vi "main4ChProspectiveStudy.vi"() -> ()   [LabVIEW 2024]
doc: "Main VI for FLS imaging system."
uses:
  SubVI/DigitizerConfiguration/FLImDAQ.ctl
  <instrlib>/niScope/Controls/niScope trigger source.ctl
  SubVI/LabJack/LJ Pin Setting.ctl
  ConfigFiles/AimingBeamVideoConfig.ctl
  LaguerreDeconLib/DeconEngineClass/LaguerreDeconEngineClass.lvclass/LaguerreDeconEngineClass.ctl
  <vilib>/Utility/error.llb/DialogType.ctl
  LaguerreDeconLib/DeconEngineClass/LaguerreDeconEngineClass.lvclass
  <vilib>/event_ctls.llb/usereventprio.ctl
  <vilib>/Utility/miscctls.llb/LVMinMaxIncTypeDef.ctl
  SubVI/APD/APDClass.lvclass
  <vilib>/Analysis/baseanly.llb/Mean (DBL).vi
  SubVI/GlobalVariables.vi
  <vilib>/addons/control/pid/pid.llb/PID (DBL).vi
  <instrlib>/niScope/Acquire/Fetch/niScope Multi Fetch Binary 16.vi
  <vilib>/Instr/_visa.llb/VISA Configure Serial Port (Instr).vi
  <vilib>/Python/Open Anaconda Python Session.vi
  C:/Users/MarcuLab/Documents/GitHub/NetDeconForLV/Source/DotNETAssembly/output/build/LaguerreDeConNative.dll
  Documents/GitHub/NetDeconForLV/Source/DotNETAssembly/output/build/LaguerreDeConNative.dll
  <userlib>/_OpenG.lib/file/file.llb/openg_file.lvlib
  <userlib>/_OpenG.lib/time/time.llb/openg_time.lvlib
  <vilib>/Analysis/NI_AALBase.lvlib
  <vilib>/Utility/miscctls.llb/LVPointTypeDef.ctl
  <vilib>/addons/control/pid/NI_PID_pid.lvlib
panel:
  in  "488nm Power":u16(ring)=32 items=["3.30mW"=60, "2.35mW"=50, "2.00mW"=47, "1.75mW"=44, "1.48mW"=41, "1.16mW"=38, "0.87mW"=35, "0.57mW"=32, "0.28mW"=29]
  in  "CancerThreshold":dbl=0.15
  out "Decon Loop timing (ms)":dbl
  out "Ch3 Lifetime (ns)":dbl caption="Lifetime (ns)"
  out "Ch2 Lifetime (ns)":dbl caption="Lifetime (ns)"
  out "Ch1 Lifetime (ns)":dbl caption="Lifetime (ns)"
  out "Cancer Prob":dbl
  in  "Overlay selection":u16(ring)=2 items=["Gain", "Lifetime", "CancerProbability"]
  out "Record Backlog 2":i32
  in  "Auto gain ch4":bool=TRUE caption="Auto gain ch3"
  in  "V 4":dbl caption="Gain 3" min=0.0 max=4.67 step=0.1
  out "Gain4":dbl
  out "IntR4":dbl format="%#_2g"
  out "SNR4":dbl format="%#_3g"
  out "Channel 4":dbl[][](graph) caption="Channel 3"
  out "RunStartTime":u32
  out "Dig1 Temp":dbl
  out "Dig2 Temp":dbl
  out "Visualization PC video source":T1
  in  "V target(1.0)":dbl=1.0 caption="V target(1.5)" min=0.3 max=1.5 step=0.1 format="%#_4g"
  out "SNR3":dbl format="%#_3g"
  out "SNR2":dbl format="%#_3g"
  out "SNR1":dbl format="%#_3g"
  in  "Show BG removed?":bool=TRUE
  out "IntR3":dbl format="%#_2g"
  out "IntR2":dbl format="%#_2g"
  out "IntR1":dbl format="%#_2g"
  in  "Video Display":bool
  out "Gain3":dbl
  out "Gain2":dbl
  out "Gain1":dbl
  in  "Skip Data Save?":bool
  out "Aq Loop?":bool
  out "ML?":bool
  out "aquisition loop Error Out":errorcluster
  out "Laser f (Hz)":dbl
  out "Record Backlog":i32
  out "Fetch Record #":i32
  out "Sync Success?":bool
  out "Disclamer":picture
  out "Calibration #":i8
  out "BG #":i8
  in  "TCP Connect":bool
  out "Help":string
  in  "355nm Laser toggle":bool caption="355nm 460Hz"
  in  "Cali&iRF alignment":bool
  in  "Background":bool
  in  "Aiming beam toggle":bool caption="488nm 15Hz"
  in  "Auto gain ch3":bool=TRUE
  in  "Auto gain ch2":bool=TRUE
  in  "Auto gain ch1":bool=TRUE
  out "Run #":i8
  in  "StopButton":bool caption="Stop"
  out "Aquisition Status:":bool
  in  "StartButton":bool caption="Start"
  in  "V 3":dbl caption="Gain 3" min=0.0 max=4.6 step=0.1
  in  "V 2":dbl caption="Gain 2" min=0.0 max=4.6 step=0.1
  in  "V 1":dbl caption="Gain 1" min=0.0 max=4.6 step=0.1 format="%#_4g"
  in  "Video Source":enum32{"Camera", "FrameGrabber"}(radio)
  out "Case #":string
  out "System Hardware Connection Status":T2
  out "Channel 3":dbl[][](graph)
  out "Channel 2":dbl[][](graph)
  out "Channel 1":dbl[][](graph)
  in  "Tab Control":T3(tab)
  out "display loop timing(ms)":u32
  out "Aquisition loop timing(ms)":u32 format="%.2f"
  out "DisplayLoop":i32
  out "PID loop":i32 caption="processing loop"
  out "PID loop timing(ms)":u32 caption="processing loop timing(ms)"
  out "Communication loop(ms)":u32
  out "laser EM lamp V":dbl format="%0.6f"
  out "Auisition Loop idx":i32
  out "LJ process (ms)":u32
  out "LJ time(ms)":u32[](array[numeric])
  out "output variable":i32
  out "BG Graph":dbl[][](graph)
  out "Lifetime (ns)":cluster{dbl, dbl, dbl}(graph)
  out "DeCon Speed(ms)":dbl(graph)
  out "iRF Graph":dbl[][](graph)
  in  "Show BG":bool
  out "iRF length":i32
  out "BG length":i32
  out "data length":i32
  out "WarmupTime(ms)":u32
  out "BGAll":dbl[][](array[numeric])
  out "DeConOut":dbl[](array[numeric])
  in  "Ch1GainLim":dbl=350.0 format="%#_13g"
  in  "Ch2&3GainLim":dbl=1750.0 format="%#_13g"
  out "LJ Pinout":T4={"Ch1 Bias"="DAC0", "Ch2 Bias"="DAC1", "Ch3 Bias"="DAC2", "Ch4 Bias"="DAC0", "355 PWM"="FIO0", "AimingBeam PWM"="FIO2", "Laser Ready"="FIO3", "Interlock"="FIO1", "Laser Start/Stop"="FIO1", "Red LED"="FIO1", "Green LED"="DIO3", "Foot Pedal"="DIO15"}
  out "FLImDAQ":T5={"Digitizer 1"="", "Digitizer 2"="", "Channel"=enum."Channel 0", "trigger source"="VAL_EXTERNAL", "trigger level"=0.5, "trigger delay"=1.35e-07, "min sample rate"=12500000000.0, "min record length"=2500, "vertical range"=1.0, "vertical offset"=-0.25, "Waveform to Avg"=2000} caption="FLIm DAQ Configuration" {"trigger delay" format="%^#.4e"; "trigger level" min=0.0 max=3.5 step=0.5 format="%.2f"; "vertical offset" format="%.4f"; "vertical range" format="%.2f"; "min sample rate" format="%#.2p"}
  in  "Sys Reconfig":bool
  out "data out(communcation loop)":string
  out "PID loop error out":errorcluster caption="processing Error Out"
  out "decon error out":errorcluster
  out "Laser Rep Rate":dbl
  out "V4 Size":i32 caption="V3 Size"
  in  "Data Class":enum16{"Data", "BG", "Cali"}(ring)=enum."BG"
  out "V1 Size":i32
  out "V2 Size":i32
  out "V3 Size":i32
  out "data Size":i32[](array[numeric])
  out "State log":string
  out "SysConfigCluster":T7
  in  "Ch4 PID gains":T8={"proportional gain (Kc)"=30.0, "integral time (Ti, min)"=0.0003, "derivative time (Td, min)"=1e-05}
  in  "Ch3 PID gains":T8={"proportional gain (Kc)"=30.0, "integral time (Ti, min)"=0.0003, "derivative time (Td, min)"=1e-05}
  in  "Ch2 PID gains":T8={"proportional gain (Kc)"=30.0, "integral time (Ti, min)"=0.0003, "derivative time (Td, min)"=1e-05}
  in  "Ch1 PID gains":T8={"proportional gain (Kc)"=30.0, "integral time (Ti, min)"=0.0003, "derivative time (Td, min)"=1e-05}
  in  "module path":path=path "C:/Users/MarcuLab/Documents/GitHub/NetDeconForLV/Classifier/ClassifierModule.py"
  in  "model path":path=path "C:/Users/MarcuLab/Desktop/V6 APD LV/V6 APD LV/ClassifierFile/xgb_model.pkl"
  in  "Env name":string="HNClassifier"
  in  "Python version":string="3.10"
  out "Python session":refnum<k35>
  in  "Quit":bool
  in  "Radio Buttons":T9(radio)=enum."Ch2" caption="DeCon Chan"
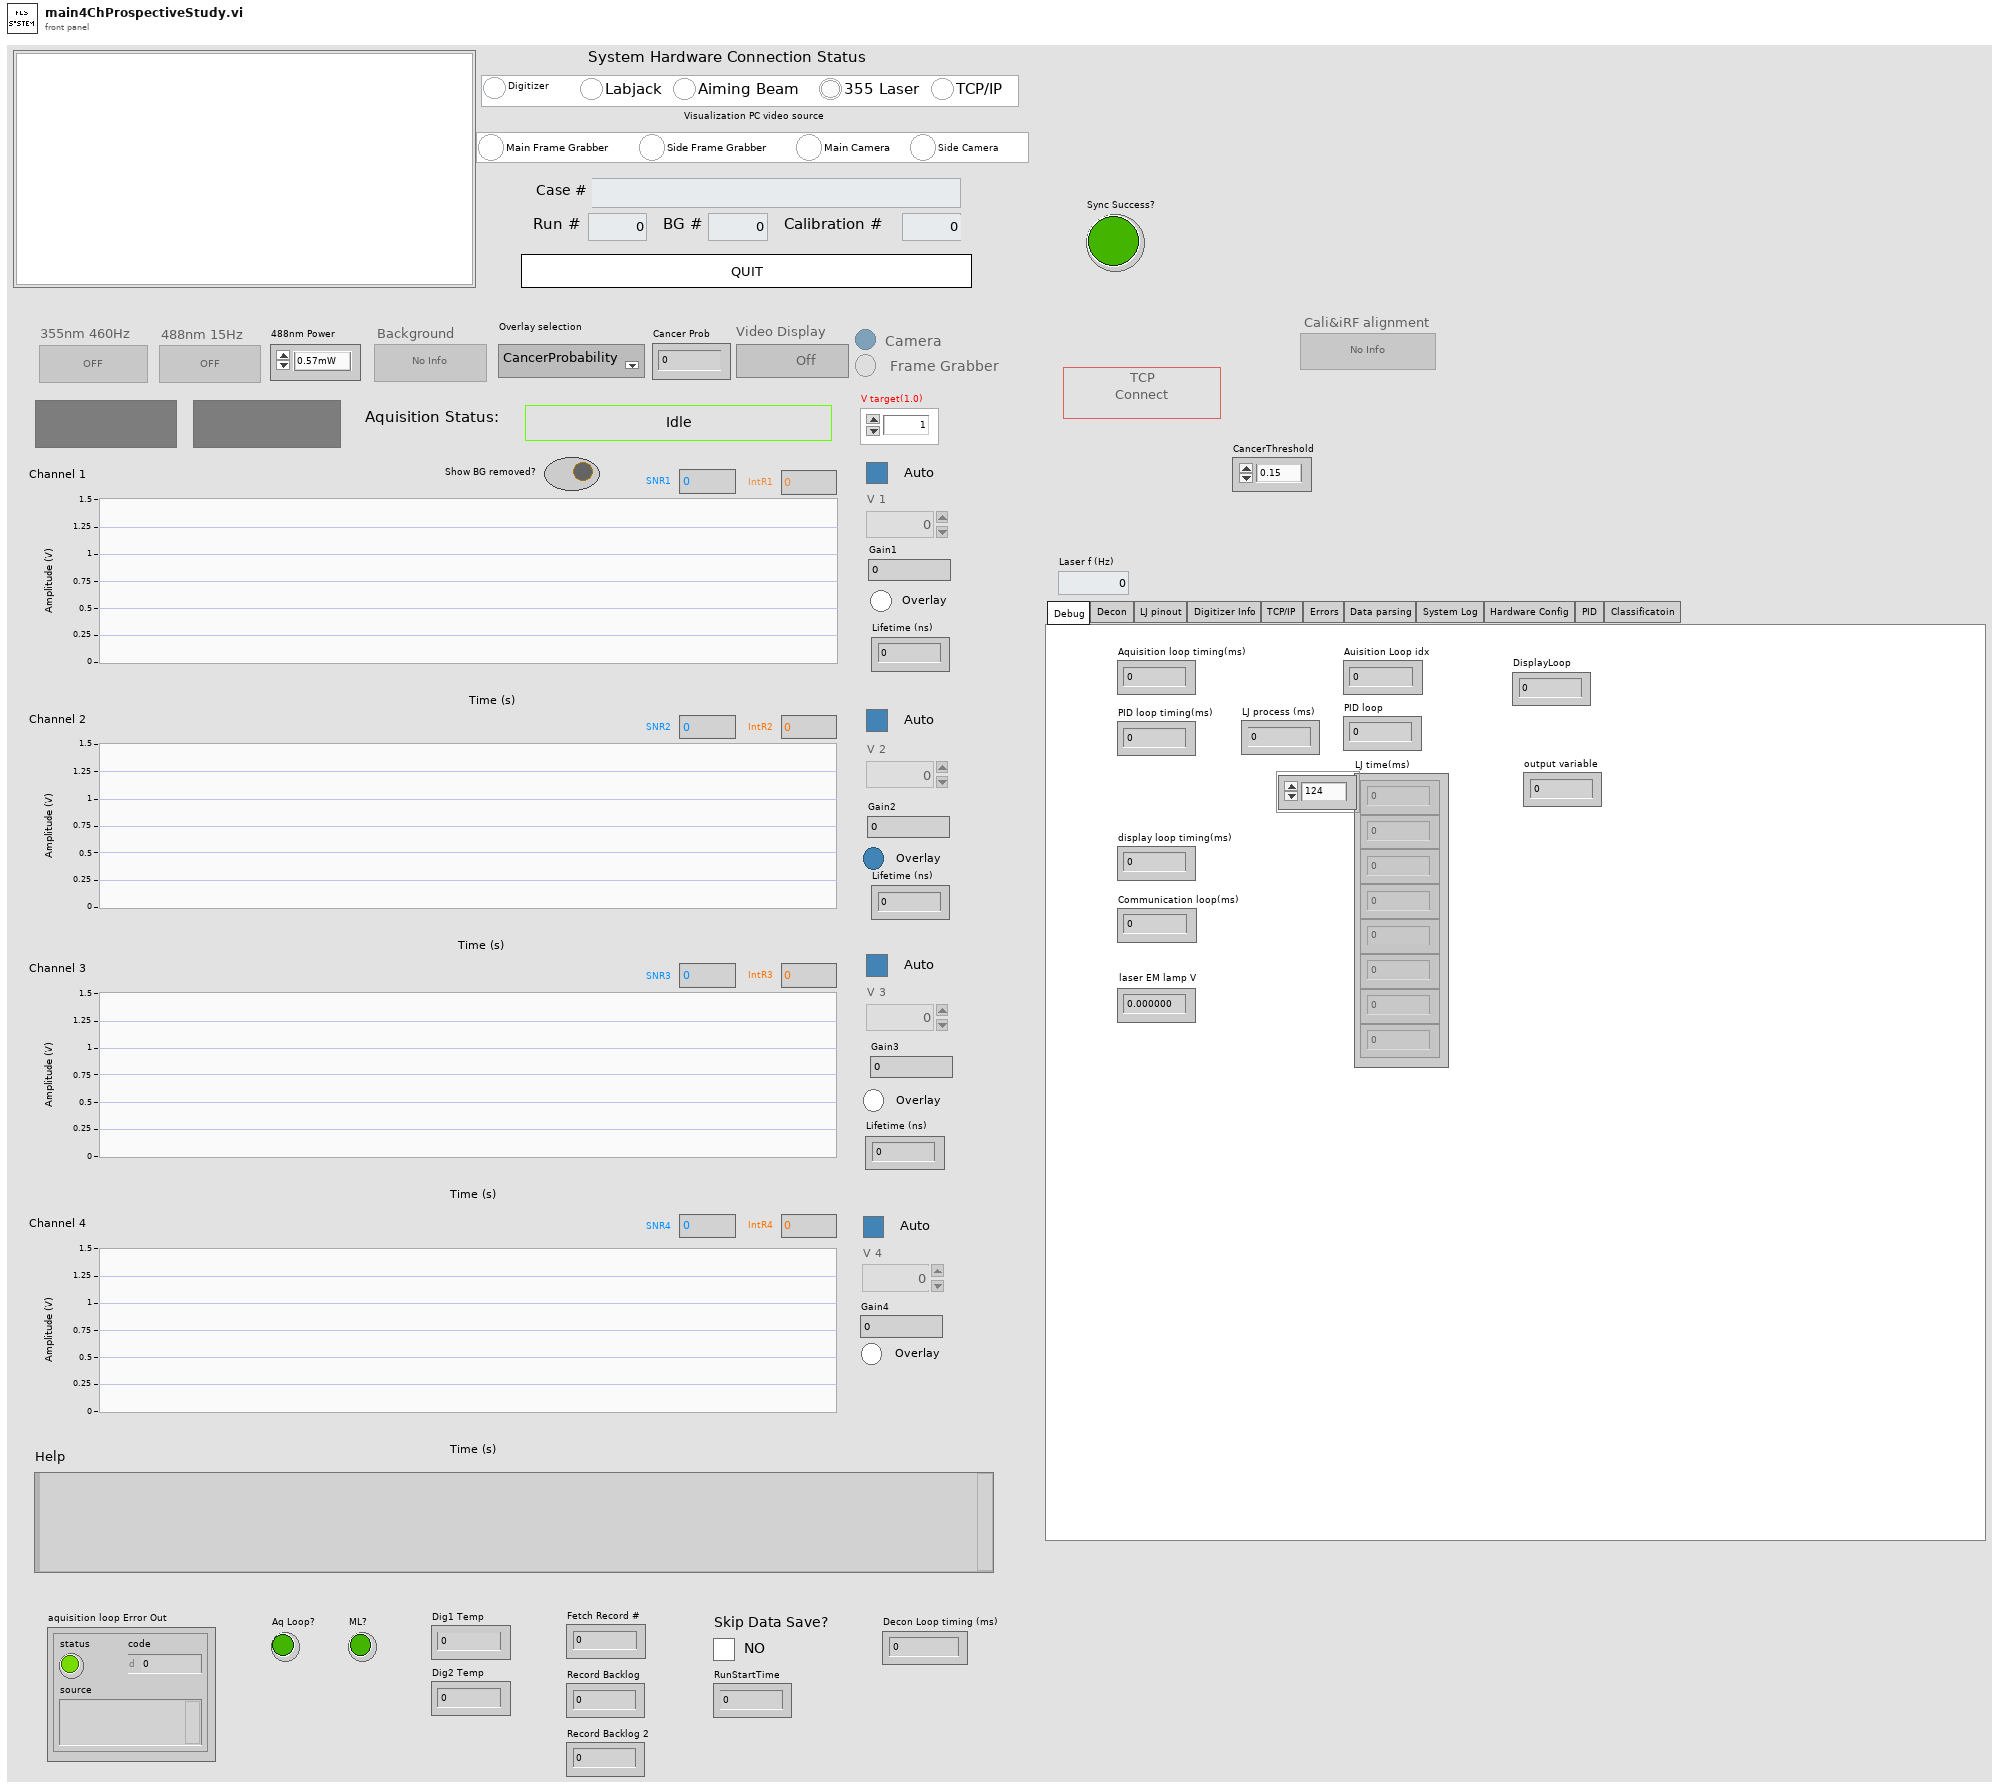
[diagram p1: front panel]
types:
  T1 = cluster{"Main Frame Grabber":bool, "Side Frame Grabber":bool, "Main Camera":bool, "Side Camera":bool}
  T2 = cluster{"Digitizer":bool, "Labjack":bool, "Aiming Beam":bool, "355 Laser":bool, "TCP/IP":bool}
  T3 = enum32{"Debug", "Decon", "LJ pinout", "Digitizer Info", "TCP/IP", "Errors", "Data parsing", "System Log", "Hardware Config", "PID", "Classificatoin"}
  T4 = typedef "LJ Pin Setting.ctl" = cluster{"Ch1 Bias":string, "Ch2 Bias":string, "Ch3 Bias":string, "Ch4 Bias":string, "355 PWM":string, "AimingBeam PWM":string, "Laser Ready":string, "Interlock":string, "Laser Start/Stop":string, "Red LED":string, "Green LED":string, "Foot Pedal":string}
  T5 = typedef "FLImDAQ.ctl" = cluster{"Digitizer 1":refnum<k15>, "Digitizer 2":refnum<k15>, "Channel":enum16{"Channel 0", "Channel 1", "Channel 0&1"}, "trigger source":T6, "trigger level":dbl, "trigger delay":dbl, "min sample rate":dbl, "min record length":i32, "vertical range":dbl, "vertical offset":dbl, "Waveform to Avg":i16}
  T6 = typedef "niScope trigger source.ctl" = string
  T7 = cluster{"Ch1Enable?":bool, "Ch2Enable?":bool, "Ch3Enable?":bool, "Ch1AutoGain?":bool, "Ch2AutoGain?":bool, "Ch3AutoGain?":bool, "AimingBeamEnable?":bool}
  T8 = cluster{"proportional gain (Kc)":dbl, "integral time (Ti, min)":dbl, "derivative time (Td, min)":dbl}
  T9 = enum32{"No Selection", "Ch1", "Ch2", "Ch3", "Ch4"}
  T10 = cluster{"remote start event":refnum<user-event>, "remote stop  event":refnum<user-event>}
  T11 = enum8{"Enabled", "Disabled", "Disabled and Grayed Out"}
  T12 = enum16{"open", "replace", "create", "open or create", "replace or create", "replace or create with confirmation"}
  T13 = cluster{"CH1":dbl[][], "CH2":dbl[][], "CH3":dbl[][], "CH4":dbl[][], "Gain cluster":cluster{"V1":dbl, "V2":dbl, "V3":dbl, "V4":dbl}}
  T14 = cluster{"idx":i32, "CH1&2":dbl[][], "CH3&4":dbl[][], "V cluster":cluster{"V1":dbl, "V2":dbl, "V3":dbl, "V4":dbl}}
  T15 = enum16{"open", "open or create", "create or replace", "create", "open (read-only)"}
  T16 = cluster{"Ch1 iRF":dbl[], "Ch2 iRF":dbl[], "Ch3 iRF":dbl[], "Ch4 iRF":dbl[]}
  T17 = enum32{"Invalid", "Standard", "Closed", "Hidden", "Minimized", "Maximized"}
  T18 = enum32{"invalid app kind", "Development System", "Run Time System", "Student Edition", "Embedded LabVIEW", "Evaluation", "Custom"}
  T19 = typedef "usereventprio.ctl" = enum32{"high priority", "normal priority"}
  T20 = enum32{"Bad", "Idle", "Run top level", "Running"}
  T21 = enum16{"Standard", "Buffered", "CRLF", "Immediate"}
  T22 = typedef "AimingBeamVideoConfig.ctl" = cluster{"DeCon Channel":enum16{"1", "2", "3"}, "Scale Bar":bool, "Scale Low":dbl, "Scale High":dbl, "ANSI":dbl, "Radius":dbl, "3D?":bool, "Firefly?":bool, "Pentero?":bool}
  T23 = cluster{"Core":cluster{"Current VI Reference":refnum<vi>, "Close Panel on Exit?":bool}, "SysConfigCluster":cluster{"Ch1Enable?":bool, "Ch2Enable?":bool, "Ch3Enable?":bool, "Ch1AutoGain?":bool, "Ch2AutoGain?":bool, "Ch3AutoGain?":bool, "AimingBeamEnable?":bool}, "System Status":cluster{"Digitizer":bool, "Labjack":bool, "Aiming Beam":bool, "355 Laser":bool, "TCP/IP":bool}, "IDs":cluster{"RunID":i8, "BG ID":i8, "Cali ID":i8}, "CaseID":string, "DefaultPath":path, "Pathes":cluster{"DataPath":path, "BG Path":path, "iRFPath":path, "CaliPath":path}, "FLImDAQ":cluster{"resource name":refnum<k15>, "resource name 2":refnum<k15>, "Channel":enum16{"Channel 0", "Channel 1", "Channel 0&1"}, "trigger source":T6, "trigger level":dbl, "trigger delay":dbl, "min sample rate":dbl, "min record length":i32, "vertical range":dbl, "vertical offset":dbl, "Waveform to Avg":i32}, "SysRunning?":bool, "AB Cluster":cluster{"Aiming Beam COM Port":refnum<visa-resource-name>, "Min Current":dbl, "Max Current":dbl, "Default Current":dbl, "Freq":i32}, "LJ Pinout":T4, "355 PWM setting":cluster{"DIO_EF_CLOCK1_DIVISOR":i16, "DIO_EF_CLOCK1_ROLL_VALUE":i32, "DIO#_EF_INDEX":i16, "DIO#_EF_OPTIONS":i16, "DIO#_EF_CONFIG_A":i32}, "AB PWM setting":cluster{"DIO_EF_CLOCK1_DIVISOR":i16, "DIO_EF_CLOCK1_ROLL_VALUE":i32, "DIO#_EF_INDEX":i16, "DIO#_EF_OPTIONS":i16, "DIO#_EF_CONFIG_A":i32}, "Last Trigger":u32, "niTClk sessions":refnum<k20>[], "Laser start tic":u32, "TCP attempt count":i32, "Ch1Data":dbl[][], "Ch2Data":dbl[][], "Ch3Data":dbl[][], "Ch4Data":dbl[][], "V1":dbl[], "V2":dbl[], "V3":dbl[], "V4":dbl[], "SlowTimer":u32, "FastTimer":u32, "listener ID":refnum<k5>, "TempPath":path, "CaliPath":path, "LED vi reference":refnum<vi>, "Aquisition Timer":u32, "APDSerialNum":cluster{"Ch1APDSerial#":string, "Ch2APDSerial#":string, "Ch3APDSerial#":string, "Ch4APDSerial#":string}, "VideoConfig":T22, "LED vi ref open?":bool, "video source":cluster{"Main Frame Grabber":bool, "Side Frame Grabber":bool, "Main Camera":bool, "Side Camera":bool}, "bothVidSourceAvail":bool}
  T24 = typedef "LVCursorListTypeDef.ctl" = cluster{"Name":string, "Color":u32, "Style":u8, "Point Style":u8, "Name Visible":bool, "Allow Drag":bool, "Cursor Mode":u32, "Plot":i32, "Index":i32, "Position":cluster{"X":dbl, "Y":dbl}, "X Scale":u32, "Y Scale":u32, "Watch Plots":i32[], "Watch All Plots":bool, "Plot Area":i32, "Label Offset":cluster{"X":dbl, "Y":dbl}}[]
  T25 = cluster{"Name":string, "Color":u32, "Style":u8, "Point Style":u8, "Name Visible":bool, "Allow Drag":bool, "Cursor Mode":u32, "Plot":i32, "Index":i32, "Position":cluster{"X":dbl, "Y":dbl}, "X Scale":u32, "Y Scale":u32, "Watch Plots":i32[], "Watch All Plots":bool, "Plot Area":i32, "Label Offset":cluster{"X":dbl, "Y":dbl}}
  T26 = cluster{"Ch1APDSerial#":string, "Ch2APDSerial#":string, "Ch3APDSerial#":string, "Ch4APDSerial#":string}
  T27 = cluster{"DataPath":path, "BG Path":path, "iRFPath":path, "CaliPath":path}
  T28 = cluster{"DIO_EF_CLOCK1_DIVISOR":i16, "DIO_EF_CLOCK1_ROLL_VALUE":i32, "DIO#_EF_INDEX":i16, "DIO#_EF_OPTIONS":i16, "DIO#_EF_CONFIG_A":i32}
  T29 = cluster{"Aiming Beam COM Port":refnum<visa-resource-name>, "Min Current":dbl, "Max Current":dbl, "Default Current":dbl, "Freq":i32}
  T30 = cluster{"resource name":refnum<k15>, "resource name 2":refnum<k15>, "Channel":enum16{"Channel 0", "Channel 1", "Channel 0&1"}, "trigger source":T6, "trigger level":dbl, "trigger delay":dbl, "min sample rate":dbl, "min record length":i32, "vertical range":dbl, "vertical offset":dbl, "Waveform to Avg":i32}
  T31 = cluster{"Current VI Reference":refnum<vi>, "Close Panel on Exit?":bool}
  T32 = cluster{"Channel 1":dbl[], "Channel 2":dbl[], "Channel 3":dbl[], "Channel 4":dbl[]}
  T33 = cluster{"V 1":dbl[], "V 2":dbl[], "V 3":dbl[], "V 4":dbl[]}
  T34 = cluster{"Ch1 WF":dbl[], "Ch2 WF":dbl[], "Ch3 WF":dbl[], "Ch4 WF":dbl[], "V1":dbl, "V2":dbl, "V3":dbl, "V4":dbl}
  T35 = typedef "iRFData.ctl" = cluster{"dt":dbl, "NumOfWFs":i32, "WFLength":i32, "iRFCtrlV":dbl[], "iRFWFsAvg":dbl[][], "iRFRaw":dbl[][]}
  T36 = cluster{"mean":dbl, "mean":dbl, "mean":dbl, "mean":dbl}
  T37 = cluster{"V1":dbl, "V2":dbl, "V3":dbl, "V4":dbl}[]
  T38 = cluster{"DataPath":path, "CaseID":string, "RunID":i16, "Ch1Data":dbl[][], "Ch2Data":dbl[][], "Ch3Data":dbl[][], "Ch4Data":dbl[][], "V1":dbl[], "V2":dbl[], "V3":dbl[], "V4":dbl[], "LaserRepRate":u16, "WFAverage":i16, "RunStartTime":u64}
  T39 = typedef "DialogType.ctl" = u16
  T40 = typedef "APD.ctl" = cluster{"gainV":dbl[], "gain":dbl[], "irfV":dbl[], "irfTNorm":dbl[][]}
  T41 = typedef "LJ PWM Setting.ctl" = cluster{"DIO_EF_CLOCK1_DIVISOR":i16, "DIO_EF_CLOCK1_ROLL_VALUE":i32, "DIO#_EF_INDEX":i16, "DIO#_EF_OPTIONS":i16, "DIO#_EF_CONFIG_A":i32}
  T42 = typedef "AimingBeam.ctl" = cluster{"Aiming Beam COM Port":refnum<visa-resource-name>, "Min Current":dbl, "Max Current":dbl, "Default Current":dbl, "Frequency(Hz)":u32}
  T43 = cluster{"DC1":i32, "DC2":i32, "BG1":i32, "BG2":i32}
  T44 = typedef "LVMinMaxIncTypeDef.ctl" = cluster{"Minimum":dbl, "Maximum":dbl, "Increment":dbl}
  T45 = typedef "LVBoundsTypeDef.ctl" = cluster{"Width":u32, "Height":u32}
  T46 = typedef "imagedata.ctl" = cluster{"image type":i32, "image depth":i32, "image":u8[], "mask":u8[], "colors":u32[], "Rectangle":cluster{"left":i16, "top":i16, "right":i16, "bottom":i16}}
  T47 = cluster{"DC Idx1":i32, "DC Idx2":i32, "BG Idx1":i32, "BG Idx2":i32}
  T48 = cluster{dbl[][], dbl[][], dbl[][], dbl[][], "V cluster":cluster{"V1":dbl, "V2":dbl, "V3":dbl, "V4":dbl}}
  T49 = cluster{"actualSamples":i32, "absoluteInitialX":dbl, "relativeInitialX":dbl, "xIncrement":dbl, "offset":dbl, "gain":dbl, "reserved1":dbl, "reserved2":dbl}[]
  T50 = cluster{"V1 out":dbl, "V2 out":dbl, "V3 out":dbl, "V3 out":dbl}
  T51 = cluster{i32, dbl[][], dbl[][], cluster{"V1 out":dbl, "V2 out":dbl, "V3 out":dbl, "V3 out":dbl}}
  T52 = typedef "LVPointTypeDef.ctl" = cluster{"Horizontal":i16, "Vertical":i16}
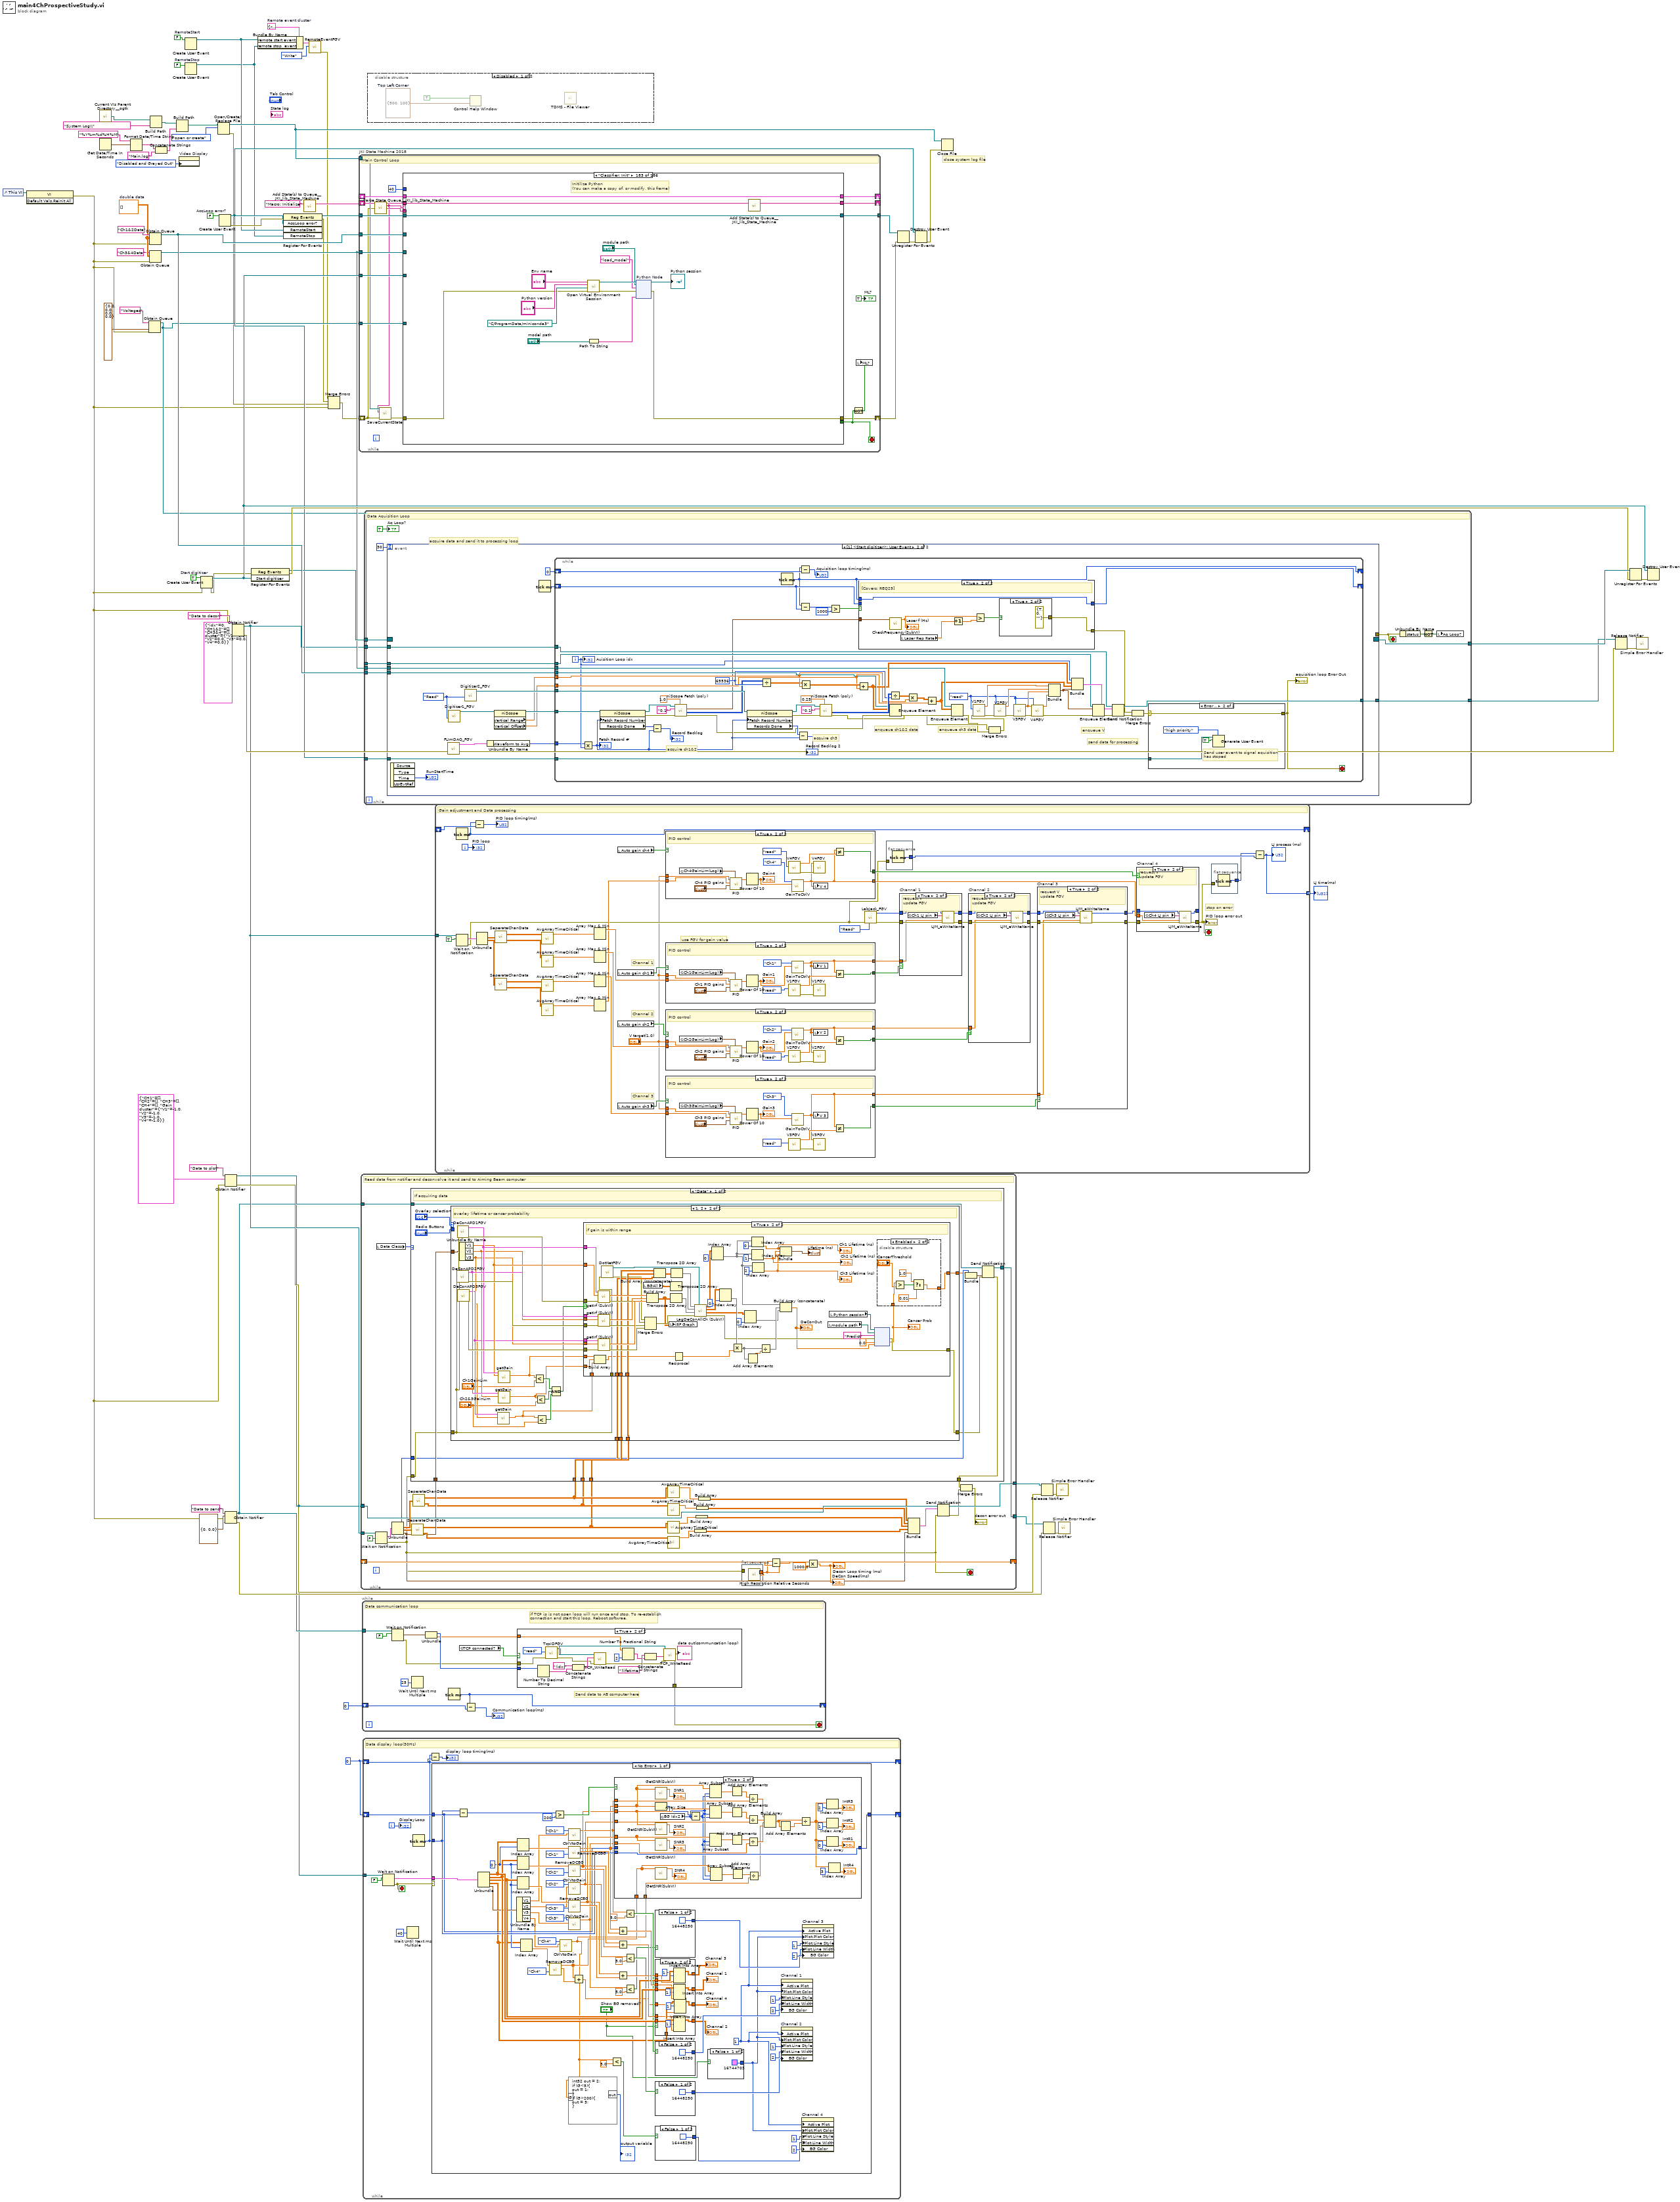
[diagram p0: block diagram]
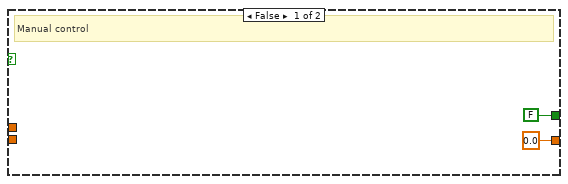
[diagram p6: hidden frame]
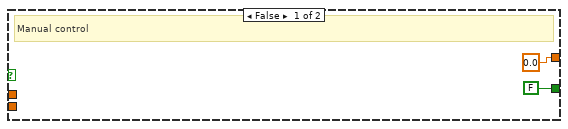
[diagram p7: hidden frame]
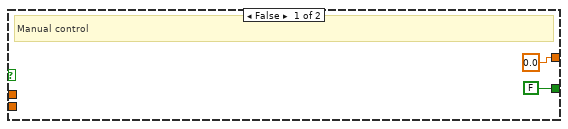
[diagram p8: hidden frame]
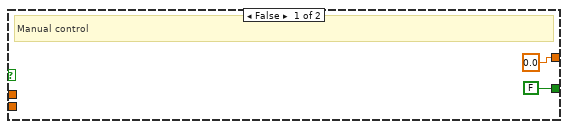
[diagram p9: hidden frame]
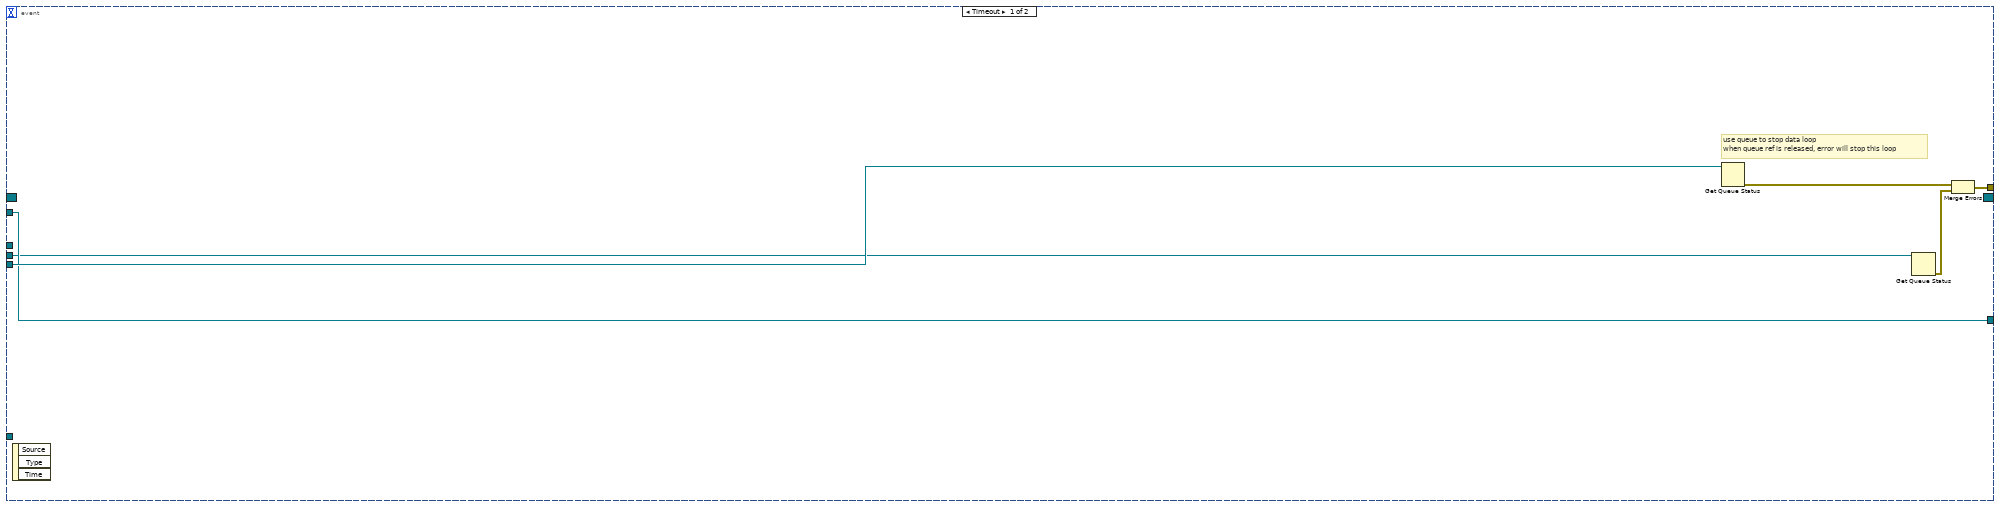
[diagram p10: hidden frame]
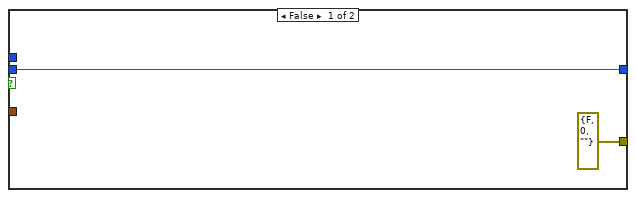
[diagram p11: hidden frame]
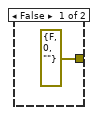
[diagram p12: hidden frame]
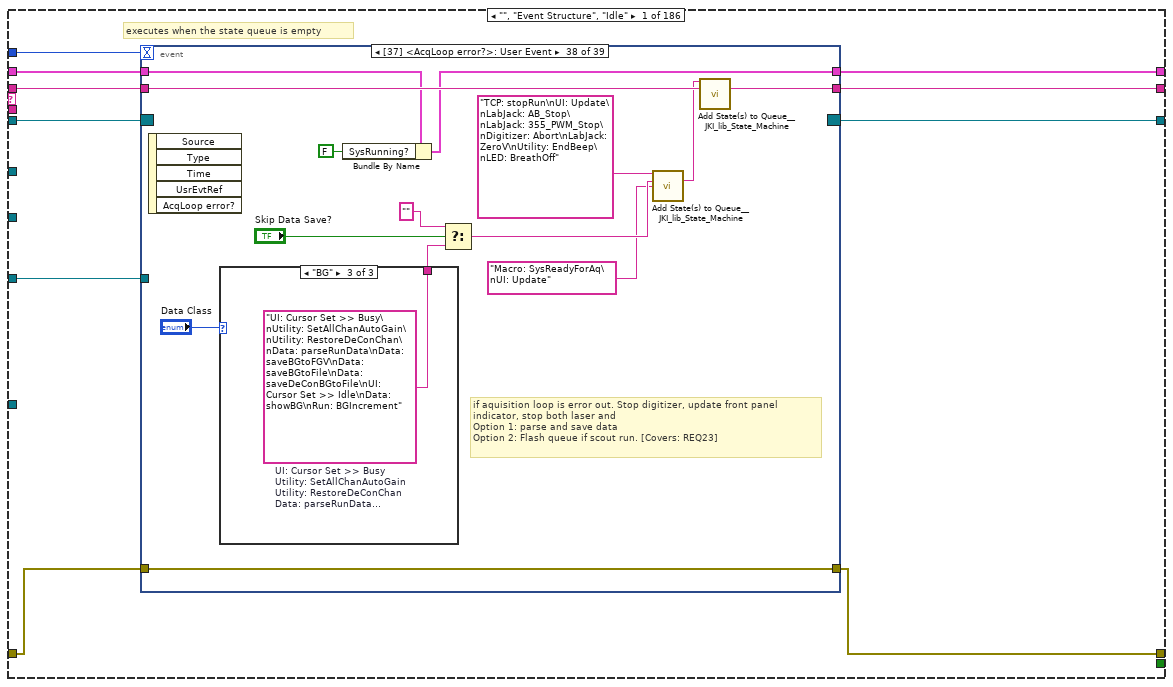
[diagram p14: hidden frame]
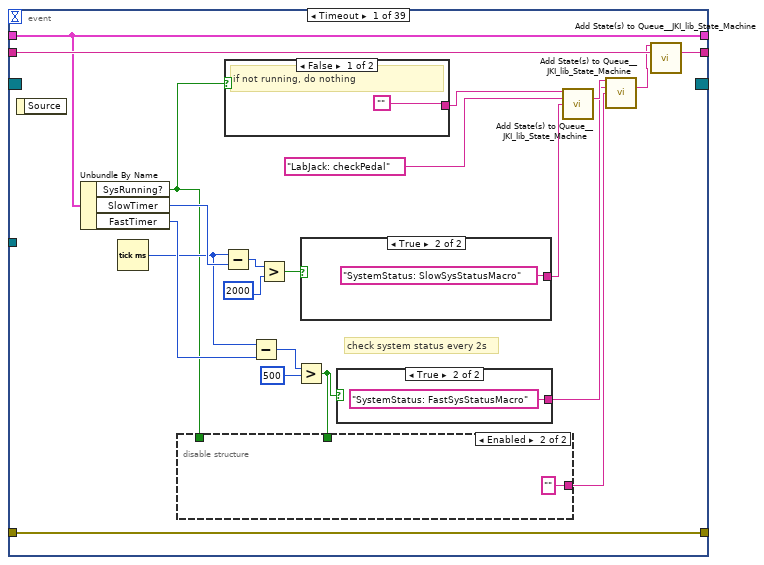
[diagram p15: hidden frame]
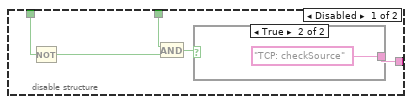
[diagram p16: hidden frame]
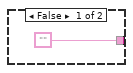
[diagram p17: hidden frame]
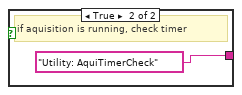
[diagram p18: hidden frame]
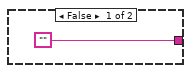
[diagram p19: hidden frame]
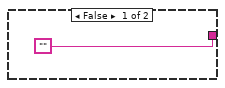
[diagram p20: hidden frame]
diagram:
  w8 = T10 {"remote start event"=refnum, "remote stop  event"=refnum}  # Remote event cluster
  w11 = FALSE  # RemoteStop
  w12 = FALSE  # RemoteStart
  w15 = u32 0 ("millisecond timer value")
  w54 = FALSE  # AcqLoop error?
  w64 = TRUE  # Start digitizer
  w67 = dbl[][] []  # double data
  # "close system log file"
  n1 = control-ref of="This VI"() -> (w69:refnum<vi>)
  n2 = invoke on="Invoke Node" class="VI" method="Default Vals.Reinit All"(reference=w69) -> (error out=w23:errorcluster)  [unwired: 2 in, 2 out]
  n3 = call <userlib>:"Current VIs Parent Directory__ogtk.vi"() -> ("Parent Directory (+ Relative)"=w34:path)  [unwired: 5 in]
  n4 = Get Date/Time In Seconds() -> (seconds since 1Jan1904=w32:timestamp)
  n5 = Format Date/Time String(time format string (%c)="%Y%m%d%H%M", seconds (now)=w32) -> (date/time string=w29:string)  [unwired: 1 in]
  n6 = Obtain Queue(name (unnamed)="Voltages", element data type=cluster{"V1":dbl, "V2":dbl, "V3":dbl, "V4":dbl} {"V1"=0.0, "V2"=0.0, "V3"=0.0, "V4"=0.0}, error in (no error)=w23) -> (queue out=w35:refnum<queue>)  [unwired: 2 in, 2 out]
  n7 = Obtain Queue(name (unnamed)="Ch3&4Data", element data type=w67, error in (no error)=w23) -> (queue out=w48:refnum<queue>)  [unwired: 2 in, 2 out]
  n8 = Obtain Queue(name (unnamed)="Ch1&2Data", element data type=w67, error in (no error)=w23) -> (queue out=w65:refnum<queue>)  [unwired: 2 in, 2 out]
  n9 = Build Path(base path=w34, name or relative path="System Log\\") -> (appended path=w25:path)
  n10 = Concatenate Strings(w29, "Main.log" ("string")) -> (w27:string)
  n11 = Build Path(base path=w25, name or relative path=w27) -> (appended path=w30:path)
  n12 = property on="Video Display" class="Bool (strict)"("DisabledEnum"=T11."Disabled and Grayed Out" ("Disabled")) -> ()  [unwired: 2 in, 2 out]
  n13 = Create User Event(user event datatype=w12) -> (user event=w10:refnum<user-event>)  [unwired: 1 in, 1 out]
  n14 = Create User Event(user event datatype=w11) -> (user event=w9:refnum<user-event>)  [unwired: 1 in, 1 out]
  n15 = Create User Event(user event datatype=w64, error in=w23) -> (user event=w53:refnum<user-event>, error out=w40:errorcluster)
  n16 = Open/Create/Replace File(file path (use dialog)=w30, operation (0:open)=T12."open or create") -> (refnum out=w21:refnum<file>, error out=w22:errorcluster)  [unwired: 4 in, 1 out]
  n17 = Create User Event(user event datatype=w54) -> (user event=w39:refnum<user-event>, error out=w41:errorcluster)  [unwired: 1 in]
  n18 = Obtain Notifier(name (unnamed)="Data to plot", notification data type=T13 {"CH1"=[], "CH2"=[], "CH3"=[], "CH4"=[], "Gain cluster"={"V1"=-1.0, "V2"=-1.0, "V3"=-1.0, "V4"=-1.0}}, error in (no error)=w23) -> (notifier out=w13:refnum<notifier>, error out=w49:errorcluster)  [unwired: 1 in, 1 out]
  n19 = Obtain Notifier(name (unnamed)="Data to send", notification data type=cluster{"idx":i32, "lifetime":dbl} {"idx"=0, "lifetime"=0.0}, error in (no error)=w23) -> (notifier out=w18:refnum<notifier>, error out=w38:errorcluster)  [unwired: 1 in, 1 out]
  n20 = Obtain Notifier(name (unnamed)="Data to decon", notification data type=T14 {"idx"=0, "CH1&2"=[], "CH3&4"=[], "V cluster"={"V1"=0.0, "V2"=0.0, "V3"=0.0, "V4"=0.0}}, error in (no error)=w23) -> (notifier out=w19:refnum<notifier>, error out=w58:errorcluster)  [unwired: 1 in, 1 out]
  n21 = register-events(error in=w40, w53) -> (reference out=w55:refnum<event-registration>, error out=w61:errorcluster)  [unwired: 1 in]
  n22 = Bundle By Name(cluster=w8, "remote start event"=w10, "remote stop  event"=w9) -> (w6:T10)
  n23 = register-events(error in=w41, w39, w10, w9) -> (reference out=w47:refnum<event-registration>, error out=w5:errorcluster)  [unwired: 1 in]
  n24 = call <vilib>:"Add State(s) to Queue__JKI_lib_State_Machine.vi"("State(s) in (\"\")"="Macro: Initialize") -> ("States Out"=w71:string)  [unwired: 14 in]
  n25 = call "RemoteEventFGV.vi"("Operation (Read)"=enum16{"Read", "Write"}."Write", "Remote Event in"=w6) -> ("Error Out"=w2:errorcluster)  [unwired: 8 in, 1 out]
  n26 = Merge Errors(w2, w5, w22, w23) -> (w24:errorcluster)
  n27 = while "JKI State Machine 2018" {
    shift-right: [w88] -> _
    shift-left: _ -> [w87]
    shift-right: [w72] -> w4
    shift-left: w24 -> [w74]
    shift-right: [w89] -> _
    shift-left: w71 -> [w90]
    tunnel: w65 -> [w85]
    tunnel: w48 -> [w84]
    tunnel: w53 -> [w83]
    tunnel: w47 -> [w82]
    tunnel: [w81] -> w46
    tunnel: w35 -> [w77]
    tunnel: w21 -> [w76]
    stop <- w80 stop-if-true
    # "Main Control Loop"
    n28 = call <vilib>:"Parse State Queue__JKI_lib_State_Machine.vi"("State Queue"=w90, "Error In (no error)"=w74) -> ("Remaining States"=w92:string, "Current State"=w75:string, "Arguments"=w91:string)  [unwired: 11 in]
    n29 = call "SaveCurrentState.vi"("error in (no error)"=w74, "Current State"=w75, "Byte Stream File in"=w76) -> ("error out"=w73:errorcluster)  [unwired: 8 in]
    n30 = case shown="\"Classifier: Init\"" w75 {
      selector: w75 -> [_ _ _ _ _ _ _ _ _ _ _ _ _ _ _ _ _ _ _ _ _ _ _ _ _ _ w1131 _ _ _ _ _ _ _ _ _ _ _ _ _ _ _ _ _ _ _ _ _ _ _ _ _ _ _ _ _ _ _ _ _ _ _ _ _ _ _ _ _ _ _ _ _ _ _ _ _ _ _ _ _ _ _ _ _ _ _ _ _ _ _ _ _ _ _ _ _ _ _ _ _ _ _ _ _ _ _ _ _ _ _ _ _ _ _ _ _ _ _ _ _ _ _ _ _ _ _ _ _ _ _ _ _ _ _ _ _ _ _ _ _ _ _ _ _ _ _ _ _ _ _ _ _ _ _ _ _ _ _ _ _ _ _ _ _ _ _ _ _ _ _ _ _ _ _ _ _ _ _ _ _ _ _ _ _ _ _]
      tunnel: w92 -> [w102 w515 w524 w530 w536 w558 w571 w613 w619 w646 w671 w683 w754 w769 w800 w827 w859 w890 w919 w945 w950 w1035 w1072 w1111 w1124 w1129 w1135 w1163 w1171 w1194 w1199 w1212 w1231 w1259 w1287 w1325 w1330 w1339 w1350 w1380 w1388 w1394 w1418 w1442 w1466 w1490 w1495 w1512 w1559 w1581 w1597 w1612 w1632 w1637 w1649 w1678 w1704 w1716 w1754 w1767 w1773 w1784 w1796 w1827 w1840 w1854 w1869 w1888 w1923 w1928 w1942 w1952 w1968 w1980 w1992 w2020 w2035 w2040 w2052 w2064 w2069 w2077 w2085 w2094 w2103 w2108 w2116 w2125 w2143 w2160 w2180 w2191 w2209 w2224 w2241 w2246 w2254 w2262 w2267 w2275 w2282 w2290 w2297 w2307 w2335 w2343 w2350 w2358 w2363 w2371 w2378 w2384 w2393 w2409 w2414 w2421 w2433 w2503 w2515 w2524 w2538 w2547 w2564 w2587 w2604 w2615 w2628 w2653 w2676 w2682 w2698 w2720 w2728 w2734 w2739 w2746 w2756 w2768 w2777 w2782 w2794 w2799 w2809 w2815 w2821 w2826 w2831 w2836 w2846 w2870 w2891 w2896 w2907 w2932 w2959 w2982 w2987 w3002 w3053 w3099 w3144 w3155 w3173 w3193 w3207 w3220 w3228 w3245 w3267 w3291 w3310 w3328 w3346 w3364 w3378 w3392 w3411 w3425 w3440 w3455 w3464 w3469 w3485 w3493 w3500 w3505]
      tunnel: w91 -> [_ _ _ _ _ _ _ _ _ _ _ _ _ _ _ _ _ _ _ _ _ _ _ _ _ _ _ _ _ _ _ _ _ _ _ _ _ _ _ _ _ _ _ _ _ _ _ _ _ _ _ _ _ _ _ _ _ _ _ _ _ _ w1794 _ _ _ _ _ _ _ _ _ _ _ _ _ _ _ _ _ _ _ _ _ _ _ _ _ _ _ _ _ _ _ _ _ _ _ _ _ _ _ _ w2298 _ _ _ _ _ _ _ _ _ _ _ w2416 w2427 _ _ _ _ w2544 w2561 _ _ _ _ _ w2672 _ _ _ _ _ _ w2741 _ _ _ _ _ _ w2805 _ _ _ _ _ _ _ _ _ _ _ _ _ _ _ _ _ _ _ _ _ _ _ _ _ _ _ _ _ _ _ _ _ _ _ _ _ _ _ _ _ _ _]
      tunnel: w87 -> [w100 w512 w520 w527 w533 w555 w568 _ w615 w642 w668 w679 w751 w760 w797 w819 w850 w887 w916 w942 w947 w996 w1064 w1099 w1119 w1126 w1133 w1156 w1168 w1192 w1196 w1200 w1221 w1251 w1279 w1321 w1327 w1337 w1348 w1378 w1386 w1391 w1399 w1423 w1448 w1472 w1492 w1505 w1549 w1578 w1582 w1609 w1629 w1634 w1638 w1667 w1694 w1709 w1737 w1765 w1770 w1777 w1792 w1810 w1835 w1846 w1864 w1881 w1906 w1925 w1938 w1946 w1965 w1977 w1989 w2008 w2024 w2037 w2050 w2062 w2066 w2071 w2078 w2090 w2099 w2105 w2112 w2122 w2130 w2147 w2175 w2181 w2206 w2217 w2239 w2243 w2247 w2255 w2264 w2273 w2279 w2287 w2294 w2304 w2332 w2340 w2347 w2355 w2360 w2365 w2376 w2381 w2387 w2406 w2411 w2419 w2429 w2500 w2505 w2518 w2536 w2545 w2562 w2577 w2601 w2612 w2622 w2646 w2673 w2679 w2691 w2716 w2725 w2731 w2736 w2743 w2750 w2764 w2774 w2779 w2791 w2796 w2802 w2812 w2818 w2823 w2828 w2833 w2843 w2868 w2889 w2893 w2905 w2930 w2957 w2980 w2984 w2995 w3047 w3095 w3141 w3151 w3168 w3188 w3202 w3216 w3222 w3240 w3262 w3286 w3305 w3323 w3341 w3359 w3373 w3387 w3406 w3420 w3435 w3452 w3462 w3466 w3483 w3491 w3497 w3502]
      tunnel: [w93 w513 w522 w528 w534 w556 w569 w611 w617 w638 w656 w675 w728 w756 w798 w807 w839 w875 w907 w929 w948 w972 w1061 w1098 w1120 w1127 w1137 w1160 errorcluster {"status"=FALSE, "code"=0, "source"=""} ("error out") w1191 w1197 w1210 w1229 w1243 w1266 w1323 w1328 w1332 w1343 w1353 w1382 w1392 w1400 w1424 w1449 w1473 w1493 w1496 w1541 w1572 w1586 w1610 w1620 w1635 w1641 w1665 w1693 w1708 w1724 w1759 w1771 w1782 w1786 w1801 w1830 w1842 w1860 w1880 w1897 w1926 w1930 w1948 w1963 w1975 w1987 w2010 w2025 w2038 w2042 w2059 w2067 w2075 w2083 w2087 w2096 w2106 w2109 w2118 w2133 w2155 w2174 w2185 w2199 w2221 w2237 w2244 w2252 w2260 w2265 w2272 w2280 w2288 w2295 w2305 w2333 w2341 w2348 w2356 w2361 w2369 w2375 w2382 w2390 w2407 w2412 w2417 w2430 w2501 w2509 w2521 w2528 w2541 w2558 w2578 w2602 w2611 w2624 w2648 w2674 w2680 w2688 w2710 w2726 w2732 w2737 w2744 w2754 w2766 w2775 w2780 w2792 w2797 w2807 w2813 w2819 w2824 w2829 w2834 w2844 w2858 w2882 w2894 w2898 w2917 w2949 w2974 w2985 w2989 w3048 w3096 w3142 w3150 w3170 w3190 w3204 w3218 w3224 w3242 w3264 w3288 w3307 w3325 w3343 w3361 w3375 w3389 w3408 w3422 w3436 w3453 w3460 w3467 w3473 w3486 w3498 w3503] -> w72
      tunnel: w73 -> [w99 w513 w522 w528 w534 w556 w569 w611 w617 w639 w663 w673 w728 w755 w798 w808 w846 w876 w897 w937 w948 w972 w1062 w1101 w1121 w1127 w1136 w1160 w1164 w1191 w1197 w1210 w1229 w1242 w1278 w1323 w1328 w1331 w1344 w1358 w1381 w1392 w1404 w1428 w1453 w1477 w1493 w1503 w1544 w1571 w1585 w1610 w1622 w1635 w1640 w1666 w1684 w1714 w1735 w1758 w1771 w1779 w1789 w1800 w1829 w1845 w1859 w1879 w1896 w1926 w1936 w1949 w1962 w1974 w1986 w2009 w2026 w2038 w2041 w2054 w2067 w2075 w2083 w2086 w2095 w2106 w2110 w2119 w2138 w2154 w2173 w2184 w2205 w2220 w2236 w2244 w2252 w2260 w2265 w2272 w2280 w2288 w2295 w2305 w2333 w2341 w2348 w2356 w2361 w2369 w2375 w2382 w2390 w2407 w2412 w2418 w2431 w2501 w2510 w2520 w2527 w2540 w2557 w2579 w2602 w2611 w2619 w2651 w2674 w2680 w2693 w2709 w2726 w2732 w2737 w2744 w2754 w2766 w2775 w2780 w2792 w2797 w2807 w2813 w2819 w2824 w2829 w2834 w2844 w2857 w2881 w2894 w2897 w2916 w2939 w2965 w2985 _ w3049 w3096 w3142 w3149 w3169 w3189 w3203 w3218 w3223 w3241 w3263 w3287 w3306 w3324 w3342 w3360 w3374 w3388 w3407 w3421 w3434 w3453 w3459 w3467 w3478 w3488 w3498 w3503]
      tunnel: [w101 w514 w523 w529 w535 w557 w570 w612 w618 w645 w670 w682 w753 w768 w799 w826 w858 w889 w918 w944 w949 w1034 w1071 w1110 w1123 w1128 w1134 w1162 w1170 w1193 w1198 w1211 w1230 w1258 w1286 w1324 w1329 w1338 w1349 w1379 w1387 w1393 w1417 w1441 w1465 w1489 w1494 w1511 w1558 w1580 w1596 w1611 w1631 w1636 w1648 w1677 w1703 w1715 w1753 w1766 w1772 w1783 w1795 w1826 w1839 w1853 w1868 w1887 w1922 w1927 w1941 w1951 w1967 w1979 w1991 w2019 w2034 w2039 w2051 w2063 w2068 w2076 w2084 w2093 w2102 w2107 w2115 w2124 w2142 w2159 w2179 w2190 w2208 w2223 w2240 w2245 w2253 w2261 w2266 w2274 w2281 w2289 w2296 w2306 w2334 w2342 w2349 w2357 w2362 w2370 w2377 w2383 w2392 w2408 w2413 w2420 w2432 w2502 w2514 w2523 w2537 w2546 w2563 w2586 w2603 w2614 w2627 w2652 w2675 w2681 w2697 w2719 w2727 w2733 w2738 w2745 w2755 w2767 w2776 w2781 w2793 w2798 w2808 w2814 w2820 w2825 w2830 w2835 w2845 w2869 w2890 w2895 w2906 w2931 w2958 w2981 w2986 w3001 w3052 w3098 w3143 w3154 w3172 w3192 w3206 w3219 w3227 w3244 w3266 w3290 w3309 w3327 w3345 w3363 w3377 w3391 w3410 w3424 w3439 w3454 w3463 w3468 w3484 w3492 w3499 w3504] -> w89
      tunnel: [_ _ _ _ _ _ _ _ _ _ _ _ _ _ _ _ _ _ _ _ _ _ _ _ _ _ _ _ _ TRUE _ _ _ _ _ _ _ _ _ _ _ _ _ _ _ _ _ _ _ _ _ _ _ _ _ _ _ _ _ _ _ _ _ _ _ _ _ _ _ _ _ _ _ _ _ _ _ _ _ _ _ _ _ _ _ _ _ _ _ _ _ _ _ _ _ _ _ _ _ _ _ _ _ _ _ _ _ _ _ _ _ _ _ _ _ _ _ _ _ _ _ _ _ _ _ _ _ _ _ _ _ _ _ _ _ _ _ _ _ _ _ _ _ _ _ _ _ _ _ _ _ _ _ _ _ _ _ _ _ _ _ _ _ _ _ _ _ _ _ _ _ _ _ _ _ _ _ _ _ _ _ _ _ _ _ _] -> w80
      tunnel: [w98 w512 w520 w527 w533 w555 w568 w586 w615 w642 w668 w679 w751 w760 w797 w819 w850 w887 w916 w942 w947 w996 w1065 w1100 w1119 w1126 w1133 w1161 w1168 w1192 w1196 w1201 w1222 w1252 w1280 w1322 w1327 w1337 w1348 w1378 w1386 w1391 w1399 w1423 w1448 w1472 w1492 w1505 w1550 w1578 w1583 w1609 w1630 w1634 w1639 w1667 w1694 w1713 w1737 w1765 w1770 w1780 w1792 w1810 w1835 w1846 w1864 w1881 w1906 w1925 w1939 w1946 w1965 w1977 w1989 w2008 w2024 w2037 w2050 w2062 w2066 w2072 w2079 w2091 w2100 w2105 w2113 w2123 w2131 w2153 w2162 w2186 w2207 w2218 w2239 w2243 w2248 w2256 w2264 w2273 w2279 w2287 w2294 w2304 w2332 w2340 w2347 w2355 w2360 w2365 w2376 w2381 w2387 w2406 w2411 w2419 w2429 w2500 w2506 w2519 w2536 w2545 w2562 w2577 w2601 w2612 w2623 w2647 w2673 w2679 w2692 w2716 w2725 w2731 w2736 w2743 w2751 w2764 w2774 w2779 w2791 w2796 w2802 w2812 w2818 w2823 w2828 w2833 w2843 w2868 w2889 w2893 w2905 w2930 w2957 w2980 w2984 w3000 w3046 w3095 w3141 w3151 w3168 w3188 w3202 w3216 w3222 w3240 w3262 w3286 w3305 w3323 w3341 w3359 w3373 w3387 w3406 w3420 w3437 w3452 w3462 w3466 w3483 w3491 w3497 w3502] -> w88
      tunnel: 40 ("Timeout") -> [w97 _ _ _ _ _ _ _ _ _ _ _ _ _ _ _ _ _ _ _ _ _ _ _ _ _ _ _ _ _ _ _ _ _ _ _ _ _ _ _ _ _ _ _ _ _ _ _ _ _ _ _ _ _ _ _ _ _ _ _ _ _ _ _ _ _ _ _ _ _ _ _ _ _ _ _ _ _ _ _ _ _ _ _ _ _ _ _ _ _ _ _ _ _ _ _ _ _ _ _ _ _ _ _ _ _ _ _ _ _ _ _ _ _ _ _ _ _ _ _ _ _ _ _ _ _ _ _ _ _ _ _ _ _ _ _ _ _ _ _ _ _ _ _ _ _ _ _ _ _ _ _ _ _ _ _ _ _ _ _ _ _ _ _ _ _ _ _ _ _ _ _ _ _ _ _ _ _ _ _ _ _ _ _ _ _]
      tunnel: w85 -> [_ _ _ _ _ _ _ _ _ _ _ _ _ _ _ _ _ _ _ _ _ _ w1069 _ _ _ _ _ _ _ _ _ _ _ _ _ _ _ _ _ _ _ _ _ _ _ _ _ _ _ _ _ _ _ _ _ _ _ _ _ _ _ _ _ _ _ _ _ _ _ _ _ _ _ _ _ _ _ w2047 w2058 _ _ _ _ _ _ _ _ _ _ _ _ _ _ _ _ _ _ _ _ _ _ _ _ _ _ _ _ _ _ _ _ _ _ _ _ _ _ _ _ _ _ _ _ _ _ _ _ _ _ _ _ _ _ _ _ _ _ _ _ _ _ _ _ _ _ _ _ _ _ _ _ _ _ _ _ _ _ _ _ _ _ _ _ _ _ _ _ _ _ _ _ _ _ _ _ _ _ _ _ _ _ _ _ _ _]
      tunnel: w84 -> [_ _ _ _ _ _ _ _ _ _ _ _ _ _ _ _ _ _ _ _ _ _ w1068 _ _ _ _ _ _ _ _ _ _ _ _ _ _ _ _ _ _ _ _ _ _ _ _ _ _ _ _ _ _ _ _ _ _ _ _ _ _ _ _ _ _ _ _ _ _ _ _ _ _ _ _ _ _ _ w2048 w2057 _ _ _ _ _ _ _ _ _ _ _ _ _ _ _ _ _ _ _ _ _ _ _ _ _ _ _ _ _ _ _ _ _ _ _ _ _ _ _ _ _ _ _ _ _ _ _ _ _ _ _ _ _ _ _ _ _ _ _ _ _ _ _ _ _ _ _ _ _ _ _ _ _ _ _ _ _ _ _ _ _ _ _ _ _ _ _ _ _ _ _ _ _ _ _ _ _ _ _ _ _ _ _ _ _ _]
      tunnel: w83 -> [w96 _ _ _ _ _ _ _ _ _ _ _ _ _ _ _ _ _ _ _ _ _ _ _ _ _ _ _ _ _ _ _ _ _ _ _ _ _ _ _ _ _ _ _ _ _ _ _ _ w1574 _ _ _ _ _ _ _ _ _ _ _ _ _ _ _ _ _ _ _ _ _ _ _ _ _ _ _ _ _ _ _ _ _ _ _ _ _ _ _ _ _ _ _ _ _ _ _ _ _ _ _ _ _ _ _ _ _ _ _ _ _ _ _ _ _ _ _ _ _ _ _ _ _ _ _ _ _ _ _ _ _ _ _ _ _ _ _ _ _ _ _ _ _ _ _ _ _ _ _ _ _ _ _ _ _ _ _ _ _ _ _ _ _ _ _ _ _ _ _ _ _ _ _ _ _ _ _ _ _ _ _ _ _ _ _ _]
      tunnel: w82 -> [w95 w511 w521 w526 w532 w547 w567 w596 w616 w644 w669 w681 w752 w767 w796 w825 w857 w888 w917 w943 w946 w1033 w1070 w1109 w1118 w1125 w1130 w1148 w1167 w1190 w1195 w1209 w1228 w1257 w1277 w1320 w1326 w1336 w1347 w1377 w1385 w1390 w1398 w1422 w1447 w1471 w1491 w1500 w1524 w1579 w1595 w1608 w1617 w1633 w1647 w1676 w1702 w1707 w1752 w1757 w1769 w1776 w1785 w1797 w1828 w1844 w1858 w1878 w1893 w1924 w1940 w1950 w1966 w1978 w1990 w2018 w2021 w2036 w2049 w2056 w2065 w2074 w2082 w2089 w2098 w2104 w2114 w2117 w2129 w2148 w2163 w2182 w2204 w2222 w2238 w2242 w2250 w2258 w2263 w2271 w2278 w2286 w2293 w2303 w2331 w2339 w2346 w2351 w2359 w2368 w2374 w2380 w2389 w2401 w2410 w2415 w2426 w2499 w2504 w2516 w2526 w2539 w2556 w2585 w2600 w2613 w2625 w2649 w2669 w2677 w2690 w2718 w2723 w2729 w2735 w2742 w2753 w2765 w2773 w2778 w2790 w2795 w2806 w2811 w2817 w2822 w2827 w2832 w2842 w2867 w2888 w2892 w2904 w2929 w2956 w2979 w2983 w2999 w3051 w3097 w3138 w3153 w3171 w3191 w3205 w3217 w3226 w3243 w3265 w3289 w3308 w3326 w3344 w3362 w3376 w3390 w3409 w3423 w3438 w3451 w3461 w3465 w3482 w3490 w3496 w3501]
      tunnel: [w94 w511 w521 w526 w532 w547 w567 w596 w616 w644 w669 w681 w752 w767 w796 w825 w857 w888 w917 w943 w946 w1033 w1070 w1109 w1118 w1125 w1130 w1148 w1167 w1190 w1195 w1209 w1228 w1257 w1277 w1320 w1326 w1336 w1347 w1377 w1385 w1390 w1398 w1422 w1447 w1471 w1491 w1500 w1524 w1579 w1595 w1608 w1617 w1633 w1647 w1676 w1702 w1707 w1752 w1757 w1769 w1776 w1785 w1797 w1828 w1844 w1858 w1878 w1893 w1924 w1940 w1950 w1966 w1978 w1990 w2018 w2021 w2036 w2049 w2056 w2065 w2074 w2082 w2089 w2098 w2104 w2114 w2117 w2129 w2148 w2163 w2182 w2204 w2222 w2238 w2242 w2250 w2258 w2263 w2271 w2278 w2286 w2293 w2303 w2331 w2339 w2346 w2351 w2359 w2368 w2374 w2380 w2389 w2401 w2410 w2415 w2426 w2499 w2504 w2516 w2526 w2539 w2556 w2585 w2600 w2613 w2625 w2649 w2669 w2677 w2690 w2718 w2723 w2729 w2735 w2742 w2753 w2765 w2773 w2778 w2790 w2795 w2806 w2811 w2817 w2822 w2827 w2832 w2842 w2867 w2888 w2892 w2904 w2929 w2956 w2979 w2983 w2999 w3051 w3097 w3138 w3153 w3171 w3191 w3205 w3217 w3226 w3243 w3265 w3289 w3308 w3326 w3344 w3362 w3376 w3390 w3409 w3423 w3438 w3451 w3461 w3465 w3482 w3490 w3496 w3501] -> w81
      tunnel: w77 -> [_ _ _ _ _ _ _ _ _ _ _ _ _ _ _ _ _ _ _ _ _ _ w1063 _ _ _ _ _ _ _ _ _ _ _ _ _ _ _ _ _ _ _ _ _ _ _ _ _ _ _ _ _ _ _ _ _ _ _ _ _ _ _ _ _ _ _ _ _ _ _ _ _ _ _ _ _ _ _ w2046 w2055 _ _ _ _ _ _ _ _ _ _ _ _ _ _ _ _ _ _ _ _ _ _ _ _ _ _ _ _ _ _ _ _ _ _ _ _ _ _ _ _ _ _ _ _ _ _ _ _ _ _ _ _ _ _ _ _ _ _ _ _ _ _ _ _ _ _ _ _ _ _ _ _ _ _ _ _ _ _ _ _ _ _ _ _ _ _ _ _ _ _ _ _ _ _ _ _ _ _ _ _ _ _ _ _ _ _]
      frame "", "Event Structure", "Idle" {
        # "executes when the state queue is empty"
        n31 = event shown="[37] <AcqLoop error?>: User Event" {
          selector: w95 -> [_ _ _ _ _ _ _ _ _ _ _ _ _ _ _ _ _ _ _ _ _ _ _ _ _ _ _ _ _ _ _ _ _ _ _ _ _ _ _]
          dyn-events: [_ _ _ _ _ _ _ _ _ _ _ _ _ _ _ _ _ _ _ _ _ _ _ _ _ _ _ _ _ _ _ _ _ _ _ _ _ _ _] -> w94
          timeout: w97 -> [_ _ _ _ _ _ _ _ _ _ _ _ _ _ _ _ _ _ _ _ _ _ _ _ _ _ _ _ _ _ _ _ _ _ _ _ _ _ _]
          tunnel: w102 -> [w122 w141 w149 w153 w157 w165 w171 w179 w187 w197 w204 w233 w253 w273 w293 w297 w304 w327 w341 w355 w369 w374 w377 w383 w390 w397 w403 w409 w415 w422 w435 w446 w458 w465 w469 w473 w480 w494 w510]
          tunnel: [w123 w141 w148 w153 w156 w165 w171 w179 w187 w197 w203 w233 w253 w273 w293 w297 w303 w327 w341 w355 w369 w373 w376 w383 w391 w398 w402 w408 w415 w423 w436 w446 w459 w465 w469 w472 w479 w495 w509] -> w101
          tunnel: w100 -> [w106 w139 w143 w151 w158 w164 w172 w180 w188 w195 w199 w231 w251 w271 w291 w295 w299 w326 w340 w354 w368 w370 w378 w381 w386 w393 w405 w410 w413 w417 w430 w444 w454 w463 w467 w474 w481 w492 w507]
          tunnel: [w121 w140 w144 w152 w159 w163 w170 w178 w186 w196 w205 w232 w252 w272 w292 w296 w305 w324 w328 w351 w366 w372 w379 w382 w387 w394 w406 w411 w414 w421 w434 w445 w455 w464 w468 w475 w482 w496 w508] -> w93
          tunnel: w99 -> [w121 w140 w144 w152 w159 w163 w170 w178 w186 w196 w205 w232 w252 w272 w292 w296 w305 w321 w330 w342 w358 w372 w379 w382 w387 w394 w406 w411 w414 w421 w434 w445 w457 w464 w468 w475 w482 w496 w508]
          tunnel: [w106 w139 w143 w151 w158 w164 w172 w180 w188 w195 w200 w231 w251 w271 w291 w295 w300 w326 w340 w354 w368 w370 w378 w381 w388 w395 w405 w410 w413 w418 w431 w444 w460 w463 w467 w474 w481 w493 w507] -> w98
          tunnel: w96 -> [_ _ _ _ _ _ _ _ _ _ _ _ _ _ _ _ _ _ _ _ _ _ _ _ _ _ _ _ _ _ _ _ _ _ _ _ _ _ _]
          event Timeout {
            # "check system status every 2s"
            n32 = event-data() -> ()  [unwired: 1 in, 1 out]
            n33 = Unbundle By Name(w106) -> ("SysRunning?"=w104:bool, "SlowTimer"=w120:u32, "FastTimer"=w114:u32)
            n34 = Tick Count (ms)() -> (millisecond timer value=w107:u32)
            n35 = Subtract(x=w107, y=w120) -> (x-y=w117:u32)
            n36 = case shown="False" w104 {
              tunnel: ["" "Utility: AquiTimerCheck" ("State(s) in Front (\"\")")] -> w112
              frame False {
                # "if not running, do nothing"
              }
              frame True {
                # "if aquisition is running, check timer"
              }
            }
            n37 = Subtract(x=w107, y=w114) -> (x-y=w115:u32)
            n38 = Greater?(x=w117, y=u32 2000) -> (0:w118:bool)
            n39 = Greater?(x=w115, y=u32 500) -> (0:w105:bool)
            n40 = disable-structure shown="Enabled" {
              disable-tunnel: w105 -> [w128 _]
              disable-tunnel: w104 -> [w127 _]
              disable-tunnel: [w124 "" ("State(s) at Back (\"\")")] -> w103
              frame Disabled {
                n41 = Not(x=w127) -> (.not. x?=w126:bool)
                n42 = And(x=w128, y=w126) -> (x .and. y?=w125:bool)
                n43 = case shown="True" w125 {
                  tunnel: ["" ("Empty String Constant") "TCP: checkSource" ("State(s) in Front (\"\")")] -> w124
                  frame False {
                  }
                  frame True {
                  }
                }
              }
              frame Enabled {
              }
            }
            n44 = case shown="True" w118 {
              tunnel: ["" ("Empty String Constant") "SystemStatus: SlowSysStatusMacro" ("State(s) in Front (\"\")")] -> w110
              frame False {
              }
              frame True {
              }
            }
            n45 = case shown="True" w105 {
              tunnel: ["" ("Empty String Constant") "SystemStatus: FastSysStatusMacro" ("State(s) in Front (\"\")")] -> w108
              frame False {
              }
              frame True {
              }
            }
            n46 = call <vilib>:"Add State(s) to Queue__JKI_lib_State_Machine.vi"("State(s) in Front (\"\")"=w112, "State(s) in (\"\")"="LabJack: checkPedal" ("State(s) in Front (\"\")"), "State(s) at Back (\"\")"=w110) -> ("States Out"=w109:string)  [unwired: 12 in]
            n47 = call <vilib>:"Add State(s) to Queue__JKI_lib_State_Machine.vi"("State(s) in Front (\"\")"=w109, "State(s) in (\"\")"=w108, "State(s) at Back (\"\")"=w103) -> ("States Out"=w113:string)  [unwired: 12 in]
            n48 = call <vilib>:"Add State(s) to Queue__JKI_lib_State_Machine.vi"("State(s) in Front (\"\")"=w113, "State(s) in (\"\")"=w122) -> ("States Out"=w123:string)  [unwired: 13 in]
          }
          event "355nm Laser toggle": Mouse Enter {
            n49 = event-data() -> ()  [unwired: 1 in, 4 out]
            n50 = local write "Help"("Toggle 355nm laser." ("Help")) -> ()
          }
          event "355nm Laser toggle": Value Change {
            # "[Covers: REQ34]"
            n51 = event-data() -> ()  [unwired: 1 in, 6 out]
            n52 = Select(t="LabJack: 355_PWM_Start\nLabJack: AB_Start", s="355nm Laser toggle", f="LabJack: 355_PWM_Stop\nLabJack: AB_Stop") -> (s? t:f=w146:string)
            n53 = call <vilib>:"Add State(s) to Queue__JKI_lib_State_Machine.vi"("State(s) in Front (\"\")"=w146, "State(s) in (\"\")"=w149) -> ("States Out"=w148:string)  [unwired: 13 in]
          }
          event "Aiming beam toggle": Mouse Enter {
            n54 = event-data() -> ()  [unwired: 1 in, 4 out]
            n55 = local write "Help"("Toggle aiming beam laser." ("Help")) -> ()
          }
          event "Aiming beam toggle": Value Change {
            # "[Covers: REQ33]"
            n56 = event-data() -> ()  [unwired: 1 in, 6 out]
            n57 = case shown="True" "Aiming beam toggle" {
              tunnel: ["LabJack: AB_Stop" ("State(s) in Front (\"\")") "LabJack: AB_Start" ("State(s) in Front (\"\")")] -> w155
              frame False {
              }
              frame True {
              }
            }
            n58 = call <vilib>:"Add State(s) to Queue__JKI_lib_State_Machine.vi"("State(s) in Front (\"\")"=w155, "State(s) in (\"\")"=w157) -> ("States Out"=w156:string)  [unwired: 13 in]
          }
          event "Auto gain ch1": Value Change {
            n59 = event-data() -> ("NewVal"=w162:bool)  [unwired: 1 in, 5 out]
            n60 = case shown="True" w162 {
              frame False {
                n61 = local read "V 1"() -> (w166:dbl)
                n62 = call "V1FGV.vi"("action (write)"=enum16{"write", "read"}."write" ("action"), "V1 in"=w166) -> ()  [unwired: 8 in, 2 out]
                n63 = property on="V 1" class="DigNum (strict)"("DisabledEnum"=T11."Enabled" ("Disabled")) -> ()  [unwired: 2 in, 2 out]
              }
              frame True {
                n64 = property on="V 1" class="DigNum (strict)"("DisabledEnum"=T11."Disabled and Grayed Out" ("Disabled")) -> ()  [unwired: 2 in, 2 out]
              }
            }
          }
          event "Auto gain ch2": Value Change {
            n65 = event-data() -> ("NewVal"=w173:bool)  [unwired: 1 in, 5 out]
            n66 = case shown="False" w173 {
              frame False {
                n67 = local read "V 2"() -> (w174:dbl)
                n68 = property on="V 2" class="DigNum (strict)"("DisabledEnum"=T11."Enabled" ("Disabled")) -> ()  [unwired: 2 in, 2 out]
                n69 = call "V2FGV.vi"("action(write)"=enum16{"write", "read"}."write" ("action"), "V2 in"=w174) -> ()  [unwired: 8 in, 2 out]
              }
              frame True {
                n70 = property on="V 2" class="DigNum (strict)"("DisabledEnum"=T11."Disabled and Grayed Out" ("Disabled")) -> ()  [unwired: 2 in, 2 out]
              }
            }
          }
          event "Auto gain ch3": Value Change {
            n71 = event-data() -> ("NewVal"=w181:bool)  [unwired: 1 in, 5 out]
            n72 = case shown="False" w181 {
              frame False {
                n73 = local read "V 3"() -> (w182:dbl)
                n74 = property on="V 3" class="DigNum (strict)"("DisabledEnum"=T11."Enabled" ("Disabled")) -> ()  [unwired: 2 in, 2 out]
                n75 = call "V3FGV.vi"("action(write)"=enum16{"write", "read"}."write" ("action"), "V3 in"=w182) -> ()  [unwired: 8 in, 2 out]
              }
              frame True {
                n76 = property on="V 3" class="DigNum (strict)"("DisabledEnum"=T11."Disabled and Grayed Out" ("Disabled")) -> ()  [unwired: 2 in, 2 out]
              }
            }
          }
          event "Auto gain ch4": Value Change {
            n77 = event-data() -> ("NewVal"=w189:bool)  [unwired: 1 in, 5 out]
            n78 = case shown="False" w189 {
              frame False {
                n79 = local read "V 4"() -> (w190:dbl)
                n80 = property on="V 4" class="DigNum (strict)"("DisabledEnum"=T11."Enabled" ("Disabled")) -> ()  [unwired: 2 in, 2 out]
                n81 = call "V4FGV.vi"("action(write)"=enum16{"write", "read"}."write" ("action"), "V3 in"=w190) -> ()  [unwired: 8 in, 2 out]
              }
              frame True {
                n82 = property on="V 4" class="DigNum (strict)"("DisabledEnum"=T11."Disabled and Grayed Out" ("Disabled")) -> ()  [unwired: 2 in, 2 out]
              }
            }
          }
          event "Background": Mouse Enter {
            n83 = event-data() -> ()  [unwired: 1 in, 4 out]
            n84 = local write "Help"("Click to record a background." ("Help")) -> ()
          }
          event "Background": Value Change {
            n85 = event-data() -> ("NewVal"=w201:bool)  [unwired: 1 in, 5 out]
            n86 = case shown="True" w201 {
              tunnel: ["Utility: SetAllChanManualGain\nQueue: Flash\nUtility: Dewelling >> 2500\nLabJack: 355_PWM_Stop\nLabJack: AB_Stop" "Utility: SetDataClass >> Bg\nUI: Update\nLabJack: 355_PWM_Start\nLabJack: AB_Start\nUtility: SaveDeconChan\nUtility: Dewelling >> 50\nLabJack: SetV\nDigitizer: Start\nUtility: AquiTimerReset\nLED: BreathGreen\nUI: duringBGAcquire"] -> w202
              tunnel: [FALSE TRUE] -> w198
              frame False {
                n87 = local read "Skip Data Save?"() -> (w206:bool)
                n88 = case shown="False" w206 {
                  frame False {
                    n89 = property on="Background" class="Bool (strict)"("BoolText.Text"="Done!" ("Boolean Text.Text")) -> ()  [unwired: 2 in, 2 out]
                  }
                  frame True {
                  }
                }
              }
              frame True {
                # "[Covers: REQ6]"
                n90 = property on="Background" class="Bool (strict)"("BoolText.Text"="Running" ("Boolean Text.Text"), "Colors [4]"=cluster{u32, u32}[] [{6618880, 6618880}, {16711680, 16711680}]) -> ()  [unwired: 2 in, 2 out]
              }
            }
            n91 = Bundle By Name(cluster=w199, "SysRunning?"=w198) -> (w200:T23)
            n92 = call <vilib>:"Add State(s) to Queue__JKI_lib_State_Machine.vi"("State(s) in Front (\"\")"=w202, "State(s) in (\"\")"=w204) -> ("States Out"=w203:string)  [unwired: 13 in]
          }
          event "Channel 1": Cursor Move {
            n93 = event-data() -> ("CursIdx"=w217:i32, "CursLoc"=w229:cluster{"X":dbl, "Y":dbl})  [unwired: 1 in, 7 out]
            n94 = property on="Channel 3" class="WFGraph (strict)"() -> ("CrsrList"=w224:T24)  [unwired: 2 in, 2 out]
            n95 = property on="Channel 4" class="WFGraph (strict)"() -> ("CrsrList"=w216:T24)  [unwired: 2 in, 2 out]
            n96 = property on="Channel 2" class="WFGraph (strict)"() -> ("CrsrList"=w227:T24)  [unwired: 2 in, 2 out]
            n97 = Index Array(array=w224, index=w217) -> (element=w228:T25)
            n98 = Index Array(array=w216, index=w217) -> (element=w219:T25)
            n99 = Unbundle By Name(w229) -> ("X"=w218:dbl)
            n100 = Index Array(array=w227, index=w217) -> (element=w230:T25)
            n101 = Bundle By Name(cluster=w228, "Position.X"=w218) -> (w223:T25)
            n102 = Bundle By Name(cluster=w219, "Position.X"=w218) -> (w215:T25)
            n103 = Bundle By Name(cluster=w230, "Position.X"=w218) -> (w226:T25)
            n104 = control-ref of="Channel 1"() -> (w220:refnum<vi>)
            n105 = Replace Array Subset(array=w224, new element=w223, index=w217) -> (w222:T24)
            n106 = Replace Array Subset(array=w216, new element=w215, index=w217) -> (w214:T24)
            n107 = Replace Array Subset(array=w227, new element=w226, index=w217) -> (w225:T24)
            n108 = property on="Channel 3" class="WFGraph (strict)"("CrsrList"=w222) -> (error out=w221:errorcluster)  [unwired: 2 in, 1 out]
            n109 = property on="Channel 4" class="WFGraph (strict)"("CrsrList"=w214) -> ()  [unwired: 2 in, 2 out]
            n110 = property on="Channel 2" class="WFGraph (strict)"("CrsrList"=w225) -> ()  [unwired: 2 in, 2 out]
            n111 = call "UpdateCurserIdx(SubVI).vi"("error in (no error)"=w221, "WaveformGraph in"=w220) -> ()  [unwired: 9 in, 1 out]
          }
          event "Channel 2": Cursor Move {
            n112 = event-data() -> ("CursIdx"=w236:i32, "CursLoc"=w250:cluster{"X":dbl, "Y":dbl})  [unwired: 1 in, 7 out]
            n113 = Unbundle By Name(w250) -> ("X"=w238:dbl)
            n114 = property on="Channel 1" class="WFGraph (strict)"() -> ("CrsrList"=w244:T24)  [unwired: 2 in, 2 out]
            n115 = property on="Channel 3" class="WFGraph (strict)"() -> ("CrsrList"=w246:T24)  [unwired: 2 in, 2 out]
            n116 = property on="Channel 4" class="WFGraph (strict)"() -> ("CrsrList"=w237:T24)  [unwired: 2 in, 2 out]
            n117 = Index Array(array=w244, index=w236) -> (element=w249:T25)
            n118 = Index Array(array=w246, index=w236) -> (element=w248:T25)
            n119 = Index Array(array=w237, index=w236) -> (element=w239:T25)
            n120 = Bundle By Name(cluster=w239, "Position.X"=w238) -> (w235:T25)
            n121 = Bundle By Name(cluster=w249, "Position.X"=w238) -> (w247:T25)
            n122 = Bundle By Name(cluster=w248, "Position.X"=w238) -> (w245:T25)
            n123 = Replace Array Subset(array=w244, new element=w247, index=w236) -> (w243:T24)
            n124 = Replace Array Subset(array=w246, new element=w245, index=w236) -> (w242:T24)
            n125 = Replace Array Subset(array=w237, new element=w235, index=w236) -> (w234:T24)
            n126 = control-ref of="Channel 1"() -> (w241:refnum<vi>)
            n127 = property on="Channel 1" class="WFGraph (strict)"("CrsrList"=w243) -> ()  [unwired: 2 in, 2 out]
            n128 = property on="Channel 3" class="WFGraph (strict)"("CrsrList"=w242) -> (error out=w240:errorcluster)  [unwired: 2 in, 1 out]
            n129 = property on="Channel 4" class="WFGraph (strict)"("CrsrList"=w234) -> ()  [unwired: 2 in, 2 out]
            n130 = call "UpdateCurserIdx(SubVI).vi"("error in (no error)"=w240, "WaveformGraph in"=w241) -> ()  [unwired: 9 in, 1 out]
          }
          event "Channel 3": Cursor Move {
            n131 = event-data() -> ("CursIdx"=w256:i32, "CursLoc"=w270:cluster{"X":dbl, "Y":dbl})  [unwired: 1 in, 7 out]
            n132 = Unbundle By Name(w270) -> ("X"=w258:dbl)
            n133 = property on="Channel 4" class="WFGraph (strict)"() -> ("CrsrList"=w257:T24)  [unwired: 2 in, 2 out]
            n134 = property on="Channel 1" class="WFGraph (strict)"() -> ("CrsrList"=w267:T24)  [unwired: 2 in, 2 out]
            n135 = property on="Channel 2" class="WFGraph (strict)"() -> ("CrsrList"=w265:T24)  [unwired: 2 in, 2 out]
            n136 = Index Array(array=w257, index=w256) -> (element=w259:T25)
            n137 = Index Array(array=w267, index=w256) -> (element=w269:T25)
            n138 = Index Array(array=w265, index=w256) -> (element=w268:T25)
            n139 = Bundle By Name(cluster=w259, "Position.X"=w258) -> (w255:T25)
            n140 = Bundle By Name(cluster=w269, "Position.X"=w258) -> (w266:T25)
            n141 = Bundle By Name(cluster=w268, "Position.X"=w258) -> (w264:T25)
            n142 = Replace Array Subset(array=w257, new element=w255, index=w256) -> (w254:T24)
            n143 = Replace Array Subset(array=w267, new element=w266, index=w256) -> (w263:T24)
            n144 = Replace Array Subset(array=w265, new element=w264, index=w256) -> (w262:T24)
            n145 = control-ref of="Channel 1"() -> (w260:refnum<vi>)
            n146 = property on="Channel 4" class="WFGraph (strict)"("CrsrList"=w254) -> ()  [unwired: 2 in, 2 out]
            n147 = property on="Channel 1" class="WFGraph (strict)"("CrsrList"=w263) -> ()  [unwired: 2 in, 2 out]
            n148 = property on="Channel 2" class="WFGraph (strict)"("CrsrList"=w262) -> (error out=w261:errorcluster)  [unwired: 2 in, 1 out]
            n149 = call "UpdateCurserIdx(SubVI).vi"("error in (no error)"=w261, "WaveformGraph in"=w260) -> ()  [unwired: 9 in, 1 out]
          }
          event "Channel 4": Cursor Move {
            n150 = event-data() -> ("CursIdx"=w278:i32, "CursLoc"=w290:cluster{"X":dbl, "Y":dbl})  [unwired: 1 in, 7 out]
            n151 = Unbundle By Name(w290) -> ("X"=w276:dbl)
            n152 = property on="Channel 1" class="WFGraph (strict)"() -> ("CrsrList"=w288:T24)  [unwired: 2 in, 2 out]
            n153 = property on="Channel 2" class="WFGraph (strict)"() -> ("CrsrList"=w284:T24)  [unwired: 2 in, 2 out]
            n154 = property on="Channel 3" class="WFGraph (strict)"() -> ("CrsrList"=w279:T24)  [unwired: 2 in, 2 out]
            n155 = Index Array(array=w288, index=w278) -> (element=w289:T25)
            n156 = Index Array(array=w284, index=w278) -> (element=w285:T25)
            n157 = Index Array(array=w279, index=w278) -> (element=w281:T25)
            n158 = Bundle By Name(cluster=w289, "Position.X"=w276) -> (w287:T25)
            n159 = Bundle By Name(cluster=w285, "Position.X"=w276) -> (w283:T25)
            n160 = Bundle By Name(cluster=w281, "Position.X"=w276) -> (w280:T25)
            n161 = Replace Array Subset(array=w288, new element=w287, index=w278) -> (w286:T24)
            n162 = Replace Array Subset(array=w284, new element=w283, index=w278) -> (w282:T24)
            n163 = Replace Array Subset(array=w279, new element=w280, index=w278) -> (w277:T24)
            n164 = control-ref of="Channel 1"() -> (w274:refnum<vi>)
            n165 = call "UpdateCurserIdx(SubVI).vi"() -> ()  [unwired: 11 in, 1 out]
            n166 = call "UpdateCurserIdx(SubVI).vi"() -> ()  [unwired: 11 in, 1 out]
            n167 = property on="Channel 1" class="WFGraph (strict)"("CrsrList"=w286) -> ()  [unwired: 2 in, 2 out]
            n168 = property on="Channel 2" class="WFGraph (strict)"("CrsrList"=w282) -> ()  [unwired: 2 in, 2 out]
            n169 = property on="Channel 3" class="WFGraph (strict)"("CrsrList"=w277) -> (error out=w275:errorcluster)  [unwired: 2 in, 1 out]
            n170 = call "UpdateCurserIdx(SubVI).vi"("error in (no error)"=w275, "WaveformGraph in"=w274) -> ()  [unwired: 9 in, 1 out]
          }
          event "Cali&iRF alignment": Mouse Enter {
            n171 = event-data() -> ()  [unwired: 1 in, 4 out]
            n172 = local write "Help"("Click to run system intensity calibration and irf alignment" ("Help")) -> ()
          }
          event "Cali&iRF alignment": Value Change {
            n173 = event-data() -> ("NewVal"=w301:bool)  [unwired: 1 in, 5 out]
            n174 = case shown="False" w301 {
              tunnel: ["Utility: SetAllChanManualGain\nQueue: Flash\nUtility: Dewelling >> 2500\nLabJack: 355_PWM_Stop\nLabJack: AB_Stop" "Utility: SetDataClass >> Cali\nUI: Update\nUtility: SaveDeconChan\nLabJack: 355_PWM_Start\nLabJack: AB_Start\nLabJack: SetV\nDigitizer: Start\nUtility: AquiTimerReset\nLED: BreathGreen\nUI: duringIRFAlign"] -> w302
              tunnel: [FALSE TRUE] -> w298
              frame False {
                n175 = local read "Skip Data Save?"() -> (w306:bool)
                n176 = case shown="False" w306 {
                  frame False {
                    n177 = property on="Cali&iRF alignment" class="Bool (strict)"("BoolText.Text"="Done!" ("Boolean Text.Text")) -> ()  [unwired: 2 in, 2 out]
                  }
                  frame True {
                  }
                }
              }
              frame True {
                n178 = property on="Cali&iRF alignment" class="Bool (strict)"("BoolText.Text"="Running" ("Boolean Text.Text"), "Colors [4]"=cluster{u32, u32}[] [{6618880, 6618880}, {16711680, 16711680}]) -> ()  [unwired: 2 in, 2 out]
              }
            }
            n179 = Bundle By Name(cluster=w299, "SysRunning?"=w298) -> (w300:T23)
            n180 = call <vilib>:"Add State(s) to Queue__JKI_lib_State_Machine.vi"("State(s) in Front (\"\")"=w302, "State(s) in (\"\")"=w304) -> ("States Out"=w303:string)  [unwired: 13 in]
          }
          event "V 1": Value Change {
            n181 = event-data() -> ()  [unwired: 1 in, 6 out]
            n182 = call "LabJack_FGV.vi"("Operation(Read)"=enum16{"Write", "Read"}."Read" ("Operation"), "error in (no error)"=w321) -> ("error out"=w318:errorcluster, "Read data"=w319:i32)  [unwired: 8 in]
            n183 = global read "GlobalVariables.vi" "Ch1 LJ pin"() -> (w317:string)
            n184 = call "LJM_eWriteName.vi"("Handle In"=w319, "Name"=w317, "Value"="V 1", "error in"=w318) -> ("error out"=w315:errorcluster)  [unwired: 10 in, 1 out]
            n185 = call "V1FGV.vi"("Error In"=w315, "action (write)"=enum16{"write", "read"}."write" ("action"), "V1 in"="V 1") -> ("Error Out"=w314:errorcluster)  [unwired: 7 in, 1 out]
            n186 = call "CtrlVtoGain.vi"("error in (no error)"=w314, "CtrlV(V)"="V 1", "Channel"=enum16{"Ch1", "Ch2", "Ch3"}."Ch1" ("Enum")) -> ("error out"=w324:errorcluster, "Gain"=w323:dbl)  [unwired: 7 in]
            n187 = local write "Gain1"(w323) -> ()
          }
          event "V 2": Value Change {
            n188 = event-data() -> ()  [unwired: 1 in, 6 out]
            n189 = call "LabJack_FGV.vi"("Operation(Read)"=enum16{"Write", "Read"}."Read" ("Operation"), "error in (no error)"=w330) -> ("error out"=w335:errorcluster, "Read data"=w336:i32)  [unwired: 8 in]
            n190 = global read "GlobalVariables.vi" "Ch2 LJ pin"() -> (w334:string)
            n191 = call "LJM_eWriteName.vi"("Handle In"=w336, "Name"=w334, "Value"="V 2", "error in"=w335) -> ("error out"=w333:errorcluster)  [unwired: 10 in, 1 out]
            n192 = call "V2FGV.vi"("Error In"=w333, "action(write)"=enum16{"write", "read"}."write" ("action"), "V2 in"="V 2") -> ("Error Out"=w332:errorcluster)  [unwired: 7 in, 1 out]
            n193 = call "CtrlVtoGain.vi"("error in (no error)"=w332, "CtrlV(V)"="V 2", "Channel"=enum16{"Ch1", "Ch2", "Ch3"}."Ch2" ("Enum")) -> ("error out"=w328:errorcluster, "Gain"=w329:dbl)  [unwired: 7 in]
            n194 = local write "Gain2"(w329) -> ()
          }
          event "V 3": Value Change {
            n195 = event-data() -> ()  [unwired: 1 in, 6 out]
            n196 = call "LabJack_FGV.vi"("Operation(Read)"=enum16{"Write", "Read"}."Read" ("Operation"), "error in (no error)"=w342) -> ("error out"=w347:errorcluster, "Read data"=w348:i32)  [unwired: 8 in]
            n197 = global read "GlobalVariables.vi" "Ch3 LJ pin"() -> (w346:string)
            n198 = call "LJM_eWriteName.vi"("Handle In"=w348, "Name"=w346, "Value"="V 3", "error in"=w347) -> ("error out"=w344:errorcluster)  [unwired: 10 in, 1 out]
            n199 = call "V3FGV.vi"("Error In"=w344, "action(write)"=enum16{"write", "read"}."write" ("action"), "V3 in"="V 3") -> ("Error Out"=w343:errorcluster)  [unwired: 7 in, 1 out]
            n200 = call "CtrlVtoGain.vi"("error in (no error)"=w343, "CtrlV(V)"="V 3", "Channel"=enum16{"Ch1", "Ch2", "Ch3"}."Ch3" ("Enum")) -> ("error out"=w351:errorcluster, "Gain"=w350:dbl)  [unwired: 7 in]
            n201 = local write "Gain3"(w350) -> ()
          }
          event "V 4": Value Change {
            n202 = event-data() -> ()  [unwired: 1 in, 6 out]
            n203 = call "LabJack_FGV.vi"("Operation(Read)"=enum16{"Write", "Read"}."Read" ("Operation"), "error in (no error)"=w358) -> ("error out"=w362:errorcluster, "Read data"=w363:i32)  [unwired: 8 in]
            n204 = global read "GlobalVariables.vi" "Ch4 LJ pin"() -> (w361:string)
            n205 = call "LJM_eWriteName.vi"("Handle In"=w363, "Name"=w361, "Value"="V 4", "error in"=w362) -> ("error out"=w360:errorcluster)  [unwired: 10 in, 1 out]
            n206 = call "V4FGV.vi"("Error In"=w360, "action(write)"=enum16{"write", "read"}."write" ("action"), "V3 in"="V 4") -> ("Error Out"=w359:errorcluster)  [unwired: 7 in, 1 out]
            n207 = call "CtrlVtoGain.vi"("error in (no error)"=w359, "CtrlV(V)"="V 4", "Channel"=enum16{"Ch1", "Ch2", "Ch3", "Ch4"}."Ch4") -> ("error out"=w366:errorcluster, "Gain"=w365:dbl)  [unwired: 7 in]
            n208 = local write "Gain4"(w365) -> ()
          }
          event "Quit": Value Change {
            # "Exit Button Value Change (pressed) Event\n(when pressed.  quite)"
            n209 = event-data() -> ()  [unwired: 1 in, 1 out]
            n210 = call <vilib>:"Add State(s) to Queue__JKI_lib_State_Machine.vi"("State(s) in Front (\"\")"="LED: Off\nMacro: Exit", "State(s) in (\"\")"=w374) -> ("States Out"=w373:string)  [unwired: 13 in]
          }
          event "Show BG": Value Change {
            n211 = event-data() -> ()  [unwired: 1 in, 6 out]
            n212 = call <vilib>:"Add State(s) to Queue__JKI_lib_State_Machine.vi"("State(s) in Front (\"\")"="Data: showBG" ("State(s) in Front (\"\")"), "State(s) in (\"\")"=w377) -> ("States Out"=w376:string)  [unwired: 13 in]
          }
          event "StartButton": Mouse Enter {
            n213 = event-data() -> ()  [unwired: 1 in, 4 out]
            n214 = local write "Help"("Press to start aquisition." ("Help")) -> ()
          }
          event "StartButton": Value Change {
            # "[Covers: REQ32]"
            # "start PWM before acquisition"
            # "Initialize both digitizer aquisition and\n send user event to trigger aquisition loop"
            n215 = event-data() -> ()  [unwired: 1 in, 6 out]
            n216 = local write "StartButton"(FALSE ("StartButton")) -> ()
            n217 = Bundle By Name(cluster=w386, "SysRunning?"=TRUE) -> (w388:T23)
            n218 = call <vilib>:"Add State(s) to Queue__JKI_lib_State_Machine.vi"("State(s) in Front (\"\")"="TCP: stopCam\nUtility: SetDataClass >> Data\nQueue: Flash\nUI: Update\nUtility: StartBeep\nLabJack: 355_PWM_Start\nLabJack: AB_Start\nLabJack: SetV\nDigitizer: Start\nUtility: AquiTimerReset\nUI: DuringAquisition\nLED: BreathGreen\nTCP: sendRunNum\nTCP: sendVideoSource\nTCP: sendChannel\nTCP: startRun", "State(s) in (\"\")"=w390) -> ("States Out"=w391:string)  [unwired: 13 in]
          }
          event User Event {
            # "[Covers: REQ32]"
            # "start PWM before acquisition"
            # "Initialize both digitizer aquisition and\n send user event to trigger aquisition loop"
            n219 = event-data() -> ()  [unwired: 1 in, 5 out]
            n220 = Bundle By Name(cluster=w393, "SysRunning?"=TRUE) -> (w395:T23)
            n221 = call <vilib>:"Add State(s) to Queue__JKI_lib_State_Machine.vi"("State(s) in Front (\"\")"="TCP: stopCam\nUtility: SetDataClass >> Data\nQueue: Flash\nUI: Update\nUtility: StartBeep\nLabJack: 355_PWM_Start\nLabJack: AB_Start\nLabJack: SetV\nDigitizer: Start\nUtility: AquiTimerReset\nUI: DuringAquisition\nLED: BreathGreen\nTCP: sendRunNum\nTCP: sendVideoSource\nTCP: sendChannel\nTCP: startRun", "State(s) in (\"\")"=w397) -> ("States Out"=w398:string)  [unwired: 13 in]
          }
          event "Video Display": Value Change {
            n222 = event-data() -> ("NewVal"=w404:bool)  [unwired: 1 in, 5 out]
            n223 = Select(t="TCP: startCam", s=w404, f="TCP: stopCam") -> (s? t:f=w401:string)
            n224 = call <vilib>:"Add State(s) to Queue__JKI_lib_State_Machine.vi"("State(s) in (\"\")"=w403, "State(s) at Back (\"\")"=w401) -> ("States Out"=w402:string)  [unwired: 13 in]
          }
          event "Video Source": Value Change {
            n225 = event-data() -> ()  [unwired: 1 in, 6 out]
            n226 = call <vilib>:"Add State(s) to Queue__JKI_lib_State_Machine.vi"("State(s) in Front (\"\")"="TCP: sendVideoSource" ("State(s) in Front (\"\")"), "State(s) in (\"\")"=w409) -> ("States Out"=w408:string)  [unwired: 13 in]
          }
          event "StopButton": Mouse Enter {
            n227 = event-data() -> ()  [unwired: 1 in, 4 out]
            n228 = local write "Help"("Press to stop data aquisition." ("Help")) -> ()
          }
          event "StopButton": Value Change {
            # "if system is running, send stop command, if not do nothing."
            # "stop aquisition\nupdate UI"
            n229 = event-data() -> ()  [unwired: 1 in, 6 out]
            n230 = Unbundle By Name(w417) -> ("SysRunning?"=w419:bool)
            n231 = case shown="True" w419 {
              tunnel: ["" ("Empty String Constant") "LabJack: AB_Stop\nLabJack: 355_PWM_Stop\n/*Digitizer: Abort"] -> w420
              tunnel: w417 -> [w424 w428]
              tunnel: [w424 w427] -> w418
              frame False {
              }
              frame True {
                n232 = Bundle By Name(cluster=w428, "SysRunning?"=FALSE) -> (w427:T23)
              }
            }
            n233 = call <vilib>:"Add State(s) to Queue__JKI_lib_State_Machine.vi"("State(s) in Front (\"\")"=w420, "State(s) in (\"\")"=w422) -> ("States Out"=w423:string)  [unwired: 13 in]
            n234 = local write "StopButton"(FALSE ("StopButton")) -> ()
          }
          event User Event {
            # "if system is running, send stop command, if not do nothing."
            # "stop aquisition\nupdate UI"
            n235 = event-data() -> ()  [unwired: 1 in, 5 out]
            n236 = Unbundle By Name(w430) -> ("SysRunning?"=w432:bool)
            n237 = case shown="True" w432 {
              tunnel: ["" ("Empty String Constant") "LabJack: AB_Stop\nLabJack: 355_PWM_Stop\n/*Digitizer: Abort"] -> w433
              tunnel: w430 -> [w437 w441]
              tunnel: [w437 w440] -> w431
              frame False {
              }
              frame True {
                n238 = Bundle By Name(cluster=w441, "SysRunning?"=FALSE) -> (w440:T23)
              }
            }
            n239 = call <vilib>:"Add State(s) to Queue__JKI_lib_State_Machine.vi"("State(s) in Front (\"\")"=w433, "State(s) in (\"\")"=w435) -> ("States Out"=w436:string)  [unwired: 13 in]
          }
          event "Sys Reconfig": Mouse Enter {
            n240 = event-data() -> ()  [unwired: 1 in, 4 out]
            n241 = local write "Help"("Click to reconfig digitizer settings." ("Help")) -> ()
          }
          event "Sys Reconfig": Value Change {
            # "everytime the user change data aquisition setting, need to reinitilize decon engine and realign iRF.\ncheck whether data length has changed, if changed, reinitialize Decon engine\nreset BG ready, need a new BG"
            # "update DAQ FGV"
            n242 = event-data() -> ()  [unwired: 1 in, 6 out]
            n243 = call "SystemConfigEditorV6.vi"("error in"=w457) -> ("error out"=w456:errorcluster, "FLImDAQ out"=w451:T5)  [unwired: 1 in]
            n244 = Unbundle By Name(w454) -> ("FLImDAQ.min record length"=w453:i32)
            n245 = Unbundle By Name(w451) -> ("min record length"=w452:i32)
            n246 = call "FLImDAQ_FGV.vi"("error in (no error)"=w456, "Operation (Read)"=enum16{"Write", "Read"}."Write" ("Operation"), "Write data"=w451) -> ("error out"=w455:errorcluster, "Read data"=w450:T5)  [unwired: 7 in]
            n247 = Equal?(x=w453, y=w452) -> (x = y?=w449:bool)
            n248 = case shown="False" w449 {
              tunnel: ["UI: Cursor Set >> Busy\nDigitizer: Config\nDeconEngine: InitializeCh1\nDeconEngine: InitializeCh2\nDeconEngine: InitializeCh3\nUI: CaliAndiRFNotReady\n/*UI iRF not ready\nUI: Update\nUI: Cursor Set >> Idle" "UI: Cursor Set >> Busy\nDigitizer: Config\nUI: Update\nUI: Cursor Set >> Idle"] -> w448
              frame False {
              }
              frame True {
              }
            }
            n249 = Bundle By Name(cluster=w454, "FLImDAQ"=w450) -> (w460:T23)
            n250 = call <vilib>:"Add State(s) to Queue__JKI_lib_State_Machine.vi"("State(s) in Front (\"\")"=w448, "State(s) in (\"\")"=w458) -> ("States Out"=w459:string)  [unwired: 13 in]
          }
          event "System Hardware Connection Status", "StartButton", "StopButton", "355nm Laser toggle", "Aiming beam toggle", "Cali&iRF alignment", "Background", "Sys Reconfig": Mouse Leave {
            n251 = event-data() -> ()  [unwired: 1 in, 4 out]
            n252 = invoke on="Help" class="Str" method="Reinit To Default"() -> ()  [unwired: 3 in, 3 out]
          }
          event "System Hardware Connection Status.Digitizer": Mouse Enter {
            n253 = event-data() -> ()  [unwired: 1 in, 4 out]
            n254 = local write "Help"("Status of hardware connections. TCP/IP is optional." ("Help")) -> ()
          }
          event "TCP Connect": Value Change {
            n255 = event-data() -> ("NewVal"=w470:bool)  [unwired: 1 in, 5 out]
            n256 = case shown="True" w470 {
              tunnel: ["TCP: Close\nUI: Update" ("State(s) in Front (\"\")") "TCP: SendSettingMacro\nUI: Update" ("State(s) in Front (\"\")")] -> w471
              frame False {
              }
              frame True {
              }
            }
            n257 = call <vilib>:"Add State(s) to Queue__JKI_lib_State_Machine.vi"("State(s) in Front (\"\")"=w471, "State(s) in (\"\")"=w473) -> ("States Out"=w472:string)  [unwired: 13 in]
          }
          event "488nm Power": Value Change {
            n258 = event-data() -> ()  [unwired: 1 in, 6 out]
            n259 = call <vilib>:"Add State(s) to Queue__JKI_lib_State_Machine.vi"("State(s) in Front (\"\")"="AimingBeam: Set Current" ("State(s) in Front (\"\")"), "State(s) in (\"\")"=w480) -> ("States Out"=w479:string)  [unwired: 13 in]
          }
          event User Event {
            # "if aquisition loop is error out. Stop digitizer, update front panel indicator, stop both laser and \nOption 1: parse and save data\nOption 2: Flash queue if scout run. [Covers: REQ23]"
            n260 = event-data() -> ()  [unwired: 1 in, 5 out]
            n261 = case shown="\"BG\"" "Data Class" {
              tunnel: [w500 "UI: Cursor Set >> Busy\nUtility: SetAllChanAutoGain\nUtility: RestoreDeConChan\nData: parseRunData\nData: irfAlignment\nUI: Cursor Set >> Idle" w504] -> w490
              frame "Data", Default {
                n262 = local read "Video Display"() -> (w502:bool)
                n263 = Select(t="TCP: startCam", s=w502, f="") -> (s? t:f=w498:string)
                n264 = call <vilib>:"Add State(s) to Queue__JKI_lib_State_Machine.vi"("State(s) in Front (\"\")"="UI: Cursor Set >> Busy\nData: parseRunData\nData: saveRunData\nUI: Cursor Set>>Idle" ("State(s) in Front (\"\")"), "State(s) in (\"\")"=w498) -> ("States Out"=w500:string)  [unwired: 13 in]
              }
              frame "Cali" {
              }
              frame "BG" {
                w504 = "UI: Cursor Set >> Busy\nUtility: SetAllChanAutoGain\nUtility: RestoreDeConChan\nData: parseRunData\nData: saveBGtoFGV\nData: saveBGtoFile\nData: saveDeConBGtoFile\nUI: Cursor Set >> Idle\nData: showBG\nRun: BGIncrement"  # UI: Cursor Set >> Busy Utility: SetAllChanAutoGain Utility: RestoreDeConChan Data: parseRunData Data: saveBGtoFGV Data: saveBGtoFile Data: saveDeConBGtoFile UI: Cursor Set >> Idle Data: showBG Run: BGIncrement
              }
            }
            n265 = Bundle By Name(cluster=w492, "SysRunning?"=FALSE) -> (w493:T23)
            n266 = Select(t="" ("State(s) in Front (\"\")"), s="Skip Data Save?", f=w490) -> (s? t:f=w487:string)
            n267 = call <vilib>:"Add State(s) to Queue__JKI_lib_State_Machine.vi"("State(s) in Front (\"\")"="TCP: stopRun\nUI: Update\nLabJack: AB_Stop\nLabJack: 355_PWM_Stop\nDigitizer: Abort\nLabJack: ZeroV\nUtility: EndBeep\nLED: BreathOff" ("State(s) in Front (\"\")"), "State(s) in (\"\")"=w487, "State(s) at Back (\"\")"="Macro: SysReadyForAq\nUI: Update" ("State(s) in Front (\"\")")) -> ("States Out"=w485:string)  [unwired: 12 in]
            n268 = call <vilib>:"Add State(s) to Queue__JKI_lib_State_Machine.vi"("State(s) in Front (\"\")"=w485, "State(s) in (\"\")"=w494) -> ("States Out"=w495:string)  [unwired: 13 in]
          }
          event Panel Close? {
            # "Discard the event because we'll close the front panel ourselves in Macro: Exit"
            # "Close Panel button (pressed) Event\n(this executes Macro: Exit to terminate the VI)"
            n269 = event-data() -> ()  [unwired: 1 in, 1 out]
            n270 = event-data ("Event Filter Node")("Discard?"=TRUE) -> ()  [unwired: 1 in, 1 out]
            n271 = call <vilib>:"Add State(s) to Queue__JKI_lib_State_Machine.vi"("State(s) in Front (\"\")"="Macro: Exit", "State(s) in (\"\")"=w510) -> ("States Out"=w509:string)  [unwired: 13 in]
          }
        }
      }
      frame "---------- Macro ----------" {
        # "Do not put any code in this frame.\n(It is a separator no-op. You can make a copy of this frame to create a new Macro frame)"
        n272 = call <vilib>:"Add State(s) to Queue__JKI_lib_State_Machine.vi"("State(s) in (\"\")"=w515) -> ("States Out"=w514:string)  [unwired: 14 in]
      }
      frame "Macro: Initialize" {
        # "load Labjack setting 1st as it contaisn laser pin infortmation"
        # "start laser 1st, need 7.5s for laser to get ready"
        # "Initialization Macro\n(This is called once, when the VI starts)"
        n273 = call <vilib>:"Add State(s) to Queue__JKI_lib_State_Machine.vi"("State(s) in Front (\"\")"="UI: showDisclaimer\nUI: Cursor Set >> Busy\nData: Initialize\nInitialize Core Data\nUI: Initialize\nUI: Front Panel State >> Open\nMacro: LoadSysConfig\nTCP: InitializeNew\nTCP: checkSource\nUI: Update\nLabJack: Open\nLabJack: SetDefaultSub\nLED: OpenVIRef\nLED: BreathOrange\nUI: Update\n355 Laser: CheckControllerStatus\n355 Laser: Laser enable\n355 Laser: Dewelling>>500\n355 Laser: CheckControllerStatus\nUI: Update\nLabJack: 355_PWM_Config\nLabJack: AB_PWM_Config\nUI: Update", "State(s) in (\"\")"="Digitizer: Initialize\nDigitizer: Config\nUI: Update\nAimingBeam: Initialize\nAimingBeam: Set APC Status>>Disable\nAimingBeam: Set ACC Status>>Enable\nAimingBeam: Set Current\nUI: Update\n355 Laser: Check Dewelling\nUI: Cursor Set >> Idle\nCase: GetID\nUI: Update\nTCP: SendSettingMacro\nCase: CreatFileStruct\nUI: Update\nData: loadLastUseMacro\nDeconEngine: InitDotNet\nDeconEngine: loadIRF\nDeconEngine: Warmup\nClassifier: Init\nGraph: SetXMultiplier\nGraph: AddCursors\nAPD: Initialize\nAPD: LoadFromSerial\nAPD: UpdateCtrlVLimit\nAPD: GetGainLimits\nPID: loadPID\nLED: BreathOff\nMacro: SysReadyForAq") -> ("States Out"=w516:string)  [unwired: 13 in]
        n274 = call <vilib>:"Add State(s) to Queue__JKI_lib_State_Machine.vi"("State(s) in Front (\"\")"=w516, "State(s) in (\"\")"=w524) -> ("States Out"=w523:string)  [unwired: 13 in]
        "Help" <- "Hover over controls to see help!" ("Help")
      }
      frame "Macro: LoadSysConfig" {
        # "System configuration Macro. [Covers: REQ15]\n(Load configurations for different component of the system)"
        n275 = call <vilib>:"Add State(s) to Queue__JKI_lib_State_Machine.vi"("State(s) in Front (\"\")"="SysConfig: Load Sys Config\nSysConfig: Load Digitizer Setting\nSysConfig: Load AB setting\nSysConfig: Load LJ Pinout\nSysConfig: Load 355 PWM\nSysConfig: LoadAPDSerialNumber\nSysConfig: LoadABVideoSetting\nSysConfig: LoadCursorLocation", "State(s) in (\"\")"=w530) -> ("States Out"=w529:string)  [unwired: 13 in]
      }
      frame "Macro: SysReadyForAq" {
        # "Macro for system ready\n(It is a separator no-op. You can make a copy of this frame to create a new Macro frame)"
        n276 = call <vilib>:"Add State(s) to Queue__JKI_lib_State_Machine.vi"("State(s) in Front (\"\")"="UI: ReadyForAquisition\nLED: Green" ("State(s) in Front (\"\")"), "State(s) in (\"\")"=w536) -> ("States Out"=w535:string)  [unwired: 13 in]
      }
      frame "Macro: Exit" {
        # "close LJ last"
        # "check whether hardware is initilized, if so close, if not do nothing"
        # "Exit Macro, close all hardware\n(This is called once, when the VI exits)"
        n277 = Unbundle By Name(w555) -> ("System Status.Digitizer"=w551:bool, "System Status.Aiming Beam"=w550:bool, "System Status.355 Laser"=w549:bool, "System Status.Labjack"=w540:bool, "Core.Close Panel on Exit?"=w544:bool)
        n278 = case shown="True" w551 {
          tunnel: ["" ("Empty String Constant") "Digitizer: Close"] -> w546
          frame False {
          }
          frame True {
          }
        }
        n279 = case shown="True" w540 {
          tunnel: ["" ("Empty String Constant") "LabJack: SetDefaultAndClose"] -> w537
          frame False {
          }
          frame True {
          }
        }
        n280 = case shown="True" w550 {
          tunnel: ["" ("Empty String Constant") "AimingBeam: Set ACC Status >> Disable\nAimingBeam: Close"] -> w539
          frame False {
          }
          frame True {
          }
        }
        n281 = case shown="True" w549 {
          tunnel: ["" ("Empty String Constant") "355 Laser: Close\n355 Laser: CheckControllerStatus"] -> w538
          frame False {
          }
          frame True {
          }
        }
        n282 = Select(t="UI: Front Panel State >> Close", s=w544, f="" ("Empty String Constant")) -> (s? t:f=w541:string)
        n283 = call <vilib>:"Add State(s) to Queue__JKI_lib_State_Machine.vi"("State(s) in Front (\"\")"="TCP: Close\nDeconEngine: CloseNetRef\nClassifier: Close", "State(s) in (\"\")"=w546, "State(s) at Back (\"\")"=w539) -> ("States Out"=w548:string)  [unwired: 12 in]
        n284 = call <vilib>:"Add State(s) to Queue__JKI_lib_State_Machine.vi"("State(s) in Front (\"\")"=w548, "State(s) in (\"\")"=w538, "State(s) at Back (\"\")"=w537) -> ("States Out"=w543:string)  [unwired: 12 in]
        n285 = call <vilib>:"Add State(s) to Queue__JKI_lib_State_Machine.vi"("State(s) in Front (\"\")"=w543, "State(s) in (\"\")"="UI: Update\nUI: Reset\nGraph: SaveCursorLoc\nLED: CloseVIRef\nQueue: Destory\nData: Cleanup\nExit", "State(s) at Back (\"\")"=w541) -> ("States Out"=w552:string)  [unwired: 12 in]
        n286 = call <vilib>:"Add State(s) to Queue__JKI_lib_State_Machine.vi"("State(s) in Front (\"\")"=w552, "State(s) in (\"\")"=w558) -> ("States Out"=w557:string)  [unwired: 13 in]
      }
      frame "---------- Data ----------" {
        # "Do not put any code in this frame.\n(It is a separator no-op. You can make a copy of this frame to create a new Data frame)"
        n287 = call <vilib>:"Add State(s) to Queue__JKI_lib_State_Machine.vi"("State(s) in (\"\")"=w571) -> ("States Out"=w570:string)  [unwired: 14 in]
      }
      frame "Data: Initialize" {
        w572 = path ""  # CaliPath
        w573 = dbl[] []  # V4
        w574 = dbl[][] []  # Ch4Data
        w575 = FALSE  # bothVidSourceAvail
        w576 = T1 {"Main Frame Grabber"=FALSE, "Side Frame Grabber"=FALSE, "Main Camera"=FALSE, "Side Camera"=FALSE}  # video source
        w577 = FALSE  # LED vi ref open?
        w579 = T22 {"DeCon Channel"=enum."1", "Scale Bar"=FALSE, "Scale Low"=3.0, "Scale High"=8.0, "ANSI"=20.0, "Radius"=1.0, "3D?"=FALSE, "Firefly?"=FALSE, "Pentero?"=FALSE}  # VideoConfig
        w580 = T26 {"Ch1APDSerial#"="", "Ch2APDSerial#"="", "Ch3APDSerial#"="", "Ch4APDSerial#"=""}  # APDSerialNum
        w581 = u32 0  # Aquisition Timer
        w582 = cluster{"RunID":i8, "BG ID":i8, "Cali ID":i8} {"RunID"=1, "BG ID"=1, "Cali ID"=1}  # IDs
        w583 = refnum<vi> refnum  # LED vi reference
        w584 = path ""  # TempPath
        w585 = T27 {"DataPath"=path "", "BG Path"=path "", "iRFPath"=path "", "CaliPath"=path ""}  # Pathes
        w587 = dbl[] []  # V3
        w588 = dbl[] []  # V2
        w589 = dbl[] []  # V1
        w591 = u32 0  # FastTimer
        w592 = u32 0  # SlowTimer
        w593 = dbl[][] []  # Ch3Data
        w594 = dbl[][] []  # Ch2Data
        w578 = dbl[][] []  # Ch1Data
        w597 = T2 {"Digitizer"=FALSE, "Labjack"=FALSE, "Aiming Beam"=FALSE, "355 Laser"=FALSE, "TCP/IP"=FALSE}  # System Status
        w598 = T28 {"DIO_EF_CLOCK1_DIVISOR"=16, "DIO_EF_CLOCK1_ROLL_VALUE"=25000, "DIO#_EF_INDEX"=0, "DIO#_EF_OPTIONS"=1, "DIO#_EF_CONFIG_A"=6250}  # AB PWM setting
        w599 = T4 {"Ch1 Bias"="TDA11", "Ch2 Bias"="DAC10", "Ch3 Bias"="DAC0", "Ch4 Bias"="DAC0", "355 PWM"="FIO0", "AimingBeam PWM"="FIO2", "Laser Ready"="FIO3", "Interlock"="FIO1", "Laser Start/Stop"="FIO1", "Red LED"="FIO1", "Green LED"="FIO1", "Foot Pedal"="DIO15"}  # LJ Pinout
        w600 = 0  # TCP attempt count
        w601 = u32 0  # Laser start tic
        w602 = refnum<k20>[] []  # niTClk sessions
        w603 = u32 0  # Last Trigger
        w604 = T28 {"DIO_EF_CLOCK1_DIVISOR"=16, "DIO_EF_CLOCK1_ROLL_VALUE"=25000, "DIO#_EF_INDEX"=0, "DIO#_EF_OPTIONS"=1, "DIO#_EF_CONFIG_A"=6250}  # 355 PWM setting
        w605 = T29 {"Aiming Beam COM Port"="COM3", "Min Current"=0.0, "Max Current"=63.0, "Default Current"=20.0, "Freq"=0}  # AB Cluster
        w606 = T30 {"resource name"="", "resource name 2"="", "Channel"=enum."Channel 0", "trigger source"="VAL_EXTERNAL", "trigger level"=0.5, "trigger delay"=1.35e-07, "min sample rate"=12500000000.0, "min record length"=2500, "vertical range"=1.0, "vertical offset"=-0.25, "Waveform to Avg"=2000}  # FLImDAQ
        w607 = FALSE  # SysRunning?
        w595 = path ""  # DefaultPath
        w608 = ""  # CaseID
        w609 = T7 {"Ch1Enable?"=FALSE, "Ch2Enable?"=FALSE, "Ch3Enable?"=FALSE, "Ch1AutoGain?"=FALSE, "Ch2AutoGain?"=FALSE, "Ch3AutoGain?"=FALSE, "AimingBeamEnable?"=FALSE}  # SysConfigCluster
        w610 = T31 {"Current VI Reference"=refnum, "Close Panel on Exit?"=FALSE}  # Core
        # "Initialize the shift-register data, here.\n(data names are defined by what you wire into the bundle function)"
        n288 = Bundle("Core"=w610, "SysConfigCluster"=w609, "System Status"=w597, "IDs"=w582, "CaseID"=w608, "DefaultPath"=w595, "Pathes"=w585, "FLImDAQ"=w606, "SysRunning?"=w607, "AB Cluster"=w605, "LJ Pinout"=w599, "355 PWM setting"=w604, "AB PWM setting"=w598, "Last Trigger"=w603, "niTClk sessions"=w602, "Laser start tic"=w601, "TCP attempt count"=w600, "Ch1Data"=w578, "Ch2Data"=w594, "Ch3Data"=w593, "Ch4Data"=w574, "V1"=w589, "V2"=w588, "V3"=w587, "V4"=w573, "SlowTimer"=w592, "FastTimer"=w591, "listener ID"=refnum<k5> refnum, "TempPath"=w584, "CaliPath"=w572, "LED vi reference"=w583, "Aquisition Timer"=w581, "APDSerialNum"=w580, "VideoConfig"=w579, "LED vi ref open?"=w577, "video source"=w576, "bothVidSourceAvail"=w575) -> (w586:T23)  [unwired: 1 in]
        n289 = call <vilib>:"Add State(s) to Queue__JKI_lib_State_Machine.vi"("State(s) in (\"\")"=w613) -> ("States Out"=w612:string)  [unwired: 14 in]
      }
      frame "Data: loadLastUseMacro" {
        # "Load last use BG and Cali and iRF.\n(It is a separator no-op. You can make a copy of this frame to create a new Data frame)"
        n290 = call <vilib>:"Add State(s) to Queue__JKI_lib_State_Machine.vi"("State(s) in Front (\"\")"="Data: loadLastUseBG\nData: LoadRealtimeDeConBG\nData: loadSystemCali\nData: loadLastUseiRF\n/*Data: LoadiRFFromAPDFile\nUI: CaliAndiRFLoaded\nData: ShowiRF" ("State(s) in Front (\"\")"), "State(s) in (\"\")"=w619) -> ("States Out"=w618:string)  [unwired: 13 in]
      }
      frame "Data: loadLastUseBG" {
        w623 = enum16{"write", "read"}."write" ("action")
        # "Load last use BG.\n()"
        n291 = Unbundle By Name(w642) -> ("TempPath"=w641:path)
        n292 = call "FLImDAQ_FGV.vi"() -> ("Read data"=w637:T5)  [unwired: 10 in, 1 out]
        n293 = Build Path(base path=w641, name or relative path="Background.tdms") -> (appended path=w640:path)
        n294 = call "ReadBGorCali (SubVI).vi"("DataType"=enum16{"BG", "Cali"}."BG", "error in (no error)"=w639, "file path in"=w640) -> ("error out"=w638:errorcluster, "AvgDataCluster"=w633:T32)  [unwired: 6 in, 1 out]
        n295 = Unbundle By Name(w633) -> ("Channel 1"=w620:dbl[], "Channel 2"=w632:dbl[], "Channel 3"=w625:dbl[], "Channel 4"=w622:dbl[])
        n296 = Unbundle By Name(w637) -> ("min record length"=w629:i32)
        n297 = Array Size(array=w620) -> (size(s)=w631:i32)
        "BG length" <- w631
        n298 = Equal?(x=w631, y=w629) -> (x = y?=w630:bool)
        n299 = Select(t="UI: BGLoaded" ("State(s) in Front (\"\")"), s=w630, f="UI: BGSizeError" ("State(s) in Front (\"\")")) -> (s? t:f=w634:string)
        n300 = case shown="True" w630 {
          tunnel: w620 -> [_ w653]
          tunnel: w632 -> [_ w652]
          tunnel: w625 -> [_ w651]
          tunnel: w629 -> [w648 _]
          tunnel: [w647 w653] -> w628
          tunnel: [w647 w652] -> w627
          tunnel: [w647 w651] -> w626
          tunnel: w622 -> [_ w650]
          tunnel: [w647 w650] -> w621
          frame False {
            # "If error set BG all 0, update UI"
            n301 = for {
              N: w648 -> [_]
              tunnel: [0.0] -> w647 mode=indexing
            }
          }
          frame True {
            # "If no error, check size match"
          }
        }
        n302 = call "BG4FGV.vi"("action"=w623, "BG4 in"=w621) -> ()  [unwired: 8 in, 2 out]
        n303 = call "BG3FGV.vi"("action"=w623, "BG3 in"=w626) -> ()  [unwired: 8 in, 2 out]
        n304 = call "BG1FGV.vi"("action"=w623, "BG1 in"=w628) -> ()  [unwired: 8 in, 2 out]
        n305 = call "BG2FGV.vi"("action"=w623, "BG2 in"=w627) -> ()  [unwired: 8 in, 2 out]
        n306 = call <vilib>:"Add State(s) to Queue__JKI_lib_State_Machine.vi"("State(s) in Front (\"\")"=w634, "State(s) in (\"\")"=w646) -> ("States Out"=w645:string)  [unwired: 13 in]
      }
      frame "Data: LoadRealtimeDeConBG" {
        # "Load saved realtime DeCon BG from Temp file"
        n307 = Unbundle By Name(w668) -> ("TempPath"=w667:path)
        n308 = Build Path(base path=w667, name or relative path="RealTimeDeConBGTemp.tdms") -> (appended path=w665:path)
        n309 = TDMS Open(8:w663, 10:T15."open" ("operation (0:open)"), 11:w665) -> (0:w660:errorcluster, 3:w662:refnum<k34>)  [unwired: 4 in]
        n310 = TDMS Read(0:w662, 5:"Realtime DeCon BG" ("group name in (Untitled)"), 7:string[] ["Ch1", "Ch2", "Ch3"], 11:w660, 12:dbl[][] [] ("BGAll")) -> (4:w658:refnum<k34>, 10:w654:dbl[][], 15:w657:errorcluster)  [unwired: 3 in, 3 out]
        n311 = local write "BGAll"(w654) -> ()
        n312 = TDMS Close(8:w657, 11:w658) -> (0:w656:errorcluster)  [unwired: 1 out]
        n313 = local write "BG Graph"(w654) -> ()
        n314 = call <vilib>:"Add State(s) to Queue__JKI_lib_State_Machine.vi"("State(s) in (\"\")"=w671) -> ("States Out"=w670:string)  [unwired: 14 in]
      }
      frame "Data: loadSystemCali" {
        # "Load last use calibration.\n()"
        n315 = Unbundle By Name(w679) -> ("CaliPath"=w678:path)
        n316 = Build Path(base path=w678, name or relative path="Calibration.tdms") -> (appended path=w674:path)
        n317 = call "ReadBGorCali (SubVI).vi"("DataType"=enum16{"BG", "Cali"}."Cali", "error in (no error)"=w673, "file path in"=w674) -> ("error out"=w675:errorcluster, "CtrlVCluster"=w677:T33, "AvgDataCluster"=w676:T32)  [unwired: 6 in]
        n318 = case shown="No Error" w675 {
          tunnel: w677 -> [w698 _]
          tunnel: w676 -> [w697 _]
          frame No Error {
            w688 = T34 {"Ch1 WF"=[], "Ch2 WF"=[], "Ch3 WF"=[], "Ch4 WF"=[], "V1"=0.0, "V2"=0.0, "V3"=0.0, "V4"=0.0}  # SysCaliData
            n319 = Unbundle By Name(w697) -> ("Channel 1"=w696:dbl[], "Channel 2"=w695:dbl[], "Channel 3"=w694:dbl[], "Channel 4"=w687:dbl[])
            n320 = Unbundle By Name(w698) -> ("V 1"=w693:dbl[], "V 2"=w692:dbl[], "V 3"=w686:dbl[], "V 4"=w684:dbl[])
            n321 = Index Array(array=w693) -> (element=w691:dbl)  [unwired: 1 in]
            n322 = Index Array(array=w692) -> (element=w690:dbl)  [unwired: 1 in]
            n323 = Index Array(array=w686) -> (element=w689:dbl)  [unwired: 1 in]
            n324 = Index Array(array=w684) -> (element=w685:dbl)  [unwired: 1 in]
            n325 = Bundle By Name(cluster=w688, "Ch1 WF"=w696, "Ch2 WF"=w695, "Ch3 WF"=w694, "Ch4 WF"=w687, "V1"=w691, "V2"=w690, "V3"=w689, "V4"=w685) -> (w699:T34)
            n326 = global write "GlobalVariables.vi" "SysCaliData"(w699) -> ()
          }
          frame Error {
          }
        }
        n327 = call <vilib>:"Add State(s) to Queue__JKI_lib_State_Machine.vi"("State(s) in (\"\")"=w683) -> ("States Out"=w682:string)  [unwired: 14 in]
      }
      frame "Data: LoadiRFFromAPDFile" {
        w729 = T16 {"Ch1 iRF"=[], "Ch2 iRF"=[], "Ch3 iRF"=[], "Ch4 iRF"=[]}  # LastUseiRF
        # "only load the last 5th  iRF for the moment"
        # "Load APD detector data\n(It is a separator no-op. You can make a copy of this frame to create a new Data frame)"
        n328 = Unbundle By Name(w751) -> ("APDSerialNum.Ch1APDSerial#"=w750:string, "APDSerialNum.Ch2APDSerial#"=w731:string, "APDSerialNum.Ch3APDSerial#"=w730:string, "APDSerialNum.Ch4APDSerial#"=w727:string)
        n329 = call "CreatFromSerialNumNoRaw.vi"("error in (no error)"=w728, "APD Serial #"=w750) -> ("error out"=w748:errorcluster, "APDClass out"=w749:refnum<class "APDClass.lvclass">)  [unwired: 8 in]
        n330 = call "CreatFromSerialNumNoRaw.vi"("error in (no error)"=w728, "APD Serial #"=w731) -> ("error out"=w739:errorcluster, "APDClass out"=w740:refnum<class "APDClass.lvclass">)  [unwired: 8 in]
        n331 = call "CreatFromSerialNumNoRaw.vi"("error in (no error)"=w728, "APD Serial #"=w730) -> ("error out"=w733:errorcluster, "APDClass out"=w734:refnum<class "APDClass.lvclass">)  [unwired: 8 in]
        n332 = call "CreatFromSerialNumNoRaw.vi"("error in (no error)"=w728, "APD Serial #"=w727) -> ("error out"=w725:errorcluster, "APDClass out"=w726:refnum<class "APDClass.lvclass">)  [unwired: 8 in]
        n333 = call-dynamic "Read iRFData.vi"("error in (no error)"=w748, "APDClass in"=w749) -> ("iRFData"=w747:T35)  [unwired: 7 in, 2 out]
        n334 = call-dynamic "Read iRFData.vi"("error in (no error)"=w739, "APDClass in"=w740) -> ("iRFData"=w743:T35)  [unwired: 7 in, 2 out]
        n335 = call-dynamic "Read iRFData.vi"("error in (no error)"=w733, "APDClass in"=w734) -> ("iRFData"=w737:T35)  [unwired: 7 in, 2 out]
        n336 = call-dynamic "Read iRFData.vi"("error in (no error)"=w725, "APDClass in"=w726) -> ("iRFData"=w724:T35)  [unwired: 7 in, 2 out]
        n337 = Unbundle By Name(w747) -> ("iRFWFsAvg"=w746:dbl[][])
        n338 = Unbundle By Name(w743) -> ("iRFWFsAvg"=w742:dbl[][])
        n339 = Unbundle By Name(w737) -> ("iRFWFsAvg"=w736:dbl[][])
        n340 = Unbundle By Name(w724) -> ("iRFWFsAvg"=w721:dbl[][])
        n341 = Array Size(array=w746) -> (size(s)=w745:i32[])
        n342 = Array Size(array=w742) -> (size(s)=w738:i32[])
        n343 = Array Size(array=w736) -> (size(s)=w732:i32[])
        n344 = Array Size(array=w721) -> (size(s)=w722:i32[])
        n345 = Index Array(array=w745, index=0) -> (element=w720:i32)
        n346 = Index Array(array=w738, index=0) -> (element=w716:i32)
        n347 = Index Array(array=w732, index=0) -> (element=w713:i32)
        n348 = Index Array(array=w722, index=0) -> (element=w710:i32)
        n349 = Subtract(x=w720, y=5) -> (x-y=w718:i32)
        n350 = Subtract(x=w716, y=5) -> (x-y=w715:i32)
        n351 = Subtract(x=w713, y=5) -> (x-y=w712:i32)
        n352 = Subtract(x=w710, y=5) -> (x-y=w709:i32)
        n353 = Index Array(array=w746, index (row)=w718) -> (element=w708:dbl[])  [unwired: 1 in]
        n354 = Index Array(array=w742, index (row)=w715) -> (element=w707:dbl[])  [unwired: 1 in]
        n355 = Index Array(array=w736, index (row)=w712) -> (element=w706:dbl[])  [unwired: 1 in]
        n356 = Index Array(array=w721, index (row)=w709) -> (element=w705:dbl[])  [unwired: 1 in]
        n357 = call "DownSampleAndShiftiRF (SubVI).vi"("ArrayIn"=w708) -> ("ArrayOut"=w704:dbl[])  [unwired: 10 in]
        n358 = call "DownSampleAndShiftiRF (SubVI).vi"("ArrayIn"=w707) -> ("ArrayOut"=w700:dbl[])  [unwired: 10 in]
        n359 = call "DownSampleAndShiftiRF (SubVI).vi"("ArrayIn"=w706) -> ("ArrayOut"=w701:dbl[])  [unwired: 10 in]
        n360 = call "DownSampleAndShiftiRF (SubVI).vi"("ArrayIn"=w705) -> ("ArrayOut"=w703:dbl[])  [unwired: 10 in]
        n361 = call <vilib>:"Add State(s) to Queue__JKI_lib_State_Machine.vi"("State(s) in (\"\")"=w754) -> ("States Out"=w753:string)  [unwired: 14 in]
        n362 = Bundle(cluster=w729, "Ch1 iRF"=w704, "Ch2 iRF"=w700, "Ch3 iRF"=w701, "Ch4 iRF"=w703) -> (w702:T16)
        n363 = global write "GlobalVariables.vi" "LastUseiRF"(w702) -> ()
      }
      frame "Data: loadLastUseiRF" {
        # "Load last use iRF.\n()"
        n364 = Unbundle By Name(w760) -> ("TempPath"=w759:path)
        n365 = Build Path(base path=w759, name or relative path="iRF.tdms") -> (appended path=w765:path)
        n366 = TDMS Open(8:w755, 11:w765) -> (0:w763:errorcluster, 3:w764:refnum<k34>)  [unwired: 5 in]
        n367 = TDMS Read(0:w764, 11:w763, 12:dbl[][] []) -> (4:w758:refnum<k34>, 10:w761:dbl[][], 15:w757:errorcluster)  [unwired: 5 in, 3 out]
        n368 = TDMS Close(8:w757, 11:w758) -> (0:w756:errorcluster)  [unwired: 1 out]
        n369 = case shown="No Error" w757 {
          tunnel: w761 -> [w775 _]
          frame No Error {
            w778 = T16 {"Ch1 iRF"=[], "Ch2 iRF"=[], "Ch3 iRF"=[], "Ch4 iRF"=[]}  # LastUseiRF
            n370 = Index Array(array=w775, index (row)=0) -> (element=w770:dbl[])  [unwired: 1 in]
            n371 = Index Array(array=w775, index (row)=1) -> (element=w771:dbl[])  [unwired: 1 in]
            n372 = Index Array(array=w775, index (row)=2) -> (element=w772:dbl[])  [unwired: 1 in]
            n373 = Index Array(array=w775, index (row)=3) -> (element=w773:dbl[])  [unwired: 1 in]
            n374 = Add Array Elements(numeric array=w770) -> (sum=w784:dbl)
            n375 = Add Array Elements(numeric array=w771) -> (sum=w782:dbl)
            n376 = Add Array Elements(numeric array=w772) -> (sum=w780:dbl)
            n377 = Add Array Elements(numeric array=w773) -> (sum=w776:dbl)
            n378 = Divide(x=w770, y=w784) -> (x/y=w783:dbl[])
            n379 = Divide(x=w771, y=w782) -> (x/y=w781:dbl[])
            n380 = Divide(x=w772, y=w780) -> (x/y=w779:dbl[])
            n381 = Divide(x=w773, y=w776) -> (x/y=w774:dbl[])
            n382 = Bundle(cluster=w778, "Ch1 iRF"=w783, "Ch2 iRF"=w781, "Ch3 iRF"=w779, "Ch4 iRF"=w774) -> (w786:T16)
            n383 = Array Size(array=w770) -> (size(s)=→"iRF length":i32)
            n384 = global write "GlobalVariables.vi" "LastUseiRF"(w786) -> ()
          }
          frame Error {
          }
        }
        n385 = call <vilib>:"Add State(s) to Queue__JKI_lib_State_Machine.vi"("State(s) in (\"\")"=w769) -> ("States Out"=w768:string)  [unwired: 14 in]
      }
      frame "Data: ShowiRF" {
        # "Show loaded iRF.\n(It is a separator no-op. You can make a copy of this frame to create a new Data frame)"
        n386 = global read "GlobalVariables.vi" "LastUseiRF"() -> (w795:T16)
        n387 = Unbundle By Name(w795) -> ("Ch1 iRF"=w794:dbl[], "Ch2 iRF"=w793:dbl[], "Ch3 iRF"=w792:dbl[], "Ch4 iRF"=w791:dbl[])
        n388 = Build Array(w794, w793, w792, w791) -> (→"iRF Graph":dbl[][])
        n389 = call <vilib>:"Add State(s) to Queue__JKI_lib_State_Machine.vi"("State(s) in (\"\")"=w800) -> ("States Out"=w799:string)  [unwired: 14 in]
      }
      frame "Data: saveCalibration" {
        # "Average data and save calibration file. [Covers: REQ11]\n(It is a separator no-op. You can make a copy of this frame to create a new Data frame)"
        n390 = Unbundle By Name(w819) -> ("Ch1Data"=w818:dbl[][], "V1"=w817:dbl[], "Ch2Data"=w816:dbl[][], "V2"=w815:dbl[], "Ch3Data"=w814:dbl[][], "V3"=w813:dbl[], "Ch4Data"=w804:dbl[][], "V4"=w803:dbl[], "Pathes.CaliPath"=w822:path, "IDs.Cali ID"=w821:i8)
        n391 = Increment(x=w821) -> (x+1=w805:i8)
        n392 = Bundle("Ch1Data"=w818, "V1"=w817) -> (w812:cluster{"Ch1Data":dbl[][], "V1":dbl[]})  [unwired: 1 in]
        n393 = Bundle("Ch4Data"=w804, "V4"=w803) -> (w802:cluster{"Ch4Data":dbl[][], "V4":dbl[]})  [unwired: 1 in]
        n394 = Bundle("Ch2Data"=w816, "V2"=w815) -> (w811:cluster{"Ch2Data":dbl[][], "V2":dbl[]})  [unwired: 1 in]
        n395 = Bundle("Ch3Data"=w814, "V3"=w813) -> (w810:cluster{"Ch3Data":dbl[][], "V3":dbl[]})  [unwired: 1 in]
        n396 = Format Value(string ("")="Calibration" ("default name"), format string="%02d", value (0)=w805) -> (output string=w824:string)
        n397 = Build Path(base path=w822, name or relative path=w824) -> (appended path=w809:path)
        n398 = call "SaveBGorCali(SubVI).vi"("Channel1"=w812, "BG path"=w809, "DataType"=enum16{"BG", "Cali"}."Cali", "Channel 2"=w811, "Channel 3"=w810, "Channel 4"=w802, "error in (no error)"=w808, "SytemID"="UCDVetMed") -> ("error out"=w807:errorcluster)  [unwired: 7 in]
        n399 = call <vilib>:"Add State(s) to Queue__JKI_lib_State_Machine.vi"("State(s) in (\"\")"=w827) -> ("States Out"=w826:string)  [unwired: 14 in]
      }
      frame "Data: saveiRF" {
        w833 = enum16{"write", "read"}."read" ("action")
        # "Get iRF from decon stracture and save it on disk.\n(It is a separator no-op. You can make a copy of this frame to create a new Data frame)"
        n400 = Unbundle By Name(w850) -> ("TempPath"=w849:path)
        n401 = call "Ch1DeconEngineFGV.vi"("action(read)"=w833) -> ("Error Out"=w855:errorcluster, "Ch1DeconEngine out"=w856:refnum<class "LaguerreDeconEngineClass.lvclass">)  [unwired: 9 in]
        n402 = call "Ch2DeconEngineFGV.vi"("action(read)"=w833) -> ("Error Out"=w853:errorcluster, "Ch2DeconEngine out"=w854:refnum<class "LaguerreDeconEngineClass.lvclass">)  [unwired: 9 in]
        n403 = call "Ch3DeconEngineFGV.vi"("action(read)"=w833) -> ("Error Out"=w851:errorcluster, "Ch3DeconEngine out"=w852:refnum<class "LaguerreDeconEngineClass.lvclass">)  [unwired: 9 in]
        n404 = call "Ch4DeconEngineFGV.vi"("action(read)"=w833) -> ("Error Out"=w832:errorcluster, "Ch3DeconEngine out"=w831:refnum<class "LaguerreDeconEngineClass.lvclass">)  [unwired: 9 in]
        n405 = Build Path(base path=w849, name or relative path="iRF" ("default name")) -> (appended path=w847:path)
        n406 = call "getIRF.vi"("error in (no error)"=w832, "LaguerreDeconEngineClass in"=w831) -> ("iRF"=w830:dbl[])  [unwired: 7 in, 2 out]
        n407 = call "getIRF.vi"("error in (no error)"=w855, "LaguerreDeconEngineClass in"=w856) -> ("iRF"=w838:dbl[])  [unwired: 7 in, 2 out]
        n408 = call "getIRF.vi"("error in (no error)"=w853, "LaguerreDeconEngineClass in"=w854) -> ("iRF"=w837:dbl[])  [unwired: 7 in, 2 out]
        n409 = call "getIRF.vi"("error in (no error)"=w851, "LaguerreDeconEngineClass in"=w852) -> ("iRF"=w836:dbl[])  [unwired: 7 in, 2 out]
        n410 = TDMS Open(8:w846, 10:T15."create or replace" ("operation (0:open)"), 11:w847) -> (0:w843:errorcluster, 3:w844:refnum<k34>)  [unwired: 4 in]
        n411 = Bundle(cluster=T16 {"Ch1 iRF"=[], "Ch2 iRF"=[], "Ch3 iRF"=[], "Ch4 iRF"=[]} ("LastUseiRF"), "Ch1 iRF"=w838, "Ch2 iRF"=w837, "Ch3 iRF"=w836, "Ch4 iRF"=w830) -> (w834:T16)
        n412 = Build Array(w838, w837, w836, w830) -> (w842:dbl[][])
        n413 = global write "GlobalVariables.vi" "LastUseiRF"(w834) -> ()
        n414 = TDMS Write(0:w844, 5:"iRF" ("group name in (Untitled)"), 7:string[] ["Ch1", "Ch2", "Ch3", "Ch4"] ("channel name(s) in (Untitled)"), 9:w842, 11:w843) -> (4:w841:refnum<k34>, 15:w840:errorcluster)  [unwired: 1 in, 2 out]
        n415 = TDMS Close(8:w840, 11:w841) -> (0:w839:errorcluster)  [unwired: 1 out]
        n416 = call <vilib>:"Add State(s) to Queue__JKI_lib_State_Machine.vi"("State(s) in (\"\")"=w859) -> ("States Out"=w858:string)  [unwired: 14 in]
      }
      frame "Data: saveBGtoFGV" {
        w886 = enum16{"write", "read"}."write" ("action")
        # "Save BG and pass it to FGV.\n(save BG to disk and set it to FGV)"
        n417 = call "DotNetFGV.vi"("Error In"=w876) -> ("Error Out"=w881:errorcluster, "reference out"=w882:refnum<k24>)  [unwired: 9 in]
        n418 = Unbundle By Name(w887) -> ("Ch1Data"=w871:dbl[][], "Ch2Data"=w869:dbl[][], "Ch3Data"=w867:dbl[][], "Ch4Data"=w865:dbl[][])
        n419 = Transpose 2D Array(2D array=w871) -> (transposed array=w885:dbl[][])
        n420 = Transpose 2D Array(2D array=w869) -> (transposed array=w884:dbl[][])
        n421 = Transpose 2D Array(2D array=w867) -> (transposed array=w883:dbl[][])
        n422 = call "AvgArrayTimeCritical.vi"("2D array"=w869) -> ("1D Avg"=w868:dbl[])  [unwired: 10 in]
        n423 = call "AvgArrayTimeCritical.vi"("2D array"=w867) -> ("1D Avg"=w866:dbl[])  [unwired: 10 in]
        n424 = call "WaveformTUA(SubVI).vi"("error in (no error)"=w881, "WF in"=w885, "new reference"=w882) -> ("error out"=w863:errorcluster, "WF out"=w872:dbl[])  [unwired: 6 in, 1 out]
        n425 = call "WaveformTUA(SubVI).vi"("error in (no error)"=w881, "WF in"=w884, "new reference"=w882) -> ("error out"=w862:errorcluster, "WF out"=w874:dbl[])  [unwired: 6 in, 1 out]
        n426 = call "WaveformTUA(SubVI).vi"("error in (no error)"=w881, "WF in"=w883, "new reference"=w882) -> ("error out"=w861:errorcluster, "WF out"=w873:dbl[])  [unwired: 6 in, 1 out]
        n427 = call "AvgArrayTimeCritical.vi"("2D array"=w871) -> ("1D Avg"=w870:dbl[])  [unwired: 10 in]
        n428 = call "AvgArrayTimeCritical.vi"("2D array"=w865) -> ("1D Avg"=w864:dbl[])  [unwired: 10 in]
        n429 = call "BG1FGV.vi"("Error In"=w863, "action"=w886, "BG1 in"=w870) -> ("Error Out"=w880:errorcluster)  [unwired: 7 in, 1 out]
        n430 = call "BG2FGV.vi"("Error In"=w862, "action"=w886, "BG2 in"=w868) -> ("Error Out"=w879:errorcluster)  [unwired: 7 in, 1 out]
        n431 = call "BG3FGV.vi"("Error In"=w861, "action"=w886, "BG3 in"=w866) -> ("Error Out"=w878:errorcluster)  [unwired: 7 in, 1 out]
        n432 = call "BG4FGV.vi"("action"=w886, "BG4 in"=w864) -> ("Error Out"=w877:errorcluster)  [unwired: 8 in, 1 out]
        n433 = Build Array(w872, w874, w873) -> (→"BGAll" →"BG Graph":dbl[][])
        n434 = Merge Errors(w880, w879, w878, w877) -> (w875:errorcluster)
        n435 = call <vilib>:"Add State(s) to Queue__JKI_lib_State_Machine.vi"("State(s) in (\"\")"=w890) -> ("States Out"=w889:string)  [unwired: 14 in]
      }
      frame "Data: saveBGtoFile" {
        w912 = "Background" ("name or relative path")
        # "Save BG to file.\n(save BG to disk both data folder and temp folder)"
        n436 = Unbundle By Name(w916) -> ("Pathes.BG Path"=w909:path, "IDs.BG ID"=w908:i8, "Ch1Data"=w906:dbl[][], "V1"=w905:dbl[], "Ch2Data"=w904:dbl[][], "V2"=w903:dbl[], "Ch3Data"=w902:dbl[][], "V3"=w901:dbl[], "Ch4Data"=w893:dbl[][], "V4"=w892:dbl[], "TempPath"=w914:path)
        n437 = Increment(x=w908) -> (x+1=w913:i8)
        n438 = Format Value(string ("")=w912, format string="%02d", value (0)=w913) -> (output string=w911:string)
        n439 = Build Path(base path=w914, name or relative path=w912) -> (appended path=w895:path)
        n440 = call "File Dialog2"("start path"=w909, "prompt"="Please select BG name, DO NOT CANCEL!", "default name"=w911) -> ("selected path"=w896:path)  [unwired: 9 in, 3 out]
        n441 = Bundle("Ch1Data"=w906, "V1"=w905) -> (w900:cluster{"Ch1Data":dbl[][], "V1":dbl[]})  [unwired: 1 in]
        n442 = Bundle("Ch4Data"=w893, "V4"=w892) -> (w891:cluster{"Ch4Data":dbl[][], "V4":dbl[]})  [unwired: 1 in]
        n443 = Bundle("Ch2Data"=w904, "V2"=w903) -> (w899:cluster{"Ch2Data":dbl[][], "V2":dbl[]})  [unwired: 1 in]
        n444 = Bundle("Ch3Data"=w902, "V3"=w901) -> (w898:cluster{"Ch3Data":dbl[][], "V3":dbl[]})  [unwired: 1 in]
        n445 = Build Array(w896, w895) -> (w894:path[])
        n446 = for {
          tunnel: w900 -> [w927]
          tunnel: w899 -> [w926]
          tunnel: w898 -> [w925]
          shift-right: [w928] -> w907
          shift-left: w897 -> [w924]
          tunnel: w894 -> [w923] mode=indexing
          tunnel: w891 -> [w921]
          n447 = call "SaveBGorCali(SubVI).vi"("Channel1"=w927, "BG path"=w923, "DataType"=enum16{"BG", "Cali"}."BG", "Channel 2"=w926, "Channel 3"=w925, "Channel 4"=w921, "error in (no error)"=w924, "SytemID"="UCDMC") -> ("error out"=w928:errorcluster)  [unwired: 7 in]
        }
        n448 = call <vilib>:"Add State(s) to Queue__JKI_lib_State_Machine.vi"("State(s) in (\"\")"=w919) -> ("States Out"=w918:string)  [unwired: 14 in]
      }
      frame "Data: saveDeConBGtoFile" {
        # "Save realtime DeCon BG to temp file.\n(It is a separator no-op. You can make a copy of this frame to create a new Data frame)"
        n449 = Unbundle By Name(w942) -> ("TempPath"=w941:path)
        n450 = Build Path(base path=w941, name or relative path="RealTimeDeConBGTemp") -> (appended path=w939:path)
        n451 = local read "BGAll"() -> (w935:dbl[][])
        n452 = TDMS Open(8:w937, 10:T15."create or replace" ("operation (0:open)"), 11:w939) -> (0:w934:errorcluster, 3:w936:refnum<k34>)  [unwired: 4 in]
        n453 = TDMS Write(0:w936, 5:"Realtime DeCon BG" ("group name in (Untitled)"), 7:string[] ["Ch1", "Ch2", "Ch3"], 9:w935, 11:w934) -> (4:w931:refnum<k34>, 15:w930:errorcluster)  [unwired: 1 in, 2 out]
        n454 = TDMS Close(8:w930, 11:w931) -> (0:w929:errorcluster)  [unwired: 1 out]
        n455 = call <vilib>:"Add State(s) to Queue__JKI_lib_State_Machine.vi"("State(s) in (\"\")"=w945) -> ("States Out"=w944:string)  [unwired: 14 in]
      }
      frame "Data: showBG" {
        # "Show BG in seperate window.\n()"
        n456 = call "showBG.vi"() -> ()  [unwired: 12 in]
        n457 = call <vilib>:"Add State(s) to Queue__JKI_lib_State_Machine.vi"("State(s) in (\"\")"=w950) -> ("States Out"=w949:string)  [unwired: 14 in]
      }
      frame "Data: irfAlignment" {
        w951 = enum16{"write", "read"}."write" ("action")
        # "do iRF alignment in this state\n(It is a separator no-op. You can make a copy of this frame to create a new Data frame)"
        n458 = Unbundle By Name(w996) -> ("Ch1Data"=w1032:dbl[][], "Ch2Data"=w1031:dbl[][], "Ch3Data"=w1030:dbl[][], "Ch4Data"=w973:dbl[][])
        n459 = call "Ch1DeconEngineFGV.vi"("Error In"=w972) -> ("Error Out"=w1028:errorcluster, "Ch1DeconEngine out"=w1029:refnum<class "LaguerreDeconEngineClass.lvclass">)  [unwired: 9 in]
        n460 = call "Ch2DeconEngineFGV.vi"("Error In"=w972) -> ("Error Out"=w1026:errorcluster, "Ch2DeconEngine out"=w1027:refnum<class "LaguerreDeconEngineClass.lvclass">)  [unwired: 9 in]
        n461 = call "Ch3DeconEngineFGV.vi"("Error In"=w972) -> ("Error Out"=w1024:errorcluster, "Ch3DeconEngine out"=w1025:refnum<class "LaguerreDeconEngineClass.lvclass">)  [unwired: 9 in]
        n462 = call "Ch4DeconEngineFGV.vi"("Error In"=w972) -> ("Error Out"=w963:errorcluster, "Ch3DeconEngine out"=w962:refnum<class "LaguerreDeconEngineClass.lvclass">)  [unwired: 9 in]
        n463 = call "AvgArray.vi"("2D array in"=w1031) -> ("1D Avg out"=w978:dbl[])  [unwired: 10 in]
        n464 = call "AvgArray.vi"("2D array in"=w1030) -> ("1D Avg out"=w977:dbl[])  [unwired: 10 in]
        n465 = call "AvgArray.vi"("2D array in"=w973) -> ("1D Avg out"=w952:dbl[])  [unwired: 10 in]
        n466 = call "AvgArray.vi"("2D array in"=w1032) -> ("1D Avg out"=w979:dbl[])  [unwired: 10 in]
        n467 = call "RemoveDCBG.vi"("WF in"=w979) -> ("DC"=w986:dbl, "WF out"=w976:dbl[])  [unwired: 8 in, 1 out]
        n468 = call "RemoveDCBG.vi"("WF in"=w978) -> ("DC"=w983:dbl, "WF out"=w989:dbl[])  [unwired: 8 in, 1 out]
        n469 = call "RemoveDCBG.vi"("WF in"=w977) -> ("DC"=w981:dbl, "WF out"=w988:dbl[])  [unwired: 8 in, 1 out]
        n470 = call "RemoveDCBG.vi"("WF in"=w952) -> ("DC"=w956:dbl, "WF out"=w954:dbl[])  [unwired: 8 in, 1 out]
        n471 = call "computeIRFAlignment.vi"("error in (no error)"=w1028, "fIRF temp"=w976, "LaguerreDeconEngineClass in"=w1029) -> ("error out"=w1020:errorcluster, "LaguerreDeconEngineClass out"=w1021:refnum<class "LaguerreDeconEngineClass.lvclass">)  [unwired: 6 in, 1 out]
        n472 = call "computeIRFAlignment.vi"("error in (no error)"=w1026, "fIRF temp"=w989, "LaguerreDeconEngineClass in"=w1027) -> ("error out"=w1018:errorcluster, "LaguerreDeconEngineClass out"=w1019:refnum<class "LaguerreDeconEngineClass.lvclass">)  [unwired: 6 in, 1 out]
        n473 = call "computeIRFAlignment.vi"("error in (no error)"=w1024, "fIRF temp"=w988, "LaguerreDeconEngineClass in"=w1025) -> ("error out"=w1022:errorcluster, "LaguerreDeconEngineClass out"=w1023:refnum<class "LaguerreDeconEngineClass.lvclass">)  [unwired: 6 in, 1 out]
        n474 = call "computeIRFAlignment.vi"("error in (no error)"=w963, "fIRF temp"=w954, "LaguerreDeconEngineClass in"=w962) -> ("error out"=w970:errorcluster, "LaguerreDeconEngineClass out"=w971:refnum<class "LaguerreDeconEngineClass.lvclass">)  [unwired: 6 in, 1 out]
        n475 = call "Ch1DeconEngineFGV.vi"("Error In"=w1020, "action(read)"=w951, "Ch1DeconEngine in"=w1021) -> ("Error Out"=w1016:errorcluster, "Ch1DeconEngine out"=w1017:refnum<class "LaguerreDeconEngineClass.lvclass">)  [unwired: 7 in]
        n476 = call "Ch2DeconEngineFGV.vi"("Error In"=w1018, "action(read)"=w951, "Ch2DeconEngine in"=w1019) -> ("Error Out"=w1006:errorcluster, "Ch2DeconEngine out"=w1007:refnum<class "LaguerreDeconEngineClass.lvclass">)  [unwired: 7 in]
        n477 = call "Ch3DeconEngineFGV.vi"("Error In"=w1022, "action(read)"=w951, "Ch3DeconEngine in"=w1023) -> ("Error Out"=w1000:errorcluster, "Ch3DeconEngine out"=w1001:refnum<class "LaguerreDeconEngineClass.lvclass">)  [unwired: 7 in]
        n478 = call "Ch4DeconEngineFGV.vi"("Error In"=w970, "action(read)"=w951, "Ch3DeconEngine in"=w971) -> ("Error Out"=w964:errorcluster, "Ch3DeconEngine out"=w965:refnum<class "LaguerreDeconEngineClass.lvclass">)  [unwired: 7 in]
        n479 = call "setfIRF.vi"("error in (no error)"=w1000, "fIRF"=w988, "LaguerreDeconEngineClass in"=w1001) -> ("error out"=w1004:errorcluster, "LaguerreDeconEngineClass out"=w1005:refnum<class "LaguerreDeconEngineClass.lvclass">)  [unwired: 7 in]
        n480 = call "setfIRF.vi"("error in (no error)"=w964, "fIRF"=w954, "LaguerreDeconEngineClass in"=w965) -> ("error out"=w968:errorcluster, "LaguerreDeconEngineClass out"=w969:refnum<class "LaguerreDeconEngineClass.lvclass">)  [unwired: 7 in]
        n481 = call "setfIRF.vi"("error in (no error)"=w1006, "fIRF"=w989, "LaguerreDeconEngineClass in"=w1007) -> ("error out"=w1010:errorcluster, "LaguerreDeconEngineClass out"=w1011:refnum<class "LaguerreDeconEngineClass.lvclass">)  [unwired: 7 in]
        n482 = call "setfIRF.vi"("error in (no error)"=w1016, "fIRF"=w976, "LaguerreDeconEngineClass in"=w1017) -> ("error out"=w1014:errorcluster, "LaguerreDeconEngineClass out"=w1015:refnum<class "LaguerreDeconEngineClass.lvclass">)  [unwired: 7 in]
        n483 = Unbundle By Name(w996) -> ("V1"=w975:dbl[], "V2"=w995:dbl[], "V3"=w994:dbl[], "V4"=w961:dbl[])
        n484 = call "computeLCs.vi"("error in (no error)"=w1014, "LaguerreDeconClass in"=w1015) -> ("error out"=w1012:errorcluster, "LaguerreDeconClass out"=w1013:refnum<class "LaguerreDeconEngineClass.lvclass">)  [unwired: 8 in]
        n485 = call "computeLCs.vi"("error in (no error)"=w1010, "LaguerreDeconClass in"=w1011) -> ("error out"=w1008:errorcluster, "LaguerreDeconClass out"=w1009:refnum<class "LaguerreDeconEngineClass.lvclass">)  [unwired: 8 in]
        n486 = call "computeLCs.vi"("error in (no error)"=w1004, "LaguerreDeconClass in"=w1005) -> ("error out"=w1002:errorcluster, "LaguerreDeconClass out"=w1003:refnum<class "LaguerreDeconEngineClass.lvclass">)  [unwired: 8 in]
        n487 = call "computeLCs.vi"("error in (no error)"=w968, "LaguerreDeconClass in"=w969) -> ("error out"=w966:errorcluster, "LaguerreDeconClass out"=w967:refnum<class "LaguerreDeconEngineClass.lvclass">)  [unwired: 8 in]
        n488 = call-poly <vilib>:"Mean.vi"("X"=w975) -> ("mean"=w974:dbl)  [unwired: 1 out]
        n489 = call-poly <vilib>:"Mean.vi"("X"=w961) -> ("mean"=w960:dbl)  [unwired: 1 out]
        n490 = call-poly <vilib>:"Mean.vi"("X"=w995) -> ("mean"=w993:dbl)  [unwired: 1 out]
        n491 = call "getFitting.vi"("error in (no error)"=w1012, "LaguerreDeconEngineClass in"=w1013) -> ("Fitting"=w985:dbl[])  [unwired: 7 in, 2 out]
        n492 = call "getFitting.vi"("error in (no error)"=w1008, "LaguerreDeconEngineClass in"=w1009) -> ("Fitting"=w982:dbl[])  [unwired: 7 in, 2 out]
        n493 = call "getFitting.vi"("error in (no error)"=w1002, "LaguerreDeconEngineClass in"=w1003) -> ("Fitting"=w958:dbl[])  [unwired: 7 in, 2 out]
        n494 = call "getFitting.vi"("error in (no error)"=w966, "LaguerreDeconEngineClass in"=w967) -> ("Fitting"=w957:dbl[])  [unwired: 7 in, 2 out]
        n495 = Add(x=w986, y=w985) -> (x+y=w987:dbl[])
        n496 = Add(x=w983, y=w982) -> (x+y=w984:dbl[])
        n497 = call-poly <vilib>:"Mean.vi"("X"=w994) -> ("mean"=w992:dbl)  [unwired: 1 out]
        n498 = Add(x=w981, y=w958) -> (x+y=w980:dbl[])
        n499 = Build Array(w979, w987) -> (w999:dbl[][])
        n500 = Build Array(w978, w984) -> (w998:dbl[][])
        n501 = Build Array(w977, w980) -> (w997:dbl[][])
        n502 = Add(x=w956, y=w957) -> (x+y=w955:dbl[])
        n503 = Bundle("mean"=w974, "mean"=w993, "mean"=w992, "mean"=w960) -> (w959:T36)  [unwired: 1 in]
        n504 = Build Array(w952, w955) -> (w953:dbl[][])
        n505 = call "Calib_and_iRFAlign_confirm.vi"("Current V"=w959, "Ch4 Data"=w953, "Ch3 Data"=w997, "Ch2 Data"=w998, "Ch1 Data"=w999) -> ("Save?"=w991:bool)  [unwired: 6 in]
        n506 = case shown="True" w991 {
          tunnel: ["" ("Empty String Constant") "Data: saveCalibration\nData: saveiRF\nRun: CaliIncrement"] -> w990
          frame False {
          }
          frame True {
            # "[Covers: REQ2]"
          }
        }
        n507 = call <vilib>:"Add State(s) to Queue__JKI_lib_State_Machine.vi"("State(s) in Front (\"\")"=w990, "State(s) in (\"\")"=w1035) -> ("States Out"=w1034:string)  [unwired: 13 in]
      }
      frame "Data: parseRunData" {
        # "All APD bias"
        # "flash queue"
        # "Ch3&4"
        # "Ch1&2"
        # "Flash data from queue and save it in structure\n()"
        n508 = Flush Queue(queue=w1063, error in (no error)=w1062) -> (remaining elements=w1057:T37, error out=w1058:errorcluster)  [unwired: 1 out]
        n509 = Flush Queue(queue=w1068, error in (no error)=w1062) -> (remaining elements=w1066:cluster{"double data":dbl[][]}[], error out=w1059:errorcluster)  [unwired: 1 out]
        n510 = Flush Queue(queue=w1069, error in (no error)=w1062) -> (remaining elements=w1067:cluster{"double data":dbl[][]}[], error out=w1060:errorcluster)  [unwired: 1 out]
        n511 = for {
          tunnel: w1067 -> [w1085] mode=indexing
          tunnel: [w1083] -> w1052 mode=concatenating
          tunnel: [w1082] -> w1053 mode=concatenating
          n512 = Unbundle By Name(w1085) -> ("double data"=w1084:dbl[][])
          n513 = call "SeperateChanData.vi"("Input (Ch1&2)"=w1084) -> ("Ch1"=w1083:dbl[][], "Ch2"=w1082:dbl[][])
        }
        n514 = for {
          tunnel: w1066 -> [w1081] mode=indexing
          tunnel: [w1080] -> w1042 mode=concatenating
          tunnel: [w1078] -> w1043 mode=concatenating
          n515 = Unbundle By Name(w1081) -> ("double data"=w1079:dbl[][])
          n516 = call "SeperateChanData.vi"("Input (Ch1&2)"=w1079) -> ("Ch1"=w1080:dbl[][], "Ch2"=w1078:dbl[][])
        }
        n517 = call "FLImDAQ_FGV.vi"() -> ("Read data"=w1050:T5)  [unwired: 10 in, 1 out]
        n518 = Unbundle By Name(w1050) -> ("Waveform to Avg"=w1040:i16)
        n519 = for {
          tunnel: w1057 -> [w1077] mode=indexing
          tunnel: [w1076] -> w1049 mode=indexing
          tunnel: [w1075] -> w1047 mode=indexing
          tunnel: [w1074] -> w1045 mode=indexing
          tunnel: [w1073] -> w1041 mode=indexing
          n520 = Unbundle By Name(w1077) -> ("V1"=w1076:dbl, "V2"=w1075:dbl, "V3"=w1074:dbl, "V4"=w1073:dbl)
        }
        n521 = call "DuplicateV(SubVI).vi"("Averaging"=w1040, "V in"=w1049) -> ("V out"=w1048:dbl[])  [unwired: 9 in]
        n522 = Array Size(array=w1042) -> (size(s)=→"data Size":i32[])
        n523 = call "DuplicateV(SubVI).vi"("Averaging"=w1040, "V in"=w1047) -> ("V out"=w1046:dbl[])  [unwired: 9 in]
        n524 = call "DuplicateV(SubVI).vi"("Averaging"=w1040, "V in"=w1045) -> ("V out"=w1044:dbl[])  [unwired: 9 in]
        n525 = call "DuplicateV(SubVI).vi"("Averaging"=w1040, "V in"=w1041) -> ("V out"=w1038:dbl[])  [unwired: 9 in]
        n526 = Bundle By Name(cluster=w1064, "Ch1Data"=w1052, "Ch2Data"=w1053, "Ch3Data"=w1042, "Ch4Data"=w1043, "V1"=w1048, "V2"=w1046, "V3"=w1044, "V4"=w1038) -> (w1065:T23)
        n527 = Merge Errors(w1060, w1059, w1058) -> (w1061:errorcluster)
        n528 = Array Size(array=w1048) -> (size(s)=→"V1 Size":i32)
        n529 = Array Size(array=w1046) -> (size(s)=→"V2 Size":i32)
        n530 = Array Size(array=w1044) -> (size(s)=→"V3 Size":i32)
        n531 = Array Size(array=w1038) -> (size(s)=→"V4 Size":i32)
        n532 = call <vilib>:"Add State(s) to Queue__JKI_lib_State_Machine.vi"("State(s) in (\"\")"=w1072) -> ("States Out"=w1071:string)  [unwired: 14 in]
      }
      frame "Data: saveRunData" {
        w1088 = T38 {"DataPath"=path "", "CaseID"="", "RunID"=0, "Ch1Data"=[], "Ch2Data"=[], "Ch3Data"=[], "Ch4Data"=[], "V1"=[], "V2"=[], "V3"=[], "V4"=[], "LaserRepRate"=0, "WFAverage"=0, "RunStartTime"=0}  # Data cluster
        # "Save FLIm data to disk.\n(Save to LV tdms file format)"
        n533 = Unbundle By Name(w1099) -> ("Pathes.DataPath"=w1095:path, "CaseID"=w1107:string, "IDs.RunID"=w1097:i8, "Ch1Data"=w1106:dbl[][], "Ch2Data"=w1105:dbl[][], "Ch3Data"=w1094:dbl[][], "Ch4Data"=w1087:dbl[][], "V1"=w1089:dbl[], "V2"=w1104:dbl[], "V3"=w1103:dbl[], "V4"=w1086:dbl[])
        n534 = call "FLImDAQ_FGV.vi"() -> ("Read data"=w1092:T5)  [unwired: 10 in, 1 out]
        n535 = Unbundle By Name(w1092) -> ("Waveform to Avg"=w1091:i16)
        n536 = local read "RunStartTime"() -> (w1090:u32)
        n537 = local read "Laser Rep Rate"() -> (w1093:dbl)
        n538 = Increment(x=w1097) -> (x+1=w1096:i8)
        n539 = Bundle By Name(cluster=w1088, "DataPath"=w1095, "CaseID"=w1107, "RunID"=w1096, "Ch1Data"=w1106, "Ch2Data"=w1105, "Ch3Data"=w1094, "Ch4Data"=w1087, "V1"=w1089, "V2"=w1104, "V3"=w1103, "V4"=w1086, "LaserRepRate"=w1093, "WFAverage"=w1091, "RunStartTime"=w1090) -> (w1102:T38)
        n540 = call "SaveRunData(SubVI).vi"("Data cluster"=w1102, "error in (no error)"=w1101) -> ("error out"=w1098:errorcluster)  [unwired: 13 in]
        n541 = flat-sequence {
          tunnel: w1099 -> [w1115]
          tunnel: [w1114] -> w1100
          tunnel: w1098 -> [_]
          frame #0 {
            w1112 = dbl[][] [] ("Ch1Data")
            w1113 = dbl[] [] ("V1")
            # "reset local data"
            n542 = Bundle By Name(cluster=w1115, "Ch1Data"=w1112, "Ch2Data"=w1112, "Ch3Data"=w1112, "Ch4Data"=w1112, "V1"=w1113, "V2"=w1113, "V3"=w1113, "V4"=w1113) -> (w1114:T23)
          }
        }
        n543 = case shown="No Error" w1098 {
          tunnel: ["Run: Increment" "" ("Empty String Constant")] -> w1108
          frame No Error {
          }
          frame Error {
          }
        }
        n544 = call <vilib>:"Add State(s) to Queue__JKI_lib_State_Machine.vi"("State(s) in Front (\"\")"=w1108, "State(s) in (\"\")"=w1111) -> ("States Out"=w1110:string)  [unwired: 13 in]
      }
      frame "Data: Cleanup" {
        # "Cleanup any data and references, here.\n(this is called automatically, by the Macro: Exit)"
        n545 = Unbundle By Name(w1119) -> ("Core.Current VI Reference"=w1122:refnum<vi>)
        n546 = Close Reference(reference=w1122, error in (no error)=w1121) -> (error out=w1120:errorcluster)
        n547 = call <vilib>:"Add State(s) to Queue__JKI_lib_State_Machine.vi"("State(s) in (\"\")"=w1124) -> ("States Out"=w1123:string)  [unwired: 14 in]
      }
      frame "---------- Core ----------" {
        # "Do not put any code in this frame.\n(it is a separator no-op)"
        n548 = call <vilib>:"Add State(s) to Queue__JKI_lib_State_Machine.vi"("State(s) in (\"\")"=w1129) -> ("States Out"=w1128:string)  [unwired: 14 in]
      }
      frame Default {
        w1140 = 42 items=["No error", "Argument error", "Memory is full", "Out of zone", "End of file", "File already open", "Generic file I/O error", "File not found", "File permission error", "Disk is full", "Duplicate path", "Too many files open", "System feature not enabled", "Resource file not found", "Cannot add resource", "Resource not found", "Image not found", "Image memory error", "Pen does not exist", "Config type invalid", "Config token not found", "Config parse error", "Config memory error", "Bad external code format", "Bad external code offset", "External code not present", "Null window", "Destroy window error", "Null menu", "Print aborted", "Bad print record", "Print driver error", "Windows error during printing", "Memory error during printing", "Print dialog error", "Generic print error", "Invalid device refnum", "Device not found", "Device parameter error", "Device unit error", "Cannot open device", "Device call aborted", "Generic error", "Cancelled by user", "Object ID too low", "Object ID too high", "Object not in heap", "Unknown heap", "Unknown object (invalid DefProc)", "Unknown object (DefProc not in table)", "Message out of range", "Invalid (null) method", "Unknown message", "Manager call not supported", "Bad address", "Network operation in progress", "Network operation timed out", "Connection is busy", "Network attribute not supported", "Network error", "Address in use", "System out of memory", "Connection aborted", "Connection refused", "Not connected", "Already connected", "Connection closed", "Initialization error (interapplication manager)", "Bad occurrence", "Wait on unbound occurrence handler", "Occurrence queue overflow", "Datalog type conflict", "Unused", "Unrecognized type (interapplication manager)", "Memory corrupt", "Failed to make temporary DLL", "Old CIN version", "Drag socket not found", "Failed to load drop-object", "Failed to register OLE object", "Failed to release OLE object", "Format specifier type mismatch", "Unknown format specifier", "Too few format specifiers", "Too many format specifiers", "Scan failed", "Newer CIN version", "Error converting to variant", "Runtime menu error", "Password tampered", "Variant attribute not found", "Incompatible variant data type", "Event data is not available", "Event Store is not present", "Occurrence is not found", "Event Queue is not created", "Event info is not available", "Refnum passed is NULL", "Error retrieving Class GUID", "Error retrieving CoClass GUID", "Error retrieving TypeLib GUID.", "Bad built application magic bytes.", "Specific driver is different from the specific driver associated with the Logical Name.", "There is no session opened to the class driver.", "Max Error", "MAX - Error with config objects", "MAX - Error loading configuration", "MAX - Group not supported"]
        # "Current State"
        # "Do not delete, rename, or modify this frame.\n(this is used to capture unhandled states and typos)"
        # "Handle mistyped state name (developer tool)"
        n549 = Format Into String(format string="Software Exception: Unhandled State \"%s\"." ("message"), error in=w1136, w1131) -> (resulting string=w1139:string, error out=w1138:errorcluster)  [unwired: 1 in]
        n550 = call <vilib>:"Error Cluster From Error Code.vi"("show call chain? (False)"=TRUE, "error in (no error)"=w1138, "error message (\"\")"=w1139, "error code (0)"=w1140) -> ("error out"=w1137:errorcluster)  [unwired: 5 in]
        n551 = call <vilib>:"Add State(s) to Queue__JKI_lib_State_Machine.vi"("State(s) in (\"\")"=w1135) -> ("States Out"=w1134:string)  [unwired: 14 in]
      }
      frame "Initialize Core Data" {
        # "Build default path based on the location of project"
        # "Do not delete, rename, or modify this frame.\n(this is used to determine panel behavior on exit)"
        # "originally closed?"
        # "exe?"
        # "If panel starts closed or is an EXE, then close it when we exit"
        n552 = call <vilib>:"Application Directory.vi"() -> ("Application Directory"=w1143:path)
        n553 = property on="Property Node" class="App"() -> ("App.Kind"=w1159:T18)  [unwired: 2 in, 2 out]
        n554 = property on="Property Node" class="VI"() -> ("FP.State"=w1153:T17)  [unwired: 2 in, 2 out]
        n555 = control-ref of="Current VI Reference"() -> (w1154:refnum<vi>)
        n556 = Equal?(x=w1153, y=T17."Closed" ("Front Panel Window:State")) -> (x = y?=w1151:bool)
        n557 = Strip Path(path=w1143) -> (stripped path=w1142:path)  [unwired: 1 out]
        n558 = Equal?(x=w1159, y=T18."Run Time System" ("Application:Kind")) -> (x = y?=w1157:bool)
        n559 = Build Path(base path=w1142, name or relative path="Data") -> (appended path=w1149:path)
        n560 = Build Path(base path=w1143, name or relative path="SystemTemp") -> (appended path=w1146:path)
        n561 = Build Path(base path=w1143, name or relative path="SystemCalibrationFile") -> (appended path=w1144:path)
        n562 = Or(x=w1151, y=w1157) -> (x .or. y?=w1155:bool)
        n563 = Bundle By Name(cluster=w1156, "Core.Current VI Reference"=w1154, "Core.Close Panel on Exit?"=w1155, "DefaultPath"=w1149, "TempPath"=w1146, "CaliPath"=w1144) -> (w1161:T23)
        n564 = call <vilib>:"Add State(s) to Queue__JKI_lib_State_Machine.vi"("State(s) in (\"\")"=w1163) -> ("States Out"=w1162:string)  [unwired: 14 in]
      }
      frame "Error Handler" {
        # "Unhandled Error -- Display it"
        # "Handle any errors here.\nYou can also output any states to clean-up after errors occur"
        # "Clear error"
        n565 = Unbundle By Name(w1164) -> ("code"=w1166:i32)
        n566 = case shown="Default" w1166 {
          tunnel: ["Macro: Exit" w1176 w1182] -> w1165
          tunnel: w1164 -> [w1172 _ _]
          frame Default {
            w1174 = T39 1 items=["no dialog", "OK message", "continue or stop message", "OK message + warnings", "continue/stop + warnings"] ("type of dialog (OK msg:1)")
            n567 = call <vilib>:"General Error Handler.vi"("type of dialog (OK msg:1)"=w1174, "error in (no error)"=w1172) -> ()  [unwired: 9 in, 5 out]
          }
          frame 5002 {
            n568 = Two Button Dialog(message="Laser interlock open! Please close interlock and try again! ", 1:"Safely Shutdown" ("F button name (\"Cancel\")"), 2:"OK" ("T button name (\"OK\")")) -> (T button?=w1177:bool)
            n569 = case shown="True" w1177 {
              tunnel: ["Macro: Exit" "355 Laser: CheckControllerStatus"] -> w1176
              frame False {
              }
              frame True {
              }
            }
          }
          frame 5001 {
            n570 = Two Button Dialog(message="Unable to connect to imaging computer, do you want to run data aquisiton alone? ", 1:"No" ("F button name (\"Cancel\")"), 2:"Yes" ("T button name (\"OK\")")) -> (T button?=w1183:bool)
            n571 = case shown="False" w1183 {
              tunnel: ["Macro: Exit" "" ("Empty String Constant")] -> w1182
              frame False {
              }
              frame True {
              }
            }
          }
        }
        n572 = call <vilib>:"Add State(s) to Queue__JKI_lib_State_Machine.vi"("State(s) in Front (\"\")"=w1165, "State(s) in (\"\")"=w1171) -> ("States Out"=w1170:string)  [unwired: 13 in]
      }
      frame "Exit" {
        # "Do not put any code in this frame.\n(No errors that occur here will be handled.)"
        n573 = call <vilib>:"Add State(s) to Queue__JKI_lib_State_Machine.vi"("State(s) in (\"\")"=w1194) -> ("States Out"=w1193:string)  [unwired: 14 in]
      }
      frame "---------- Case ----------" {
        # "Template Separator\n(You can make a copy of, or modify, this frame)"
        n574 = call <vilib>:"Add State(s) to Queue__JKI_lib_State_Machine.vi"("State(s) in (\"\")"=w1199) -> ("States Out"=w1198:string)  [unwired: 14 in]
      }
      frame "Case: getCaliID" {
        # "Get Calibration file #\n(You can make a copy of, or modify, this frame)"
        n575 = Unbundle By Name(w1200) -> ("Pathes.CaliPath"=w1203:path)
        n576 = call <vilib>:"Recursive File List.vi"("pattern"="*.tdms", "Treat LLBs as Folders?"=FALSE, "Folder Path"=w1203) -> ("All Files in Dir"=w1208:path[])  [unwired: 4 in, 4 out]
        n577 = for {
          tunnel: w1208 -> [w1218] mode=indexing
          tunnel: [w1217] -> w1207 mode=indexing
          tunnel: "Calibration" -> [w1214]
          n578 = Strip Path(path=w1218) -> (name=w1215:string)  [unwired: 1 out]
          n579 = Search and Replace String(input string=w1215, search string=w1214) -> (result string=w1213:string)  [unwired: 6 in, 3 out]
          n580 = Scan From String(format string="%d" ("string"), input string=w1213) -> (output 1=w1217:i32)  [unwired: 3 in, 3 out]
        }
        n581 = Array Max & Min(array=w1207) -> (max value=w1206:i32)  [unwired: 3 out]
        n582 = Bundle By Name(cluster=w1200, "IDs.Cali ID"=w1206) -> (w1201:T23)
        n583 = call <vilib>:"Add State(s) to Queue__JKI_lib_State_Machine.vi"("State(s) in (\"\")"=w1212) -> ("States Out"=w1211:string)  [unwired: 14 in]
      }
      frame "Case: getBGID" {
        # "Get background #\n(You can make a copy of, or modify, this frame)"
        n584 = Unbundle By Name(w1221) -> ("Pathes.BG Path"=w1226:path)
        n585 = call <vilib>:"Recursive File List.vi"("pattern"="*.tdms", "Treat LLBs as Folders?"=FALSE, "Folder Path"=w1226) -> ("All Files in Dir"=w1224:path[])  [unwired: 4 in, 4 out]
        n586 = for {
          tunnel: w1224 -> [w1241] mode=indexing
          tunnel: "Background" ("name or relative path") -> [w1239]
          shift-right: [w1232] -> w1219
          shift-left: 0 -> [w1236]
          n587 = Strip Path(path=w1241) -> (name=w1240:string)  [unwired: 1 out]
          n588 = Search and Replace String(input string=w1240, search string=w1239) -> (number of replacements=w1238:i32)  [unwired: 6 in, 3 out]
          n589 = Greater Than 0?(x=w1238) -> (x > 0?=w1237:bool)
          n590 = Select(t=1, s=w1237, f=0) -> (s? t:f=w1235:i32)
          n591 = Add(x=w1235, y=w1236) -> (x+y=w1232:i32)
        }
        n592 = Bundle By Name(cluster=w1221, "IDs.BG ID"=w1219) -> (w1222:T23)
        n593 = call <vilib>:"Add State(s) to Queue__JKI_lib_State_Machine.vi"("State(s) in (\"\")"=w1231) -> ("States Out"=w1230:string)  [unwired: 14 in]
      }
      frame "Case: getRunID" {
        # "Check folder for run ID\n(You can make a copy of, or modify, this frame)"
        n594 = Unbundle By Name(w1251) -> ("Pathes.DataPath"=w1250:path, "CaseID"=w1246:string)
        n595 = Build Array("Background" ("name or relative path"), "Calibration", "3DScanData" ("element")) -> (w1256:string[])
        n596 = call <vilib>:"Recursive File List.vi"("Folders to Exclude"=w1256, "pattern"="*.tdms", "Treat LLBs as Folders?"=FALSE, "Folder Path"=w1250) -> ("All Files in Dir"=w1247:path[])  [unwired: 3 in, 4 out]
        n597 = for {
          tunnel: w1247 -> [w1265] mode=indexing
          tunnel: [w1264] -> w1253 mode=indexing
          tunnel: w1246 -> [w1261]
          n598 = Strip Path(path=w1265) -> (name=w1262:string)  [unwired: 1 out]
          n599 = Search and Replace String(input string=w1262, search string=w1261) -> (result string=w1260:string)  [unwired: 6 in, 3 out]
          n600 = Scan From String(format string="_%d" ("string"), input string=w1260) -> (output 1=w1264:i32)  [unwired: 3 in, 3 out]
        }
        n601 = Array Max & Min(array=w1253) -> (max value=w1244:i32)  [unwired: 3 out]
        n602 = Bundle By Name(cluster=w1251, "IDs.RunID"=w1244) -> (w1252:T23)
        n603 = call "RunIDFGV.vi"("Error In"=w1242, "RunID in"=w1244) -> ("Error Out"=w1243:errorcluster)  [unwired: 8 in, 1 out]
        n604 = call <vilib>:"Add State(s) to Queue__JKI_lib_State_Machine.vi"("State(s) in (\"\")"=w1259) -> ("States Out"=w1258:string)  [unwired: 14 in]
      }
      frame "Case: CreatFileStruct" {
        # "Creat case file structure"
        n605 = Unbundle By Name(w1279) -> ("DefaultPath"=w1285:path, "CaseID"=w1272:string)
        n606 = Build Path(base path=w1285, name or relative path=w1272) -> (appended path=w1284:path)
        n607 = call <vilib>:"Check if File or Folder Exists.vi"("error in (no error)"=w1278, "path"=w1284) -> ("error out"=w1281:errorcluster, "file or folder exists?"=w1283:bool, "dup path"=w1282:path)  [unwired: 7 in]
        n608 = case shown="True" w1283 {
          tunnel: w1282 -> [w1302 w1310]
          tunnel: w1281 -> [w1300 w1305]
          tunnel: [w1294 w1310] -> w1270
          tunnel: [w1298 w1312] -> w1269
          tunnel: [u32 0 u32 0] -> w1268
          tunnel: [w1296 w1315] -> w1276
          tunnel: "Background" ("name or relative path") -> [w1295 w1307]
          tunnel: "Calibration" -> [w1293 w1306]
          tunnel: [w1289 w1308] -> w1273
          tunnel: w1272 -> [_ _]
          tunnel: ["" ("Empty String Constant") "Case: getRunID\nCase: getBGID\nCase: getCaliID\nUI: Update"] -> w1271
          frame False {
            # "Folder not exist. Creat folders."
            n609 = Create Folder(path (use dialog)=w1302, error in=w1300) -> (created path=w1294:path, error out=w1291:errorcluster)  [unwired: 1 in, 1 out]
            n610 = Build Path(base path=w1294, name or relative path=w1293) -> (appended path=w1292:path)
            n611 = Build Path(base path=w1294, name or relative path=w1295) -> (appended path=w1301:path)
            n612 = Create Folder(path (use dialog)=w1301, error in=w1291) -> (created path=w1296:path, error out=w1297:errorcluster)  [unwired: 1 in, 1 out]
            n613 = Create Folder(path (use dialog)=w1292, error in=w1291) -> (created path=w1289:path, error out=w1290:errorcluster)  [unwired: 1 in, 1 out]
            n614 = Merge Errors(w1297, w1290) -> (w1298:errorcluster)
          }
          frame True {
            # "Folder exsit, check file #"
            n615 = Build Path(base path=w1310, name or relative path=w1306) -> (appended path=w1311:path)
            n616 = Build Path(base path=w1310, name or relative path=w1307) -> (appended path=w1316:path)
            n617 = call <vilib>:"Check if File or Folder Exists.vi"("path"=w1311) -> ("file or folder exists?"=w1309:bool, "dup path"=w1308:path)  [unwired: 8 in, 1 out]
            n618 = call <vilib>:"Check if File or Folder Exists.vi"("path"=w1316) -> ("file or folder exists?"=w1314:bool, "dup path"=w1315:path)  [unwired: 8 in, 1 out]
            n619 = And(x=w1314, y=w1309) -> (x .and. y?=w1313:bool)
            n620 = case shown="False" w1313 {
              tunnel: w1305 -> [_ w1318]
              tunnel: [errorcluster {"status"=TRUE, "code"=5003, "source"="File structure error."} ("error out") w1318] -> w1312
              frame False {
              }
              frame True {
              }
            }
          }
        }
        n621 = Bundle By Name(cluster=w1279, "Pathes.DataPath"=w1270, "Pathes.BG Path"=w1276, "Pathes.CaliPath"=w1273, "IDs.RunID"=w1268, "IDs.BG ID"=w1268, "IDs.Cali ID"=w1268) -> (w1280:T23)
        n622 = call "DataRootPathFGV.vi"("Error In"=w1269, "PathIn"=w1270) -> ("Error Out"=w1267:errorcluster)  [unwired: 8 in, 1 out]
        n623 = call "RunIDFGV.vi"("Error In"=w1267, "RunID in"=w1268) -> ("Error Out"=w1266:errorcluster)  [unwired: 8 in, 1 out]
        n624 = call <vilib>:"Add State(s) to Queue__JKI_lib_State_Machine.vi"("State(s) in Front (\"\")"=w1271, "State(s) in (\"\")"=w1287) -> ("States Out"=w1286:string)  [unwired: 13 in]
      }
      frame "Case: GetID" {
        # "Template Separator\n(You can make a copy of, or modify, this frame)"
        n625 = call "set_subjectID.vi"() -> ("subject_id"=w1319:string)  [unwired: 10 in]
        n626 = Bundle By Name(cluster=w1321, "CaseID"=w1319) -> (w1322:T23)
        n627 = call <vilib>:"Add State(s) to Queue__JKI_lib_State_Machine.vi"("State(s) in (\"\")"=w1325) -> ("States Out"=w1324:string)  [unwired: 14 in]
      }
      frame "---------- DeconEngine ----------" {
        # "start data aquisition and then set irfAligh to ture and decon channel to 1,2 and 3."
        # "Template Separator\n(You can make a copy of, or modify, this frame)"
        n628 = call <vilib>:"Add State(s) to Queue__JKI_lib_State_Machine.vi"("State(s) in (\"\")"=w1330) -> ("States Out"=w1329:string)  [unwired: 14 in]
      }
      frame "DeconEngine: InitDotNet" {
        # "Initialize Dot Net Decon and save the FGV"
        # "Initilize Dot Net \n(You can make a copy of, or modify, this frame)"
        n629 = constructor on="Constructor Node" class="LaguerreDeCon"(error in=w1331) -> (reference out=w1334:refnum<k24>, error out=w1333:errorcluster)  [unwired: 2 in, 1 out]
        n630 = call "DotNetFGV.vi"("Error In"=w1333, "Operation (Read)"=enum16{"Read", "Write"}."Write", "reference in"=w1334) -> ("Error Out"=w1332:errorcluster)  [unwired: 7 in, 1 out]
        n631 = call <vilib>:"Add State(s) to Queue__JKI_lib_State_Machine.vi"("State(s) in (\"\")"=w1339) -> ("States Out"=w1338:string)  [unwired: 14 in]
      }
      frame "DeconEngine: Warmup" {
        # "Warm up parpool\n(You can make a copy of, or modify, this frame)"
        n632 = call "DotNetFGV.vi"("Error In"=w1344) -> ("Error Out"=w1345:errorcluster, "reference out"=w1346:refnum<k24>)  [unwired: 9 in]
        n633 = flat-sequence {
          tunnel: w1344 -> [_]
          tunnel: [w1352] -> w1341
          frame #0 {
            n634 = Tick Count (ms)() -> (millisecond timer value=w1352:u32)
          }
        }
        n635 = invoke class="LaguerreDeCon" method="init_parpool"(reference=w1346, error in=w1345) -> (error out=w1343:errorcluster)  [unwired: 1 in, 2 out]
        n636 = flat-sequence {
          tunnel: w1343 -> [_]
          tunnel: [w1351] -> w1342
          frame #0 {
            n637 = Tick Count (ms)() -> (millisecond timer value=w1351:u32)
          }
        }
        n638 = Subtract(x=w1342, y=w1341) -> (x-y=→"WarmupTime(ms)":u32)
        n639 = call <vilib>:"Add State(s) to Queue__JKI_lib_State_Machine.vi"("State(s) in (\"\")"=w1350) -> ("States Out"=w1349:string)  [unwired: 14 in]
      }
      frame "DeconEngine: loadIRF" {
        # "Load IRF for decon and save to FGV\n(You can make a copy of, or modify, this frame)"
        n640 = Current VI's Path() -> (path=w1370:path)
        n641 = Strip Path(path=w1370) -> (stripped path=w1369:path)  [unwired: 1 out]
        n642 = Build Path(base path=w1369, name or relative path="DotNetDecon") -> (appended path=w1357:path)
        n643 = Build Path(base path=w1357, name or relative path="Channel1.tdms") -> (appended path=w1374:path)
        n644 = Build Path(base path=w1357, name or relative path="Channel3.tdms") -> (appended path=w1359:path)
        n645 = Build Path(base path=w1357, name or relative path="Channel2.tdms") -> (appended path=w1360:path)
        n646 = call "LoadIRF.vi"("error in (no error)"=w1358, "file path"=w1374) -> ("error out"=w1372:errorcluster, "APD"=w1373:T40)  [unwired: 8 in]
        n647 = call "LoadIRF.vi"("error in (no error)"=w1358, "file path"=w1360) -> ("error out"=w1365:errorcluster, "APD"=w1366:T40)  [unwired: 8 in]
        n648 = call "LoadIRF.vi"("error in (no error)"=w1358, "file path"=w1359) -> ("error out"=w1362:errorcluster, "APD"=w1363:T40)  [unwired: 8 in]
        n649 = call "DeConAPD1FGV.vi"("Error In"=w1372, "Operation (Read)"=enum16{"Read", "Write"}."Write", "APDClass in"=w1373) -> ("Error Out"=w1356:errorcluster)  [unwired: 7 in, 1 out]
        n650 = call "DeConAPD2FGV.vi"("Error In"=w1365, "Operation (Read)"=enum16{"Read", "Write"}."Write", "APDClass in"=w1366) -> ("Error Out"=w1355:errorcluster)  [unwired: 7 in, 1 out]
        n651 = call "DeConAPD3FGV.vi"("Error In"=w1362, "Operation (Read)"=enum16{"Read", "Write"}."Write", "APDClass in"=w1363) -> ("Error Out"=w1354:errorcluster)  [unwired: 7 in, 1 out]
        n652 = Merge Errors(w1356, w1355, w1354) -> (w1353:errorcluster)
        n653 = call <vilib>:"Add State(s) to Queue__JKI_lib_State_Machine.vi"("State(s) in (\"\")"=w1380) -> ("States Out"=w1379:string)  [unwired: 14 in]
      }
      frame "DeconEngine: CloseNetRef" {
        # "Template Separator\n(You can make a copy of, or modify, this frame)"
        n654 = call "DotNetFGV.vi"("Error In"=w1381) -> ("Error Out"=w1383:errorcluster, "reference out"=w1384:refnum<k24>)  [unwired: 9 in]
        n655 = Close Reference(reference=w1384, error in (no error)=w1383) -> (error out=w1382:errorcluster)
        n656 = call <vilib>:"Add State(s) to Queue__JKI_lib_State_Machine.vi"("State(s) in (\"\")"=w1388) -> ("States Out"=w1387:string)  [unwired: 14 in]
      }
      frame "DeconEngine: InitilizeMacro" {
        # "start data aquisition and then set irfAligh to ture and decon channel to 1,2 and 3."
        # "Initilize Decon Engine for all channel\n(You can make a copy of, or modify, this frame)"
        n657 = call <vilib>:"Add State(s) to Queue__JKI_lib_State_Machine.vi"("State(s) in Front (\"\")"="DeconEngine: InitializeCh1\nDeconEngine: InitializeCh2\nDeconEngine: InitializeCh3\nDeconEngine: InitializeCh4" ("State(s) in Front (\"\")"), "State(s) in (\"\")"=w1394) -> ("States Out"=w1393:string)  [unwired: 13 in]
      }
      frame "DeconEngine: InitializeCh1" {
        w1416 = refnum<class "LaguerreDeconEngineClass.lvclass"> refnum  # Ch1DeconObj
        # "Initilize Laguerre Deconvolution engine Object\n(You can make a copy of, or modify, this frame)"
        n658 = global read "GlobalVariables.vi" "LastUseiRF"() -> (w1397:T16)
        n659 = call "setLaguerreOrder.vi"("error in (no error)"=w1404, "LaguerreOrder"=u32 12, "LaguerreDeconClass in"=w1416) -> ("error out"=w1413:errorcluster, "LaguerreDeconClass out"=w1414:refnum<class "LaguerreDeconEngineClass.lvclass">)  [unwired: 7 in]
        n660 = Unbundle By Name(w1397) -> ("Ch1 iRF"=w1396:dbl[])
        n661 = call "setDataLength.vi"("error in (no error)"=w1413, "dataLength"=u32 600, "LaguerreDeconClass in"=w1414) -> ("error out"=w1412:errorcluster, "LaguerreDeconClass out"=w1411:refnum<class "LaguerreDeconEngineClass.lvclass">)  [unwired: 7 in]
        n662 = call "setIRF.vi"("error in (no error)"=w1412, "iRF"=w1396, "LaguerreDeconClass in"=w1411) -> ("error out"=w1409:errorcluster, "LaguerreDeconClass out"=w1410:refnum<class "LaguerreDeconEngineClass.lvclass">)  [unwired: 7 in]
        n663 = call "computeAlpha.vi"("error in (no error)"=w1409, "LaguerreDeconClass in"=w1410) -> ("error out"=w1407:errorcluster, "LaguerreDeconClass out"=w1408:refnum<class "LaguerreDeconEngineClass.lvclass">)  [unwired: 8 in]
        n664 = call "dataInitilize.vi"("error in (no error)"=w1407, "LaguerreDeconClass in"=w1408) -> ("error out"=w1405:errorcluster, "LaguerreDeconClass out"=w1406:refnum<class "LaguerreDeconEngineClass.lvclass">)  [unwired: 8 in]
        n665 = call "computeDeconMatrix.vi"("error in (no error)"=w1405, "LaguerreDeconClass in"=w1406) -> ("error out"=w1401:errorcluster, "LaguerreDeconClass out"=w1403:refnum<class "LaguerreDeconEngineClass.lvclass">)  [unwired: 8 in]
        n666 = call "Ch1DeconEngineFGV.vi"("Error In"=w1401, "action(read)"=enum16{"write", "read"}."write" ("action"), "Ch1DeconEngine in"=w1403) -> ("Error Out"=w1400:errorcluster)  [unwired: 7 in, 1 out]
        n667 = call <vilib>:"Add State(s) to Queue__JKI_lib_State_Machine.vi"("State(s) in (\"\")"=w1418) -> ("States Out"=w1417:string)  [unwired: 14 in]
      }
      frame "DeconEngine: InitializeCh2" {
        w1440 = refnum<class "LaguerreDeconEngineClass.lvclass"> refnum  # Ch2DeconObj
        # "Initilize Laguerre Deconvolution engine Object\n(You can make a copy of, or modify, this frame)"
        n668 = global read "GlobalVariables.vi" "LastUseiRF"() -> (w1421:T16)
        n669 = call "setLaguerreOrder.vi"("error in (no error)"=w1428, "LaguerreOrder"=u32 12, "LaguerreDeconClass in"=w1440) -> ("error out"=w1437:errorcluster, "LaguerreDeconClass out"=w1438:refnum<class "LaguerreDeconEngineClass.lvclass">)  [unwired: 7 in]
        n670 = Unbundle By Name(w1421) -> ("Ch2 iRF"=w1420:dbl[])
        n671 = call "setDataLength.vi"("error in (no error)"=w1437, "dataLength"=u32 600, "LaguerreDeconClass in"=w1438) -> ("error out"=w1436:errorcluster, "LaguerreDeconClass out"=w1435:refnum<class "LaguerreDeconEngineClass.lvclass">)  [unwired: 7 in]
        n672 = call "setIRF.vi"("error in (no error)"=w1436, "iRF"=w1420, "LaguerreDeconClass in"=w1435) -> ("error out"=w1433:errorcluster, "LaguerreDeconClass out"=w1434:refnum<class "LaguerreDeconEngineClass.lvclass">)  [unwired: 7 in]
        n673 = call "computeAlpha.vi"("error in (no error)"=w1433, "LaguerreDeconClass in"=w1434) -> ("error out"=w1431:errorcluster, "LaguerreDeconClass out"=w1432:refnum<class "LaguerreDeconEngineClass.lvclass">)  [unwired: 8 in]
        n674 = call "dataInitilize.vi"("error in (no error)"=w1431, "LaguerreDeconClass in"=w1432) -> ("error out"=w1429:errorcluster, "LaguerreDeconClass out"=w1430:refnum<class "LaguerreDeconEngineClass.lvclass">)  [unwired: 8 in]
        n675 = call "computeDeconMatrix.vi"("error in (no error)"=w1429, "LaguerreDeconClass in"=w1430) -> ("error out"=w1425:errorcluster, "LaguerreDeconClass out"=w1427:refnum<class "LaguerreDeconEngineClass.lvclass">)  [unwired: 8 in]
        n676 = call "Ch2DeconEngineFGV.vi"("Error In"=w1425, "action(read)"=enum16{"write", "read"}."write" ("action"), "Ch2DeconEngine in"=w1427) -> ("Error Out"=w1424:errorcluster)  [unwired: 7 in, 1 out]
        n677 = call <vilib>:"Add State(s) to Queue__JKI_lib_State_Machine.vi"("State(s) in (\"\")"=w1442) -> ("States Out"=w1441:string)  [unwired: 14 in]
      }
      frame "DeconEngine: InitializeCh3" {
        w1444 = refnum<class "LaguerreDeconEngineClass.lvclass"> refnum  # Ch3DeconObj
        # "Initilize Laguerre Deconvolution engine Object\n(You can make a copy of, or modify, this frame)"
        n678 = global read "GlobalVariables.vi" "LastUseiRF"() -> (w1446:T16)
        n679 = call "setLaguerreOrder.vi"("error in (no error)"=w1453, "LaguerreOrder"=u32 12, "LaguerreDeconClass in"=w1444) -> ("error out"=w1462:errorcluster, "LaguerreDeconClass out"=w1463:refnum<class "LaguerreDeconEngineClass.lvclass">)  [unwired: 7 in]
        n680 = Unbundle By Name(w1446) -> ("Ch3 iRF"=w1445:dbl[])
        n681 = call "setDataLength.vi"("error in (no error)"=w1462, "dataLength"=600, "LaguerreDeconClass in"=w1463) -> ("error out"=w1461:errorcluster, "LaguerreDeconClass out"=w1460:refnum<class "LaguerreDeconEngineClass.lvclass">)  [unwired: 7 in]
        n682 = call "setIRF.vi"("error in (no error)"=w1461, "iRF"=w1445, "LaguerreDeconClass in"=w1460) -> ("error out"=w1458:errorcluster, "LaguerreDeconClass out"=w1459:refnum<class "LaguerreDeconEngineClass.lvclass">)  [unwired: 7 in]
        n683 = call "computeAlpha.vi"("error in (no error)"=w1458, "LaguerreDeconClass in"=w1459) -> ("error out"=w1456:errorcluster, "LaguerreDeconClass out"=w1457:refnum<class "LaguerreDeconEngineClass.lvclass">)  [unwired: 8 in]
        n684 = call "dataInitilize.vi"("error in (no error)"=w1456, "LaguerreDeconClass in"=w1457) -> ("error out"=w1454:errorcluster, "LaguerreDeconClass out"=w1455:refnum<class "LaguerreDeconEngineClass.lvclass">)  [unwired: 8 in]
        n685 = call "computeDeconMatrix.vi"("error in (no error)"=w1454, "LaguerreDeconClass in"=w1455) -> ("error out"=w1450:errorcluster, "LaguerreDeconClass out"=w1452:refnum<class "LaguerreDeconEngineClass.lvclass">)  [unwired: 8 in]
        n686 = call "Ch3DeconEngineFGV.vi"("Error In"=w1450, "action(read)"=enum16{"write", "read"}."write" ("action"), "Ch3DeconEngine in"=w1452) -> ("Error Out"=w1449:errorcluster)  [unwired: 7 in, 1 out]
        n687 = call <vilib>:"Add State(s) to Queue__JKI_lib_State_Machine.vi"("State(s) in (\"\")"=w1466) -> ("States Out"=w1465:string)  [unwired: 14 in]
      }
      frame "DeconEngine: InitializeCh4" {
        w1468 = refnum<class "LaguerreDeconEngineClass.lvclass"> refnum  # Ch3DeconObj
        # "Initilize Laguerre Deconvolution engine Object\n(You can make a copy of, or modify, this frame)"
        n688 = global read "GlobalVariables.vi" "LastUseiRF"() -> (w1470:T16)
        n689 = call "setLaguerreOrder.vi"("error in (no error)"=w1477, "LaguerreOrder"=u32 12, "LaguerreDeconClass in"=w1468) -> ("error out"=w1486:errorcluster, "LaguerreDeconClass out"=w1487:refnum<class "LaguerreDeconEngineClass.lvclass">)  [unwired: 7 in]
        n690 = Unbundle By Name(w1470) -> ("Ch4 iRF"=w1469:dbl[])
        n691 = call "setDataLength.vi"("error in (no error)"=w1486, "dataLength"=u32 600, "LaguerreDeconClass in"=w1487) -> ("error out"=w1485:errorcluster, "LaguerreDeconClass out"=w1484:refnum<class "LaguerreDeconEngineClass.lvclass">)  [unwired: 7 in]
        n692 = call "setIRF.vi"("error in (no error)"=w1485, "iRF"=w1469, "LaguerreDeconClass in"=w1484) -> ("error out"=w1482:errorcluster, "LaguerreDeconClass out"=w1483:refnum<class "LaguerreDeconEngineClass.lvclass">)  [unwired: 7 in]
        n693 = call "computeAlpha.vi"("error in (no error)"=w1482, "LaguerreDeconClass in"=w1483) -> ("error out"=w1480:errorcluster, "LaguerreDeconClass out"=w1481:refnum<class "LaguerreDeconEngineClass.lvclass">)  [unwired: 8 in]
        n694 = call "dataInitilize.vi"("error in (no error)"=w1480, "LaguerreDeconClass in"=w1481) -> ("error out"=w1478:errorcluster, "LaguerreDeconClass out"=w1479:refnum<class "LaguerreDeconEngineClass.lvclass">)  [unwired: 8 in]
        n695 = call "computeDeconMatrix.vi"("error in (no error)"=w1478, "LaguerreDeconClass in"=w1479) -> ("error out"=w1474:errorcluster, "LaguerreDeconClass out"=w1476:refnum<class "LaguerreDeconEngineClass.lvclass">)  [unwired: 8 in]
        n696 = call "Ch4DeconEngineFGV.vi"("Error In"=w1474, "action(read)"=enum16{"write", "read"}."write" ("action"), "Ch3DeconEngine in"=w1476) -> ("Error Out"=w1473:errorcluster)  [unwired: 7 in, 1 out]
        n697 = call <vilib>:"Add State(s) to Queue__JKI_lib_State_Machine.vi"("State(s) in (\"\")"=w1490) -> ("States Out"=w1489:string)  [unwired: 14 in]
      }
      frame "---------- Digitizer ----------" {
        # "Template Separator\n(You can make a copy of, or modify, this frame)"
        n698 = call <vilib>:"Add State(s) to Queue__JKI_lib_State_Machine.vi"("State(s) in (\"\")"=w1495) -> ("States Out"=w1494:string)  [unwired: 14 in]
      }
      frame "Digitizer: Initialize" {
        # "reset digitizer to everytime the system runs"
        # "reset digitizer to everytime the system runs"
        # "Initialize digitizer.\nInitialize both digitizer and update status."
        n699 = call "FLImDAQ_FGV.vi"("error in (no error)"=w1503) -> ("error out"=w1497:errorcluster, "Read data"=w1502:T5)  [unwired: 9 in]
        n700 = Unbundle By Name(w1505) -> ("SysConfigCluster.Ch1Enable?"=w1510:bool, "SysConfigCluster.Ch2Enable?"=w1509:bool, "SysConfigCluster.Ch3Enable?"=w1507:bool)
        n701 = Unbundle By Name(w1502) -> ("Digitizer 1"=w1498:refnum<k15>, "Digitizer 2"=w1501:refnum<k15>)
        n702 = property on="Digitizer" class="Bool (strict)"("Blinking"=TRUE) -> ()  [unwired: 2 in, 2 out]
        n703 = Or(x=w1510, y=w1509) -> (x .or. y?=w1508:bool)
        n704 = case shown="True" w1508 {
          tunnel: w1497 -> [w1518 w1521]
          tunnel: [w1518 w1520] -> w1499
          tunnel: w1498 -> [_ w1522]
          frame False {
          }
          frame True {
            n705 = call <instrlib>:"niScope Initialize.vi"("resource name"=w1522, "reset device"=TRUE, "error in"=w1521) -> ("error out"=w1520:errorcluster)  [unwired: 11 in, 1 out]
          }
        }
        n706 = case shown="True" w1507 {
          tunnel: w1497 -> [w1513 w1515]
          tunnel: [w1513 w1517] -> w1504
          tunnel: w1501 -> [_ w1516]
          frame False {
          }
          frame True {
            n707 = call <instrlib>:"niScope Initialize.vi"("resource name"=w1516, "reset device"=TRUE, "error in"=w1515) -> ("error out"=w1517:errorcluster)  [unwired: 11 in, 1 out]
          }
        }
        n708 = Merge Errors(w1499, w1504) -> (w1496:errorcluster)
        n709 = call <vilib>:"Add State(s) to Queue__JKI_lib_State_Machine.vi"("State(s) in (\"\")"=w1512) -> ("States Out"=w1511:string)  [unwired: 14 in]
      }
      frame "Digitizer: Config" {
        # "Synchronize is taking time ~3s."
        # "Config  digitizer\nCall subVi to config digitizer"
        n710 = call "FLImDAQ_FGV.vi"() -> ("Read data"=w1540:T5)  [unwired: 10 in, 1 out]
        n711 = Unbundle By Name(w1549) -> ("SysConfigCluster.Ch1Enable?"=w1557:bool, "SysConfigCluster.Ch2Enable?"=w1556:bool, "SysConfigCluster.Ch3Enable?"=w1554:bool, "FLImDAQ"=w1551:T30)
        n712 = Unbundle By Name(w1540) -> ("Digitizer 1"=w1543:refnum<k15>, "Digitizer 2"=w1542:refnum<k15>)
        n713 = property on="Digitizer" class="Bool (strict)"(error in=w1544, "Blinking"=TRUE) -> (error out=w1545:errorcluster)  [unwired: 1 in, 1 out]
        n714 = Or(x=w1557, y=w1556) -> (x .or. y?=w1555:bool)
        n715 = case shown="True" w1555 {
          tunnel: w1551 -> [_ w1570]
          tunnel: w1545 -> [w1566 w1569]
          tunnel: [w1566 w1568] -> w1552
          tunnel: w1543 -> [_ w1567]
          frame False {
          }
          frame True {
            n716 = call "DigitizerConfig.vi"("error in (no error)"=w1569, "FLImDAQ"=w1570, "IVI Refnum in"=w1567) -> ("error out"=w1568:errorcluster)  [unwired: 7 in, 1 out]
          }
        }
        n717 = case shown="True" w1554 {
          tunnel: w1551 -> [_ w1565]
          tunnel: w1552 -> [w1560 w1564]
          tunnel: [w1560 w1563] -> w1528
          tunnel: w1542 -> [_ w1561]
          frame False {
          }
          frame True {
            n718 = call "DigitizerConfig.vi"("Config Trigger? (T)"=FALSE ("Config Trigge(T)r:"), "error in (no error)"=w1564, "FLImDAQ"=w1565, "IVI Refnum in"=w1561) -> ("error out"=w1563:errorcluster)  [unwired: 6 in, 1 out]
          }
        }
        n719 = call "Digitizer1_FGV.vi"("error in (no error)"=w1528) -> ("error out"=w1538:errorcluster, "Read data"=w1539:refnum<k15>)  [unwired: 9 in]
        n720 = call <instrlib>:"niScope Get Session Reference.vi"("instrument handle"=w1539, "error in"=w1538) -> ("session reference"=w1532:refnum<k20>, "error out"=w1530:errorcluster)  [unwired: 11 in, 1 out]
        n721 = call "Digitizer2_FGV.vi"("error in (no error)"=w1530) -> ("error out"=w1536:errorcluster, "Read data"=w1537:refnum<k15>)  [unwired: 9 in]
        n722 = call <instrlib>:"niScope Get Session Reference.vi"("instrument handle"=w1537, "error in"=w1536) -> ("session reference"=w1531:refnum<k20>, "error out"=w1529:errorcluster)  [unwired: 11 in, 1 out]
        n723 = Build Array(w1532, w1531) -> (w1535:refnum<k20>[])
        n724 = call <instrlib>:"niTClk Configure For Homogeneous Triggers.vi"("error in (no error)"=w1529, "sessions"=w1535) -> ("error out"=w1534:errorcluster, "sessions out"=w1533:refnum<k20>[])  [unwired: 8 in]
        n725 = call <instrlib>:"niTClk Synchronize.vi"("error in (no error)"=w1534, "sessions"=w1533) -> ("error out"=w1527:errorcluster, "sessions out"=w1525:refnum<k20>[])  [unwired: 8 in]
        n726 = call <userlib>:"Wait (ms)__ogtk.vi"("error in (no error)"=w1527, "milliseconds to wait"=u32 1500) -> ("error out"=w1523:errorcluster)  [unwired: 8 in, 1 out]
        n727 = Unbundle By Name(w1523) -> ("status"=w1548:bool)
        n728 = Not(x=w1548) -> (.not. x?=w1547:bool)
        n729 = Bundle By Name(cluster=w1549, "System Status.Digitizer"=w1547, "niTClk sessions"=w1525) -> (w1550:T23)
        n730 = property on="Digitizer" class="Bool (strict)"(error in=w1523, "Blinking"=FALSE) -> (error out=w1541:errorcluster)  [unwired: 1 in, 1 out]
        n731 = call <vilib>:"Add State(s) to Queue__JKI_lib_State_Machine.vi"("State(s) in (\"\")"=w1559) -> ("States Out"=w1558:string)  [unwired: 14 in]
      }
      frame "Digitizer: Start" {
        # "send trigger to start acquisition loop"
        # "initilize aquisition"
        # "Start Digitizer\n(TClk start)"
        n732 = Unbundle By Name(w1578) -> ("niTClk sessions"=w1577:refnum<k20>[])
        n733 = call <instrlib>:"niTClk Initiate.vi"("error in (no error)"=w1571, "sessions"=w1577) -> ("error out"=w1573:errorcluster)  [unwired: 8 in, 1 out]
        n734 = Generate User Event(priority (normal)=usereventprio."high priority", user event=w1574, event data cluster=TRUE ("event data"), error in=w1573) -> (error out=w1572:errorcluster)  [unwired: 1 out]
        n735 = call <vilib>:"Add State(s) to Queue__JKI_lib_State_Machine.vi"("State(s) in (\"\")"=w1581) -> ("States Out"=w1580:string)  [unwired: 14 in]
      }
      frame "Digitizer: Abort" {
        # "Template Separator\n(You can make a copy of, or modify, this frame)"
        n736 = call "Digitizer1_FGV.vi"("error in (no error)"=w1585, "Operation (Read)"=enum16{"Write", "Read"}."Read" ("Operation")) -> ("error out"=w1592:errorcluster, "Read data"=w1589:refnum<k15>)  [unwired: 8 in]
        n737 = call "Digitizer2_FGV.vi"("error in (no error)"=w1585, "Operation (Read)"=enum16{"Write", "Read"}."Read" ("Operation")) -> ("error out"=w1588:errorcluster, "Read data"=w1590:refnum<k15>)  [unwired: 8 in]
        n738 = Bundle By Name(cluster=w1582, "SysRunning?"=FALSE ("System Status")) -> (w1583:T23)
        n739 = call <instrlib>:"niScope Abort.vi"("instrument handle"=w1589, "error in"=w1592) -> ("error out"=w1594:errorcluster)  [unwired: 12 in, 1 out]
        n740 = call <instrlib>:"niScope Abort.vi"("instrument handle"=w1590, "error in"=w1588) -> ("error out"=w1593:errorcluster)  [unwired: 12 in, 1 out]
        n741 = Merge Errors(w1594, w1593) -> (w1586:errorcluster)
        n742 = call <vilib>:"Add State(s) to Queue__JKI_lib_State_Machine.vi"("State(s) in (\"\")"=w1597) -> ("States Out"=w1596:string)  [unwired: 14 in]
      }
      frame "Digitizer: checkTemp" {
        w1600 = 65.0 ("y")
        w1605 = enum16{"Write", "Read"}."Read" ("Operation")
        # "Template Separator\n(You can make a copy of, or modify, this frame)"
        n743 = call "Digitizer1_FGV.vi"("Operation (Read)"=w1605) -> ("error out"=w1606:errorcluster, "Read data"=w1607:refnum<k15>)  [unwired: 9 in]
        n744 = call "Digitizer2_FGV.vi"("Operation (Read)"=w1605) -> ("error out"=w1603:errorcluster, "Read data"=w1604:refnum<k15>)  [unwired: 9 in]
        n745 = property on="Property Node" class="niScope"(reference=w1604, error in=w1603) -> ("Device Temperature"=w1601:dbl)  [unwired: 2 out]
        "Dig2 Temp" <- w1601
        n746 = property on="Property Node" class="niScope"(reference=w1607, error in=w1606) -> ("Device Temperature"=w1602:dbl)  [unwired: 2 out]
        "Dig1 Temp" <- w1602
        n747 = Greater?(x=w1602, y=w1600) -> (0:w1599:bool)
        n748 = Greater?(x=w1601, y=w1600) -> (0:w1598:bool)
        n749 = case shown="True" w1599 {
          frame False {
          }
          frame True {
            n750 = One Button Dialog(message="Digitizer 1 over heating!", button name ("OK")="OK") -> ()  [unwired: 1 out]
          }
        }
        n751 = case shown="True" w1598 {
          frame False {
          }
          frame True {
            n752 = One Button Dialog(message="Digitizer 2 over heating!", button name ("OK")="OK") -> ()  [unwired: 1 out]
          }
        }
        n753 = call <vilib>:"Add State(s) to Queue__JKI_lib_State_Machine.vi"("State(s) in (\"\")"=w1612) -> ("States Out"=w1611:string)  [unwired: 14 in]
      }
      frame "Digitizer: Close" {
        # "Close Digitizer"
        n754 = call "Digitizer1_FGV.vi"("error in (no error)"=w1622, "Operation (Read)"=enum16{"Write", "Read"}."Read" ("Operation")) -> ("error out"=w1624:errorcluster, "Read data"=w1628:refnum<k15>)  [unwired: 8 in]
        n755 = call "Digitizer2_FGV.vi"("error in (no error)"=w1622, "Operation (Read)"=enum16{"Write", "Read"}."Read" ("Operation")) -> ("error out"=w1623:errorcluster, "Read data"=w1626:refnum<k15>)  [unwired: 8 in]
        n756 = call <instrlib>:"niScope Close.vi"("instrument handle"=w1628, "error in"=w1624) -> ("error out"=w1621:errorcluster)  [unwired: 13 in]
        n757 = call <instrlib>:"niScope Close.vi"("instrument handle"=w1626, "error in"=w1623) -> ("error out"=w1620:errorcluster)  [unwired: 13 in]
        n758 = Merge Errors(w1621, w1620) -> (w1619:errorcluster)
        n759 = Unbundle By Name(w1619) -> ("status"=w1618:bool)
        n760 = Bundle By Name(cluster=w1629, "System Status.Digitizer"=w1618) -> (w1630:T23)
        n761 = call <vilib>:"Add State(s) to Queue__JKI_lib_State_Machine.vi"("State(s) in (\"\")"=w1632) -> ("States Out"=w1631:string)  [unwired: 14 in]
      }
      frame "---------- LabJack ----------" {
        # "Template Separator\n(You can make a copy of, or modify, this frame)"
        n762 = call <vilib>:"Add State(s) to Queue__JKI_lib_State_Machine.vi"("State(s) in (\"\")"=w1637) -> ("States Out"=w1636:string)  [unwired: 14 in]
      }
      frame "LabJack: checkPedal" {
        # "Template Separator\n(You can make a copy of, or modify, this frame)"
        n763 = Unbundle By Name(w1638) -> ("LJ Pinout.Foot Pedal"=w1642:string)
        n764 = call "LabJack_FGV.vi"("Operation(Read)"=enum16{"Write", "Read"}."Read" ("Operation"), "error in (no error)"=w1640) -> ("error out"=w1644:errorcluster, "Read data"=w1645:i32)  [unwired: 8 in]
        n765 = call "LJM_eReadName.vi"("Handle In"=w1645, "Name"=w1642, "error in"=w1644) -> ("Value"=w1643:dbl, "error out"=w1641:errorcluster)  [unwired: 10 in, 1 out]
        n766 = case shown="1" w1643 {
          tunnel: w1638 -> [w1650 w1653]
          tunnel: [w1650 w1651] -> w1639
          frame 0, Default {
          }
          frame 1 {
            # "If Pedal pressed"
            n767 = Tick Count (ms)() -> (millisecond timer value=w1657:u32)
            n768 = Unbundle By Name(w1653) -> ("Last Trigger"=w1652:u32)
            n769 = Subtract(x=w1657, y=w1652) -> (x-y=w1656:u32)
            n770 = Greater Or Equal?(x=w1656, y=u32 2000) -> (x >= y?=w1654:bool)
            n771 = case shown="True" w1654 {
              tunnel: w1653 -> [w1658 w1659]
              tunnel: w1652 -> [_ _]
              tunnel: [w1658 w1660] -> w1651
              frame False {
              }
              frame True {
                n772 = Tick Count (ms)() -> (millisecond timer value=w1661:u32)
                n773 = Unbundle By Name(w1659) -> ("SysRunning?"=w1662:bool)
                n774 = case shown="False" w1662 {
                  frame False {
                    n775 = property on="StartButton" class="Bool (strict)"("Val(Sgnl)"=TRUE ("Value (Signaling)")) -> ()  [unwired: 2 in, 2 out]
                  }
                  frame True {
                    n776 = property on="StopButton" class="Bool (strict)"("Val(Sgnl)"=TRUE ("Value (Signaling)")) -> ()  [unwired: 2 in, 2 out]
                  }
                }
                n777 = Bundle By Name(cluster=w1659, "Last Trigger"=w1661) -> (w1660:T23)
              }
            }
          }
        }
        n778 = call <vilib>:"Add State(s) to Queue__JKI_lib_State_Machine.vi"("State(s) in (\"\")"=w1649) -> ("States Out"=w1648:string)  [unwired: 14 in]
      }
      frame "LabJack: ZeroV" {
        # "Just Zero V\nDO not update FGV and front panel\nWIll resume from last V"
        # "set bias to 0"
        # "Zero APD bias\n(You can make a copy of, or modify, this frame)"
        n779 = Unbundle By Name(w1667) -> ("LJ Pinout.Ch1 Bias"=w1672:string, "LJ Pinout.Ch2 Bias"=w1671:string, "LJ Pinout.Ch3 Bias"=w1670:string)
        n780 = Build Array(w1672, w1671, w1670) -> (w1669:string[])
        n781 = call "LabJack_FGV.vi"("Operation(Read)"=enum16{"Write", "Read"}."Read" ("Operation"), "error in (no error)"=w1666) -> ("error out"=w1673:errorcluster, "Read data"=w1674:i32)  [unwired: 8 in]
        n782 = call "LJM_eWriteNames.vi"("Handle In"=w1674, "aNames"=w1669, "aValuesIn"=dbl[] [0.0, 0.0, 0.0], "error in"=w1673) -> ("error out"=w1665:errorcluster)  [unwired: 9 in, 2 out]
        n783 = call <vilib>:"Add State(s) to Queue__JKI_lib_State_Machine.vi"("State(s) in (\"\")"=w1678) -> ("States Out"=w1677:string)  [unwired: 14 in]
      }
      frame "LabJack: SetV" {
        w1685 = enum16{"write", "read"}."read" ("action (write)")
        # "set bias to user specifid"
        # "Set APD bias\n(You can make a copy of, or modify, this frame)"
        n784 = Unbundle By Name(w1694) -> ("LJ Pinout.Ch1 Bias"=w1698:string, "LJ Pinout.Ch2 Bias"=w1697:string, "LJ Pinout.Ch3 Bias"=w1696:string, "LJ Pinout.Ch4 Bias"=w1688:string)
        n785 = call "V2FGV.vi"("Error In"=w1684, "action(write)"=w1685) -> ("Error Out"=w1682:errorcluster, "V2 out"=w1690:dbl)  [unwired: 8 in]
        n786 = call "V4FGV.vi"("Error In"=w1684, "action(write)"=w1685) -> ("Error Out"=w1680:errorcluster, "V3 out"=w1686:dbl)  [unwired: 8 in]
        n787 = call "V1FGV.vi"("Error In"=w1684, "action (write)"=w1685) -> ("Error Out"=w1683:errorcluster, "V1 out"=w1687:dbl)  [unwired: 8 in]
        n788 = call "V3FGV.vi"("Error In"=w1684, "action(write)"=w1685) -> ("Error Out"=w1681:errorcluster, "V3 out"=w1689:dbl)  [unwired: 8 in]
        n789 = local write "V 3"(w1689) -> ()
        n790 = local write "V 2"(w1690) -> ()
        n791 = local write "V 4"(w1686) -> ()
        n792 = local write "V 1"(w1687) -> ()
        n793 = Build Array(w1698, w1697, w1696, w1688) -> (w1695:string[])
        n794 = call "LabJack_FGV.vi"("Operation(Read)"=enum16{"Write", "Read"}."Read" ("Operation"), "error in (no error)"=w1684) -> ("error out"=w1699:errorcluster, "Read data"=w1700:i32)  [unwired: 8 in]
        n795 = Build Array(w1687, w1690, w1689, w1686) -> (w1691:dbl[])
        n796 = call "LJM_eWriteNames.vi"("Handle In"=w1700, "aNames"=w1695, "aValuesIn"=w1691, "error in"=w1699) -> ("error out"=w1692:errorcluster)  [unwired: 9 in, 2 out]
        n797 = Merge Errors(w1683, w1682, w1681, w1680) -> (w1679:errorcluster)
        n798 = call <vilib>:"Add State(s) to Queue__JKI_lib_State_Machine.vi"("State(s) in (\"\")"=w1704) -> ("States Out"=w1703:string)  [unwired: 14 in]
        n799 = Merge Errors(w1679, w1692) -> (w1693:errorcluster)
      }
      frame "LabJack: Open" {
        # "Initialize LabJack T7\nEstablish connection and initialize pins"
        n800 = call "LJ_Open.vi"("error in"=w1714, "DeviceType"="LJM_dtT7") -> ("error out"=w1711:errorcluster, "Success?"=w1712:bool, "Handle Out"=w1706:i32)  [unwired: 7 in]
        n801 = call "LabJack_FGV.vi"("Operation(Read)"=enum16{"Write", "Read"}."Write" ("Operation"), "error in (no error)"=w1711, "Write data"=w1706) -> ("error out"=w1708:errorcluster)  [unwired: 7 in, 1 out]
        n802 = Bundle By Name(cluster=w1709, "System Status.Labjack"=w1712) -> (w1713:T23)
        n803 = call <vilib>:"Add State(s) to Queue__JKI_lib_State_Machine.vi"("State(s) in (\"\")"=w1716) -> ("States Out"=w1715:string)  [unwired: 14 in]
      }
      frame "LabJack: SetDefaultSub" {
        w1726 = enum16{"write", "read"}."write" ("action")
        w1727 = 0.0 ("V1 in")
        w1740 = "_EF_ENABLE" ("string")
        # "1. Disable PWM\n2. Set all V to 0\n3. Set 355 relay to open\n4. Set LED to off"
        # "read once to set DIO to input"
        # "set all initila V to 0. Set footpedal to input. Set PWM to low. Set laser relay to open. Set LEDs to yellow."
        # "Set Labjack to correct input and output state and initial values"
        n804 = disable-structure shown="Disabled" {
          frame Disabled {
            (unwired) dbl[] [0.0, 0.0, 0.0, 0.0, 0.0, 0.0, 0.0, 0.0, 0.0] ("aValuesIn")
          }
          frame Enabled {
          }
        }
        n805 = Unbundle By Name(w1737) -> ("LJ Pinout.355 PWM"=w1742:string, "LJ Pinout.AimingBeam PWM"=w1741:string, "LJ Pinout.Ch1 Bias"=w1747:string, "LJ Pinout.Ch2 Bias"=w1717:string, "LJ Pinout.Ch3 Bias"=w1751:string, "LJ Pinout.Ch4 Bias"=w1731:string, "LJ Pinout.Laser Start/Stop"=w1750:string, "LJ Pinout.Red LED"=w1749:string, "LJ Pinout.Green LED"=w1748:string)
        n806 = call "V1FGV.vi"("Error In"=w1735, "action (write)"=w1726, "V1 in"=w1727) -> ("Error Out"=w1730:errorcluster, "V1 out"=w1734:dbl)  [unwired: 7 in]
        n807 = local write "V 1"(w1734) -> ()
        n808 = call "V2FGV.vi"("Error In"=w1730, "action(write)"=w1726, "V2 in"=w1727) -> ("Error Out"=w1729:errorcluster, "V2 out"=w1733:dbl)  [unwired: 7 in]
        n809 = call "LabJack_FGV.vi"("Operation(Read)"=enum16{"Write", "Read"}."Read" ("Operation"), "error in (no error)"=w1735) -> ("error out"=w1723:errorcluster, "Read data"=w1745:i32)  [unwired: 8 in]
        n810 = Concatenate Strings(w1742, w1740) -> (w1739:string)
        n811 = Concatenate Strings(w1741, w1740) -> (w1738:string)
        n812 = local write "V 2"(w1733) -> ()
        n813 = call "V3FGV.vi"("Error In"=w1729, "action(write)"=w1726, "V3 in"=w1727) -> ("Error Out"=w1728:errorcluster, "V3 out"=w1732:dbl)  [unwired: 7 in]
        n814 = Build Array(w1739, w1738, w1747, w1717, w1751, w1731, w1750, w1749, w1748) -> (w1721:string[])
        n815 = local write "V 3"(w1732) -> ()
        n816 = call "V4FGV.vi"("Error In"=w1728, "action(write)"=w1726, "V3 in"=w1727) -> ("Error Out"=w1724:errorcluster, "V3 out"=w1725:dbl)  [unwired: 7 in]
        n817 = Array Size(array=w1721) -> (size(s)=w1720:i32)
        n818 = local write "V 4"(w1725) -> ()
        n819 = Initialize Array(0.0 ("element"), w1720) -> (w1718:dbl[])
        n820 = Unbundle By Name(w1737) -> ("LJ Pinout.Foot Pedal"=w1736:string)
        n821 = call "LJM_eWriteNames.vi"("Handle In"=w1745, "aNames"=w1721, "aValuesIn"=w1718, "error in"=w1723) -> ("Handle Out"=w1744:i32, "error out"=w1743:errorcluster)  [unwired: 9 in, 1 out]
        n822 = call "LJM_eReadName.vi"("Handle In"=w1744, "Name"=w1736, "error in"=w1743) -> ("error out"=w1722:errorcluster)  [unwired: 10 in, 2 out]
        n823 = case shown="Error .." w1722 {
          frame No Error {
            # "no error"
          }
          frame Error {
            # "handle error"
            n824 = One Button Dialog(message="Labjack error! The pin assignment is likely wrong. Please check pin setting of Labjack. Program will terminate.", button name ("OK")="OK") -> ()  [unwired: 1 out]
          }
        }
        n825 = call <vilib>:"Add State(s) to Queue__JKI_lib_State_Machine.vi"("State(s) in (\"\")"=w1754) -> ("States Out"=w1753:string)  [unwired: 14 in]
      }
      frame "LabJack: FootPedalConfig" {
        # "Setup footPedal\n(You can make a copy of, or modify, this frame)"
        n826 = call "LabJack_FGV.vi"("Operation(Read)"=enum16{"Write", "Read"}."Read" ("Operation"), "error in (no error)"=w1758) -> ("error out"=w1762:errorcluster, "Read data"=w1763:i32)  [unwired: 8 in]
        n827 = call "LJM_eWriteName.vi"("Handle In"=w1763, "Name"="DIO15", "Value"=1.0, "error in"=w1762) -> ("error out"=w1759:errorcluster)  [unwired: 10 in, 1 out]
        n828 = call <vilib>:"Add State(s) to Queue__JKI_lib_State_Machine.vi"("State(s) in (\"\")"=w1767) -> ("States Out"=w1766:string)  [unwired: 14 in]
      }
      frame "LabJack: SetDefaultAndClose" {
        # "Template Separator\n(You can make a copy of, or modify, this frame)"
        n829 = call <vilib>:"Add State(s) to Queue__JKI_lib_State_Machine.vi"("State(s) in Front (\"\")"="LabJack: SetDefaultSub\nLabJack: Close" ("State(s) in Front (\"\")"), "State(s) in (\"\")"=w1773) -> ("States Out"=w1772:string)  [unwired: 13 in]
      }
      frame "LabJack: Close" {
        # "Close LabJack Refnum"
        n830 = call "LabJack_FGV.vi"("Operation(Read)"=enum16{"Write", "Read"}."Read" ("Operation"), "error in (no error)"=w1779) -> ("error out"=w1774:errorcluster, "Read data"=w1775:i32)  [unwired: 8 in]
        n831 = Bundle By Name(cluster=w1777, "System Status.Labjack"=FALSE ("System Status.Gain Control")) -> (w1780:T23)
        n832 = call "LJM_Close.vi"("error in"=w1774, "Handle"=w1775) -> ("error out"=w1782:errorcluster)  [unwired: 9 in]
        n833 = call <vilib>:"Add State(s) to Queue__JKI_lib_State_Machine.vi"("State(s) in (\"\")"=w1784) -> ("States Out"=w1783:string)  [unwired: 14 in]
      }
      frame "LabJack: Interlock enable/disable" {
        w1793 = i8 0  # int8
        # "[Covers: REQ8]"
        # "Interlock enable/disable\n(Usage: \"LabJack: Interlock enable/disable >> 1|0\")"
        n834 = Fract/Exp String To Number(string=w1794, default (0 dbl)=w1793) -> (number=w1790:i8)  [unwired: 2 in, 1 out]
        n835 = Unbundle By Name(w1792) -> ("LJ Pinout.Interlock"=w1791:string)
        n836 = call "LabJack_FGV.vi"("Operation(Read)"=enum16{"Write", "Read"}."Read" ("Operation")) -> ("Read data"=w1788:i32)  [unwired: 9 in, 1 out]
        n837 = call "LJM_eWriteName.vi"("Handle In"=w1788, "Name"=w1791, "Value"=w1790, "error in"=w1789) -> ("error out"=w1786:errorcluster)  [unwired: 10 in, 1 out]
        n838 = call <vilib>:"Add State(s) to Queue__JKI_lib_State_Machine.vi"("State(s) in (\"\")"=w1796) -> ("States Out"=w1795:string)  [unwired: 14 in]
      }
      frame "LabJack: 355_PWM_Config" {
        w1798 = 0.0 ("element")
        w1818 = "DIO_EF_CLOCK1_ENABLE"
        # "Config PWM frequency"
        n839 = Unbundle By Name(w1810) -> ("LJ Pinout.355 PWM"=w1817:string)
        n840 = Unbundle By Name(w1810) -> ("355 PWM setting.DIO_EF_CLOCK1_DIVISOR"=w1809:i16, "355 PWM setting.DIO_EF_CLOCK1_ROLL_VALUE"=w1808:i32, "355 PWM setting.DIO#_EF_INDEX"=w1805:i16, "355 PWM setting.DIO#_EF_OPTIONS"=w1804:i16, "355 PWM setting.DIO#_EF_CONFIG_A"=w1803:i32)
        n841 = Concatenate Strings(w1817, "_EF_ENABLE" ("string")) -> (w1813:string)
        n842 = Concatenate Strings(w1817, "_EF_INDEX") -> (w1816:string)
        n843 = Concatenate Strings(w1817, "_EF_OPTIONS") -> (w1815:string)
        n844 = Concatenate Strings(w1817, "_EF_CONFIG_A") -> (w1814:string)
        n845 = call "LabJack_FGV.vi"("Operation(Read)"=enum16{"Write", "Read"}."Read" ("Operation")) -> ("Read data"=w1811:i32)  [unwired: 9 in, 1 out]
        n846 = Build Array(w1798, w1798, w1809, w1808, 1.0 ("element"), 0.0 ("element"), w1805, w1804, w1803) -> (w1802:dbl[])
        n847 = Build Array("DIO_EF_CLOCK0_ENABLE", w1818, "DIO_EF_CLOCK1_DIVISOR", "DIO_EF_CLOCK1_ROLL_VALUE", w1818, w1813, w1816, w1815, w1814) -> (w1812:string[])
        n848 = call "LJM_eWriteNames.vi"("Handle In"=w1811, "aNames"=w1812, "aValuesIn"=w1802, "error in"=w1800) -> ("error out"=w1801:errorcluster)  [unwired: 9 in, 2 out]
        n849 = call <vilib>:"Add State(s) to Queue__JKI_lib_State_Machine.vi"("State(s) in (\"\")"=w1827) -> ("States Out"=w1826:string)  [unwired: 14 in]
      }
      frame "LabJack: 355_PWM_Start" {
        # "Template Separator\n(You can make a copy of, or modify, this frame)"
        n850 = Unbundle By Name(w1835) -> ("LJ Pinout.355 PWM"=w1834:string)
        n851 = call "LabJack_FGV.vi"("Operation(Read)"=enum16{"Write", "Read"}."Read" ("Operation"), "error in (no error)"=w1829) -> ("error out"=w1836:errorcluster, "Read data"=w1837:i32)  [unwired: 8 in]
        n852 = Concatenate Strings(w1834, "_EF_ENABLE" ("string")) -> (w1832:string)
        n853 = call "LJM_eWriteName.vi"("Handle In"=w1837, "Name"=w1832, "Value"=1.0, "error in"=w1836) -> ("error out"=w1830:errorcluster)  [unwired: 10 in, 1 out]
        n854 = call <vilib>:"Add State(s) to Queue__JKI_lib_State_Machine.vi"("State(s) in (\"\")"=w1840) -> ("States Out"=w1839:string)  [unwired: 14 in]
      }
      frame "LabJack: 355_PWM_Stop" {
        # "Template Separator\n(You can make a copy of, or modify, this frame)"
        n855 = Unbundle By Name(w1846) -> ("LJ Pinout.355 PWM"=w1850:string)
        n856 = call "LabJack_FGV.vi"("Operation(Read)"=enum16{"Write", "Read"}."Read" ("Operation"), "error in (no error)"=w1845) -> ("error out"=w1851:errorcluster, "Read data"=w1843:i32)  [unwired: 8 in]
        n857 = Concatenate Strings(w1850, "_EF_ENABLE" ("string")) -> (w1848:string)
        n858 = call "LJM_eWriteName.vi"("Handle In"=w1843, "Name"=w1848, "Value"=0.0, "error in"=w1851) -> ("error out"=w1842:errorcluster)  [unwired: 10 in, 1 out]
        n859 = local write "355nm Laser toggle"(FALSE ("355nm Laser toggle")) -> ()
        n860 = call <vilib>:"Add State(s) to Queue__JKI_lib_State_Machine.vi"("State(s) in (\"\")"=w1854) -> ("States Out"=w1853:string)  [unwired: 14 in]
      }
      frame "LabJack: AB_Start" {
        # "Aiming Beam Start\n(Based on aimging beam frequency, set LabJack pin)"
        n861 = Unbundle By Name(w1864) -> ("AB Cluster.Freq"=w1856:i32, "LJ Pinout.AimingBeam PWM"=w1863:string)
        n862 = Greater Than 0?(x=w1856) -> (x > 0?=w1855:bool)
        n863 = case shown="False" w1855 {
          tunnel: w1863 -> [w1870 w1873]
          tunnel: [w1870 w1871] -> w1862
          frame False {
            # "if 0 freq, set PWM pin"
          }
          frame True {
            # "if non zero freq, set PWM enable"
            n864 = Concatenate Strings(w1873, "_EF_ENABLE" ("string")) -> (w1871:string)
          }
        }
        n865 = call "LabJack_FGV.vi"("Operation(Read)"=enum16{"Write", "Read"}."Read" ("Operation"), "error in (no error)"=w1859) -> ("error out"=w1865:errorcluster, "Read data"=w1866:i32)  [unwired: 8 in]
        n866 = call "LJM_eWriteName.vi"("Handle In"=w1866, "Name"=w1862, "Value"=1.0, "error in"=w1865) -> ("error out"=w1860:errorcluster)  [unwired: 10 in, 1 out]
        n867 = local write "Aiming beam toggle"(TRUE ("Aiming beam toggle")) -> ()
        n868 = call <vilib>:"Add State(s) to Queue__JKI_lib_State_Machine.vi"("State(s) in (\"\")"=w1869) -> ("States Out"=w1868:string)  [unwired: 14 in]
      }
      frame "LabJack: AB_Stop" {
        # "Aiming Beam Stop\n(Based on aiming beam frequency, set LabJack pin low)"
        n869 = Unbundle By Name(w1881) -> ("AB Cluster.Freq"=w1876:i32, "LJ Pinout.AimingBeam PWM"=w1883:string)
        n870 = Greater Than 0?(x=w1876) -> (x > 0?=w1875:bool)
        n871 = case shown="False" w1875 {
          tunnel: w1883 -> [w1889 w1892]
          tunnel: [w1889 w1890] -> w1874
          frame False {
          }
          frame True {
            n872 = Concatenate Strings(w1892, "_EF_ENABLE" ("string")) -> (w1890:string)
          }
        }
        n873 = call "LabJack_FGV.vi"("Operation(Read)"=enum16{"Write", "Read"}."Read" ("Operation"), "error in (no error)"=w1879) -> ("error out"=w1884:errorcluster, "Read data"=w1885:i32)  [unwired: 8 in]
        n874 = call "LJM_eWriteName.vi"("Handle In"=w1885, "Name"=w1874, "Value"=0.0, "error in"=w1884) -> ("error out"=w1880:errorcluster)  [unwired: 10 in, 1 out]
        n875 = local write "Aiming beam toggle"(FALSE ("Aiming beam toggle")) -> ()
        n876 = call <vilib>:"Add State(s) to Queue__JKI_lib_State_Machine.vi"("State(s) in (\"\")"=w1888) -> ("States Out"=w1887:string)  [unwired: 14 in]
      }
      frame "LabJack: AB_PWM_Config" {
        w1894 = 0.0 ("element")
        w1914 = "DIO_EF_CLOCK2_ENABLE"
        # "Config PWM frequency"
        n877 = Unbundle By Name(w1906) -> ("LJ Pinout.AimingBeam PWM"=w1913:string)
        n878 = Unbundle By Name(w1906) -> ("AB PWM setting.DIO_EF_CLOCK1_DIVISOR"=w1905:i16, "AB PWM setting.DIO_EF_CLOCK1_ROLL_VALUE"=w1904:i32, "AB PWM setting.DIO#_EF_INDEX"=w1901:i16, "AB PWM setting.DIO#_EF_OPTIONS"=w1900:i16, "AB PWM setting.DIO#_EF_CONFIG_A"=w1899:i32)
        n879 = Concatenate Strings(w1913, "_EF_ENABLE" ("string")) -> (w1909:string)
        n880 = Concatenate Strings(w1913, "_EF_INDEX") -> (w1912:string)
        n881 = Concatenate Strings(w1913, "_EF_OPTIONS") -> (w1911:string)
        n882 = Concatenate Strings(w1913, "_EF_CONFIG_A") -> (w1910:string)
        n883 = call "LabJack_FGV.vi"("Operation(Read)"=enum16{"Write", "Read"}."Read" ("Operation")) -> ("Read data"=w1907:i32)  [unwired: 9 in, 1 out]
        n884 = Build Array(w1894, w1894, w1905, w1904, 1.0 ("element"), 0.0 ("element"), w1901, w1900, w1899) -> (w1898:dbl[])
        n885 = Build Array("DIO_EF_CLOCK0_ENABLE", w1914, "DIO_EF_CLOCK2_DIVISOR", "DIO_EF_CLOCK2_ROLL_VALUE", w1914, w1909, w1912, w1911, w1910) -> (w1908:string[])
        n886 = call "LJM_eWriteNames.vi"("Handle In"=w1907, "aNames"=w1908, "aValuesIn"=w1898, "error in"=w1896) -> ("error out"=w1897:errorcluster)  [unwired: 9 in, 2 out]
        n887 = call <vilib>:"Add State(s) to Queue__JKI_lib_State_Machine.vi"("State(s) in (\"\")"=w1923) -> ("States Out"=w1922:string)  [unwired: 14 in]
      }
      frame "---------- LED ----------" {
        # "Template Separator\n(You can make a copy of, or modify, this frame)"
        n888 = call <vilib>:"Add State(s) to Queue__JKI_lib_State_Machine.vi"("State(s) in (\"\")"=w1928) -> ("States Out"=w1927:string)  [unwired: 14 in]
      }
      frame "LED: OpenVIRef" {
        # "Template Separator\n(You can make a copy of, or modify, this frame)"
        n889 = call <vilib>:"Application Directory.vi"() -> ("Application Directory"=w1935:path)
        n890 = Build Path(base path=w1935, name or relative path="SubVI") -> (appended path=w1933:path)
        n891 = Build Path(base path=w1933, name or relative path="LEDBreath.vi") -> (appended path=w1931:path)
        n892 = Open VI Reference(vi path=w1931, error in (no error)=w1936) -> (vi reference=w1937:refnum<vi>, error out=w1930:errorcluster)  [unwired: 4 in]
        n893 = case shown="Error .." w1930 {
          tunnel: [TRUE FALSE] -> w1929
          frame No Error {
          }
          frame Error {
          }
        }
        n894 = Bundle By Name(cluster=w1938, "LED vi reference"=w1937, "LED vi ref open?"=w1929) -> (w1939:T23)
        n895 = call <vilib>:"Add State(s) to Queue__JKI_lib_State_Machine.vi"("State(s) in (\"\")"=w1942) -> ("States Out"=w1941:string)  [unwired: 14 in]
      }
      frame "LED: CloseVIRef" {
        # "Template Separator\n(You can make a copy of, or modify, this frame)"
        n896 = Unbundle By Name(w1946) -> ("LED vi reference"=w1947:refnum<vi>, "LED vi ref open?"=w1945:bool)
        n897 = case shown="True" w1945 {
          tunnel: w1949 -> [w1953 w1956]
          tunnel: [w1953 w1955] -> w1948
          tunnel: w1947 -> [_ w1954]
          frame False {
          }
          frame True {
            n898 = Close Reference(reference=w1954, error in (no error)=w1956) -> (error out=w1955:errorcluster)
          }
        }
        n899 = call <vilib>:"Add State(s) to Queue__JKI_lib_State_Machine.vi"("State(s) in (\"\")"=w1952) -> ("States Out"=w1951:string)  [unwired: 14 in]
      }
      frame "LED: BreathGreen" {
        w1957 = FALSE ("Wait Until Done")
        # "Breath system LED\n(LED: Breath >> True/False)"
        n900 = Unbundle By Name(w1965) -> ("LED vi reference"=w1964:refnum<vi>)
        n901 = invoke class="VI" method="Ctrl Val.Set"(reference=w1964, error in=w1962, "Control Name"="Color", "Value"=0) -> (reference out=w1961:refnum<vi>, error out=w1960:errorcluster)  [unwired: 1 in, 3 out]
        n902 = invoke on="Invoke Node" class="VI" method="Run VI"(reference=w1961, error in=w1960, "Wait until done"=w1957, "Auto Dispose Ref"=w1957) -> (error out=w1963:errorcluster)  [unwired: 1 in, 4 out]
        n903 = call <vilib>:"Add State(s) to Queue__JKI_lib_State_Machine.vi"("State(s) in (\"\")"=w1968) -> ("States Out"=w1967:string)  [unwired: 14 in]
      }
      frame "LED: BreathOrange" {
        w1969 = FALSE ("Wait Until Done")
        # "Breath system LED\n(LED: Breath >> True/False)"
        n904 = Unbundle By Name(w1977) -> ("LED vi reference"=w1976:refnum<vi>)
        n905 = invoke class="VI" method="Ctrl Val.Set"(reference=w1976, error in=w1974, "Control Name"="Color", "Value"=1) -> (reference out=w1973:refnum<vi>, error out=w1972:errorcluster)  [unwired: 1 in, 3 out]
        n906 = invoke on="Invoke Node" class="VI" method="Run VI"(reference=w1973, error in=w1972, "Wait until done"=w1969, "Auto Dispose Ref"=w1969) -> (error out=w1975:errorcluster)  [unwired: 1 in, 4 out]
        n907 = call <vilib>:"Add State(s) to Queue__JKI_lib_State_Machine.vi"("State(s) in (\"\")"=w1980) -> ("States Out"=w1979:string)  [unwired: 14 in]
      }
      frame "LED: BreathOff" {
        # "System LED Breath Off\n(Breath off, check VI status to make sure it is off)"
        n908 = Unbundle By Name(w1989) -> ("LED vi reference"=w1988:refnum<vi>)
        n909 = invoke on="Invoke Node" class="VI" method="Ctrl Val.Set"(reference=w1988, error in=w1986, "Control Name"="Stop", "Value"=TRUE) -> (reference out=w1981:refnum<vi>, error out=w1982:errorcluster)  [unwired: 1 in, 3 out]
        n910 = case shown="No Error" w1982 {
          selector: w1982 -> [w1994 _]
          tunnel: [w1993 errorcluster {"status"=FALSE, "code"=0, "source"=""} ("error IO")] -> w1987
          tunnel: ["" ("State(s) in Front (\"\")") "LED: BreathOff" ("State(s) in Front (\"\")")] -> w1985
          tunnel: w1981 -> [w1995 _]
          frame No Error {
            # "No error, wait for VI to stop"
            n911 = while {
              tunnel: w1995 -> [w2003]
              shift-right: [w1997] -> w1993
              shift-left: w1994 -> [w2002]
              stop <- w1999 stop-if-true
              # "continue check whether vi is running"
              n912 = property class="VI"(reference=w2003, error in=w2002) -> (error out=w1997:errorcluster, "Exec.State"=w2001:T20)  [unwired: 1 out]
              n913 = Wait (ms)(milliseconds to wait=u32 50) -> ()  [unwired: 1 out]
              n914 = Equal?(x=w2001, y=T20."Idle") -> (x = y?=w1999:bool)
            }
          }
          frame Error {
            # "try again when error"
          }
        }
        n915 = call <vilib>:"Add State(s) to Queue__JKI_lib_State_Machine.vi"("State(s) in Front (\"\")"=w1985, "State(s) in (\"\")"=w1992) -> ("States Out"=w1991:string)  [unwired: 13 in]
      }
      frame "LED: Off" {
        # "set LED to red"
        # "Template Separator\n(You can make a copy of, or modify, this frame)"
        n916 = Unbundle By Name(w2008) -> ("LJ Pinout.Red LED"=w2007:string, "LJ Pinout.Green LED"=w2006:string)
        n917 = call "LabJack_FGV.vi"("Operation(Read)"=enum16{"Write", "Read"}."Read" ("Operation"), "error in (no error)"=w2009) -> ("error out"=w2016:errorcluster, "Read data"=w2015:i32)  [unwired: 8 in]
        n918 = call "LJM_eWriteName.vi"("Handle In"=w2015, "Name"=w2007, "Value"=0.0, "error in"=w2016) -> ("Handle Out"=w2013:i32, "error out"=w2012:errorcluster)  [unwired: 10 in]
        n919 = call "LJM_eWriteName.vi"("Handle In"=w2013, "Name"=w2006, "Value"=0.0, "error in"=w2012) -> ("error out"=w2010:errorcluster)  [unwired: 10 in, 1 out]
        n920 = call <vilib>:"Add State(s) to Queue__JKI_lib_State_Machine.vi"("State(s) in (\"\")"=w2020) -> ("States Out"=w2019:string)  [unwired: 14 in]
      }
      frame "LED: Green" {
        # "set LED to green"
        # "Template Separator\n(You can make a copy of, or modify, this frame)"
        n921 = Unbundle By Name(w2024) -> ("LJ Pinout.Red LED"=w2022:string, "LJ Pinout.Green LED"=w2023:string)
        n922 = call "LabJack_FGV.vi"("Operation(Read)"=enum16{"Write", "Read"}."Read" ("Operation"), "error in (no error)"=w2026) -> ("error out"=w2032:errorcluster, "Read data"=w2031:i32)  [unwired: 8 in]
        n923 = call "LJM_eWriteName.vi"("Handle In"=w2031, "Name"=w2022, "Value"=0.0, "error in"=w2032) -> ("Handle Out"=w2029:i32, "error out"=w2028:errorcluster)  [unwired: 10 in]
        n924 = call "LJM_eWriteName.vi"("Handle In"=w2029, "Name"=w2023, "Value"=9.0, "error in"=w2028) -> ("error out"=w2025:errorcluster)  [unwired: 10 in, 1 out]
        n925 = call <vilib>:"Add State(s) to Queue__JKI_lib_State_Machine.vi"("State(s) in (\"\")"=w2035) -> ("States Out"=w2034:string)  [unwired: 14 in]
      }
      frame "---------- Queue ----------" {
        # "Template Separator\n(You can make a copy of, or modify, this frame)"
        n926 = call <vilib>:"Add State(s) to Queue__JKI_lib_State_Machine.vi"("State(s) in (\"\")"=w2040) -> ("States Out"=w2039:string)  [unwired: 14 in]
      }
      frame "Queue: Flash" {
        # "Clear queue contnet\n(clear queue content by flash it)"
        n927 = Flush Queue(queue=w2047, error in (no error)=w2041) -> (error out=w2045:errorcluster)  [unwired: 2 out]
        n928 = Flush Queue(queue=w2048, error in (no error)=w2041) -> (error out=w2044:errorcluster)  [unwired: 2 out]
        n929 = Flush Queue(queue=w2046, error in (no error)=w2041) -> (error out=w2043:errorcluster)  [unwired: 2 out]
        n930 = Merge Errors(w2045, w2044, w2043) -> (w2042:errorcluster)
        n931 = call <vilib>:"Add State(s) to Queue__JKI_lib_State_Machine.vi"("State(s) in (\"\")"=w2052) -> ("States Out"=w2051:string)  [unwired: 14 in]
      }
      frame "Queue: Destory" {
        # "Destory Data Queue\nDistory data queue ref so the aquisition loop stop"
        n932 = Release Queue(queue=w2058, error in (no error)=w2054) -> (error out=w2061:errorcluster)  [unwired: 1 in, 2 out]
        n933 = Release Queue(queue=w2057, error in (no error)=w2054) -> (error out=w2060:errorcluster)  [unwired: 1 in, 2 out]
        n934 = Release Queue(queue=w2055, error in (no error)=w2054) -> (error out=w2053:errorcluster)  [unwired: 1 in, 2 out]
        n935 = Merge Errors(w2061, w2060, w2053) -> (w2059:errorcluster)
        n936 = call <vilib>:"Simple Error Handler.vi"("error in (no error)"=w2059) -> ()  [unwired: 4 in, 5 out]
        n937 = call <vilib>:"Add State(s) to Queue__JKI_lib_State_Machine.vi"("State(s) in (\"\")"=w2064) -> ("States Out"=w2063:string)  [unwired: 14 in]
      }
      frame "---------- Run ----------" {
        # "Template Separator\n(You can make a copy of, or modify, this frame)"
        n938 = call <vilib>:"Add State(s) to Queue__JKI_lib_State_Machine.vi"("State(s) in (\"\")"=w2069) -> ("States Out"=w2068:string)  [unwired: 14 in]
      }
      frame "Run: CaliIncrement" {
        # "Increment Calibration #\n(You can make a copy of, or modify, this frame)"
        n939 = Unbundle By Name(w2071) -> ("IDs.Cali ID"=w2073:i8)
        n940 = Increment(x=w2073) -> (x+1=w2070:i8)
        n941 = Bundle By Name(cluster=w2071, "IDs.Cali ID"=w2070) -> (w2072:T23)
        n942 = call <vilib>:"Add State(s) to Queue__JKI_lib_State_Machine.vi"("State(s) in (\"\")"=w2077) -> ("States Out"=w2076:string)  [unwired: 14 in]
      }
      frame "Run: BGIncrement" {
        # "Increment BG #\n(You can make a copy of, or modify, this frame)"
        n943 = Unbundle By Name(w2078) -> ("IDs.BG ID"=w2081:i8)
        n944 = Increment(x=w2081) -> (x+1=w2080:i8)
        n945 = Bundle By Name(cluster=w2078, "IDs.BG ID"=w2080) -> (w2079:T23)
        n946 = call <vilib>:"Add State(s) to Queue__JKI_lib_State_Machine.vi"("State(s) in (\"\")"=w2085) -> ("States Out"=w2084:string)  [unwired: 14 in]
      }
      frame "Run: Increment" {
        # "Increase Run# by 1"
        n947 = Unbundle By Name(w2090) -> ("IDs.RunID"=w2092:i8)
        n948 = Increment(x=w2092) -> (x+1=w2088:i8)
        n949 = Bundle By Name(cluster=w2090, "IDs.RunID"=w2088) -> (w2091:T23)
        n950 = call "RunIDFGV.vi"("Error In"=w2086, "RunID in"=w2088) -> ("Error Out"=w2087:errorcluster)  [unwired: 8 in, 1 out]
        n951 = call <vilib>:"Add State(s) to Queue__JKI_lib_State_Machine.vi"("State(s) in (\"\")"=w2094) -> ("States Out"=w2093:string)  [unwired: 14 in]
      }
      frame "Run: Decrement" {
        # "Increase Run# by 1"
        n952 = Unbundle By Name(w2099) -> ("IDs.RunID"=w2101:i8)
        n953 = Decrement(x=w2101) -> (x-1=w2097:i8)
        n954 = Bundle By Name(cluster=w2099, "IDs.RunID"=w2097) -> (w2100:T23)
        n955 = call "RunIDFGV.vi"("Error In"=w2095, "RunID in"=w2097) -> ("Error Out"=w2096:errorcluster)  [unwired: 8 in, 1 out]
        n956 = call <vilib>:"Add State(s) to Queue__JKI_lib_State_Machine.vi"("State(s) in (\"\")"=w2103) -> ("States Out"=w2102:string)  [unwired: 14 in]
      }
      frame "---------- SysConfig ----------" {
        # "Template Separator\n(You can make a copy of, or modify, this frame)"
        n957 = call <vilib>:"Add State(s) to Queue__JKI_lib_State_Machine.vi"("State(s) in (\"\")"=w2108) -> ("States Out"=w2107:string)  [unwired: 14 in]
      }
      frame "SysConfig: LoadAPDSerialNumber" {
        # "Template Separator\n(You can make a copy of, or modify, this frame)"
        n958 = call "readAPDSerial.vi"("Error In"=w2110) -> ("Error Out"=w2109:errorcluster, "output cluster"=w2111:T26)  [unwired: 9 in]
        n959 = Bundle By Name(cluster=w2112, "APDSerialNum"=w2111) -> (w2113:T23)
        n960 = call <vilib>:"Add State(s) to Queue__JKI_lib_State_Machine.vi"("State(s) in (\"\")"=w2116) -> ("States Out"=w2115:string)  [unwired: 14 in]
      }
      frame "SysConfig: Load Sys Config" {
        # "[Covers: REQ5]"
        # "Load System config"
        # "Load system configuration\n(Load both hardware and DAQ config)"
        n961 = call "LoadSysConfig.vi"("Error In"=w2119, "Enum"=enum16{"LastUse", "Default"}."LastUse") -> ("Error Out"=w2118:errorcluster, "SysConfigCluster"=w2121:T7)  [unwired: 8 in]
        "SysConfigCluster" <- w2121
        n962 = Bundle By Name(cluster=w2122, "SysConfigCluster"=w2121) -> (w2123:T23)
        n963 = call <vilib>:"Add State(s) to Queue__JKI_lib_State_Machine.vi"("State(s) in (\"\")"=w2125) -> ("States Out"=w2124:string)  [unwired: 14 in]
      }
      frame "SysConfig: Load Digitizer Setting" {
        w2126 = enum16{"Write", "Read"}."Write" ("Operation")
        # "Load DAQ config\nSave to FGV"
        # "Template Separator\n(You can make a copy of, or modify, this frame)"
        n964 = call <userlib>:"Current VIs Parent Directory__ogtk.vi"() -> ("Parent Directory (+ Relative)"=w2140:path)  [unwired: 5 in]
        n965 = Build Path(base path=w2140, name or relative path="SubVI\\DigitizerConfiguration\\V6_Scope_last_use.config") -> (appended path=w2141:path)
        n966 = call "ReadDigitizerConfig(SubVI).vi"("error in (no error)"=w2138, "appended path"=w2141) -> ("error out"=w2134:errorcluster, "FLImDAQ"=w2132:T5)  [unwired: 8 in]
        n967 = call "FLImDAQ_FGV.vi"("error in (no error)"=w2134, "Operation (Read)"=w2126, "Write data"=w2132) -> ("error out"=w2136:errorcluster)  [unwired: 7 in, 1 out]
        n968 = Unbundle By Name(w2132) -> ("min record length"=→"data length":i32, "Digitizer 1"=w2128:refnum<k15>, "Digitizer 2"=w2135:refnum<k15>)
        n969 = Bundle By Name(cluster=w2130, "FLImDAQ"=w2132) -> (w2131:T23)
        n970 = call "Digitizer1_FGV.vi"("error in (no error)"=w2136, "Operation (Read)"=w2126, "Write data"=w2128) -> ("error out"=w2137:errorcluster)  [unwired: 7 in, 1 out]
        n971 = call "Digitizer2_FGV.vi"("error in (no error)"=w2137, "Operation (Read)"=w2126, "Write data"=w2135) -> ("error out"=w2133:errorcluster)  [unwired: 7 in, 1 out]
        n972 = call <vilib>:"Add State(s) to Queue__JKI_lib_State_Machine.vi"("State(s) in (\"\")"=w2143) -> ("States Out"=w2142:string)  [unwired: 14 in]
      }
      frame "SysConfig: Load LJ Pinout" {
        # "Template Separator\n(You can make a copy of, or modify, this frame)"
        n973 = call <userlib>:"Current VIs Parent Directory__ogtk.vi"() -> ("Parent Directory (+ Relative)"=w2158:path)  [unwired: 5 in]
        n974 = Build Path(base path=w2158, name or relative path="SubVI\\LabJack\\LJ_pin_setting.config") -> (appended path=w2156:path)
        n975 = call "ReadLabjackConfig(SubVI).vi"("error in (no error)"=w2154, "appended path"=w2156) -> ("error out"=w2155:errorcluster, "Utility"=w2152:T4)  [unwired: 8 in]
        n976 = Unbundle By Name(w2152) -> ("Ch1 Bias"=w2151:string, "Ch2 Bias"=w2150:string, "Ch3 Bias"=w2149:string, "Ch4 Bias"=w2144:string, "Red LED"=w2146:string, "Green LED"=w2145:string)
        n977 = global write "GlobalVariables.vi" "LED Green pin"(w2145) -> ()
        n978 = global write "GlobalVariables.vi" "Ch1 LJ pin"(w2151) -> ()
        n979 = global write "GlobalVariables.vi" "Ch2 LJ pin"(w2150) -> ()
        n980 = global write "GlobalVariables.vi" "Ch3 LJ pin"(w2149) -> ()
        n981 = global write "GlobalVariables.vi" "Ch4 LJ pin"(w2144) -> ()
        n982 = global write "GlobalVariables.vi" "LED Red pin"(w2146) -> ()
        n983 = Bundle By Name(cluster=w2147, "LJ Pinout"=w2152) -> (w2153:T23)
        n984 = call <vilib>:"Add State(s) to Queue__JKI_lib_State_Machine.vi"("State(s) in (\"\")"=w2160) -> ("States Out"=w2159:string)  [unwired: 14 in]
      }
      frame "SysConfig: Load 355 PWM" {
        # "Template Separator\n(You can make a copy of, or modify, this frame)"
        n985 = call <userlib>:"Current VIs Parent Directory__ogtk.vi"() -> ("Parent Directory (+ Relative)"=w2178:path)  [unwired: 5 in]
        n986 = Build Path(base path=w2178, name or relative path="SubVI\\LabJack\\PWM_setting_355.config") -> (appended path=w2176:path)
        n987 = call "ReadPWMConfig(SubVI).vi"("error in (no error)"=w2173, "appended path"=w2176) -> ("error out"=w2174:errorcluster, "PWM Setting"=w2172:T41)  [unwired: 8 in]
        n988 = Unbundle By Name(w2172) -> ("DIO_EF_CLOCK1_DIVISOR"=w2169:i16, "DIO_EF_CLOCK1_ROLL_VALUE"=w2168:i32)
        n989 = Multiply(x=w2169, y=w2168) -> (x*y=w2170:i32)
        n990 = Bundle By Name(cluster=w2175, "355 PWM setting"=w2172) -> (w2162:T23)
        n991 = Divide(x=80000000.0, y=w2170) -> (x/y=w2167:dbl)
        "Laser Rep Rate" <- w2167
        n992 = Number To Decimal String(number=w2167) -> (decimal integer string=w2166:string)  [unwired: 1 in]
        n993 = Concatenate Strings("355nm " ("string"), w2166, "Hz" ("string")) -> (w2164:string)
        n994 = property on="355nm Laser toggle" class="Bool (strict)"("Caption.Text"=w2164) -> ()  [unwired: 2 in, 2 out]
        n995 = call <vilib>:"Add State(s) to Queue__JKI_lib_State_Machine.vi"("State(s) in (\"\")"=w2180) -> ("States Out"=w2179:string)  [unwired: 14 in]
      }
      frame "SysConfig: Load AB PWM" {
        # "Template Separator\n(You can make a copy of, or modify, this frame)"
        n996 = call <userlib>:"Current VIs Parent Directory__ogtk.vi"() -> ("Parent Directory (+ Relative)"=w2189:path)  [unwired: 5 in]
        n997 = Build Path(base path=w2189, name or relative path="SubVI\\LabJack\\PWM_setting_AB.config") -> (appended path=w2187:path)
        n998 = call "ReadPWMConfig(SubVI).vi"("error in (no error)"=w2184, "appended path"=w2187) -> ("error out"=w2185:errorcluster, "PWM Setting"=w2183:T41)  [unwired: 8 in]
        n999 = Bundle By Name(cluster=w2181, "AB PWM setting"=w2183) -> (w2186:T23)
        n1000 = call <vilib>:"Add State(s) to Queue__JKI_lib_State_Machine.vi"("State(s) in (\"\")"=w2191) -> ("States Out"=w2190:string)  [unwired: 14 in]
      }
      frame "SysConfig: Load AB setting" {
        # "load aming beam setting\n(check frequency, if 0 do nothing, if not zero, config PWM)"
        n1001 = call "readAimingBeamSetting.vi"("error in (no error)"=w2205) -> ("error out"=w2200:errorcluster, "Aiming Beam Setting"=w2193:T42)  [unwired: 9 in]
        n1002 = Unbundle By Name(w2193) -> ("Frequency(Hz)"=w2192:u32)
        n1003 = Equal To 0?(x=w2192) -> (x = 0?=w2198:bool)
        n1004 = Select(t="", s=w2198, f="SysConfig: Load AB PWM" ("State(s) in Front (\"\")")) -> (s? t:f=w2201:string)
        n1005 = Number To Decimal String(number=w2192) -> (decimal integer string=w2197:string)  [unwired: 1 in]
        n1006 = Concatenate Strings("488nm " ("string"), w2197, "Hz " ("string")) -> (w2196:string)
        n1007 = property on="Aiming beam toggle" class="Bool (strict)"("Caption.Text"=w2196) -> ()  [unwired: 2 in, 2 out]
        n1008 = case shown="False" w2198 {
          tunnel: w2200 -> [w2213 w2216]
          tunnel: [w2212 w2216] -> w2199
          tunnel: w2192 -> [w2211 _]
          frame False {
            n1009 = call "LJ_calculate_PWM_parameters.vi"("Duty Cycle (%)"=u32 10, "Error In"=w2213, "Show Confirmation"=FALSE, "Laser Rep Rate (Hz)"=w2211, "Laser"=enum16{"355nm", "AimingBeam"}."AimingBeam") -> ("Error Out"=w2212:errorcluster)  [unwired: 5 in, 1 out]
          }
          frame True {
          }
        }
        n1010 = Bundle By Name(cluster=w2206, "AB Cluster"=w2193) -> (w2207:T23)
        n1011 = call <vilib>:"Add State(s) to Queue__JKI_lib_State_Machine.vi"("State(s) in Front (\"\")"=w2201, "State(s) in (\"\")"=w2209) -> ("States Out"=w2208:string)  [unwired: 13 in]
      }
      frame "SysConfig: LoadABVideoSetting" {
        # "Load AB video setting form ini file\n()"
        n1012 = call "readVideoConfig.vi"("error in (no error)"=w2220) -> ("error out"=w2221:errorcluster, "Aiming Beam Config"=w2219:T22)  [unwired: 8 in, 1 out]
        n1013 = Bundle By Name(cluster=w2217, "VideoConfig"=w2219) -> (w2218:T23)
        n1014 = call <vilib>:"Add State(s) to Queue__JKI_lib_State_Machine.vi"("State(s) in (\"\")"=w2224) -> ("States Out"=w2223:string)  [unwired: 14 in]
      }
      frame "SysConfig: LoadCursorLocation" {
        # "Load cursor location from ini file\n(load cursor from system setting ini file)"
        n1015 = call "readCursorConfigMain.vi"("error in (no error)"=w2236) -> ("error out"=w2237:errorcluster, "Cursor Locations"=w2235:T43)  [unwired: 9 in]
        n1016 = Unbundle By Name(w2235) -> ("DC1"=w2234:i32, "DC2"=w2233:i32, "BG1"=w2228:i32, "BG2"=w2227:i32)
        n1017 = Build Array(w2234, w2233) -> (w2232:i32[])
        n1018 = Build Array(w2228, w2227) -> (w2229:i32[])
        n1019 = Array Max & Min(array=w2232) -> (max value=w2231:i32, min value=w2230:i32)  [unwired: 2 out]
        n1020 = Array Max & Min(array=w2229) -> (max value=w2226:i32, min value=w2225:i32)  [unwired: 2 out]
        n1021 = global write "GlobalVariables.vi" "DC Idx2"(w2231) -> ()
        n1022 = global write "GlobalVariables.vi" "DC Idx1"(w2230) -> ()
        n1023 = global write "GlobalVariables.vi" "BG Idx2"(w2226) -> ()
        n1024 = global write "GlobalVariables.vi" "BG Idx1"(w2225) -> ()
        n1025 = call <vilib>:"Add State(s) to Queue__JKI_lib_State_Machine.vi"("State(s) in (\"\")"=w2241) -> ("States Out"=w2240:string)  [unwired: 14 in]
      }
      frame "---------- SystemStatus ----------" {
        # "Template Separator\n(You can make a copy of, or modify, this frame)"
        n1026 = call <vilib>:"Add State(s) to Queue__JKI_lib_State_Machine.vi"("State(s) in (\"\")"=w2246) -> ("States Out"=w2245:string)  [unwired: 14 in]
      }
      frame "SystemStatus: SlowSysStatusMacro" {
        # "store system check time"
        # "Template Separator\n(You can make a copy of, or modify, this frame)"
        n1027 = Tick Count (ms)() -> (millisecond timer value=w2249:u32)
        n1028 = Bundle By Name(cluster=w2247, "SlowTimer"=w2249) -> (w2248:T23)
        n1029 = call <vilib>:"Add State(s) to Queue__JKI_lib_State_Machine.vi"("State(s) in Front (\"\")"="Digitizer: checkTemp\nTCP: CheckConnection" ("State(s) in Front (\"\")"), "State(s) in (\"\")"=w2254) -> ("States Out"=w2253:string)  [unwired: 13 in]
      }
      frame "SystemStatus: FastSysStatusMacro" {
        # "store system check time"
        # "Template Separator\n(You can make a copy of, or modify, this frame)"
        n1030 = Tick Count (ms)() -> (millisecond timer value=w2257:u32)
        n1031 = Bundle By Name(cluster=w2255, "FastTimer"=w2257) -> (w2256:T23)
        n1032 = call <vilib>:"Add State(s) to Queue__JKI_lib_State_Machine.vi"("State(s) in Front (\"\")"="355 Laser: CheckPWMStatus\nAimingBeam: GetPWMStatus\n/*355 Laser: CheckControllerStatus" ("State(s) in Front (\"\")"), "State(s) in (\"\")"=w2262) -> ("States Out"=w2261:string)  [unwired: 13 in]
      }
      frame "---------- UI ----------" {
        # "Do not put any code in this frame.\n(It is a separator no-op. You can make a copy of this frame to create a new UI frame)"
        n1033 = call <vilib>:"Add State(s) to Queue__JKI_lib_State_Machine.vi"("State(s) in (\"\")"=w2267) -> ("States Out"=w2266:string)  [unwired: 14 in]
      }
      frame "UI: Initialize" {
        w2269 = T44 {"Minimum"=0.0, "Maximum"=4.6, "Increment"=0.1} ("Data Entry Limits")
        w2268 = T11."Disabled and Grayed Out" ("Disabled")
        # "Disable all button on startup"
        # "Initialize the User Interface, here.\n(this is called automatically, by the Macro: Init)"
        n1034 = property on="V 1" class="DigNum (strict)"("DisabledEnum"=w2268) -> ()  [unwired: 2 in, 2 out]
        n1035 = property on="V 2" class="DigNum (strict)"("DisabledEnum"=w2268) -> ()  [unwired: 2 in, 2 out]
        n1036 = property on="StopButton" class="Bool (strict)"("DisabledEnum"=w2268) -> ()  [unwired: 2 in, 2 out]
        n1037 = property on="Sys Reconfig" class="Bool"("DisabledEnum"=w2268) -> ()  [unwired: 2 in, 2 out]
        n1038 = property on="StartButton" class="Bool (strict)"("DisabledEnum"=w2268) -> ()  [unwired: 2 in, 2 out]
        n1039 = property on="355nm Laser toggle" class="Bool (strict)"("DisabledEnum"=w2268) -> ()  [unwired: 2 in, 2 out]
        n1040 = property on="Aiming beam toggle" class="Bool (strict)"("DisabledEnum"=w2268) -> ()  [unwired: 2 in, 2 out]
        n1041 = property on="Background" class="Bool (strict)"("DisabledEnum"=w2268) -> ()  [unwired: 2 in, 2 out]
        n1042 = property on="Cali&iRF alignment" class="Bool (strict)"("DisabledEnum"=w2268) -> ()  [unwired: 2 in, 2 out]
        n1043 = property on="V 3" class="DigNum (strict)"("DisabledEnum"=w2268) -> ()  [unwired: 2 in, 2 out]
        n1044 = property on="Video Source" class="RadioBtnsControl (strict)"("DisabledEnum"=w2268) -> ()  [unwired: 2 in, 2 out]
        n1045 = property on="V 1" class="DigNum (strict)"("Data Range"=w2269) -> ()  [unwired: 2 in, 2 out]
        n1046 = property on="V 2" class="DigNum (strict)"("Data Range"=w2269) -> ()  [unwired: 2 in, 2 out]
        n1047 = property on="V 3" class="DigNum (strict)"("Data Range"=w2269) -> ()  [unwired: 2 in, 2 out]
        n1048 = call <vilib>:"Add State(s) to Queue__JKI_lib_State_Machine.vi"("State(s) in Front (\"\")"="UI: CaliAndiRFNotReady" ("State(s) in Front (\"\")"), "State(s) in (\"\")"=w2275) -> ("States Out"=w2274:string)  [unwired: 13 in]
      }
      frame "UI: BGLoaded" {
        # "[Covers: REQ24]"
        # "Do not put any code in this frame.\n(It is a separator no-op. You can make a copy of this frame to create a new UI frame)"
        n1049 = property on="Background" class="Bool (strict)"("BoolText.Text"="Loaded!" ("Boolean Text.Text"), "Colors [4]"=cluster{u32, u32}[] [{15764023, 15764023}, {16711680, 16711680}]) -> ()  [unwired: 2 in, 2 out]
        n1050 = call <vilib>:"Add State(s) to Queue__JKI_lib_State_Machine.vi"("State(s) in (\"\")"=w2282) -> ("States Out"=w2281:string)  [unwired: 14 in]
      }
      frame "UI: BGSizeError" {
        # "[Covers: REQ24]"
        # "Do not put any code in this frame.\n(It is a separator no-op. You can make a copy of this frame to create a new UI frame)"
        n1051 = property on="Background" class="Bool (strict)"("BoolText.Text"="Loaded!" ("Boolean Text.Text"), "Colors [4]"=cluster{u32, u32}[] [{7171459, 7171459}, {16711680, 16711680}]) -> ()  [unwired: 2 in, 2 out]
        n1052 = One Button Dialog(message="Background waveform length and current digitizer setting mismatch! Please take a new background before any aquisition!") -> ()  [unwired: 1 in, 1 out]
        n1053 = call <vilib>:"Add State(s) to Queue__JKI_lib_State_Machine.vi"("State(s) in (\"\")"=w2290) -> ("States Out"=w2289:string)  [unwired: 14 in]
      }
      frame "UI: CaliAndiRFLoaded" {
        # "[Covers: REQ24]"
        # "Do not put any code in this frame.\n(It is a separator no-op. You can make a copy of this frame to create a new UI frame)"
        n1054 = property on="Cali&iRF alignment" class="Bool (strict)"("BoolText.Text"="Loaded!" ("Boolean Text.Text"), "Colors [4]"=cluster{u32, u32}[] [{15764023, 15764023}, {16711680, 16711680}]) -> ()  [unwired: 2 in, 2 out]
        n1055 = call <vilib>:"Add State(s) to Queue__JKI_lib_State_Machine.vi"("State(s) in (\"\")"=w2297) -> ("States Out"=w2296:string)  [unwired: 14 in]
      }
      frame "UI: WFAutoScale" {
        # "Set graph auto scale.\n(UI: WFAutoScale >> T/F)"
        n1056 = Equal?(x=w2298, y="F") -> (x = y?=w2299:bool)
        n1057 = Equal?(x=w2298, y="T") -> (x = y?=w2301:bool)
        n1058 = case shown="True" w2301 {
          frame False {
          }
          frame True {
            w2317 = u8 2 ("Y Scale.Scale Fit")
            n1059 = property on="Channel 1" class="WFGraph (strict)"("YScale.ScaleFit"=w2317) -> ()  [unwired: 2 in, 2 out]
            n1060 = property on="Channel 2" class="WFGraph (strict)"("YScale.ScaleFit"=w2317) -> ()  [unwired: 2 in, 2 out]
            n1061 = property on="Channel 3" class="WFGraph (strict)"("YScale.ScaleFit"=w2317) -> ()  [unwired: 2 in, 2 out]
          }
        }
        n1062 = case shown="True" w2299 {
          frame False {
          }
          frame True {
            w2314 = 0.0 ("Y Scale.Range:Maximum")
            w2315 = 2.0 ("Y Scale.Range:Maximum")
            w2316 = u8 0 ("Y Scale.Scale Fit")
            n1063 = property on="Channel 1" class="WFGraph (strict)"("YScale.ScaleFit"=w2316) -> (error out=w2313:errorcluster)  [unwired: 2 in, 1 out]
            n1064 = property on="Channel 2" class="WFGraph (strict)"("YScale.ScaleFit"=w2316) -> (error out=w2312:errorcluster)  [unwired: 2 in, 1 out]
            n1065 = property on="Channel 3" class="WFGraph (strict)"("YScale.ScaleFit"=w2316) -> (error out=w2311:errorcluster)  [unwired: 2 in, 1 out]
            n1066 = property on="Channel 1" class="WFGraph (strict)"(error in=w2313, "YScale.Maximum"=w2315) -> (error out=w2310:errorcluster)  [unwired: 1 in, 1 out]
            n1067 = property on="Channel 2" class="WFGraph (strict)"(error in=w2312, "YScale.Maximum"=w2315) -> (error out=w2309:errorcluster)  [unwired: 1 in, 1 out]
            n1068 = property on="Channel 3" class="WFGraph (strict)"(error in=w2311, "YScale.Maximum"=w2315) -> (error out=w2308:errorcluster)  [unwired: 1 in, 1 out]
            n1069 = property on="Channel 1" class="WFGraph (strict)"(error in=w2310, "YScale.Minimum"=w2314) -> ()  [unwired: 1 in, 2 out]
            n1070 = property on="Channel 2" class="WFGraph (strict)"(error in=w2309, "YScale.Minimum"=w2314) -> ()  [unwired: 1 in, 2 out]
            n1071 = property on="Channel 3" class="WFGraph (strict)"(error in=w2308, "YScale.Minimum"=w2314) -> ()  [unwired: 1 in, 2 out]
          }
        }
        n1072 = call <vilib>:"Add State(s) to Queue__JKI_lib_State_Machine.vi"("State(s) in (\"\")"=w2307) -> ("States Out"=w2306:string)  [unwired: 14 in]
      }
      frame "UI: showDisclaimer" {
        # "Show disclamer window.\n(It is a separator no-op. You can make a copy of this frame to create a new UI frame)"
        n1073 = call <vilib>:"Application Directory.vi"() -> ("Application Directory"=w2330:path)
        n1074 = Build Path(base path=w2330, name or relative path="Disclamer.png") -> (appended path=w2328:path)
        n1075 = property on="Disclamer" class="Pict"() -> ("Draw Area Size"=w2326:T45)  [unwired: 2 in, 2 out]
        n1076 = disable-structure "Diagram Disable Structure" shown="Disabled" {
          frame Disabled {
            n1077 = flat-sequence {
              frame #0 {
                n1078 = call "disclaimer.vi"() -> ()  [unwired: 12 in]
              }
              frame #1 {
                n1079 = Wait (ms)(milliseconds to wait=u32 250) -> ()  [unwired: 1 out]
              }
              frame #2 {
                n1080 = call "SoftwareNote.vi"() -> ()  [unwired: 12 in]
              }
            }
          }
          frame Enabled {
          }
        }
        n1081 = call <vilib>:"Read PNG File.vi"("path to PNG file"=w2328) -> ("image data"=w2325:T46)  [unwired: 8 in, 2 out]
        n1082 = Unbundle By Name(w2325) -> ("Rectangle.right"=w2323:i16, "Rectangle.bottom"=w2321:i16)
        n1083 = Unbundle By Name(w2326) -> ("Width"=w2324:u32, "Height"=w2322:u32)
        n1084 = call <vilib>:"Draw Flattened Pixmap.vi"("image data"=w2325) -> ("new picture"=→"Disclamer":picture)  [unwired: 8 in]
        n1085 = Divide(x=w2324, y=w2323) -> (x/y=w2320:dbl)
        n1086 = Divide(x=w2322, y=w2321) -> (x/y=w2319:dbl)
        n1087 = Max & Min(x=w2320, y=w2319) -> (min(x,y)=w2318:dbl)  [unwired: 1 out]
        n1088 = property on="Disclamer" class="Pict"("ZoomFactor"=w2318) -> ()  [unwired: 2 in, 2 out]
        n1089 = call <vilib>:"Add State(s) to Queue__JKI_lib_State_Machine.vi"("State(s) in (\"\")"=w2335) -> ("States Out"=w2334:string)  [unwired: 14 in]
      }
      frame "UI: CaliAndiRFNotReady" {
        # "Do not put any code in this frame.\n(It is a separator no-op. You can make a copy of this frame to create a new UI frame)"
        n1090 = property on="Cali&iRF alignment" class="Bool (strict)"("BoolText.Text"="No Info" ("Boolean Text.Text"), "Colors [4]"=cluster{u32, u32}[] [{13816530, 13816530}, {16711680, 16711680}]) -> ()  [unwired: 2 in, 2 out]
        n1091 = call <vilib>:"Add State(s) to Queue__JKI_lib_State_Machine.vi"("State(s) in (\"\")"=w2343) -> ("States Out"=w2342:string)  [unwired: 14 in]
      }
      frame "UI: BGnotReady" {
        # "Do not put any code in this frame.\n(It is a separator no-op. You can make a copy of this frame to create a new UI frame)"
        n1092 = property on="Background" class="Bool (strict)"("BoolText.Text"="No Info" ("Boolean Text.Text"), "Colors [4]"=cluster{u32, u32}[] [{13816530, 13816530}, {16711680, 16711680}]) -> ()  [unwired: 2 in, 2 out]
        n1093 = call <vilib>:"Add State(s) to Queue__JKI_lib_State_Machine.vi"("State(s) in (\"\")"=w2350) -> ("States Out"=w2349:string)  [unwired: 14 in]
      }
      frame "UI: Reset" {
        w2352 = cluster{u32, u32}[] [{13816530, 13816530}, {13816530, 13816530}] ("Colors [4]")
        # "Do not put any code in this frame.\n(It is a separator no-op. You can make a copy of this frame to create a new UI frame)"
        n1094 = property on="Cali&iRF alignment" class="Bool (strict)"("BoolText.Text"="No Info" ("Boolean Text.Text"), "Colors [4]"=w2352) -> ()  [unwired: 2 in, 2 out]
        n1095 = property on="Background" class="Bool (strict)"("BoolText.Text"="No Info" ("Boolean Text.Text"), "Colors [4]"=w2352) -> ()  [unwired: 2 in, 2 out]
        n1096 = call <vilib>:"Add State(s) to Queue__JKI_lib_State_Machine.vi"("State(s) in (\"\")"=w2358) -> ("States Out"=w2357:string)  [unwired: 14 in]
      }
      frame "UI: SetButtonText" {
        # "Set button text of 355nm laser and aiming beam."
        n1097 = call <vilib>:"Add State(s) to Queue__JKI_lib_State_Machine.vi"("State(s) in (\"\")"=w2363) -> ("States Out"=w2362:string)  [unwired: 14 in]
      }
      frame "UI: DuringAquisition" {
        w2366 = T11."Disabled and Grayed Out" ("Disabled")
        # "Do not put any code in this frame.\n(It is a separator no-op. You can make a copy of this frame to create a new UI frame)"
        n1098 = Unbundle By Name(w2365) -> ("bothVidSourceAvail"=w2364:bool)
        n1099 = case shown="True" w2364 {
          tunnel: w2366 -> [_ w2372]
          frame False {
          }
          frame True {
            n1100 = property on="Video Source" class="RadioBtnsControl (strict)"("DisabledEnum"=w2372) -> ()  [unwired: 2 in, 2 out]
          }
        }
        n1101 = property on="StartButton" class="Bool (strict)"("DisabledEnum"=w2366) -> ()  [unwired: 2 in, 2 out]
        n1102 = property on="Sys Reconfig" class="Bool"("DisabledEnum"=w2366) -> ()  [unwired: 2 in, 2 out]
        n1103 = property on="355nm Laser toggle" class="Bool (strict)"("DisabledEnum"=w2366) -> ()  [unwired: 2 in, 2 out]
        n1104 = property on="Aiming beam toggle" class="Bool (strict)"("DisabledEnum"=w2366) -> ()  [unwired: 2 in, 2 out]
        n1105 = property on="Background" class="Bool (strict)"("DisabledEnum"=w2366) -> ()  [unwired: 2 in, 2 out]
        n1106 = property on="Radio Buttons" class="RadioBtnsControl (strict)"("DisabledEnum"=w2366) -> ()  [unwired: 2 in, 2 out]
        n1107 = property on="Cali&iRF alignment" class="Bool (strict)"("DisabledEnum"=w2366) -> ()  [unwired: 2 in, 2 out]
        n1108 = property on="Quit" class="Bool"("DisabledEnum"=w2366) -> ()  [unwired: 2 in, 2 out]
        n1109 = property on="Skip Data Save?" class="Bool (strict)"("DisabledEnum"=w2366) -> ()  [unwired: 2 in, 2 out]
        n1110 = property on="Video Display" class="Bool (strict)"("DisabledEnum"=w2366) -> ()  [unwired: 2 in, 2 out]
        n1111 = property on="StopButton" class="Bool (strict)"("DisabledEnum"=T11."Enabled" ("Disabled")) -> ()  [unwired: 2 in, 2 out]
        n1112 = call <vilib>:"Add State(s) to Queue__JKI_lib_State_Machine.vi"("State(s) in (\"\")"=w2371) -> ("States Out"=w2370:string)  [unwired: 14 in]
      }
      frame "UI: duringIRFAlign" {
        w2373 = T11."Disabled and Grayed Out" ("Disabled")
        # "Set UI to during iRF alignment\n(It is a separator no-op. You can make a copy of this frame to create a new UI frame)"
        n1113 = property on="StartButton" class="Bool (strict)"("DisabledEnum"=w2373) -> ()  [unwired: 2 in, 2 out]
        n1114 = property on="Sys Reconfig" class="Bool"("DisabledEnum"=w2373) -> ()  [unwired: 2 in, 2 out]
        n1115 = property on="355nm Laser toggle" class="Bool (strict)"("DisabledEnum"=w2373) -> ()  [unwired: 2 in, 2 out]
        n1116 = property on="Aiming beam toggle" class="Bool (strict)"("DisabledEnum"=w2373) -> ()  [unwired: 2 in, 2 out]
        n1117 = property on="Background" class="Bool (strict)"("DisabledEnum"=w2373) -> ()  [unwired: 2 in, 2 out]
        n1118 = property on="StopButton" class="Bool (strict)"("DisabledEnum"=w2373) -> ()  [unwired: 2 in, 2 out]
        n1119 = call <vilib>:"Add State(s) to Queue__JKI_lib_State_Machine.vi"("State(s) in (\"\")"=w2378) -> ("States Out"=w2377:string)  [unwired: 14 in]
      }
      frame "UI: duringBGAcquire" {
        w2379 = T11."Disabled and Grayed Out" ("Disabled")
        # "Do not put any code in this frame.\n(It is a separator no-op. You can make a copy of this frame to create a new UI frame)"
        n1120 = property on="StartButton" class="Bool (strict)"("DisabledEnum"=w2379) -> ()  [unwired: 2 in, 2 out]
        n1121 = property on="StopButton" class="Bool (strict)"("DisabledEnum"=w2379) -> ()  [unwired: 2 in, 2 out]
        n1122 = property on="Sys Reconfig" class="Bool"("DisabledEnum"=w2379) -> ()  [unwired: 2 in, 2 out]
        n1123 = property on="355nm Laser toggle" class="Bool (strict)"("DisabledEnum"=w2379) -> ()  [unwired: 2 in, 2 out]
        n1124 = property on="Aiming beam toggle" class="Bool (strict)"("DisabledEnum"=w2379) -> ()  [unwired: 2 in, 2 out]
        n1125 = property on="Cali&iRF alignment" class="Bool (strict)"("DisabledEnum"=w2379) -> ()  [unwired: 2 in, 2 out]
        n1126 = call <vilib>:"Add State(s) to Queue__JKI_lib_State_Machine.vi"("State(s) in (\"\")"=w2384) -> ("States Out"=w2383:string)  [unwired: 14 in]
      }
      frame "UI: ReadyForAquisition" {
        w2388 = T11."Enabled" ("Disabled")
        # "Do not put any code in this frame.\n(It is a separator no-op. You can make a copy of this frame to create a new UI frame)"
        n1127 = Unbundle By Name(w2387) -> ("System Status.TCP/IP"=w2386:bool, "bothVidSourceAvail"=w2385:bool)
        n1128 = property on="StartButton" class="Bool (strict)"("DisabledEnum"=w2388) -> ()  [unwired: 2 in, 2 out]
        n1129 = property on="Sys Reconfig" class="Bool"("DisabledEnum"=w2388) -> ()  [unwired: 2 in, 2 out]
        n1130 = property on="355nm Laser toggle" class="Bool (strict)"("DisabledEnum"=w2388) -> ()  [unwired: 2 in, 2 out]
        n1131 = property on="Aiming beam toggle" class="Bool (strict)"("DisabledEnum"=w2388) -> ()  [unwired: 2 in, 2 out]
        n1132 = property on="Cali&iRF alignment" class="Bool (strict)"("DisabledEnum"=w2388) -> ()  [unwired: 2 in, 2 out]
        n1133 = property on="Background" class="Bool (strict)"("DisabledEnum"=w2388) -> ()  [unwired: 2 in, 2 out]
        n1134 = property on="Quit" class="Bool"("DisabledEnum"=w2388) -> ()  [unwired: 2 in, 2 out]
        n1135 = property on="Radio Buttons" class="RadioBtnsControl (strict)"("DisabledEnum"=w2388) -> ()  [unwired: 2 in, 2 out]
        n1136 = case shown="True" w2385 {
          tunnel: w2388 -> [_ w2394]
          frame False {
          }
          frame True {
            n1137 = property on="Video Source" class="RadioBtnsControl (strict)"("DisabledEnum"=w2394) -> ()  [unwired: 2 in, 2 out]
          }
        }
        n1138 = property on="Skip Data Save?" class="Bool (strict)"("DisabledEnum"=w2388) -> ()  [unwired: 2 in, 2 out]
        n1139 = case shown="True" w2386 {
          tunnel: w2388 -> [_ w2395]
          frame False {
          }
          frame True {
            n1140 = property on="Video Display" class="Bool (strict)"("DisabledEnum"=w2395) -> ()  [unwired: 2 in, 2 out]
          }
        }
        n1141 = property on="StopButton" class="Bool (strict)"("DisabledEnum"=T11."Disabled and Grayed Out" ("Disabled")) -> ()  [unwired: 2 in, 2 out]
        n1142 = call <vilib>:"Add State(s) to Queue__JKI_lib_State_Machine.vi"("State(s) in (\"\")"=w2393) -> ("States Out"=w2392:string)  [unwired: 14 in]
      }
      frame "UI: Update" {
        # "Do not put any code in this frame.\n(It is a separator no-op. You can make a copy of this frame to create a new UI frame)"
        n1143 = Unbundle By Name(w2406) -> ("System Status"=→"System Hardware Connection Status":T2, "IDs.RunID"=→"Run #":i8, "CaseID"=→"Case #":string, "FLImDAQ"=→"FLImDAQ":T30, "SysRunning?"=→"Aquisition Status:":bool, "LJ Pinout"=→"LJ Pinout":T4, "IDs.BG ID"=→"BG #":i8, "IDs.Cali ID"=→"Calibration #":i8, "video source"=→"Visualization PC video source":T1)
        n1144 = call <vilib>:"Add State(s) to Queue__JKI_lib_State_Machine.vi"("State(s) in (\"\")"=w2409) -> ("States Out"=w2408:string)  [unwired: 14 in]
      }
      frame "UI: updateVideoToggle" {
        # "Set video toggle based on visualization PC video source.\n(take )"
        n1145 = call <vilib>:"Add State(s) to Queue__JKI_lib_State_Machine.vi"("State(s) in (\"\")"=w2414) -> ("States Out"=w2413:string)  [unwired: 14 in]
      }
      frame "UI: Cursor Set" {
        # "Argument"
        # "Set and Unset Cursor Busy.\n(Usage: \"UI: Cursor Set >> Busy|Idle\")"
        n1146 = case shown="\"Idle\", Default" w2416 {
          tunnel: w2418 -> [w2423 w2425]
          tunnel: [w2422 w2424] -> w2417
          frame "Idle", Default {
            n1147 = call <vilib>:"Unset Busy.vi"("error in (no error)"=w2423) -> ("error out"=w2422:errorcluster)  [unwired: 10 in]
          }
          frame "Busy" {
            n1148 = call <vilib>:"Set Busy.vi"("error in (no error)"=w2425) -> ("error out"=w2424:errorcluster)  [unwired: 9 in, 1 out]
          }
        }
        n1149 = call <vilib>:"Add State(s) to Queue__JKI_lib_State_Machine.vi"("State(s) in (\"\")"=w2421) -> ("States Out"=w2420:string)  [unwired: 14 in]
      }
      frame "UI: Front Panel State" {
        # "Argument"
        # "Set Front Panel Open or Closed\n(Usage: \"UI: Front Panel State >> Open|Close\")"
        n1150 = Unbundle By Name(w2429) -> ("Core.Current VI Reference"=w2428:refnum<vi>)
        n1151 = case shown="\"Open\", \"Standard\", Default" w2427 {
          tunnel: w2431 -> [w2439 w2454 w2465 w2478 w2491]
          tunnel: [w2441 w2455 w2467 w2480 w2493] -> w2430
          tunnel: w2428 -> [w2440 w2452 w2466 w2479 w2492]
          frame "Open", "Standard", Default {
            w2434 = T17."Standard" ("State")
            n1152 = property on="Property Node" class="VI"(reference=w2440, error in=w2439) -> (reference out=w2437:refnum<vi>, error out=w2438:errorcluster, "FP.State"=w2436:T17)
            n1153 = Not Equal?(x=w2436, y=w2434) -> (x != y?=w2435:bool)
            n1154 = case shown="True" w2435 {
              tunnel: [w2445 w2447] -> w2441
              tunnel: w2438 -> [w2444 w2447]
              tunnel: w2437 -> [w2443 _]
              tunnel: w2434 -> [w2442 _]
              frame True {
                n1155 = invoke on="Invoke Node" class="VI" method="FP.Open"(reference=w2443, error in=w2444, "Activate"=TRUE, "State"=w2442) -> (error out=w2445:errorcluster)  [unwired: 1 in, 4 out]
              }
              frame False {
              }
            }
          }
          frame "Close", "Closed" {
            n1156 = property on="Property Node" class="VI"(reference=w2452, error in=w2454) -> (reference out=w2451:refnum<vi>, error out=w2453:errorcluster, "FP.State"=w2449:T17)
            n1157 = Not Equal?(x=w2449, y=T17."Closed" ("Front Panel Window:State")) -> (x != y?=w2448:bool)
            n1158 = case shown="True" w2448 {
              tunnel: [w2456 w2459] -> w2455
              tunnel: w2453 -> [w2456 w2458]
              tunnel: w2451 -> [_ w2457]
              frame False {
              }
              frame True {
                n1159 = invoke on="Invoke Node" class="VI" method="FP.Close"(reference=w2457, error in=w2458) -> (error out=w2459:errorcluster)  [unwired: 1 in, 2 out]
              }
            }
          }
          frame "Hidden", "Hide" {
            w2460 = T17."Hidden" ("State")
            n1160 = property on="Property Node" class="VI"(reference=w2466, error in=w2465) -> (reference out=w2463:refnum<vi>, error out=w2464:errorcluster, "FP.State"=w2462:T17)
            n1161 = Not Equal?(x=w2462, y=w2460) -> (x != y?=w2461:bool)
            n1162 = case shown="True" w2461 {
              tunnel: [w2471 w2472] -> w2467
              tunnel: w2464 -> [w2470 w2472]
              tunnel: w2463 -> [w2469 _]
              tunnel: w2460 -> [w2468 _]
              frame True {
                n1163 = invoke on="Invoke Node" class="VI" method="FP.Open"(reference=w2469, error in=w2470, "State"=w2468) -> (error out=w2471:errorcluster)  [unwired: 2 in, 4 out]
              }
              frame False {
              }
            }
          }
          frame "Minimize", "Minimized" {
            w2473 = T17."Minimized" ("State")
            n1164 = property on="Property Node" class="VI"(reference=w2479, error in=w2478) -> (reference out=w2476:refnum<vi>, error out=w2477:errorcluster, "FP.State"=w2475:T17)
            n1165 = Not Equal?(x=w2475, y=w2473) -> (x != y?=w2474:bool)
            n1166 = case shown="True" w2474 {
              tunnel: [w2484 w2485] -> w2480
              tunnel: w2477 -> [w2483 w2485]
              tunnel: w2476 -> [w2482 _]
              tunnel: w2473 -> [w2481 _]
              frame True {
                n1167 = invoke on="Invoke Node" class="VI" method="FP.Open"(reference=w2482, error in=w2483, "State"=w2481) -> (error out=w2484:errorcluster)  [unwired: 2 in, 4 out]
              }
              frame False {
              }
            }
          }
          frame "Maximize", "Maximized" {
            w2486 = T17."Maximized" ("State")
            n1168 = property on="Property Node" class="VI"(reference=w2492, error in=w2491) -> (reference out=w2489:refnum<vi>, error out=w2490:errorcluster, "FP.State"=w2488:T17)
            n1169 = Not Equal?(x=w2488, y=w2486) -> (x != y?=w2487:bool)
            n1170 = case shown="True" w2487 {
              tunnel: [w2497 w2498] -> w2493
              tunnel: w2490 -> [w2496 w2498]
              tunnel: w2489 -> [w2495 _]
              tunnel: w2486 -> [w2494 _]
              frame True {
                n1171 = invoke on="Invoke Node" class="VI" method="FP.Open"(reference=w2495, error in=w2496, "State"=w2494) -> (error out=w2497:errorcluster)  [unwired: 2 in, 4 out]
              }
              frame False {
              }
            }
          }
        }
        n1172 = call <vilib>:"Add State(s) to Queue__JKI_lib_State_Machine.vi"("State(s) in (\"\")"=w2433) -> ("States Out"=w2432:string)  [unwired: 14 in]
      }
      frame "---------- AimingBeam ----------" {
        # "Template Separator\n(You can make a copy of, or modify, this frame)"
        n1173 = call <vilib>:"Add State(s) to Queue__JKI_lib_State_Machine.vi"("State(s) in (\"\")"=w2503) -> ("States Out"=w2502:string)  [unwired: 14 in]
      }
      frame "AimingBeam: Initialize" {
        # "set aiming beam button color"
        # "Open COM port for Aiming Beam\n(Require USB connection)"
        n1174 = Unbundle By Name(w2505) -> ("AB Cluster.Aiming Beam COM Port"=w2513:refnum<visa-resource-name>)
        n1175 = call-poly "VISA Configure Serial Port"("VISA resource name"=w2513, "Enable Termination\nChar (T)"=TRUE ("Enable Termination\nChar (T)"), "baud rate (9600)"=u32 9600, "error in (no error)"=w2510) -> ("error out"=w2509:errorcluster)  [unwired: 10 in, 1 out]
        n1176 = Unbundle By Name(w2509) -> ("status"=w2508:bool)
        n1177 = Not(x=w2508) -> (.not. x?=w2507:bool)
        n1178 = Bundle By Name(cluster=w2505, "System Status.Aiming Beam"=w2507) -> (w2506:T23)
        n1179 = call <vilib>:"Add State(s) to Queue__JKI_lib_State_Machine.vi"("State(s) in (\"\")"=w2515) -> ("States Out"=w2514:string)  [unwired: 14 in]
      }
      frame "AimingBeam: Close" {
        # "Close Aiming Beam COM port\n(Require USB connection to Aiming Beam Laser)"
        n1180 = Unbundle By Name(w2518) -> ("AB Cluster.Aiming Beam COM Port"=w2522:refnum<visa-resource-name>)
        n1181 = VISA Close(VISA resource name=w2522, error in (no error)=w2520) -> (error out=w2521:errorcluster)
        n1182 = Bundle By Name(cluster=w2518, "System Status.Aiming Beam"=FALSE) -> (w2519:T23)
        n1183 = call <vilib>:"Add State(s) to Queue__JKI_lib_State_Machine.vi"("State(s) in (\"\")"=w2524) -> ("States Out"=w2523:string)  [unwired: 14 in]
      }
      frame "AimingBeam: Set Current" {
        # "Set Aiming Beam Current\n(You can make a copy of, or modify, this frame)"
        n1184 = Unbundle By Name(w2536) -> ("AB Cluster.Aiming Beam COM Port"=w2529:refnum<visa-resource-name>)
        n1185 = Number To Fractional String(number="488nm Power", precision (6)=i16 2) -> (F-format string=w2530:string)  [unwired: 2 in]
        n1186 = Concatenate Strings("slc:", w2530, "\r" ("Carriage Return Constant"), "\n" ("Line Feed Constant")) -> (w2533:string)
        n1187 = VISA Write(VISA resource name=w2529, write buffer=w2533, error in (no error)=w2527) -> (error out=w2528:errorcluster)  [unwired: 2 out]
        n1188 = call <vilib>:"Add State(s) to Queue__JKI_lib_State_Machine.vi"("State(s) in (\"\")"=w2538) -> ("States Out"=w2537:string)  [unwired: 14 in]
      }
      frame "AimingBeam: Set ACC Status" {
        # "Enable Aiming Beam\n(Usage: \"AimingBeam: Set >> Enable|Disable\")"
        n1189 = Unbundle By Name(w2545) -> ("AB Cluster.Aiming Beam COM Port"=w2542:refnum<visa-resource-name>)
        n1190 = case shown="\"Enable\"" w2544 {
          tunnel: [w2548 w2552] -> w2543
          frame "Disable", Default {
            n1191 = Concatenate Strings("cof", "\r" ("Carriage Return Constant"), "\n" ("Line Feed Constant")) -> (w2548:string)
          }
          frame "Enable" {
            n1192 = Concatenate Strings("con", "\r" ("Carriage Return Constant"), "\n" ("Line Feed Constant")) -> (w2552:string)
          }
        }
        n1193 = VISA Write(VISA resource name=w2542, write buffer=w2543, error in (no error)=w2540) -> (error out=w2541:errorcluster)  [unwired: 2 out]
        n1194 = call <vilib>:"Add State(s) to Queue__JKI_lib_State_Machine.vi"("State(s) in (\"\")"=w2547) -> ("States Out"=w2546:string)  [unwired: 14 in]
      }
      frame "AimingBeam: Set APC Status" {
        # "Enable Aiming Beam\n(Usage: \"AimingBeam: Set >> Enable|Disable\")"
        n1195 = Unbundle By Name(w2562) -> ("AB Cluster.Aiming Beam COM Port"=w2559:refnum<visa-resource-name>)
        n1196 = case shown="\"Disable\", Default" w2561 {
          tunnel: [w2565 w2569] -> w2560
          frame "Disable", Default {
            n1197 = Concatenate Strings("lof", "\r" ("Carriage Return Constant"), "\n" ("Line Feed Constant")) -> (w2565:string)
          }
          frame "Enable" {
            n1198 = Concatenate Strings("lon", "\r" ("Carriage Return Constant"), "\n" ("Line Feed Constant")) -> (w2569:string)
          }
        }
        n1199 = VISA Write(VISA resource name=w2559, write buffer=w2560, error in (no error)=w2557) -> (error out=w2558:errorcluster)  [unwired: 2 out]
        n1200 = call <vilib>:"Add State(s) to Queue__JKI_lib_State_Machine.vi"("State(s) in (\"\")"=w2564) -> ("States Out"=w2563:string)  [unwired: 14 in]
      }
      frame "AimingBeam: GetPWMStatus" {
        # "Get aiming beam PWM status\n()"
        n1201 = Unbundle By Name(w2577) -> ("AB Cluster.Freq"=w2576:i32, "LJ Pinout.AimingBeam PWM"=w2583:string)
        n1202 = Equal To 0?(x=w2576) -> (x = 0?=w2575:bool)
        n1203 = call "LabJack_FGV.vi"("Operation(Read)"=enum16{"Write", "Read"}."Read" ("Operation"), "error in (no error)"=w2579) -> ("error out"=w2581:errorcluster, "Read data"=w2582:i32)  [unwired: 8 in]
        n1204 = case shown="True" w2575 {
          tunnel: w2583 -> [w2596 _]
          tunnel: [w2594 "DIO_STATE"] -> w2580
          frame False {
            n1205 = Concatenate Strings(w2596, "_EF_ENABLE" ("string")) -> (w2594:string)
          }
          frame True {
          }
        }
        n1206 = call "LJM_eReadName.vi"("Handle In"=w2582, "Name"=w2580, "error in"=w2581) -> ("Value"=w2574:dbl, "error out"=w2578:errorcluster)  [unwired: 10 in, 1 out]
        n1207 = case shown="True" w2575 {
          tunnel: w2574 -> [w2589 w2593]
          tunnel: [w2588 w2590] -> w2573
          frame False {
            n1208 = Greater Than 0?(x=w2589) -> (x > 0?=w2588:bool)
          }
          frame True {
            n1209 = Number To Boolean Array(number=w2593) -> (Boolean array=w2592:bool[])
            n1210 = Index Array(array=w2592, index=3) -> (element=w2590:bool)
          }
        }
        n1211 = case shown="False" w2573 {
          frame False {
            # "PWM is off\nset color to dark green"
            n1212 = local write "Aiming beam toggle"(FALSE ("Aimging beam")) -> ()
          }
          frame True {
            # "PWM is on\nset color to light green"
            n1213 = local write "Aiming beam toggle"(TRUE ("Aimging beam")) -> ()
          }
        }
        n1214 = call <vilib>:"Add State(s) to Queue__JKI_lib_State_Machine.vi"("State(s) in (\"\")"=w2587) -> ("States Out"=w2586:string)  [unwired: 14 in]
      }
      frame "---------- 355 Laser ----------" {
        # "Template Separator\n(You can make a copy of, or modify, this frame)"
        n1215 = call <vilib>:"Add State(s) to Queue__JKI_lib_State_Machine.vi"("State(s) in (\"\")"=w2604) -> ("States Out"=w2603:string)  [unwired: 14 in]
      }
      frame "355 Laser: Check Dewelling" {
        # "if time laser start time is less than 7.5s before, wait 250ms then check again."
        # "Template Separator\n(You can make a copy of, or modify, this frame)"
        n1216 = Unbundle By Name(w2612) -> ("Laser start tic"=w2609:u32)
        n1217 = Tick Count (ms)() -> (millisecond timer value=w2610:u32)
        n1218 = Subtract(x=w2610, y=w2609) -> (x-y=w2608:u32)
        n1219 = Greater?(x=w2608, y=u32 5000) -> (0:w2606:bool)
        n1220 = case shown="False" w2606 {
          tunnel: ["355 Laser: Check Dewelling" ""] -> w2605
          frame False {
            n1221 = Wait (ms)(milliseconds to wait=u32 250) -> ()  [unwired: 1 out]
          }
          frame True {
          }
        }
        n1222 = call <vilib>:"Add State(s) to Queue__JKI_lib_State_Machine.vi"("State(s) in Front (\"\")"=w2605, "State(s) in (\"\")"=w2615) -> ("States Out"=w2614:string)  [unwired: 13 in]
      }
      frame "355 Laser: Laser enable" {
        # "Laser enable/disable\n(Usage: \"LabJack: Laser enable/disable >> 1|0\")"
        n1223 = Unbundle By Name(w2622) -> ("LJ Pinout.Laser Start/Stop"=w2626:string, "System Status.355 Laser"=w2620:bool)
        n1224 = case shown="False" w2620 {
          tunnel: w2619 -> [w2641 w2642]
          tunnel: w2626 -> [w2635 _]
          tunnel: [w2630 w2642] -> w2624
          tunnel: [w2629 u32 0 ("millisecond timer value")] -> w2621
          frame False {
            n1225 = call "LabJack_FGV.vi"("Operation(Read)"=enum16{"Write", "Read"}."Read" ("Operation")) -> ("Read data"=w2637:i32)  [unwired: 9 in, 1 out]
            n1226 = call "LJM_eWriteName.vi"("Handle In"=w2637, "Name"=w2635, "Value"=1.0, "error in"=w2641) -> ("Handle Out"=w2636:i32, "error out"=w2634:errorcluster)  [unwired: 10 in]
            n1227 = call <userlib>:"Wait (ms)__ogtk.vi"("error in (no error)"=w2634, "milliseconds to wait"=u32 250) -> ("error out"=w2633:errorcluster)  [unwired: 8 in, 1 out]
            n1228 = call "LJM_eWriteName.vi"("Handle In"=w2636, "Name"=w2635, "Value"=0.0, "error in"=w2633) -> ("error out"=w2631:errorcluster)  [unwired: 10 in, 1 out]
            n1229 = call <userlib>:"Tick Count (ms)__ogtk.vi"("error in (no error)"=w2631) -> ("error out"=w2630:errorcluster, "millisecond timer value"=w2629:u32)  [unwired: 9 in]
          }
          frame True {
          }
        }
        n1230 = Bundle By Name(cluster=w2622, "Laser start tic"=w2621) -> (w2623:T23)
        n1231 = call <vilib>:"Add State(s) to Queue__JKI_lib_State_Machine.vi"("State(s) in (\"\")"=w2628) -> ("States Out"=w2627:string)  [unwired: 14 in]
      }
      frame "355 Laser: Laser disable" {
        # "Laser enable/disable\n(Usage: \"LabJack: Laser enable/disable >> 1|0\")"
        n1232 = Unbundle By Name(w2646) -> ("LJ Pinout.Laser Start/Stop"=w2650:string, "System Status.355 Laser"=w2644:bool)
        n1233 = case shown="True" w2644 {
          tunnel: w2651 -> [w2654 w2668]
          tunnel: w2650 -> [_ w2662]
          tunnel: [w2654 w2657] -> w2648
          tunnel: [u32 0 ("millisecond timer value") w2656] -> w2645
          frame False {
          }
          frame True {
            n1234 = call "LabJack_FGV.vi"("Operation(Read)"=enum16{"Write", "Read"}."Read" ("Operation")) -> ("Read data"=w2664:i32)  [unwired: 9 in, 1 out]
            n1235 = call "LJM_eWriteName.vi"("Handle In"=w2664, "Name"=w2662, "Value"=1.0, "error in"=w2668) -> ("Handle Out"=w2663:i32, "error out"=w2661:errorcluster)  [unwired: 10 in]
            n1236 = call <userlib>:"Wait (ms)__ogtk.vi"("error in (no error)"=w2661, "milliseconds to wait"=u32 250) -> ("error out"=w2660:errorcluster)  [unwired: 8 in, 1 out]
            n1237 = call "LJM_eWriteName.vi"("Handle In"=w2663, "Name"=w2662, "Value"=0.0, "error in"=w2660) -> ("error out"=w2658:errorcluster)  [unwired: 10 in, 1 out]
            n1238 = call <userlib>:"Tick Count (ms)__ogtk.vi"("error in (no error)"=w2658) -> ("error out"=w2657:errorcluster, "millisecond timer value"=w2656:u32)  [unwired: 9 in]
          }
        }
        n1239 = Bundle By Name(cluster=w2646, "Laser start tic"=w2645) -> (w2647:T23)
        n1240 = call <vilib>:"Add State(s) to Queue__JKI_lib_State_Machine.vi"("State(s) in (\"\")"=w2653) -> ("States Out"=w2652:string)  [unwired: 14 in]
      }
      frame "355 Laser: Dewelling" {
        # "Wait some time (ms)\n(355 Laser: Dewelling >> #)"
        n1241 = Fract/Exp String To Number(string=w2672, default (0 dbl)=0) -> (number=w2670:i32)  [unwired: 2 in, 1 out]
        n1242 = Wait (ms)(milliseconds to wait=w2670) -> ()  [unwired: 1 out]
        n1243 = call <vilib>:"Add State(s) to Queue__JKI_lib_State_Machine.vi"("State(s) in (\"\")"=w2676) -> ("States Out"=w2675:string)  [unwired: 14 in]
      }
      frame "355 Laser: Close" {
        # "Template Separator\n(You can make a copy of, or modify, this frame)"
        n1244 = call <vilib>:"Add State(s) to Queue__JKI_lib_State_Machine.vi"("State(s) in Front (\"\")"="355 Laser: CheckControllerStatus\n355 Laser: Laser disable\n355 Laser: Dewelling >>1000", "State(s) in (\"\")"=w2682) -> ("States Out"=w2681:string)  [unwired: 13 in]
      }
      frame "355 Laser: CheckControllerStatus" {
        # "if average < 2, laser no power\nif average 2 < average < 9.3, laser on\nif 9.3<average<10, interlock open, blink indicator\nif average > 10, laser off\n[Covers: REQ30]"
        # "take 10 measuremt and look at average"
        # "Check 355 laser controller status\nBy probing Emisison Lamp negative terminal voltage"
        n1245 = Unbundle By Name(w2691) -> ("LJ Pinout.Laser Ready"=w2694:string)
        n1246 = call "LabJack_FGV.vi"("Operation(Read)"=enum16{"Write", "Read"}."Read" ("Operation")) -> ("Read data"=w2695:i32)  [unwired: 9 in, 1 out]
        n1247 = for {
          N: 20 -> [_]
          tunnel: w2695 -> [w2706]
          tunnel: w2694 -> [w2705]
          shift-right: [w2704] -> w2687
          shift-left: w2693 -> [w2703]
          tunnel: [w2701] -> w2686 mode=indexing
          n1248 = call "LJM_eReadName.vi"("Handle In"=w2706, "Name"=w2705, "error in"=w2703) -> ("Value"=w2701:dbl, "error out"=w2704:errorcluster)  [unwired: 10 in, 1 out]
          n1249 = Wait (ms)(milliseconds to wait=u32 25) -> ()  [unwired: 1 out]
        }
        n1250 = call "checkLaserStatus.vi"("error in (no error)"=w2687, "Laser LED voltage"=w2686) -> ("error out"=w2688:errorcluster, "Interlock open?"=w2683:bool, "Laser on?"=w2685:bool, "Mean voltage"=→"laser EM lamp V":dbl)  [unwired: 6 in]
        n1251 = Bundle By Name(cluster=w2691, "System Status.355 Laser"=w2685) -> (w2692:T23)
        n1252 = case shown="True" w2683 {
          frame False {
            n1253 = property on="355 Laser" class="Bool (strict)"("Blinking"=FALSE) -> ()  [unwired: 2 in, 2 out]
          }
          frame True {
            n1254 = property on="355 Laser" class="Bool (strict)"("Blinking"=TRUE) -> ()  [unwired: 2 in, 2 out]
          }
        }
        n1255 = call <vilib>:"Add State(s) to Queue__JKI_lib_State_Machine.vi"("State(s) in (\"\")"=w2698) -> ("States Out"=w2697:string)  [unwired: 14 in]
      }
      frame "355 Laser: CheckPWMStatus" {
        # "Check 355 laser PWM status\n(Read LJ DIO#EF_ENABLE register to determine PWM status)"
        n1256 = Unbundle By Name(w2716) -> ("LJ Pinout.355 PWM"=w2715:string)
        n1257 = call "LabJack_FGV.vi"("Operation(Read)"=enum16{"Write", "Read"}."Read" ("Operation"), "error in (no error)"=w2709) -> ("error out"=w2712:errorcluster, "Read data"=w2713:i32)  [unwired: 8 in]
        n1258 = Concatenate Strings(w2715, "_EF_ENABLE" ("string")) -> (w2711:string)
        n1259 = call "LJM_eReadName.vi"("Handle In"=w2713, "Name"=w2711, "error in"=w2712) -> ("Value"=w2708:dbl, "error out"=w2710:errorcluster)  [unwired: 10 in, 1 out]
        n1260 = Greater Than 0?(x=w2708) -> (x > 0?=w2707:bool)
        n1261 = case shown="False" w2707 {
          frame False {
            # "PWM is off\nset color to gray"
            n1262 = local write "355nm Laser toggle"(FALSE ("355nm Laser")) -> ()
          }
          frame True {
            # "PWM is on\nset color to light green"
            n1263 = local write "355nm Laser toggle"(TRUE ("355nm Laser")) -> ()
          }
        }
        n1264 = call <vilib>:"Add State(s) to Queue__JKI_lib_State_Machine.vi"("State(s) in (\"\")"=w2720) -> ("States Out"=w2719:string)  [unwired: 14 in]
      }
      frame "355 Laser: Start" {
        # "Template Separator\n(You can make a copy of, or modify, this frame)"
        n1265 = call <vilib>:"Add State(s) to Queue__JKI_lib_State_Machine.vi"("State(s) in Front (\"\")"="LabJack: 355_PWM_Start", "State(s) in (\"\")"=w2728) -> ("States Out"=w2727:string)  [unwired: 13 in]
      }
      frame "355 Laser: Stop" {
        # "Template Separator\n(You can make a copy of, or modify, this frame)"
        n1266 = call <vilib>:"Add State(s) to Queue__JKI_lib_State_Machine.vi"("State(s) in Front (\"\")"="LabJack: 355_PWM_Stop", "State(s) in (\"\")"=w2734) -> ("States Out"=w2733:string)  [unwired: 13 in]
      }
      frame "---------- Utility ----------" {
        # "Template Separator\n(You can make a copy of, or modify, this frame)"
        n1267 = call <vilib>:"Add State(s) to Queue__JKI_lib_State_Machine.vi"("State(s) in (\"\")"=w2739) -> ("States Out"=w2738:string)  [unwired: 14 in]
      }
      frame "Utility: SetDataClass" {
        # "Set Data Class in Queues\n(Set data class to either Data, Bg or Cali)"
        n1268 = case shown="\"Cali\"" w2741 {
          tunnel: [enum16{"Data", "BG", "Cali"}."Data" ("Data Class") enum16{"Data", "BG", "Cali"}."BG" ("Data Class") enum16{"Data", "BG", "Cali"}."Cali" ("Data Class")] -> w2740
          frame "Data", Default {
          }
          frame "Bg" {
          }
          frame "Cali" {
          }
        }
        n1269 = local write "Data Class"(w2740) -> ()
        n1270 = call <vilib>:"Add State(s) to Queue__JKI_lib_State_Machine.vi"("State(s) in (\"\")"=w2746) -> ("States Out"=w2745:string)  [unwired: 14 in]
      }
      frame "Utility: AquiTimerReset" {
        # "Set Aquisition Timer\n(You can make a copy of, or modify, this frame)"
        n1271 = Tick Count (ms)() -> (millisecond timer value=w2752:u32)
        n1272 = Bundle By Name(cluster=w2750, "Aquisition Timer"=w2752) -> (w2751:T23)
        n1273 = call <vilib>:"Add State(s) to Queue__JKI_lib_State_Machine.vi"("State(s) in (\"\")"=w2756) -> ("States Out"=w2755:string)  [unwired: 14 in]
      }
      frame "Utility: AquiTimerCheck" {
        # "5min to ms"
        # "Set Aquisition Timer\n([Covers: REQ35])"
        n1274 = Unbundle By Name(w2764) -> ("Aquisition Timer"=w2762:u32)
        n1275 = Tick Count (ms)() -> (millisecond timer value=w2763:u32)
        n1276 = Subtract(x=w2763, y=w2762) -> (x-y=w2761:u32)
        n1277 = Multiply(x=1000, y=300) -> (x*y=w2758:i32)
        n1278 = Greater Or Equal?(x=w2761, y=w2758) -> (x >= y?=w2757:bool)
        n1279 = case shown="True" w2757 {
          frame False {
            # "do nothing"
          }
          frame True {
            # "if timed out, stop aquisition"
            n1280 = property on="StopButton" class="Bool (strict)"("Val(Sgnl)"=TRUE ("Value (Signaling)")) -> ()  [unwired: 2 in, 2 out]
          }
        }
        n1281 = call <vilib>:"Add State(s) to Queue__JKI_lib_State_Machine.vi"("State(s) in (\"\")"=w2768) -> ("States Out"=w2767:string)  [unwired: 14 in]
      }
      frame "Utility: StartBeep" {
        # "Beep\n([Covers: REQ18])"
        n1282 = call <vilib>:"Beep.vi"("use system alert? (T)"=FALSE, "duration (msec)"=u32 1000, "frequency (Hz)"=u32 2000) -> ()  [unwired: 9 in]
        n1283 = call <vilib>:"Add State(s) to Queue__JKI_lib_State_Machine.vi"("State(s) in (\"\")"=w2777) -> ("States Out"=w2776:string)  [unwired: 14 in]
      }
      frame "Utility: EndBeep" {
        # "Beep\n([Covers: REQ18])"
        n1284 = flat-sequence {
          frame #0 {
            n1285 = call <vilib>:"Beep.vi"("use system alert? (T)"=FALSE, "duration (msec)"=u32 500, "frequency (Hz)"=u32 2000) -> ()  [unwired: 9 in]
          }
          frame #1 {
            n1286 = call <vilib>:"Beep.vi"("use system alert? (T)"=FALSE, "duration (msec)"=u32 500, "frequency (Hz)"=u32 2000) -> ()  [unwired: 9 in]
          }
        }
        n1287 = call <vilib>:"Add State(s) to Queue__JKI_lib_State_Machine.vi"("State(s) in (\"\")"=w2782) -> ("States Out"=w2781:string)  [unwired: 14 in]
      }
      frame "Utility: RestoreDeConChan" {
        # "Template Separator\n(You can make a copy of, or modify, this frame)"
        n1288 = global read "GlobalVariables.vi" "DeconChan Temp"() -> (w2789:T9)
        n1289 = local write "Radio Buttons"(w2789) -> ()
        n1290 = call <vilib>:"Add State(s) to Queue__JKI_lib_State_Machine.vi"("State(s) in (\"\")"=w2794) -> ("States Out"=w2793:string)  [unwired: 14 in]
      }
      frame "Utility: SaveDeconChan" {
        # "Save Decon Channel to global temp\n(You can make a copy of, or modify, this frame)"
        n1291 = flat-sequence {
          frame #0 {
            n1292 = local read "Radio Buttons"() -> (w2800:T9)
            n1293 = global write "GlobalVariables.vi" "DeconChan Temp"(w2800) -> ()
          }
          frame #1 {
            n1294 = local write "Radio Buttons"(T9."No Selection" ("Radio Buttons")) -> ()
          }
        }
        n1295 = flat-sequence {
          frame #0 {
          }
          frame #1 {
            (unwired) enum32{"No Selection", "Ch1", "Ch2", "Ch3"}."No Selection" ("Radio Buttons")
          }
        }
        n1296 = call <vilib>:"Add State(s) to Queue__JKI_lib_State_Machine.vi"("State(s) in (\"\")"=w2799) -> ("States Out"=w2798:string)  [unwired: 14 in]
      }
      frame "Utility: Dewelling" {
        # "Main loop dewell\n(Dewelling >> #)"
        n1297 = Fract/Exp String To Number(string=w2805, default (0 dbl)=0) -> (number=w2803:i32)  [unwired: 2 in, 1 out]
        n1298 = Wait (ms)(milliseconds to wait=w2803) -> ()  [unwired: 1 out]
        n1299 = call <vilib>:"Add State(s) to Queue__JKI_lib_State_Machine.vi"("State(s) in (\"\")"=w2809) -> ("States Out"=w2808:string)  [unwired: 14 in]
      }
      frame "Utility: SetAllChanManualGain" {
        w2810 = FALSE ("Value (Signaling)")
        # "Set all channel to manual gain\n(You can make a copy of, or modify, this frame)"
        n1300 = property on="Auto gain ch1" class="Bool (strict)"("Val(Sgnl)"=w2810) -> ()  [unwired: 2 in, 2 out]
        n1301 = property on="Auto gain ch2" class="Bool (strict)"("Val(Sgnl)"=w2810) -> ()  [unwired: 2 in, 2 out]
        n1302 = property on="Auto gain ch3" class="Bool (strict)"("Val(Sgnl)"=w2810) -> ()  [unwired: 2 in, 2 out]
        n1303 = property on="Auto gain ch4" class="Bool (strict)"("Val(Sgnl)"=w2810) -> ()  [unwired: 2 in, 2 out]
        n1304 = call <vilib>:"Add State(s) to Queue__JKI_lib_State_Machine.vi"("State(s) in (\"\")"=w2815) -> ("States Out"=w2814:string)  [unwired: 14 in]
      }
      frame "Utility: SetAllChanAutoGain" {
        w2816 = TRUE ("Value (Signaling)")
        # "Set all channels to auto gain\n(You can make a copy of, or modify, this frame)"
        n1305 = property on="Auto gain ch1" class="Bool (strict)"("Val(Sgnl)"=w2816) -> ()  [unwired: 2 in, 2 out]
        n1306 = property on="Auto gain ch2" class="Bool (strict)"("Val(Sgnl)"=w2816) -> ()  [unwired: 2 in, 2 out]
        n1307 = property on="Auto gain ch3" class="Bool (strict)"("Val(Sgnl)"=w2816) -> ()  [unwired: 2 in, 2 out]
        n1308 = property on="Auto gain ch4" class="Bool (strict)"("Val(Sgnl)"=w2816) -> ()  [unwired: 2 in, 2 out]
        n1309 = call <vilib>:"Add State(s) to Queue__JKI_lib_State_Machine.vi"("State(s) in (\"\")"=w2821) -> ("States Out"=w2820:string)  [unwired: 14 in]
      }
      frame "---------- SysLog ----------" {
        # "Template Separator\n(You can make a copy of, or modify, this frame)"
        n1310 = call <vilib>:"Add State(s) to Queue__JKI_lib_State_Machine.vi"("State(s) in (\"\")"=w2826) -> ("States Out"=w2825:string)  [unwired: 14 in]
      }
      frame "SysLog: OpenLogFile" {
        # "Template Separator\n(You can make a copy of, or modify, this frame)"
        n1311 = call <vilib>:"Add State(s) to Queue__JKI_lib_State_Machine.vi"("State(s) in (\"\")"=w2831) -> ("States Out"=w2830:string)  [unwired: 14 in]
      }
      frame "---------- Graph ----------" {
        # "Template Separator\n(You can make a copy of, or modify, this frame)"
        n1312 = call <vilib>:"Add State(s) to Queue__JKI_lib_State_Machine.vi"("State(s) in (\"\")"=w2836) -> ("States Out"=w2835:string)  [unwired: 14 in]
      }
      frame "Graph: SetXMultiplier" {
        # "Set X multiplier of WF graphs\n(You can make a copy of, or modify, this frame)"
        n1313 = call "Digitizer1_FGV.vi"() -> ("error out"=w2840:errorcluster, "Read data"=w2841:refnum<k15>)  [unwired: 10 in]
        n1314 = property class="niScope"(reference=w2841, error in=w2840) -> ("Min Sample Rate"=w2839:dbl)  [unwired: 2 out]
        n1315 = Divide(x=1.0, y=w2839) -> (x/y=w2837:dbl)
        n1316 = property on="Channel 1" class="WFGraph (strict)"("XScale.Multiplier"=w2837) -> ()  [unwired: 2 in, 2 out]
        n1317 = property on="Channel 2" class="WFGraph (strict)"("XScale.Multiplier"=w2837) -> ()  [unwired: 2 in, 2 out]
        n1318 = property on="Channel 3" class="WFGraph (strict)"("XScale.Multiplier"=w2837) -> ()  [unwired: 2 in, 2 out]
        n1319 = property on="Channel 4" class="WFGraph (strict)"("XScale.Multiplier"=w2837) -> ()  [unwired: 2 in, 2 out]
        n1320 = call <vilib>:"Add State(s) to Queue__JKI_lib_State_Machine.vi"("State(s) in (\"\")"=w2846) -> ("States Out"=w2845:string)  [unwired: 14 in]
      }
      frame "Graph: AddCursors" {
        # "Add BG and DC cursor to all graphs\n(You can make a copy of, or modify, this frame)"
        n1321 = property on="Channel 1" class="WFGraph (strict)"() -> ("XScale.Multiplier"=w2855:dbl)  [unwired: 2 in, 2 out]
        n1322 = global read "GlobalVariables.vi" "DC Idx1"() -> (w2854:i32)
        n1323 = global read "GlobalVariables.vi" "DC Idx2"() -> (w2853:i32)
        n1324 = global read "GlobalVariables.vi" "BG Idx1"() -> (w2852:i32)
        n1325 = global read "GlobalVariables.vi" "BG Idx2"() -> (w2851:i32)
        n1326 = property on="Channel 1" class="WFGraph (strict)"(error in=w2857) -> ("CrsrList"=w2866:T24)  [unwired: 1 in, 2 out]
        n1327 = property on="Channel 2" class="WFGraph (strict)"() -> ("CrsrList"=w2863:T24)  [unwired: 2 in, 2 out]
        n1328 = property on="Channel 3" class="WFGraph (strict)"() -> ("CrsrList"=w2862:T24)  [unwired: 2 in, 2 out]
        n1329 = property on="Channel 4" class="WFGraph (strict)"() -> ("CrsrList"=w2848:T24)  [unwired: 2 in, 2 out]
        n1330 = Build Array(w2854, w2853, w2852, w2851) -> (w2850:i32[])
        n1331 = Multiply(x=w2850, y=w2855) -> (x*y=w2849:dbl[])
        n1332 = for {
          tunnel: w2866 -> [w2880] mode=indexing
          tunnel: w2849 -> [w2873] mode=indexing
          tunnel: [w2879] -> w2865 mode=indexing
          tunnel: u32[] [6618880, 6618880, 16711680, 16711680] -> [w2872] mode=indexing
          tunnel: w2863 -> [w2878] mode=indexing
          tunnel: w2862 -> [w2877] mode=indexing
          tunnel: [w2876] -> w2861 mode=indexing
          tunnel: [w2875] -> w2860 mode=indexing
          tunnel: w2848 -> [w2874] mode=indexing
          tunnel: [w2871] -> w2847 mode=indexing
          n1333 = Bundle By Name(cluster=w2880, "Position.X"=w2873, "Color"=w2872) -> (w2879:T25)
          n1334 = Bundle By Name(cluster=w2878, "Position.X"=w2873, "Color"=w2872) -> (w2876:T25)
          n1335 = Bundle By Name(cluster=w2877, "Position.X"=w2873, "Color"=w2872) -> (w2875:T25)
          n1336 = Bundle By Name(cluster=w2874, "Position.X"=w2873, "Color"=w2872) -> (w2871:T25)
        }
        n1337 = property on="Channel 1" class="WFGraph (strict)"("CrsrList"=w2865) -> (error out=w2856:errorcluster)  [unwired: 2 in, 1 out]
        n1338 = property on="Channel 2" class="WFGraph (strict)"("CrsrList"=w2861) -> ()  [unwired: 2 in, 2 out]
        n1339 = property on="Channel 3" class="WFGraph (strict)"("CrsrList"=w2860) -> ()  [unwired: 2 in, 2 out]
        n1340 = property on="Channel 4" class="WFGraph (strict)"("CrsrList"=w2847) -> ()  [unwired: 2 in, 2 out]
        n1341 = control-ref of="Channel 1"() -> (w2859:refnum<vi>)
        n1342 = call <vilib>:"Add State(s) to Queue__JKI_lib_State_Machine.vi"("State(s) in (\"\")"=w2870) -> ("States Out"=w2869:string)  [unwired: 14 in]
        n1343 = call "UpdateCurserIdx(SubVI).vi"("error in (no error)"=w2856, "WaveformGraph in"=w2859) -> ("error out"=w2858:errorcluster)  [unwired: 9 in]
      }
      frame "Graph: SaveCursorLoc" {
        # "Save cursor location to ini file\n(Save cursor location to system setting ini file)"
        n1344 = global read "GlobalVariables.vi" "DC Idx1"() -> (w2887:i32)
        n1345 = global read "GlobalVariables.vi" "DC Idx2"() -> (w2886:i32)
        n1346 = global read "GlobalVariables.vi" "BG Idx1"() -> (w2885:i32)
        n1347 = global read "GlobalVariables.vi" "BG Idx2"() -> (w2884:i32)
        n1348 = Bundle("DC Idx1"=w2887, "DC Idx2"=w2886, "BG Idx1"=w2885, "BG Idx2"=w2884) -> (w2883:T47)  [unwired: 1 in]
        n1349 = call "writeCursorConfigMain.vi"("error in (no error)"=w2881, "Cursor Locations"=w2883) -> ("error out"=w2882:errorcluster)  [unwired: 9 in]
        n1350 = call <vilib>:"Add State(s) to Queue__JKI_lib_State_Machine.vi"("State(s) in (\"\")"=w2891) -> ("States Out"=w2890:string)  [unwired: 14 in]
      }
      frame "---------- APD ----------" {
        # "Template Separator\n(You can make a copy of, or modify, this frame)"
        n1351 = call <vilib>:"Add State(s) to Queue__JKI_lib_State_Machine.vi"("State(s) in (\"\")"=w2896) -> ("States Out"=w2895:string)  [unwired: 14 in]
      }
      frame "APD: Initialize" {
        w2903 = enum16{"Read", "Write"}."Write" ("Operation (Read)")
        w2902 = refnum<class "APDClass.lvclass"> refnum  # APDClass.lvclass
        # "Initialize APD FGV\n(Initialized APD FGV for holding data)"
        n1352 = call "APD1FGV.vi"("Error In"=w2897, "Operation (Read)"=w2903, "APDClass in"=w2902) -> ("Error Out"=w2901:errorcluster)  [unwired: 7 in, 1 out]
        n1353 = call "APD2FGV.vi"("Error In"=w2897, "Operation (Read)"=w2903, "APDClass in"=w2902) -> ("Error Out"=w2900:errorcluster)  [unwired: 7 in, 1 out]
        n1354 = call "APD3FGV.vi"("Error In"=w2897, "Operation (Read)"=w2903, "APDClass in"=w2902) -> ("Error Out"=w2899:errorcluster)  [unwired: 7 in, 1 out]
        n1355 = Merge Errors(w2901, w2900, w2899) -> (w2898:errorcluster)
        n1356 = call <vilib>:"Add State(s) to Queue__JKI_lib_State_Machine.vi"("State(s) in (\"\")"=w2907) -> ("States Out"=w2906:string)  [unwired: 14 in]
      }
      frame "APD: LoadFromSerial" {
        w2909 = enum16{"Read", "Write"}."Write" ("Operation (Read)")
        # "Load APD data from tdms file\n(load and update FGV)"
        n1357 = call "readAPDSerial.vi"("Error In"=w2916) -> ("Error Out"=w2912:errorcluster, "output cluster"=w2915:T26)  [unwired: 9 in]
        n1358 = Unbundle By Name(w2915) -> ("Ch1APDSerial#"=w2928:string, "Ch2APDSerial#"=w2914:string, "Ch3APDSerial#"=w2927:string, "Ch4APDSerial#"=w2913:string)
        n1359 = call "CreatFromSerialNumNoRaw.vi"("error in (no error)"=w2912, "APD Serial #"=w2928) -> ("error out"=w2925:errorcluster, "APDClass out"=w2926:refnum<class "APDClass.lvclass">)  [unwired: 8 in]
        n1360 = call "CreatFromSerialNumNoRaw.vi"("error in (no error)"=w2912, "APD Serial #"=w2914) -> ("error out"=w2923:errorcluster, "APDClass out"=w2924:refnum<class "APDClass.lvclass">)  [unwired: 8 in]
        n1361 = call "CreatFromSerialNumNoRaw.vi"("error in (no error)"=w2912, "APD Serial #"=w2927) -> ("error out"=w2921:errorcluster, "APDClass out"=w2922:refnum<class "APDClass.lvclass">)  [unwired: 8 in]
        n1362 = call "CreatFromSerialNumNoRaw.vi"("error in (no error)"=w2912, "APD Serial #"=w2913) -> ("error out"=w2910:errorcluster, "APDClass out"=w2911:refnum<class "APDClass.lvclass">)  [unwired: 8 in]
        n1363 = call "APD1FGV.vi"("Error In"=w2925, "Operation (Read)"=w2909, "APDClass in"=w2926) -> ("Error Out"=w2920:errorcluster)  [unwired: 7 in, 1 out]
        n1364 = call "APD2FGV.vi"("Error In"=w2923, "Operation (Read)"=w2909, "APDClass in"=w2924) -> ("Error Out"=w2918:errorcluster)  [unwired: 7 in, 1 out]
        n1365 = call "APD3FGV.vi"("Error In"=w2921, "Operation (Read)"=w2909, "APDClass in"=w2922) -> ("Error Out"=w2919:errorcluster)  [unwired: 7 in, 1 out]
        n1366 = call "APD4FGV.vi"("Error In"=w2910, "Operation (Read)"=w2909, "APDClass in"=w2911) -> ("Error Out"=w2908:errorcluster)  [unwired: 7 in, 1 out]
        n1367 = Merge Errors(w2920, w2918, w2919, w2908) -> (w2917:errorcluster)
        n1368 = call <vilib>:"Add State(s) to Queue__JKI_lib_State_Machine.vi"("State(s) in (\"\")"=w2932) -> ("States Out"=w2931:string)  [unwired: 14 in]
      }
      frame "APD: UpdateCtrlVLimit" {
        w2938 = enum16{"Read", "Write"}."Read" ("Operation (Read)")
        # "Set V limit\n(You can make a copy of, or modify, this frame)"
        n1369 = call "APD1FGV.vi"("Error In"=w2939, "Operation (Read)"=w2938) -> ("Error Out"=w2954:errorcluster, "APDClass out"=w2955:refnum<class "APDClass.lvclass">)  [unwired: 8 in]
        n1370 = call "APD2FGV.vi"("Error In"=w2939, "Operation (Read)"=w2938) -> ("Error Out"=w2952:errorcluster, "APDClass out"=w2953:refnum<class "APDClass.lvclass">)  [unwired: 8 in]
        n1371 = call "APD3FGV.vi"("Error In"=w2939, "Operation (Read)"=w2938) -> ("Error Out"=w2950:errorcluster, "APDClass out"=w2951:refnum<class "APDClass.lvclass">)  [unwired: 8 in]
        n1372 = call "APD4FGV.vi"("Error In"=w2939, "Operation (Read)"=w2938) -> ("Error Out"=w2936:errorcluster, "APDClass out"=w2937:refnum<class "APDClass.lvclass">)  [unwired: 8 in]
        n1373 = call-dynamic "ReadMaxCtrlV.vi"("error in (no error)"=w2954, "APDClass in"=w2955) -> ("error out"=w2945:errorcluster, "Numeric"=w2948:dbl)  [unwired: 7 in, 1 out]
        n1374 = call-dynamic "ReadMaxCtrlV.vi"("error in (no error)"=w2952, "APDClass in"=w2953) -> ("error out"=w2943:errorcluster, "Numeric"=w2947:dbl)  [unwired: 7 in, 1 out]
        n1375 = call-dynamic "ReadMaxCtrlV.vi"("error in (no error)"=w2950, "APDClass in"=w2951) -> ("error out"=w2941:errorcluster, "Numeric"=w2946:dbl)  [unwired: 7 in, 1 out]
        n1376 = call-dynamic "ReadMaxCtrlV.vi"("error in (no error)"=w2936, "APDClass in"=w2937) -> ("error out"=w2934:errorcluster, "Numeric"=w2935:dbl)  [unwired: 7 in, 1 out]
        n1377 = property on="V 1" class="DigNum (strict)"(error in=w2945, "Maximum"=w2948) -> (error out=w2944:errorcluster)  [unwired: 1 in, 1 out]
        n1378 = property on="V 2" class="DigNum (strict)"(error in=w2943, "Maximum"=w2947) -> (error out=w2942:errorcluster)  [unwired: 1 in, 1 out]
        n1379 = property on="V 4" class="DigNum (strict)"(error in=w2934, "Maximum"=w2935) -> (error out=w2933:errorcluster)  [unwired: 1 in, 1 out]
        n1380 = property on="V 3" class="DigNum (strict)"(error in=w2941, "Maximum"=w2946) -> (error out=w2940:errorcluster)  [unwired: 1 in, 1 out]
        n1381 = Merge Errors(w2944, w2942, w2940, w2933) -> (w2949:errorcluster)
        n1382 = call <vilib>:"Add State(s) to Queue__JKI_lib_State_Machine.vi"("State(s) in (\"\")"=w2959) -> ("States Out"=w2958:string)  [unwired: 14 in]
      }
      frame "APD: GetGainLimits" {
        w2964 = enum16{"Read", "Write"}."Read" ("Operation (Read)")
        # "Template Separator\n(You can make a copy of, or modify, this frame)"
        n1383 = call "APD1FGV.vi"("Error In"=w2965, "Operation (Read)"=w2964) -> ("Error Out"=w2970:errorcluster, "APDClass out"=w2971:refnum<class "APDClass.lvclass">)  [unwired: 8 in]
        n1384 = call "APD2FGV.vi"("Error In"=w2965, "Operation (Read)"=w2964) -> ("Error Out"=w2977:errorcluster, "APDClass out"=w2978:refnum<class "APDClass.lvclass">)  [unwired: 8 in]
        n1385 = call "APD3FGV.vi"("Error In"=w2965, "Operation (Read)"=w2964) -> ("Error Out"=w2975:errorcluster, "APDClass out"=w2976:refnum<class "APDClass.lvclass">)  [unwired: 8 in]
        n1386 = call "APD4FGV.vi"("Error In"=w2965, "Operation (Read)"=w2964) -> ("Error Out"=w2962:errorcluster, "APDClass out"=w2963:refnum<class "APDClass.lvclass">)  [unwired: 8 in]
        n1387 = call-dynamic "Read Gain Limits(Log).vi"("error in (no error)"=w2970, "APDClass in"=w2971) -> ("error out"=w2969:errorcluster, "GainLimits(Log)"=w2966:cluster{"GainMax":dbl, "GainMin":dbl})  [unwired: 7 in, 1 out]
        n1388 = call-dynamic "Read Gain Limits(Log).vi"("error in (no error)"=w2977, "APDClass in"=w2978) -> ("error out"=w2973:errorcluster, "GainLimits(Log)"=w2968:cluster{"GainMax":dbl, "GainMin":dbl})  [unwired: 7 in, 1 out]
        n1389 = call-dynamic "Read Gain Limits(Log).vi"("error in (no error)"=w2975, "APDClass in"=w2976) -> ("error out"=w2972:errorcluster, "GainLimits(Log)"=w2967:cluster{"GainMax":dbl, "GainMin":dbl})  [unwired: 7 in, 1 out]
        n1390 = call-dynamic "Read Gain Limits(Log).vi"("error in (no error)"=w2962, "APDClass in"=w2963) -> ("error out"=w2960:errorcluster, "GainLimits(Log)"=w2961:cluster{"GainMax":dbl, "GainMin":dbl})  [unwired: 7 in, 1 out]
        n1391 = Merge Errors(w2969, w2973, w2972, w2960) -> (w2974:errorcluster)
        n1392 = global write "GlobalVariables.vi" "Ch1GainLim(Log)"(w2966) -> ()
        n1393 = global write "GlobalVariables.vi" "Ch2GainLim(Log)"(w2968) -> ()
        n1394 = global write "GlobalVariables.vi" "Ch3GainLim(Log)"(w2967) -> ()
        n1395 = global write "GlobalVariables.vi" "Ch4GainLim(Log)"(w2961) -> ()
        n1396 = call <vilib>:"Add State(s) to Queue__JKI_lib_State_Machine.vi"("State(s) in (\"\")"=w2982) -> ("States Out"=w2981:string)  [unwired: 14 in]
      }
      frame "---------- TCP ----------" {
        # "Template Separator\n(You can make a copy of, or modify, this frame)"
        n1397 = call <vilib>:"Add State(s) to Queue__JKI_lib_State_Machine.vi"("State(s) in (\"\")"=w2987) -> ("States Out"=w2986:string)  [unwired: 14 in]
      }
      frame "TCP: InitializeNew" {
        # "if unsuccessful and count <10, increament count \nand try again"
        # "Initialize TCP connection to aimging beam computer\n(You can make a copy of, or modify, this frame)"
        n1398 = TCP Create Listener(10:u16 2100 ("port"), 11:"RTLT" ("service name")) -> (0:w2996:errorcluster, 3:w2988:refnum<k5>)  [unwired: 3 in, 1 out]
        n1399 = while {
          tunnel: w2988 -> [w3016]
          tunnel: w2996 -> [w3015]
          tunnel: [w3006] -> w2994
          tunnel: [w3003] -> w2990
          i -> [w3012]
          stop <- w3003 stop-if-true
          n1400 = TCP Wait On Listener(8:w3015, 9:200 ("timeout ms (wait forever: -1)"), 11:w3016) -> (0:w3013:errorcluster, 4:w3010:refnum<k5>)  [unwired: 1 in, 3 out]
          n1401 = Less Or Equal?(x=50, y=w3012) -> (x <= y?=w3009:bool)
          n1402 = case shown="No Error" w3013 {
            selector: w3013 -> [w3026 w3036]
            tunnel: w3010 -> [w3027 _]
            tunnel: [errorcluster {"status"=TRUE, "code"=0, "source"=""} ("No error") w3037] -> w3005
            tunnel: [w3018 FALSE ("TCP connected?")] -> w3006
            frame No Error {
              # "connection is ready, read data"
              n1403 = TCP Read(connection ID=w3027, bytes to read=512, error in (no error)=w3026, 7:T21."CRLF" ("mode (standard)"), 9:5000 ("timeout ms (25000)")) -> (connection ID out=w3020:refnum<k5>, data out=w3022:string, error out=w3019:errorcluster)
              n1404 = Concatenate Strings("alive" ("string"), "\r\n" ("End of Line Constant")) -> (w3023:string)
              n1405 = Equal?(x=w3023, y=w3022) -> (x = y?=w3021:bool)
              n1406 = case shown="False" w3021 {
                tunnel: w3020 -> [_ w3032]
                tunnel: w3019 -> [_ _]
                tunnel: [FALSE ("TCP connected?") TRUE ("TCP connected?")] -> w3018
                frame False {
                }
                frame True {
                  n1407 = call "TcpIDFGV.vi"("action"=enum16{"write", "read"}."write", "connection ID in"=w3032) -> ()  [unwired: 8 in, 2 out]
                }
              }
            }
            frame Error {
              # "connection not ready, keep waiting"
              n1408 = Unbundle By Name(w3036) -> ("code"=w3038:i32)
              n1409 = case shown="56" w3038 {
                tunnel: w3036 -> [w3039 _]
                tunnel: [w3039 w3040] -> w3037
                frame Default {
                }
                frame 56 {
                  w3040 = errorcluster {"status"=FALSE, "code"=0, "source"=""}  # No error
                }
              }
            }
          }
          n1410 = Select(t=errorcluster {"status"=TRUE, "code"=5001, "source"=""} ("error in (no error)"), s=w3009, f=errorcluster {"status"=FALSE, "code"=0, "source"=""} ("error in (no error)")) -> (s? t:f=w3004:errorcluster)
          n1411 = Merge Errors(w3005, w3004) -> (w3003:errorcluster)
        }
        n1412 = Unbundle By Name(w2990) -> ("code"=w2993:i32)
        n1413 = Bundle By Name(cluster=w2995, "System Status.TCP/IP"=w2994, "listener ID"=w2988) -> (w3000:T23)
        n1414 = global write "GlobalVariables.vi" "TCP connected?"(w2994) -> ()
        n1415 = Equal To 0?(x=w2993) -> (x = 0?=w2992:bool)
        n1416 = Select(t=errorcluster {"status"=FALSE, "code"=0, "source"=""} ("error in (no error)"), s=w2992, f=w2990) -> (s? t:f=w2989:errorcluster)
        n1417 = call <vilib>:"Add State(s) to Queue__JKI_lib_State_Machine.vi"("State(s) in (\"\")"=w3002) -> ("States Out"=w3001:string)  [unwired: 14 in]
      }
      frame "TCP: checkSource" {
        # "Check visualization PC video source\n(send !video_source message, listen for response, then parse it to binary mask)"
        n1418 = Unbundle By Name(w3047) -> ("System Status.TCP/IP"=w3050:bool)
        n1419 = case shown="True" w3050 {
          tunnel: w3049 -> [w3055 w3078]
          tunnel: [w3055 w3062] -> w3048
          tunnel: [w3054 w3067] -> w3045
          tunnel: [w3054 w3065] -> w3044
          tunnel: [w3054 w3066] -> w3043
          tunnel: [w3054 w3064] -> w3042
          tunnel: [w3054 w3056] -> w3041
          frame False {
            w3054 = FALSE
          }
          frame True {
            n1420 = call "TcpIDFGV.vi"("Error In"=w3078, "action"=enum16{"write", "read"}."read") -> ("Error Out"=w3075:errorcluster, "connection ID out"=w3077:refnum<k5>)  [unwired: 8 in]
            n1421 = call "TCP_WriteRead.vi"("error in (no error)"=w3075, "data in"="!video_source", "connectin ID in"=w3077) -> ("error out"=w3072:errorcluster, "data out"=w3074:string)  [unwired: 4 in, 1 out]
            n1422 = Scan From String(format string="!video_source:%d", input string=w3074, error in=w3072) -> (error out=w3063:errorcluster, output 1=w3061:i32)  [unwired: 2 in, 2 out]
            n1423 = case shown="5..7, 9..11, 13..15" w3061 {
              tunnel: w3063 -> [_ _ _ _]
              tunnel: [errorcluster {"status"=TRUE, "code"=5007, "source"="Visualization PC"} ("error out") errorcluster {"status"=FALSE, "code"=0, "source"=""} ("error out") errorcluster {"status"=FALSE, "code"=0, "source"=""} ("error out") errorcluster {"status"=FALSE, "code"=0, "source"=""} ("error out")] -> w3062
              tunnel: [FALSE FALSE FALSE TRUE] -> w3056
              frame 0, Default {
                # "No video source available or default"
                n1424 = property on="Video Source" class="RadioBtnsControl (strict)"("DisabledEnum"=T11."Disabled and Grayed Out" ("Disabled")) -> ()  [unwired: 2 in, 2 out]
              }
              frame 1..3 {
                # "one or both camera available"
                n1425 = local write "Video Source"(enum32{"Camera", "FrameGrabber"}."Camera" ("Video Source")) -> ()
                n1426 = property on="Video Source" class="RadioBtnsControl (strict)"("DisabledEnum"=T11."Disabled and Grayed Out" ("Disabled")) -> ()  [unwired: 2 in, 2 out]
              }
              frame 4, 8, 12 {
                # "one or both frame grabber available"
                n1427 = local write "Video Source"(enum32{"Camera", "FrameGrabber"}."FrameGrabber" ("Video Source")) -> ()
                n1428 = property on="Video Source" class="RadioBtnsControl (strict)"("DisabledEnum"=T11."Disabled and Grayed Out" ("Disabled")) -> ()  [unwired: 2 in, 2 out]
              }
              frame 5..7, 9..11, 13..15 {
                n1429 = property on="Video Source" class="RadioBtnsControl (strict)"("DisabledEnum"=T11."Enabled" ("Disabled")) -> ()  [unwired: 2 in, 2 out]
              }
            }
            n1430 = Integer to Fixed-Point Cast(fixed-point type=fxp<+,4,4> 0.0, integer=w3061) -> (fixed-point=w3060:fxp<+,4,4>)
            n1431 = Number To Boolean Array(number=w3060) -> (Boolean array=w3058:bool[])
            n1432 = Reverse 1D Array(array=w3058) -> (reversed array=w3057:bool[])
            n1433 = Index Array(array=w3057, index=0) -> (element=w3067:bool)
            n1434 = Index Array(array=w3057, index=1) -> (element=w3065:bool)
            n1435 = Index Array(array=w3057, index=2) -> (element=w3066:bool)
            n1436 = Index Array(array=w3057, index=3) -> (element=w3064:bool)
          }
        }
        n1437 = Bundle By Name(cluster=w3047, "video source.Main Frame Grabber"=w3045, "video source.Side Frame Grabber"=w3044, "video source.Main Camera"=w3043, "video source.Side Camera"=w3042, "bothVidSourceAvail"=w3041) -> (w3046:T23)
        n1438 = call <vilib>:"Add State(s) to Queue__JKI_lib_State_Machine.vi"("State(s) in (\"\")"=w3053) -> ("States Out"=w3052:string)  [unwired: 14 in]
      }
      frame "TCP: SyncTime" {
        # "Template Separator\n(You can make a copy of, or modify, this frame)"
        n1439 = Unbundle By Name(w3095) -> ("System Status.TCP/IP"=w3094:bool)
        n1440 = case shown="True" w3094 {
          tunnel: w3096 -> [_ w3104]
          frame False {
          }
          frame True {
            n1441 = call "TcpIDFGV.vi"("Error In"=w3104, "action"=enum16{"write", "read"}."read") -> ("Error Out"=w3103:errorcluster, "connection ID out"=w3100:refnum<k5>)  [unwired: 8 in]
            n1442 = call <userlib>:"Tick Count (ms)__ogtk.vi"("error in (no error)"=w3103) -> ("error out"=w3102:errorcluster, "millisecond timer value"=w3101:u32)  [unwired: 9 in]
            n1443 = while {
              tunnel: w3102 -> [w3124]
              tunnel: w3100 -> [w3123]
              tunnel: w3101 -> [w3112]
              stop <- w3107 stop-if-true
              n1444 = Concatenate Strings("latencycheck" ("string"), "\r\n" ("End of Line Constant")) -> (w3119:string)
              n1445 = TCP Read(connection ID=w3123, bytes to read=512, error in (no error)=w3124, 7:T21."CRLF" ("mode (standard)"), 9:2000 ("timeout ms (25000)")) -> (connection ID out=w3116:refnum<k5>, data out=w3114:string, error out=w3106:errorcluster)
              n1446 = Tick Count (ms)() -> (millisecond timer value=w3113:u32)
              n1447 = Subtract(x=w3113, y=w3112) -> (x-y=w3111:u32)
              n1448 = Equal?(x=w3114, y=w3119) -> (x = y?=w3115:bool)
              n1449 = case shown="False" w3115 {
                tunnel: w3116 -> [_ w3137]
                tunnel: w3114 -> [w3129 _]
                tunnel: [w3125 FALSE] -> w3109
                tunnel: w3106 -> [_ w3131]
                frame False {
                  n1450 = Concatenate Strings("synctimer" ("string"), "\r\n" ("End of Line Constant")) -> (w3126:string)
                  n1451 = Equal?(x=w3129, y=w3126) -> (x = y?=w3125:bool)
                  "Sync Success?" <- w3125
                }
                frame True {
                  n1452 = Concatenate Strings("latencycheck:" ("string"), "\r\n" ("End of Line Constant")) -> (w3136:string)
                  n1453 = TCP Write(connection ID=w3137, data in=w3136, error in (no error)=w3131, 9:1000 ("timeout ms (25000)")) -> (error out=w3130:errorcluster)  [unwired: 2 out]
                  n1454 = call <vilib>:"Clear Errors.vi"("error in (no error)"=w3130) -> ()  [unwired: 5 in, 2 out]
                }
              }
              n1455 = Greater?(x=w3111, y=u32 10000 ("x-y")) -> (0:w3108:bool)
              n1456 = Or(x=w3109, y=w3108) -> (x .or. y?=w3107:bool)
            }
          }
        }
        n1457 = call <vilib>:"Add State(s) to Queue__JKI_lib_State_Machine.vi"("State(s) in (\"\")"=w3099) -> ("States Out"=w3098:string)  [unwired: 14 in]
      }
      frame "TCP: SendSettingMacro" {
        # "Template Separator\n(You can make a copy of, or modify, this frame)"
        n1458 = Unbundle By Name(w3141) -> ("System Status.TCP/IP"=w3140:bool)
        n1459 = case shown="True" w3140 {
          tunnel: ["" ("Empty String Constant") "TCP: sendSubjectID\nTCP: sendScaleBarSetting\nTCP: sendScaleMaxMin\nTCP: sendDeconChannel\nTCP: sendANSI\nTCP: sendRadius\nTCP: send3Dsetting\nTCP: sendFirefly\nTCP: sendPentero"] -> w3139
          frame False {
          }
          frame True {
          }
        }
        n1460 = call <vilib>:"Add State(s) to Queue__JKI_lib_State_Machine.vi"("State(s) in Front (\"\")"=w3139, "State(s) in (\"\")"=w3144) -> ("States Out"=w3143:string)  [unwired: 13 in]
      }
      frame "TCP: sendRunNum" {
        # "Send run number to AB PC\n(You can make a copy of, or modify, this frame)"
        n1461 = Unbundle By Name(w3151) -> ("System Status.TCP/IP"=w3148:bool, "IDs.RunID"=w3152:i8)
        n1462 = Increment(x=w3152) -> (x+1=w3147:i8)
        n1463 = case shown="True" w3148 {
          tunnel: w3147 -> [_ w3166]
          tunnel: [w3156 w3158] -> w3150
          tunnel: w3149 -> [w3156 w3157]
          frame False {
          }
          frame True {
            n1464 = Number To Decimal String(number=w3166, width (-)=i16 3) -> (decimal integer string=w3161:string)
            n1465 = call "TcpIDFGV.vi"("Error In"=w3157, "action"=enum16{"write", "read"}."read") -> ("Error Out"=w3159:errorcluster, "connection ID out"=w3163:refnum<k5>)  [unwired: 8 in]
            n1466 = Concatenate Strings("!run:", w3161) -> (w3160:string)
            n1467 = call "TCP_WriteRead.vi"("error in (no error)"=w3159, "data in"=w3160, "connectin ID in"=w3163) -> ("error out"=w3158:errorcluster)  [unwired: 4 in, 2 out]
          }
        }
        n1468 = call <vilib>:"Add State(s) to Queue__JKI_lib_State_Machine.vi"("State(s) in (\"\")"=w3155) -> ("States Out"=w3154:string)  [unwired: 14 in]
      }
      frame "TCP: sendVideoSource" {
        # "Send video source \n(You can make a copy of, or modify, this frame)"
        n1469 = Unbundle By Name(w3168) -> ("System Status.TCP/IP"=w3167:bool)
        n1470 = case shown="True" w3167 {
          tunnel: [w3174 w3176] -> w3170
          tunnel: w3169 -> [w3174 w3175]
          frame False {
          }
          frame True {
            n1471 = case shown="\"Camera\", Default" "Video Source" {
              tunnel: [0 1] -> w3181
              frame "Camera", Default {
              }
              frame "FrameGrabber" {
              }
            }
            n1472 = call "TcpIDFGV.vi"("Error In"=w3175, "action"=enum16{"write", "read"}."read") -> ("Error Out"=w3177:errorcluster, "connection ID out"=w3183:refnum<k5>)  [unwired: 8 in]
            n1473 = Number To Decimal String(number=w3181) -> (decimal integer string=w3179:string)  [unwired: 1 in]
            n1474 = Concatenate Strings("!invivo:" ("data in"), w3179) -> (w3178:string)
            n1475 = call "TCP_WriteRead.vi"("error in (no error)"=w3177, "data in"=w3178, "connectin ID in"=w3183) -> ("error out"=w3176:errorcluster)  [unwired: 4 in, 2 out]
          }
        }
        n1476 = call <vilib>:"Add State(s) to Queue__JKI_lib_State_Machine.vi"("State(s) in (\"\")"=w3173) -> ("States Out"=w3172:string)  [unwired: 14 in]
      }
      frame "TCP: startRun" {
        # "Template Separator\n(You can make a copy of, or modify, this frame)"
        n1477 = Unbundle By Name(w3188) -> ("System Status.TCP/IP"=w3187:bool)
        n1478 = case shown="True" w3187 {
          tunnel: [w3194 w3196] -> w3190
          tunnel: w3189 -> [w3194 w3195]
          frame False {
          }
          frame True {
            n1479 = call "TcpIDFGV.vi"("Error In"=w3195, "action"=enum16{"write", "read"}."read") -> ("Error Out"=w3197:errorcluster, "connection ID out"=w3198:refnum<k5>)  [unwired: 8 in]
            n1480 = call "TCP_WriteRead.vi"("error in (no error)"=w3197, "data in"="!acquire:1", "connectin ID in"=w3198) -> ("error out"=w3196:errorcluster)  [unwired: 4 in, 2 out]
          }
        }
        n1481 = call <vilib>:"Add State(s) to Queue__JKI_lib_State_Machine.vi"("State(s) in (\"\")"=w3193) -> ("States Out"=w3192:string)  [unwired: 14 in]
      }
      frame "TCP: stopRun" {
        # "Send stop run to AB PC\n(You can make a copy of, or modify, this frame)"
        n1482 = Unbundle By Name(w3202) -> ("System Status.TCP/IP"=w3201:bool)
        n1483 = case shown="True" w3201 {
          tunnel: [w3208 w3210] -> w3204
          tunnel: w3203 -> [w3208 w3209]
          frame False {
            # "if not connected, do nothing"
          }
          frame True {
            # "If TCP connected, send stop run"
            n1484 = call "TcpIDFGV.vi"("Error In"=w3209, "action"=enum16{"write", "read"}."read") -> ("Error Out"=w3211:errorcluster, "connection ID out"=w3213:refnum<k5>)  [unwired: 8 in]
            n1485 = call "TCP_WriteRead.vi"("error in (no error)"=w3211, "data in"="!acquire:0", "connectin ID in"=w3213) -> ("error out"=w3210:errorcluster)  [unwired: 4 in, 2 out]
          }
        }
        n1486 = call <vilib>:"Add State(s) to Queue__JKI_lib_State_Machine.vi"("State(s) in (\"\")"=w3207) -> ("States Out"=w3206:string)  [unwired: 14 in]
      }
      frame "TCP: CheckConnection" {
        # "Check TCP/IP connection statuse\n(If connection is lost, throw error)"
        n1487 = Unbundle By Name(w3216) -> ("System Status.TCP/IP"=w3215:bool)
        n1488 = case shown="False" w3215 {
          frame False {
          }
          frame True {
            # "If TCP/IP is true check, otherwise skip"
          }
        }
        n1489 = call <vilib>:"Add State(s) to Queue__JKI_lib_State_Machine.vi"("State(s) in (\"\")"=w3220) -> ("States Out"=w3219:string)  [unwired: 14 in]
      }
      frame "TCP: sendSubjectID" {
        # "Send subject ID"
        n1490 = Unbundle By Name(w3222) -> ("System Status.TCP/IP"=w3221:bool, "CaseID"=w3225:string)
        n1491 = case shown="True" w3221 {
          tunnel: w3225 -> [_ w3236]
          tunnel: [w3229 w3231] -> w3224
          tunnel: w3223 -> [w3229 w3230]
          frame False {
          }
          frame True {
            n1492 = call "TcpIDFGV.vi"("Error In"=w3230, "action"=enum16{"write", "read"}."read") -> ("Error Out"=w3232:errorcluster, "connection ID out"=w3234:refnum<k5>)  [unwired: 8 in]
            n1493 = Concatenate Strings("!subject:", w3236) -> (w3233:string)
            n1494 = call "TCP_WriteRead.vi"("error in (no error)"=w3232, "data in"=w3233, "connectin ID in"=w3234) -> ("error out"=w3231:errorcluster)  [unwired: 4 in, 2 out]
          }
        }
        n1495 = call <vilib>:"Add State(s) to Queue__JKI_lib_State_Machine.vi"("State(s) in (\"\")"=w3228) -> ("States Out"=w3227:string)  [unwired: 14 in]
      }
      frame "TCP: sendScaleBarSetting" {
        # "Template Separator\n(You can make a copy of, or modify, this frame)"
        n1496 = Unbundle By Name(w3240) -> ("System Status.TCP/IP"=w3238:bool, "VideoConfig.Scale Bar"=w3239:bool)
        n1497 = case shown="True" w3238 {
          tunnel: [w3246 w3255] -> w3242
          tunnel: w3241 -> [w3246 w3254]
          tunnel: w3239 -> [_ w3253]
          frame False {
          }
          frame True {
            n1498 = Boolean To (0,1)(Boolean=w3253) -> (0, 1=w3252:i16)
            n1499 = call "TcpIDFGV.vi"("Error In"=w3254, "action"=enum16{"write", "read"}."read") -> ("Error Out"=w3256:errorcluster, "connection ID out"=w3257:refnum<k5>)  [unwired: 8 in]
            n1500 = Number To Fractional String(number=w3252, width (-)=i16 1, precision (6)=i16 0) -> (F-format string=w3250:string)  [unwired: 1 in]
            n1501 = Concatenate Strings("!autocolor:" ("data in"), w3250) -> (w3248:string)
            n1502 = call "TCP_WriteRead.vi"("error in (no error)"=w3256, "data in"=w3248, "connectin ID in"=w3257) -> ("error out"=w3255:errorcluster)  [unwired: 4 in, 2 out]
          }
        }
        n1503 = call <vilib>:"Add State(s) to Queue__JKI_lib_State_Machine.vi"("State(s) in (\"\")"=w3245) -> ("States Out"=w3244:string)  [unwired: 14 in]
      }
      frame "TCP: sendScaleMaxMin" {
        # "Send scale bar max and min to AB PC\n(You can make a copy of, or modify, this frame)"
        n1504 = Unbundle By Name(w3262) -> ("System Status.TCP/IP"=w3259:bool, "VideoConfig.Scale Low"=w3261:dbl, "VideoConfig.Scale High"=w3260:dbl)
        n1505 = case shown="True" w3259 {
          tunnel: [w3268 w3281] -> w3264
          tunnel: w3263 -> [w3268 w3280]
          tunnel: w3261 -> [_ w3279]
          tunnel: w3260 -> [_ w3270]
          frame False {
          }
          frame True {
            n1506 = call "TcpIDFGV.vi"("Error In"=w3280, "action"=enum16{"write", "read"}."read") -> ("Error Out"=w3282:errorcluster, "connection ID out"=w3283:refnum<k5>)  [unwired: 8 in]
            n1507 = Number To Fractional String(number=w3279, width (-)=i16 4, precision (6)=i16 2) -> (F-format string=w3275:string)  [unwired: 1 in]
            n1508 = Number To Fractional String(number=w3270, width (-)=i16 4, precision (6)=i16 2) -> (F-format string=w3271:string)  [unwired: 1 in]
            n1509 = Concatenate Strings("!color:" ("string"), w3275, ";" ("string"), w3271) -> (w3269:string)
            n1510 = call "TCP_WriteRead.vi"("error in (no error)"=w3282, "data in"=w3269, "connectin ID in"=w3283) -> ("error out"=w3281:errorcluster)  [unwired: 4 in, 2 out]
          }
        }
        n1511 = call <vilib>:"Add State(s) to Queue__JKI_lib_State_Machine.vi"("State(s) in (\"\")"=w3267) -> ("States Out"=w3266:string)  [unwired: 14 in]
      }
      frame "TCP: sendDeconChannel" {
        # "Send Decon channel\n(You can make a copy of, or modify, this frame)"
        n1512 = Unbundle By Name(w3286) -> ("System Status.TCP/IP"=w3285:bool)
        n1513 = case shown="True" w3285 {
          tunnel: [w3292 w3297] -> w3288
          tunnel: w3287 -> [w3292 w3296]
          frame False {
          }
          frame True {
            n1514 = local read "Radio Buttons"() -> (w3295:T9)
            n1515 = Increment(x=w3295) -> (x+1=w3294:T9)
            n1516 = Number To Decimal String(number=w3294) -> (decimal integer string=w3293:string)  [unwired: 1 in]
            n1517 = call "TcpIDFGV.vi"("Error In"=w3296, "action"=enum16{"write", "read"}."read") -> ("Error Out"=w3298:errorcluster, "connection ID out"=w3301:refnum<k5>)  [unwired: 8 in]
            n1518 = Concatenate Strings("!channel:", w3293) -> (w3299:string)
            n1519 = call "TCP_WriteRead.vi"("error in (no error)"=w3298, "data in"=w3299, "connectin ID in"=w3301) -> ("error out"=w3297:errorcluster)  [unwired: 4 in, 2 out]
          }
        }
        n1520 = call <vilib>:"Add State(s) to Queue__JKI_lib_State_Machine.vi"("State(s) in (\"\")"=w3291) -> ("States Out"=w3290:string)  [unwired: 14 in]
      }
      frame "TCP: sendANSI" {
        # "Template Separator\n(You can make a copy of, or modify, this frame)"
        n1521 = Unbundle By Name(w3305) -> ("System Status.TCP/IP"=w3303:bool, "VideoConfig.ANSI"=w3304:dbl)
        n1522 = case shown="True" w3303 {
          tunnel: [w3311 w3317] -> w3307
          tunnel: w3306 -> [w3311 w3316]
          tunnel: w3304 -> [_ w3315]
          frame False {
          }
          frame True {
            n1523 = Number To Fractional String(number=w3315) -> (F-format string=w3313:string)  [unwired: 3 in]
            n1524 = call "TcpIDFGV.vi"("Error In"=w3316, "action"=enum16{"write", "read"}."read") -> ("Error Out"=w3318:errorcluster, "connection ID out"=w3319:refnum<k5>)  [unwired: 8 in]
            n1525 = Concatenate Strings("!ansi:" ("data in"), w3313) -> (w3312:string)
            n1526 = call "TCP_WriteRead.vi"("error in (no error)"=w3318, "data in"=w3312, "connectin ID in"=w3319) -> ("error out"=w3317:errorcluster)  [unwired: 4 in, 2 out]
          }
        }
        n1527 = call <vilib>:"Add State(s) to Queue__JKI_lib_State_Machine.vi"("State(s) in (\"\")"=w3310) -> ("States Out"=w3309:string)  [unwired: 14 in]
      }
      frame "TCP: sendRadius" {
        # "Send drawing radius to AB PC\n(You can make a copy of, or modify, this frame)"
        n1528 = Unbundle By Name(w3323) -> ("System Status.TCP/IP"=w3321:bool, "VideoConfig.Radius"=w3322:dbl)
        n1529 = case shown="True" w3321 {
          tunnel: [w3329 w3335] -> w3325
          tunnel: w3324 -> [w3329 w3334]
          tunnel: w3322 -> [_ w3333]
          frame False {
          }
          frame True {
            n1530 = Number To Fractional String(number=w3333) -> (F-format string=w3332:string)  [unwired: 3 in]
            n1531 = Concatenate Strings("!radius:" ("data in"), w3332) -> (w3330:string)
            n1532 = call "TcpIDFGV.vi"("Error In"=w3334, "action"=enum16{"write", "read"}."read") -> ("Error Out"=w3336:errorcluster, "connection ID out"=w3337:refnum<k5>)  [unwired: 8 in]
            n1533 = call "TCP_WriteRead.vi"("error in (no error)"=w3336, "data in"=w3330, "connectin ID in"=w3337) -> ("error out"=w3335:errorcluster)  [unwired: 4 in, 2 out]
          }
        }
        n1534 = call <vilib>:"Add State(s) to Queue__JKI_lib_State_Machine.vi"("State(s) in (\"\")"=w3328) -> ("States Out"=w3327:string)  [unwired: 14 in]
      }
      frame "TCP: send3Dsetting" {
        # "Send 3D setting to AB computer\n(You can make a copy of, or modify, this frame)"
        n1535 = Unbundle By Name(w3341) -> ("System Status.TCP/IP"=w3339:bool, "VideoConfig.3D?"=w3340:bool)
        n1536 = case shown="True" w3339 {
          tunnel: [w3347 w3354] -> w3343
          tunnel: w3342 -> [w3347 w3353]
          tunnel: w3340 -> [_ w3352]
          frame False {
          }
          frame True {
            n1537 = Boolean To (0,1)(Boolean=w3352) -> (0, 1=w3351:i16)
            n1538 = Number To Fractional String(number=w3351) -> (F-format string=w3350:string)  [unwired: 3 in]
            n1539 = call "TcpIDFGV.vi"("Error In"=w3353, "action"=enum16{"write", "read"}."read") -> ("Error Out"=w3355:errorcluster, "connection ID out"=w3356:refnum<k5>)  [unwired: 8 in]
            n1540 = Concatenate Strings("!3dset:" ("data in"), w3350) -> (w3348:string)
            n1541 = call "TCP_WriteRead.vi"("error in (no error)"=w3355, "data in"=w3348, "connectin ID in"=w3356) -> ("error out"=w3354:errorcluster)  [unwired: 4 in, 2 out]
          }
        }
        n1542 = call <vilib>:"Add State(s) to Queue__JKI_lib_State_Machine.vi"("State(s) in (\"\")"=w3346) -> ("States Out"=w3345:string)  [unwired: 14 in]
      }
      frame "TCP: sendFirefly" {
        # "Template Separator\n(You can make a copy of, or modify, this frame)"
        n1543 = Unbundle By Name(w3359) -> ("System Status.TCP/IP"=w3358:bool)
        n1544 = case shown="False" w3358 {
          tunnel: [w3365 w3367] -> w3361
          tunnel: w3360 -> [w3365 w3366]
          frame False {
          }
          frame True {
            n1545 = call "TcpIDFGV.vi"("Error In"=w3366, "action"=enum16{"write", "read"}."read") -> ("Error Out"=w3368:errorcluster, "connection ID out"=w3370:refnum<k5>)  [unwired: 8 in]
            n1546 = call "TCP_WriteRead.vi"("error in (no error)"=w3368, "data in"="!firefly:0", "connectin ID in"=w3370) -> ("error out"=w3367:errorcluster)  [unwired: 4 in, 2 out]
          }
        }
        n1547 = call <vilib>:"Add State(s) to Queue__JKI_lib_State_Machine.vi"("State(s) in (\"\")"=w3364) -> ("States Out"=w3363:string)  [unwired: 14 in]
      }
      frame "TCP: sendPentero" {
        # "Send Pentero setting to AB computer\n(You can make a copy of, or modify, this frame)"
        n1548 = Unbundle By Name(w3373) -> ("System Status.TCP/IP"=w3372:bool)
        n1549 = case shown="True" w3372 {
          tunnel: [w3379 w3381] -> w3375
          tunnel: w3374 -> [w3379 w3380]
          frame False {
          }
          frame True {
            n1550 = call "TcpIDFGV.vi"("Error In"=w3380, "action"=enum16{"write", "read"}."read") -> ("Error Out"=w3382:errorcluster, "connection ID out"=w3384:refnum<k5>)  [unwired: 8 in]
            n1551 = call "TCP_WriteRead.vi"("error in (no error)"=w3382, "data in"="!pentero:0", "connectin ID in"=w3384) -> ("error out"=w3381:errorcluster)  [unwired: 4 in, 2 out]
          }
        }
        n1552 = call <vilib>:"Add State(s) to Queue__JKI_lib_State_Machine.vi"("State(s) in (\"\")"=w3378) -> ("States Out"=w3377:string)  [unwired: 14 in]
      }
      frame "TCP: sendChannel" {
        # "Send DeCon Channel to AB computer\n()"
        n1553 = Unbundle By Name(w3387) -> ("System Status.TCP/IP"=w3386:bool)
        n1554 = case shown="True" w3386 {
          tunnel: [w3393 w3397] -> w3389
          tunnel: w3388 -> [w3393 w3396]
          frame False {
          }
          frame True {
            n1555 = local read "Radio Buttons"() -> (w3395:T9)
            n1556 = case shown="\"No Selection\", Default" w3395 {
              tunnel: ["" ("data in") "!channel:1" ("data in") "!channel:2" ("data in") "!channel:3" ("data in")] -> w3394
              frame "No Selection", Default {
              }
              frame "Ch1" {
              }
              frame "Ch2" {
              }
              frame "Ch3" {
              }
            }
            n1557 = call "TcpIDFGV.vi"("Error In"=w3396, "action"=enum16{"write", "read"}."read") -> ("Error Out"=w3398:errorcluster, "connection ID out"=w3399:refnum<k5>)  [unwired: 8 in]
            n1558 = call "TCP_WriteRead.vi"("error in (no error)"=w3398, "data in"=w3394, "connectin ID in"=w3399) -> ("error out"=w3397:errorcluster)  [unwired: 4 in, 2 out]
          }
        }
        n1559 = call <vilib>:"Add State(s) to Queue__JKI_lib_State_Machine.vi"("State(s) in (\"\")"=w3392) -> ("States Out"=w3391:string)  [unwired: 14 in]
      }
      frame "TCP: startCam" {
        # "Send Pentero setting to AB computer\n(You can make a copy of, or modify, this frame)"
        n1560 = Unbundle By Name(w3406) -> ("System Status.TCP/IP"=w3405:bool)
        n1561 = case shown="True" w3405 {
          tunnel: [w3412 w3414] -> w3408
          tunnel: w3407 -> [w3412 w3413]
          frame False {
          }
          frame True {
            n1562 = call "TcpIDFGV.vi"("Error In"=w3413, "action"=enum16{"write", "read"}."read") -> ("Error Out"=w3415:errorcluster, "connection ID out"=w3417:refnum<k5>)  [unwired: 8 in]
            n1563 = call "TCP_WriteRead.vi"("error in (no error)"=w3415, "data in"="!focus:1", "connectin ID in"=w3417) -> ("error out"=w3414:errorcluster)  [unwired: 4 in, 2 out]
          }
        }
        n1564 = call <vilib>:"Add State(s) to Queue__JKI_lib_State_Machine.vi"("State(s) in (\"\")"=w3411) -> ("States Out"=w3410:string)  [unwired: 14 in]
      }
      frame "TCP: stopCam" {
        # "Send Pentero setting to AB computer\n(You can make a copy of, or modify, this frame)"
        n1565 = Unbundle By Name(w3420) -> ("System Status.TCP/IP"=w3419:bool)
        n1566 = case shown="True" w3419 {
          tunnel: [w3426 w3428] -> w3422
          tunnel: w3421 -> [w3426 w3427]
          frame False {
          }
          frame True {
            n1567 = call "TcpIDFGV.vi"("Error In"=w3427, "action"=enum16{"write", "read"}."read") -> ("Error Out"=w3429:errorcluster, "connection ID out"=w3431:refnum<k5>)  [unwired: 8 in]
            n1568 = call "TCP_WriteRead.vi"("error in (no error)"=w3429, "data in"="!focus:0", "connectin ID in"=w3431) -> ("error out"=w3428:errorcluster)  [unwired: 4 in, 2 out]
          }
        }
        n1569 = call <vilib>:"Add State(s) to Queue__JKI_lib_State_Machine.vi"("State(s) in (\"\")"=w3425) -> ("States Out"=w3424:string)  [unwired: 14 in]
      }
      frame "TCP: Close" {
        # "Close TCP connection\n()"
        n1570 = Unbundle By Name(w3435) -> ("System Status.TCP/IP"=w3433:bool)
        n1571 = case shown="True" w3433 {
          tunnel: [w3441 w3443] -> w3436
          tunnel: w3434 -> [w3441 w3442]
          frame False {
          }
          frame True {
            n1572 = call "TcpIDFGV.vi"("Error In"=w3442, "action"=enum16{"write", "read"}."read") -> ("Error Out"=w3445:errorcluster, "connection ID out"=w3446:refnum<k5>)  [unwired: 8 in]
            n1573 = TCP Close Connection(connection ID=w3446, error in (no error)=w3445) -> (error out=w3443:errorcluster)  [unwired: 1 in, 1 out]
          }
        }
        n1574 = case shown="Error .." w3436 {
          tunnel: [w3449 w3450] -> w3437
          tunnel: w3435 -> [w3448 w3450]
          frame No Error {
            w3447 = FALSE ("System Status.TCP/IP")
            n1575 = Bundle By Name(cluster=w3448, "System Status.TCP/IP"=w3447) -> (w3449:T23)
            n1576 = global write "GlobalVariables.vi" "TCP connected?"(w3447) -> ()
          }
          frame Error {
          }
        }
        n1577 = call <vilib>:"Add State(s) to Queue__JKI_lib_State_Machine.vi"("State(s) in (\"\")"=w3440) -> ("States Out"=w3439:string)  [unwired: 14 in]
      }
      frame "---------- PID ----------" {
        # "Template Separator\n(You can make a copy of, or modify, this frame)"
        n1578 = call <vilib>:"Add State(s) to Queue__JKI_lib_State_Machine.vi"("State(s) in (\"\")"=w3455) -> ("States Out"=w3454:string)  [unwired: 14 in]
      }
      frame "PID: loadPID" {
        # "Template Separator\n(You can make a copy of, or modify, this frame)"
        n1579 = call "readPIDSetting.vi"("Error In"=w3459) -> ("Error Out"=w3460:errorcluster, "Ch3 PID out"=w3456:T8, "Ch2 PID out"=w3457:T8, "Ch1 PID out"=w3458:T8)  [unwired: 7 in]
        n1580 = local write "Ch1 PID gains"(w3458) -> ()
        n1581 = local write "Ch2 PID gains"(w3457) -> ()
        n1582 = local write "Ch3 PID gains"(w3456) -> ()
        n1583 = local write "Ch4 PID gains"(w3456) -> ()
        n1584 = call <vilib>:"Add State(s) to Queue__JKI_lib_State_Machine.vi"("State(s) in (\"\")"=w3464) -> ("States Out"=w3463:string)  [unwired: 14 in]
      }
      frame "---------- Classifier ----------" {
        # "Template Separator\n(You can make a copy of, or modify, this frame)"
        n1585 = call <vilib>:"Add State(s) to Queue__JKI_lib_State_Machine.vi"("State(s) in (\"\")"=w3469) -> ("States Out"=w3468:string)  [unwired: 14 in]
      }
      frame "Classifier: Init" {
        # "Initilize Python\n(You can make a copy of, or modify, this frame)"
        n1586 = call-poly <vilib>:"Open Virtual Environment Session.vi"("error in (no error)"=w3478, "Anaconda path"=path "C:/ProgramData/miniconda3", "Python version"="Python version", "Env name"="Env name") -> ("error out"=w3474:errorcluster, "session out"=w3477:refnum<k35>)  [unwired: 6 in]
        n1587 = Path To String(path="model path") -> (string=w3471:string)
        n1588 = node "Python Node"(w3477, "module path", "load_model" ("function name"), w3474, w3471) -> (→"Python session":refnum<k35>, w3473:errorcluster)  [unwired: 3 in, 2 out]
        n1589 = call <vilib>:"Add State(s) to Queue__JKI_lib_State_Machine.vi"("State(s) in (\"\")"=w3485) -> ("States Out"=w3484:string)  [unwired: 14 in]
      }
      frame "Classifier: Close" {
        # "Template Separator\n(You can make a copy of, or modify, this frame)"
        n1590 = local read "Python session"() -> (w3489:refnum<k35>)
        n1591 = Close Python Session(session in=w3489, error in=w3488) -> (11:w3487:errorcluster)
        n1592 = case shown="Error .." w3487 {
          selector: w3487 -> [w3494 _]
          tunnel: [w3494 errorcluster {"status"=FALSE, "code"=0, "source"=""} ("error IO")] -> w3486
          frame No Error {
          }
          frame Error {
          }
        }
        n1593 = call <vilib>:"Add State(s) to Queue__JKI_lib_State_Machine.vi"("State(s) in (\"\")"=w3493) -> ("States Out"=w3492:string)  [unwired: 14 in]
      }
      frame "---------- Temp ----------" {
        # "Template Separator\n(You can make a copy of, or modify, this frame)"
        n1594 = call <vilib>:"Add State(s) to Queue__JKI_lib_State_Machine.vi"("State(s) in (\"\")"=w3500) -> ("States Out"=w3499:string)  [unwired: 14 in]
      }
      frame "Temp: KeepEmpty" {
        # "Template Separator\n(You can make a copy of, or modify, this frame)"
        n1595 = call <vilib>:"Add State(s) to Queue__JKI_lib_State_Machine.vi"("State(s) in (\"\")"=w3505) -> ("States Out"=w3504:string)  [unwired: 14 in]
      }
    }
    n1596 = Not(x=w80) -> (.not. x?=w79:bool)
    n1597 = local write "ML?"(w79) -> ()
    "ML?" <- TRUE ("main loop running?")
  }
  n1598 = while {
    tunnel: w19 -> [w3539]
    tunnel: w18 -> [w3508]
    tunnel: [w3507] -> w17
    tunnel: w13 -> [w3535]
    tunnel: [w3534] -> w16
    shift-right: [w3530] -> _
    shift-left: _ -> [w3531]
    stop <- w3510 stop-if-true
    # "Read data from notifier and deconvolve it and send to Aiming Beam computer"
    n1599 = Wait on Notification(notifier=w3539, ignore previous (F)=FALSE) -> (notification=w3526:T14, error out=w3510:errorcluster)  [unwired: 2 in, 2 out]
    n1600 = local read "Data Class"() -> (w3511:enum16{"Data", "BG", "Cali"})
    n1601 = Unbundle(w3526) -> ("idx"=w3509:i32, "CH1&2"=w3538:dbl[][], "CH3&4"=w3537:dbl[][], "V cluster"=w3516:cluster{"V1":dbl, "V2":dbl, "V3":dbl, "V4":dbl})
    n1602 = call "SeperateChanData.vi"("Input (Ch1&2)"=w3537) -> ("Ch1"=w3513:dbl[][], "Ch2"=w3521:dbl[][])
    n1603 = call "SeperateChanData.vi"("Input (Ch1&2)"=w3538) -> ("Ch1"=w3515:dbl[][], "Ch2"=w3514:dbl[][])
    n1604 = case shown="\"Data\"" w3511 {
      tunnel: w3516 -> [w3551 _]
      tunnel: w3515 -> [w3550 _]
      tunnel: w3514 -> [w3549 _]
      tunnel: w3513 -> [w3548 _]
      tunnel: w3510 -> [w3547 w3659]
      tunnel: w3509 -> [w3546 _]
      tunnel: w3508 -> [w3544 w3660]
      tunnel: [w3541 w3660] -> w3507
      tunnel: [w3540 w3659] -> w3506
      frame "Data" {
        # "If acquiring data"
        n1605 = case shown="1, 2" "Overlay selection" {
          tunnel: "Radio Buttons" -> [w3555 _]
          tunnel: [w3556 w3579] -> w3542
          tunnel: w3547 -> [w3556 w3578]
          tunnel: [w3554 w3566] -> w3545
          tunnel: w3551 -> [_ w3585]
          tunnel: w3550 -> [_ w3582]
          tunnel: w3549 -> [_ w3581]
          tunnel: w3548 -> [_ w3580]
          frame 0, Default {
            # "overlay gain"
            n1606 = case shown="\"Ch4\"" w3555 {
              tunnel: [0.0 ("Gain1") w3558 w3559 w3560 w3561] -> w3554
              frame "No Selection", Default {
              }
              frame "Ch1" {
                n1607 = local read "Gain1"() -> (w3558:dbl)
              }
              frame "Ch2" {
                n1608 = local read "Gain2"() -> (w3559:dbl)
              }
              frame "Ch3" {
                n1609 = local read "Gain3"() -> (w3560:dbl)
              }
              frame "Ch4" {
                n1610 = local read "Gain4"() -> (w3561:dbl)
              }
            }
          }
          frame 1, 2 {
            # "overlay lifetime or cancer probability"
            n1611 = call "DeConAPD2FGV.vi"("Error In"=w3578) -> ("Error Out"=w3584:errorcluster, "APDClass out"=w3575:T40)  [unwired: 9 in]
            n1612 = call "DeConAPD1FGV.vi"("Error In"=w3578) -> ("Error Out"=w3586:errorcluster, "APDClass out"=w3577:T40)  [unwired: 9 in]
            n1613 = call "DeConAPD3FGV.vi"("Error In"=w3578) -> ("Error Out"=w3583:errorcluster, "APDClass out"=w3573:T40)  [unwired: 9 in]
            n1614 = Unbundle By Name(w3585) -> ("V1"=w3576:dbl, "V2"=w3574:dbl, "V3"=w3572:dbl)
            n1615 = call "getGain.vi"("CtrlV"=w3572, "APD"=w3573) -> ("gain"=w3563:dbl)  [unwired: 8 in, 1 out]
            n1616 = call "getGain.vi"("CtrlV"=w3576, "APD"=w3577) -> ("gain"=w3565:dbl)  [unwired: 8 in, 1 out]
            n1617 = call "getGain.vi"("CtrlV"=w3574, "APD"=w3575) -> ("gain"=w3564:dbl)  [unwired: 8 in, 1 out]
            n1618 = Less?(x=w3565, y="Ch1GainLim") -> (x < y?=w3570:bool)
            n1619 = Less?(x=w3564, y="Ch2&3GainLim") -> (x < y?=w3569:bool)
            n1620 = Less?(x=w3563, y="Ch2&3GainLim") -> (x < y?=w3568:bool)
            n1621 = Compound Arithmetic op=AND(w3570, w3569, w3568) -> (w3567:bool)
            n1622 = case shown="True" w3567 {
              tunnel: w3586 -> [_ w3649]
              tunnel: w3584 -> [_ w3648]
              tunnel: w3583 -> [_ w3647]
              tunnel: w3582 -> [_ w3637]
              tunnel: w3581 -> [_ w3636]
              tunnel: w3580 -> [_ w3635]
              tunnel: [w3587 w3596] -> w3579
              tunnel: w3578 -> [w3587 w3628]
              tunnel: w3577 -> [_ w3627]
              tunnel: w3576 -> [_ w3626]
              tunnel: w3575 -> [_ w3625]
              tunnel: w3574 -> [_ w3624]
              tunnel: w3573 -> [_ w3623]
              tunnel: w3572 -> [_ w3622]
              tunnel: [0.0 ("Gain4") w3589] -> w3566
              tunnel: w3565 -> [_ w3614]
              tunnel: w3564 -> [_ w3613]
              tunnel: w3563 -> [_ w3612]
              frame False {
                # "give probability of 0.5"
                # "if gain is out of acceptable range"
              }
              frame True {
                # "if gain is within range"
                n1623 = Build Array(w3614, w3613, w3612) -> (w3611:dbl[])
                n1624 = call "getIrf (SubVI).vi"("error in"=w3649, "CtrlV"=w3626, "APD"=w3627) -> ("error out"=w3641:errorcluster, "irfTNorm"=w3644:dbl[])  [unwired: 6 in, 1 out]
                n1625 = call "getIrf (SubVI).vi"("error in"=w3648, "CtrlV"=w3624, "APD"=w3625) -> ("error out"=w3640:errorcluster, "irfTNorm"=w3643:dbl[])  [unwired: 6 in, 1 out]
                n1626 = call "getIrf (SubVI).vi"("error in"=w3647, "CtrlV"=w3622, "APD"=w3623) -> ("error out"=w3639:errorcluster, "irfTNorm"=w3642:dbl[])  [unwired: 6 in, 1 out]
                n1627 = call "DotNetFGV.vi"("Error In"=w3628) -> ("Error Out"=w3632:errorcluster, "reference out"=w3633:refnum<k24>)  [unwired: 9 in]
                n1628 = local read "BGAll"() -> (w3646:dbl[][])
                n1629 = Merge Errors(w3632, w3641, w3640, w3639) -> (w3638:errorcluster)
                n1630 = Build Array(w3644, w3643, w3642) -> (w3629:dbl[][])
                n1631 = Build Array (concatenate)(w3637, w3636, w3635) -> (w3634:dbl[][])
                n1632 = local write "iRF Graph"(w3629) -> ()
                n1633 = Transpose 2D Array(2D array=w3646) -> (transposed array=w3645:dbl[][])
                n1634 = Transpose 2D Array(2D array=w3629) -> (transposed array=w3630:dbl[][])
                n1635 = Transpose 2D Array(2D array=w3634) -> (transposed array=w3631:dbl[][])
                n1636 = Reciprocal(x=w3611) -> (1/x=w3609:dbl[])
                n1637 = call "LagDeConAllCh (SubVI).vi"("new reference"=w3633, "error in (no error)"=w3638, "irf"=w3630, "BG"=w3645, "WF"=w3631) -> ("error out"=w3597:errorcluster, "LCs"=w3605:dbl[][], "INTs"=w3616:dbl[][], "LTs"=w3621:dbl[][])  [unwired: 3 in]
                n1638 = Index Array(array=w3621, index (col)=0 ("disabled index (col)")) -> (element=w3603:dbl[])  [unwired: 1 in]
                n1639 = Index Array(array=w3616, index (col)=0 ("disabled index (col)")) -> (element=w3610:dbl[])  [unwired: 1 in]
                n1640 = Multiply(x=w3610, y=w3609) -> (x*y=w3608:dbl[])
                n1641 = Index Array(array=w3605, index (col)=0 ("disabled index (col)")) -> (element=w3601:dbl[])  [unwired: 1 in]
                n1642 = Add Array Elements(numeric array=w3608) -> (sum=w3607:dbl)
                n1643 = Index Array(array=w3603, index=0) -> (element=w3593:dbl)
                "Ch1 Lifetime (ns)" <- w3593
                n1644 = Index Array(array=w3603, index=1) -> (element=w3592:dbl)
                "Ch2 Lifetime (ns)" <- w3592
                n1645 = Index Array(array=w3603, index=2) -> (element=w3591:dbl)
                "Ch3 Lifetime (ns)" <- w3591
                n1646 = Divide(x=w3608, y=w3607) -> (x/y=w3602:dbl[])
                n1647 = Bundle(w3593, w3592, w3591) -> (→"Lifetime (ns)":cluster{dbl, dbl, dbl})  [unwired: 1 in]
                n1648 = Build Array (concatenate)(w3603, w3602, w3601) -> (w3594:dbl[])
                "DeConOut" <- w3594
                n1649 = local read "module path"() -> (w3599:path)
                n1650 = local read "Python session"() -> (w3600:refnum<k35>)
                n1651 = node(w3600, w3599, "Predict" ("function name"), w3597, 0.0, w3594) -> (w3596:errorcluster, w3590:dbl)  [unwired: 1 in, 3 out]
                "Cancer Prob" <- w3590
                n1652 = disable-structure shown="Enabled" {
                  disable-tunnel: w3590 -> [w3652 w3657]
                  disable-tunnel: [w3651 w3653] -> w3589
                  frame Disabled {
                    n1653 = Add(x=0.01, y=w3652) -> (x+y=w3651:dbl)
                  }
                  frame Enabled {
                    n1654 = Greater?(x=w3657, y="CancerThreshold") -> (0:w3658:bool)
                    n1655 = Select(t=1.0, s=w3658, f=0.01) -> (s? t:f=w3653:dbl)
                  }
                }
              }
            }
          }
        }
        n1656 = Bundle("idx"=w3546, "f"=w3545) -> (w3543:cluster{"idx":i32, "f":dbl})  [unwired: 1 in]
        n1657 = Send Notification(notification=w3543, notifier=w3544, error in (no error)=w3542) -> (notifier out=w3541:refnum<notifier>, error out=w3540:errorcluster)
      }
      frame "BG", Default {
        # "if not acquiting data"
      }
    }
    n1658 = call "AvgArrayTimeCritical.vi"("2D array"=w3515) -> ("1D Avg"=w3522:dbl[])  [unwired: 10 in]
    n1659 = call "AvgArrayTimeCritical.vi"("2D array"=w3514) -> ("1D Avg"=w3523:dbl[])  [unwired: 10 in]
    n1660 = call "AvgArrayTimeCritical.vi"("2D array"=w3513) -> ("1D Avg"=w3524:dbl[])  [unwired: 10 in]
    n1661 = call "AvgArrayTimeCritical.vi"("2D array"=w3521) -> ("1D Avg"=w3525:dbl[])  [unwired: 10 in]
    n1662 = Build Array(w3525) -> (w3520:dbl[][])
    n1663 = Build Array(w3524) -> (w3519:dbl[][])
    n1664 = Build Array(w3523) -> (w3518:dbl[][])
    n1665 = Build Array(w3522) -> (w3517:dbl[][])
    n1666 = flat-sequence {
      tunnel: [w3661] -> w3530
      tunnel: w3510 -> [_]
      frame #0 {
        n1667 = call <vilib>:"High Resolution Relative Seconds.vi"() -> ("relative seconds"=w3661:dbl)
      }
    }
    n1668 = Subtract(x=w3530, y=w3531) -> (x-y=w3533:dbl)
    n1669 = Multiply(x=w3533, y=1000.0) -> (x*y=→"Decon Loop timing (ms)" →"DeCon Speed(ms)":dbl)
    n1670 = Bundle(w3517, w3518, w3519, w3520, "V cluster"=w3516) -> (w3536:T48)  [unwired: 1 in]
    n1671 = Send Notification(notification=w3536, notifier=w3535, error in (no error)=w3510) -> (notifier out=w3534:refnum<notifier>, error out=w3512:errorcluster)
    n1672 = Merge Errors(w3506, w3512) -> (→"decon error out":errorcluster)
  }
  n1673 = while {
    tunnel: w18 -> [w3673]
    shift-right: [w3666] -> _
    shift-left: u32 0 -> [w3667]
    stop <- w3664 stop-if-true
    # "Send data to AB computer here"
    # "if TCP ip is not open loop will run once and stop. To re-establish connection and start this loop. Reboot softwrae."
    # "Data communication loop"
    n1674 = Wait on Notification(notifier=w3673, ignore previous (F)=FALSE) -> (notification=w3671:cluster{"idx":i32, "lifetime":dbl}, error out=w3665:errorcluster)  [unwired: 2 in, 2 out]
    n1675 = Wait Until Next ms Multiple(millisecond multiple=u32 25) -> ()  [unwired: 1 out]
    n1676 = Unbundle(w3671) -> ("idx"=w3670:i32, "lifetime"=w3669:dbl)
    n1677 = Tick Count (ms)() -> (millisecond timer value=w3666:u32)
    n1678 = global read "GlobalVariables.vi" "TCP connected?"() -> (w3663:bool)
    n1679 = Subtract(x=w3666, y=w3667) -> (x-y=→"Communication loop(ms)":u32)
    n1680 = case shown="True" w3663 {
      tunnel: w3670 -> [_ w3682]
      tunnel: w3669 -> [_ w3681]
      tunnel: w3665 -> [w3674 w3678]
      tunnel: [w3674 w3675] -> w3664
      frame False {
      }
      frame True {
        n1681 = Number To Decimal String(number=w3682) -> (decimal integer string=w3690:string)  [unwired: 1 in]
        n1682 = call "TcpIDFGV.vi"("Error In"=w3678, "action"=enum16{"write", "read"}."read") -> ("Error Out"=w3677:errorcluster, "connection ID out"=w3688:refnum<k5>)  [unwired: 8 in]
        n1683 = Concatenate Strings("!idx:", w3690) -> (w3691:string)
        n1684 = call "TCP_WriteRead.vi"("error in (no error)"=w3677, "data in"=w3691, "connectin ID in"=w3688) -> ("error out"=w3676:errorcluster, "connectin ID out"=w3689:refnum<k5>)  [unwired: 4 in, 1 out]
        n1685 = Number To Fractional String(number=w3681, precision (6)=i16 2) -> (F-format string=w3680:string)  [unwired: 2 in]
        n1686 = Concatenate Strings("!lifetime:", w3680) -> (w3687:string)
        n1687 = call "TCP_WriteRead.vi"("error in (no error)"=w3676, "data in"=w3687, "connectin ID in"=w3689) -> ("error out"=w3675:errorcluster, "data out"=→"data out(communcation loop)":string)  [unwired: 4 in, 1 out]
      }
    }
  }
  n1688 = while {
    tunnel: w13 -> [w3702]
    shift-right: [w3693] -> _
    shift-left: w15 -> [w3700]
    shift-right: [w3695] -> _
    shift-left: w15 -> [w3694]
    i -> [w3696]
    stop <- w3697 stop-if-true
    # "Data display loop(30Hz)"
    n1689 = Wait on Notification(notifier=w3702, ignore previous (F)=FALSE) -> (notification=w3698:T13, error out=w3697:errorcluster)  [unwired: 2 in, 2 out]
    n1690 = Wait Until Next ms Multiple(millisecond multiple=u32 40) -> ()  [unwired: 1 out]
    n1691 = Tick Count (ms)() -> (millisecond timer value=w3693:u32)
    n1692 = Subtract(x=w3693, y=w3700) -> (x-y=→"display loop timing(ms)":u32)
    n1693 = case shown="No Error" w3697 {
      tunnel: w3698 -> [w3775 _]
      tunnel: w3694 -> [w3747 w3847]
      tunnel: [w3749 w3847] -> w3695
      tunnel: w3693 -> [w3746 _]
      frame No Error {
        w3704 = u32 1 ("Active Plot")
        w3723 = 0 ("index (row)")
        n1694 = Subtract(x=w3746, y=w3747) -> (x-y=w3748:u32)
        n1695 = Unbundle(w3775) -> ("CH1"=w3770:dbl[][], "CH2"=w3768:dbl[][], "CH3"=w3765:dbl[][], "CH4"=w3718:dbl[][], "Gain cluster"=w3724:cluster{"V1":dbl, "V2":dbl, "V3":dbl, "V4":dbl})
        n1696 = Unbundle By Name(w3724) -> ("V1"=w3742:dbl, "V2"=w3740:dbl, "V3"=w3738:dbl, "V4"=w3716:dbl)
        n1697 = Index Array(array=w3770, index (row)=w3723) -> (element=w3754:dbl[])  [unwired: 1 in]
        n1698 = Index Array(array=w3768, index (row)=w3723) -> (element=w3752:dbl[])  [unwired: 1 in]
        n1699 = Index Array(array=w3765, index (row)=w3723) -> (element=w3753:dbl[])  [unwired: 1 in]
        n1700 = Index Array(array=w3718, index (row)=w3723) -> (element=w3722:dbl[])  [unwired: 1 in]
        n1701 = call "RemoveDCBG.vi"("Channel"=enum16{"DC Only", "Ch1", "Ch2", "Ch3", "Ch4"}."Ch4", "WF in"=w3722) -> ("DC"=w3720:dbl, "WF out"=w3709:dbl[])  [unwired: 7 in, 1 out]
        n1702 = Greater?(x=w3748, y=u32 200) -> (0:w3750:bool)
        n1703 = call "CtrlVtoGain.vi"("CtrlV(V)"=w3716, "Channel"=enum16{"Ch1", "Ch2", "Ch3", "Ch4"}."Ch4") -> ("Gain"=w3708:dbl)  [unwired: 8 in, 1 out]
        n1704 = call "CtrlVtoGain.vi"("CtrlV(V)"=w3742, "Channel"=enum16{"Ch1", "Ch2", "Ch3"}."Ch1") -> ("Gain"=w3736:dbl)  [unwired: 8 in, 1 out]
        n1705 = call "RemoveDCBG.vi"("Channel"=enum16{"DC Only", "Ch1", "Ch2", "Ch3"}."Ch1", "WF in"=w3754) -> ("DC"=w3771:dbl, "WF out"=w3743:dbl[])  [unwired: 7 in, 1 out]
        n1706 = call "RemoveDCBG.vi"("Channel"=enum16{"DC Only", "Ch1", "Ch2", "Ch3"}."Ch2", "WF in"=w3752) -> ("DC"=w3767:dbl, "WF out"=w3744:dbl[])  [unwired: 7 in, 1 out]
        n1707 = call "CtrlVtoGain.vi"("CtrlV(V)"=w3740, "Channel"=enum16{"Ch1", "Ch2", "Ch3"}."Ch2") -> ("Gain"=w3731:dbl)  [unwired: 8 in, 1 out]
        n1708 = call "RemoveDCBG.vi"("Channel"=enum16{"DC Only", "Ch1", "Ch2", "Ch3"}."Ch3", "WF in"=w3753) -> ("DC"=w3764:dbl, "WF out"=w3745:dbl[])  [unwired: 7 in, 1 out]
        n1709 = call "CtrlVtoGain.vi"("CtrlV(V)"=w3738, "Channel"=enum16{"Ch1", "Ch2", "Ch3"}."Ch3") -> ("Gain"=w3727:dbl)  [unwired: 8 in, 1 out]
        n1710 = formula code="int32 out = 2;\nif (G<5){\nout = 1;\n}\nif (G>200){\nout = 3;\n}"("G"=w3708) -> ("out"=→"output variable":i32)
        n1711 = Add(x=w3709, y=w3720) -> (x+y=w3719:dbl[])
        n1712 = Less?(x=w3708, y=5.0) -> (x < y?=w3714:bool)
        n1713 = case shown="True" w3750 {
          tunnel: w3743 -> [_ w3804]
          tunnel: w3744 -> [_ w3807]
          tunnel: w3745 -> [_ w3806]
          tunnel: w3746 -> [_ w3822]
          tunnel: [w3786 w3822] -> w3749
          tunnel: w3747 -> [w3786 _]
          tunnel: w3736 -> [_ w3800]
          tunnel: w3731 -> [_ w3799]
          tunnel: w3727 -> [_ w3798]
          tunnel: w3709 -> [_ w3794]
          tunnel: w3708 -> [_ w3791]
          frame False {
          }
          frame True {
            n1714 = call "GetSNR(SubVI).vi"("Waveform"=w3804) -> ("SNR"=→"SNR1":dbl)  [unwired: 10 in]
            n1715 = Array Size(array=w3804) -> (size(s)=w3805:i32)
            n1716 = call "GetSNR(SubVI).vi"("Waveform"=w3807) -> ("SNR"=→"SNR2":dbl)  [unwired: 10 in]
            n1717 = call "GetSNR(SubVI).vi"("Waveform"=w3806) -> ("SNR"=→"SNR3":dbl)  [unwired: 10 in]
            n1718 = call "GetSNR(SubVI).vi"("Waveform"=w3794) -> ("SNR"=→"SNR4":dbl)  [unwired: 10 in]
            n1719 = global read "GlobalVariables.vi" "BG Idx2"() -> (w3793:i32)
            n1720 = Subtract(x=w3805, y=w3793) -> (x-y=w3792:i32)
            n1721 = Array Subset(array=w3804, index=w3793, length=w3792) -> (w3811:dbl[])
            n1722 = Array Subset(array=w3807, index=w3793, length=w3792) -> (w3813:dbl[])
            n1723 = Array Subset(array=w3806, index=w3793, length=w3792) -> (w3815:dbl[])
            n1724 = Array Subset(array=w3794, index=w3793, length=w3792) -> (w3795:dbl[])
            n1725 = Add Array Elements(numeric array=w3811) -> (sum=w3812:dbl)
            n1726 = Add Array Elements(numeric array=w3813) -> (sum=w3814:dbl)
            n1727 = Add Array Elements(numeric array=w3815) -> (sum=w3816:dbl)
            n1728 = Add Array Elements(numeric array=w3795) -> (sum=w3796:dbl)
            n1729 = Divide(x=w3812, y=w3800) -> (x/y=w3817:dbl)
            n1730 = Divide(x=w3814, y=w3799) -> (x/y=w3818:dbl)
            n1731 = Divide(x=w3816, y=w3798) -> (x/y=w3819:dbl)
            n1732 = Divide(x=w3796, y=w3791) -> (x/y=w3790:dbl)
            n1733 = Build Array(w3817, w3818, w3819, w3790) -> (w3820:dbl[])
            n1734 = Add Array Elements(numeric array=w3820) -> (sum=w3821:dbl)
            n1735 = Divide(x=w3820, y=w3821) -> (x/y=w3789:dbl[])
            n1736 = Index Array(array=w3789, index=2) -> (element=→"IntR3":dbl)
            n1737 = Index Array(array=w3789, index=1) -> (element=→"IntR2":dbl)
            n1738 = Index Array(array=w3789, index=0) -> (element=→"IntR1":dbl)
            n1739 = Index Array(array=w3789, index=3) -> (element=→"IntR4":dbl)
          }
        }
        n1740 = Add(x=w3743, y=w3771) -> (x+y=w3769:dbl[])
        n1741 = Add(x=w3744, y=w3767) -> (x+y=w3766:dbl[])
        n1742 = Add(x=w3745, y=w3764) -> (x+y=w3763:dbl[])
        n1743 = Less?(x=w3736, y=5.0 ("x")) -> (x < y?=w3734:bool)
        n1744 = Less?(x=w3731, y=5.0 ("x")) -> (x < y?=w3730:bool)
        n1745 = Less?(x=w3727, y=5.0 ("x")) -> (x < y?=w3726:bool)
        n1746 = case shown="False" w3726 {
          tunnel: [u32 16448250 ("Plot.Plot Color") u32 16711680 ("Plot.Plot Color")] -> w3725
          frame False {
          }
          frame True {
          }
        }
        n1747 = case shown="True" "Show BG removed?" {
          tunnel: w3770 -> [w3829 w3845]
          tunnel: w3769 -> [_ w3835]
          tunnel: [w3829 w3844] -> w3762
          tunnel: w3768 -> [w3828 w3843]
          tunnel: [w3828 w3842] -> w3706
          tunnel: w3766 -> [_ w3831]
          tunnel: w3765 -> [w3827 w3841]
          tunnel: [w3827 w3840] -> w3757
          tunnel: w3763 -> [_ w3836]
          tunnel: [w3826 w3839] -> w3713
          tunnel: w3719 -> [_ w3833]
          tunnel: w3718 -> [w3826 w3838]
          frame False {
          }
          frame True {
            n1748 = Insert Into Array(array=w3841, index (row)=1, new element=w3836) -> (w3840:dbl[][])  [unwired: 1 in]
            n1749 = Insert Into Array(array=w3845, index (row)=1, new element=w3835) -> (w3844:dbl[][])  [unwired: 1 in]
            n1750 = Insert Into Array(array=w3843, index (row)=1, new element=w3831) -> (w3842:dbl[][])  [unwired: 1 in]
            n1751 = Insert Into Array(array=w3838, index (row)=1, new element=w3833) -> (w3839:dbl[][])  [unwired: 1 in]
          }
        }
        "Channel 1" <- w3762
        "Channel 2" <- w3706
        "Channel 3" <- w3757
        "Channel 4" <- w3713
        n1752 = case shown="False" w3734 {
          tunnel: [u32 16448250 ("Plot.Plot Color") u32 16711680 ("Plot.Plot Color")] -> w3733
          frame False {
          }
          frame True {
          }
        }
        n1753 = case shown="False" w3730 {
          tunnel: [u32 16448250 ("Plot.Plot Color") u32 16711680 ("Plot.Plot Color")] -> w3729
          frame False {
          }
          frame True {
          }
        }
        n1754 = case shown="False" w3714 {
          tunnel: [u32 16448250 ("Plot.Plot Color") u32 16711680 ("Plot.Plot Color")] -> w3710
          frame False {
          }
          frame True {
          }
        }
        n1755 = case shown="False" "Show BG removed?" {
          tunnel: [u32 16744703 ("Plot.Plot Color") u32 16741120 ("Plot.Plot Color")] -> w3703
          frame False {
          }
          frame True {
          }
        }
        n1756 = property on="Channel 1" class="WFGraph (strict)"("Active Plot"=w3704, "Plot.Plot Color"=w3703, "Plot.Line Style"=u8 1, "Plot.Line Width"=u8 2, "BG Color"=w3733) -> ()  [unwired: 2 in, 2 out]
        n1757 = property on="Channel 2" class="WFGraph (strict)"("Active Plot"=w3704, "Plot.Plot Color"=w3703, "Plot.Line Style"=u8 1, "Plot.Line Width"=u8 2, "BG Color"=w3729) -> ()  [unwired: 2 in, 2 out]
        n1758 = property on="Channel 4" class="WFGraph (strict)"("Active Plot"=w3704, "Plot.Plot Color"=w3703, "Plot.Line Style"=u8 1, "Plot.Line Width"=u8 2, "BG Color"=w3710) -> ()  [unwired: 2 in, 2 out]
        n1759 = property on="Channel 3" class="WFGraph (strict)"("Active Plot"=w3704, "Plot.Plot Color"=w3703, "Plot.Line Style"=u8 1, "Plot.Line Width"=u8 2, "BG Color"=w3725) -> ()  [unwired: 2 in, 2 out]
      }
      frame Error {
        w3846 = u32 16448250 ("Plot Area:Colors:BG Color")
        n1760 = property on="Channel 1" class="WFGraph (strict)"("BG Color"=w3846) -> ()  [unwired: 2 in, 2 out]
        n1761 = property on="Channel 2" class="WFGraph (strict)"("BG Color"=w3846) -> ()  [unwired: 2 in, 2 out]
        n1762 = property on="Channel 3" class="WFGraph (strict)"("BG Color"=w3846) -> ()  [unwired: 2 in, 2 out]
      }
    }
    "DisplayLoop" <- w3696
  }
  n1763 = while {
    tunnel: w65 -> [w3860]
    tunnel: w55 -> [w3859]
    tunnel: [w3858] -> w63
    tunnel: w19 -> [w3857]
    tunnel: [w3856] -> w59
    tunnel: w39 -> [w3854]
    tunnel: w48 -> [w3853]
    tunnel: w35 -> [w3848]
    stop <- w3851 stop-if-true
    # "acquire data and send it to processing loop"
    # "Data Aquisition Loop"
    n1764 = event shown="[1] <Start digitizer>: User Event" {
      selector: w3859 -> [_ _]
      dyn-events: [_ _] -> w3858
      timeout: 30 -> [_ _]
      tunnel: w3860 -> [w3866 w3876]
      tunnel: [w3861 _] -> w3851
      tunnel: w3857 -> [w3865 w3883]
      tunnel: [w3865 w3882] -> w3856
      tunnel: w3854 -> [_ w3880]
      tunnel: w3853 -> [w3864 w3875]
      tunnel: w3848 -> [_ w3873]
      event Timeout {
        # "use queue to stop data loop\nwhen queue ref is released, error will stop this loop"
        n1765 = event-data() -> ()  [unwired: 1 in, 3 out]
        n1766 = Get Queue Status(queue=w3866) -> (error out=w3863:errorcluster)  [unwired: 2 in, 7 out]
        n1767 = Get Queue Status(queue=w3864) -> (error out=w3862:errorcluster)  [unwired: 2 in, 7 out]
        n1768 = Merge Errors(w3863, w3862) -> (w3861:errorcluster)
      }
      event User Event {
        w3881 = enum16{"Write", "Read"}."Read" ("Operation")
        n1769 = event-data() -> ("Time"=→"RunStartTime":u32)  [unwired: 1 in, 3 out]
        n1770 = call "FLImDAQ_FGV.vi"() -> ("Read data"=w3878:T5)  [unwired: 10 in, 1 out]
        n1771 = call "Digitizer1_FGV.vi"("Operation (Read)"=w3881) -> ("Read data"=w3872:refnum<k15>)  [unwired: 9 in, 1 out]
        n1772 = call "Digitizer2_FGV.vi"("Operation (Read)"=w3881) -> ("Read data"=w3879:refnum<k15>)  [unwired: 9 in, 1 out]
        n1773 = Unbundle By Name(w3878) -> ("Waveform to Avg"=w3877:i16)
        n1774 = property on="Property Node" class="niScope"(reference=w3872) -> (reference out=w3871:refnum<k15>, "Vertical Range"=w3870:dbl, "Vertical Offset"=w3869:dbl)  [unwired: 1 in, 1 out]
        n1775 = Tick Count (ms)() -> (millisecond timer value=w3868:u32)
        n1776 = while {
          tunnel: w3883 -> [w3943]
          tunnel: [w3942] -> w3882
          tunnel: w3879 -> [w3936]
          tunnel: w3871 -> [w3935]
          tunnel: w3880 -> [w3934]
          shift-right: [w3903] -> _
          shift-left: u32 0 ("millisecond timer value") -> [w3928]
          tunnel: w3877 -> [w3884]
          tunnel: w3876 -> [w3925]
          tunnel: w3875 -> [w3923]
          tunnel: w3873 -> [w3916]
          tunnel: w3870 -> [w3913]
          tunnel: w3869 -> [w3914]
          shift-right: [w3908] -> _
          shift-left: w3868 -> [w3907]
          i -> [w3885]
          stop <- w3906 stop-if-true
          w3896 = enum16{"write", "read"}."read" ("action")
          w3929 = 65536
          # "enqueue V"
          # "enqueue ch3 data"
          # "enqueue ch1&2 data"
          # "acquire ch3"
          # "acquire ch1&2"
          # "send data for processing"
          n1777 = Multiply(x=w3884, y=w3885) -> (x*y=w3893:i32)
          "Fetch Record #" <- w3893
          n1778 = property on="Property Node" class="niScope"(reference=w3935, "Fetch Record Number"=w3893) -> (reference out=w3947:refnum<k15>, error out=w3946:errorcluster, "Records Done"=w3915:i32)  [unwired: 1 in]
          n1779 = Subtract(x=w3915, y=w3893) -> (x-y=→"Record Backlog":i32)
          n1780 = call-poly <instrlib>:"niScope Fetch (poly).vi"("timeout"=1.0, "error in"=w3946, "channels"="0,1", "instrument handle"=w3947) -> ("error out"=w3890:errorcluster, "wfm"=w3891:i16[][], "wfm info"=w3912:T49)  [unwired: 4 in, 1 out]
          n1781 = property on="Property Node" class="niScope"(reference=w3936, "Fetch Record Number"=w3893) -> (reference out=w3940:refnum<k15>, error out=w3937:errorcluster, "Records Done"=w3894:i32)  [unwired: 1 in]
          n1782 = Divide(x=w3891, y=w3929) -> (x/y=w3902:dbl[][])
          n1783 = Tick Count (ms)() -> (millisecond timer value=w3903:u32)
          n1784 = Subtract(x=w3894, y=w3893) -> (x-y=→"Record Backlog 2":i32)
          n1785 = Subtract(x=w3903, y=w3928) -> (x-y=→"Aquisition loop timing(ms)":u32)
          n1786 = Subtract(x=w3903, y=w3907) -> (x-y=w3911:u32)
          n1787 = Multiply(x=w3902, y=w3913) -> (x*y=w3933:dbl[][])
          n1788 = call-poly <instrlib>:"niScope Fetch (poly).vi"("timeout"=0.25, "error in"=w3937, "channels"="0,1", "instrument handle"=w3940) -> ("error out"=w3889:errorcluster, "wfm"=w3930:i16[][])  [unwired: 4 in, 2 out]
          n1789 = Greater?(x=w3911, y=u32 1000) -> (0:w3909:bool)
          n1790 = Add(x=w3933, y=w3914) -> (x+y=w3924:dbl[][])
          n1791 = case shown="True" w3909 {
            tunnel: w3912 -> [_ w3956]
            tunnel: w3903 -> [_ w3955]
            tunnel: [w3949 w3955] -> w3908
            tunnel: w3907 -> [w3949 _]
            tunnel: [errorcluster {"status"=FALSE, "code"=0, "source"=""} ("error constant") w3952] -> w3904
            frame False {
            }
            frame True {
              # "[Covers: REQ29]"
              n1792 = call "CheckFrequency(SubVI).vi"("wfm info"=w3956) -> ("f (Hz)"=w3954:dbl)  [unwired: 10 in]
              "Laser f (Hz)" <- w3954
              n1793 = local read "Laser Rep Rate"() -> (w3951:dbl)
              n1794 = Increment(x=w3951) -> (x+1=w3950:dbl)
              n1795 = Greater?(x=w3954, y=w3950) -> (0:w3953:bool)
              n1796 = case shown="True" w3953 {
                tunnel: [errorcluster {"status"=FALSE, "code"=0, "source"=""} ("error constant") errorcluster {"status"=TRUE, "code"=0, "source"=""} ("error constant")] -> w3952
                frame False {
                }
                frame True {
                }
              }
            }
          }
          n1797 = Divide(x=w3930, y=w3929) -> (x/y=w3932:dbl[][])
          n1798 = Enqueue Element(queue=w3925, element=w3924, error in (no error)=w3890) -> (error out=w3888:errorcluster)  [unwired: 1 in, 2 out]
          n1799 = Multiply(x=w3932, y=w3913) -> (x*y=w3931:dbl[][])
          n1800 = Add(x=w3931, y=w3914) -> (x+y=w3922:dbl[][])
          n1801 = Enqueue Element(queue=w3923, element=w3922, error in (no error)=w3889) -> (error out=w3887:errorcluster)  [unwired: 1 in, 2 out]
          n1802 = Merge Errors(w3888, w3887) -> (w3886:errorcluster)
          n1803 = call "V1FGV.vi"("Error In"=w3886, "action (write)"=w3896) -> ("Error Out"=w3920:errorcluster, "V1 out"=w3918:dbl)  [unwired: 8 in]
          n1804 = call "V2FGV.vi"("Error In"=w3920, "action(write)"=w3896) -> ("Error Out"=w3919:errorcluster, "V2 out"=w3917:dbl)  [unwired: 8 in]
          n1805 = call "V3FGV.vi"("Error In"=w3919, "action(write)"=w3896) -> ("Error Out"=w3899:errorcluster, "V3 out"=w3898:dbl)  [unwired: 8 in]
          n1806 = call "V4FGV.vi"("Error In"=w3899, "action(write)"=w3896, "V3 in"=w3898) -> ("Error Out"=w3897:errorcluster, "V3 out"=w3895:dbl)  [unwired: 7 in]
          n1807 = Bundle("V1 out"=w3918, "V2 out"=w3917, "V3 out"=w3898, "V3 out"=w3895) -> (w3901:T50)  [unwired: 1 in]
          n1808 = Bundle(w3885, w3924, w3922, w3901) -> (w3926:T51)  [unwired: 1 in]
          n1809 = Enqueue Element(queue=w3916, element=w3901, error in (no error)=w3897) -> (error out=w3900:errorcluster)  [unwired: 1 in, 2 out]
          n1810 = Send Notification(notification=w3926, notifier=w3943, error in (no error)=w3900) -> (notifier out=w3942:refnum<notifier>, error out=w3905:errorcluster)
          n1811 = Merge Errors(w3904, w3905) -> (w3921:errorcluster)
          n1812 = case shown="Error .." w3921 {
            selector: w3921 -> [w3959 w3960]
            tunnel: w3934 -> [_ w3963]
            tunnel: [w3959 w3960] -> w3906
            frame No Error {
            }
            frame Error {
              # "Send user event to signal aquisition has stoped"
              n1813 = Generate User Event(priority (normal)=usereventprio."high priority", user event=w3963, event data cluster=TRUE ("event data")) -> ()  [unwired: 1 in, 2 out]
            }
          }
          "aquisition loop Error Out" <- w3906
          "Auisition Loop idx" <- w3885
        }
      }
    }
    n1814 = Unbundle By Name(w3851) -> ("status"=w3850:bool)
    n1815 = Not(x=w3850) -> (.not. x?=w3849:bool)
    n1816 = local write "Aq Loop?"(w3849) -> ()
    "Aq Loop?" <- TRUE ("Aq L?")
  }
  n1817 = disable-structure "Diagram Disable Structure" shown="Disabled" {
    frame Disabled {
      w3964 = T52 {"Horizontal"=500, "Vertical"=100}  # Top Left Corner
      n1818 = Control Help Window(0:w3964, 1:TRUE ("Show")) -> ()
      n1819 = call <vilib>:"TDMS - File Viewer.vi"() -> ()  [unwired: 6 in, 2 out]
    }
    frame Enabled {
    }
  }
  n1820 = while {
    tunnel: w19 -> [w4013]
    shift-right: [w3977] -> _
    shift-left: _ -> [w4009]
    tunnel: [w3968] -> w1 mode=indexing
    i -> [w3993]
    stop <- w3974 stop-if-true
    # "Channel 3"
    # "Channel 2"
    # "Channel 1"
    # "use FGV for gain value"
    # "stop on error"
    # "Gain adjustment and Data processing"
    n1821 = Tick Count (ms)() -> (millisecond timer value=w3977:u32)
    n1822 = Wait on Notification(notifier=w4013, ignore previous (F)=TRUE) -> (notification=w3987:T14, error out=w3967:errorcluster)  [unwired: 2 in, 2 out]
    n1823 = Subtract(x=w3977, y=w4009) -> (x-y=→"PID loop timing(ms)":u32)
    n1824 = Unbundle(w3987) -> ("CH1&2"=w4003:dbl[][], "CH3&4"=w4002:dbl[][])  [unwired: 2 out]
    n1825 = call "SeperateChanData.vi"("Input (Ch1&2)"=w4003) -> ("Ch1"=w3998:dbl[][], "Ch2"=w3996:dbl[][])
    n1826 = call "SeperateChanData.vi"("Input (Ch1&2)"=w4002) -> ("Ch1"=w3992:dbl[][], "Ch2"=w3985:dbl[][])
    n1827 = call "AvgArrayTimeCritical.vi"("2D array"=w3998) -> ("1D Avg"=w3997:dbl[])  [unwired: 10 in]
    n1828 = call "AvgArrayTimeCritical.vi"("2D array"=w3996) -> ("1D Avg"=w4007:dbl[])  [unwired: 10 in]
    n1829 = call "AvgArrayTimeCritical.vi"("2D array"=w3992) -> ("1D Avg"=w4004:dbl[])  [unwired: 10 in]
    n1830 = call "AvgArrayTimeCritical.vi"("2D array"=w3985) -> ("1D Avg"=w3984:dbl[])  [unwired: 10 in]
    n1831 = Array Max & Min(array=w3997) -> (max value=w3995:dbl)  [unwired: 3 out]
    n1832 = Array Max & Min(array=w4007) -> (max value=w3994:dbl)  [unwired: 3 out]
    n1833 = Array Max & Min(array=w4004) -> (max value=w3978:dbl)  [unwired: 3 out]
    n1834 = Array Max & Min(array=w3984) -> (max value=w3982:dbl)  [unwired: 3 out]
    n1835 = local read "Auto gain ch4"() -> (w3983:bool)
    n1836 = local read "Auto gain ch1"() -> (w4001:bool)
    n1837 = local read "Auto gain ch2"() -> (w4000:bool)
    n1838 = local read "Auto gain ch3"() -> (w3999:bool)
    n1839 = case shown="True" w3983 {
      tunnel: w3982 -> [_ w4060]
      tunnel: "V target(1.0)" -> [_ w4058]
      tunnel: [FALSE w4055] -> w3980
      tunnel: [0.0 ("CtrlV") w4050] -> w3981
      frame False {
        # "Manual control"
      }
      frame True {
        # "PID control"
        n1840 = global read "GlobalVariables.vi" "Ch4GainLim(Log)"() -> (w4061:cluster{"GainMax":dbl, "GainMin":dbl})
        n1841 = call-poly <vilib>:"PID.vi"("output range"=w4061, "PID gains"="Ch4 PID gains", "process variable"=w4060, "setpoint"=w4058) -> ("output"=w4059:dbl)  [unwired: 6 in, 1 out]
        n1842 = Power Of 10(x=w4059) -> (10^x=w4051:dbl)
        "Gain4" <- w4051
        n1843 = call "V4FGV.vi"("action(write)"=enum16{"write", "read"}."read") -> ("Error Out"=w4054:errorcluster, "V3 out"=w4056:dbl)  [unwired: 9 in]
        n1844 = call "GainToCtrlV.vi"("Gain"=w4051, "Channel"=enum16{"Ch1", "Ch2", "Ch3", "Ch4"}."Ch4") -> ("CtrlV"=w4050:dbl)  [unwired: 8 in, 1 out]
        n1845 = call "V4FGV.vi"("Error In"=w4054, "V3 in"=w4050) -> ()  [unwired: 8 in, 2 out]
        n1846 = local write "V 4"(w4050) -> ()
        n1847 = Not Equal?(x=w4050, y=w4056) -> (x != y?=w4055:bool)
      }
    }
    n1848 = case shown="True" w4001 {
      tunnel: "V target(1.0)" -> [_ w4075]
      tunnel: w3995 -> [_ w4072]
      tunnel: [0.0 ("CtrlV") w4064] -> w3975
      tunnel: [FALSE w4066] -> w3991
      frame False {
        # "Manual control"
      }
      frame True {
        # "PID control"
        n1849 = global read "GlobalVariables.vi" "Ch1GainLim(Log)"() -> (w4071:cluster{"GainMax":dbl, "GainMin":dbl})
        n1850 = call-poly <vilib>:"PID.vi"("output range"=w4071, "PID gains"="Ch1 PID gains", "process variable"=w4072, "setpoint"=w4075) -> ("output"=w4070:dbl)  [unwired: 6 in, 1 out]
        n1851 = Power Of 10(x=w4070) -> (10^x=w4069:dbl)
        "Gain1" <- w4069
        n1852 = call "V1FGV.vi"("action (write)"=enum16{"write", "read"}."read") -> ("Error Out"=w4065:errorcluster, "V1 out"=w4067:dbl)  [unwired: 9 in]
        n1853 = call "GainToCtrlV.vi"("Gain"=w4069, "Channel"=enum16{"Ch1", "Ch2", "Ch3"}."Ch1") -> ("CtrlV"=w4064:dbl)  [unwired: 8 in, 1 out]
        n1854 = local write "V 1"(w4064) -> ()
        n1855 = call "V1FGV.vi"("Error In"=w4065, "V1 in"=w4064) -> ()  [unwired: 8 in, 2 out]
        n1856 = Not Equal?(x=w4064, y=w4067) -> (x != y?=w4066:bool)
      }
    }
    n1857 = case shown="True" w4000 {
      tunnel: w3994 -> [_ w4102]
      tunnel: "V target(1.0)" -> [_ w4103]
      tunnel: [FALSE w4096] -> w3990
      tunnel: [0.0 ("CtrlV") w4092] -> w3986
      frame False {
        # "Manual control"
      }
      frame True {
        # "PID control"
        n1858 = global read "GlobalVariables.vi" "Ch2GainLim(Log)"() -> (w4100:cluster{"GainMax":dbl, "GainMin":dbl})
        n1859 = call-poly <vilib>:"PID.vi"("output range"=w4100, "PID gains"="Ch2 PID gains", "process variable"=w4102, "setpoint"=w4103) -> ("output"=w4099:dbl)  [unwired: 6 in, 1 out]
        n1860 = Power Of 10(x=w4099) -> (10^x=w4097:dbl)
        "Gain2" <- w4097
        n1861 = call "V2FGV.vi"("action(write)"=enum16{"write", "read"}."read") -> ("Error Out"=w4093:errorcluster, "V2 out"=w4094:dbl)  [unwired: 9 in]
        n1862 = call "GainToCtrlV.vi"("Gain"=w4097, "Channel"=enum16{"Ch1", "Ch2", "Ch3"}."Ch2") -> ("CtrlV"=w4092:dbl)  [unwired: 8 in, 1 out]
        n1863 = local write "V 2"(w4092) -> ()
        n1864 = call "V2FGV.vi"("Error In"=w4093, "V2 in"=w4092) -> ()  [unwired: 8 in, 2 out]
        n1865 = Not Equal?(x=w4092, y=w4094) -> (x != y?=w4096:bool)
      }
    }
    n1866 = case shown="True" w3999 {
      tunnel: w3978 -> [_ w4087]
      tunnel: "V target(1.0)" -> [_ w4084]
      tunnel: [FALSE w4080] -> w3989
      tunnel: [0.0 ("CtrlV") w4078] -> w3988
      frame False {
        # "Manual control"
      }
      frame True {
        # "PID control"
        n1867 = global read "GlobalVariables.vi" "Ch3GainLim(Log)"() -> (w4088:cluster{"GainMax":dbl, "GainMin":dbl})
        n1868 = call-poly <vilib>:"PID.vi"("output range"=w4088, "PID gains"="Ch3 PID gains", "process variable"=w4087, "setpoint"=w4084) -> ("output"=w4086:dbl)  [unwired: 6 in, 1 out]
        n1869 = Power Of 10(x=w4086) -> (10^x=w4083:dbl)
        "Gain3" <- w4083
        n1870 = call "V3FGV.vi"("action(write)"=enum16{"write", "read"}."read") -> ("Error Out"=w4079:errorcluster, "V3 out"=w4081:dbl)  [unwired: 9 in]
        n1871 = call "GainToCtrlV.vi"("Gain"=w4083, "Channel"=enum16{"Ch1", "Ch2", "Ch3"}."Ch3") -> ("CtrlV"=w4078:dbl)  [unwired: 8 in, 1 out]
        n1872 = local write "V 3"(w4078) -> ()
        n1873 = call "V3FGV.vi"("Error In"=w4079, "V3 in"=w4078) -> ()  [unwired: 8 in, 2 out]
        n1874 = Not Equal?(x=w4078, y=w4081) -> (x != y?=w4080:bool)
      }
    }
    n1875 = call "LabJack_FGV.vi"("Operation(Read)"=enum16{"Write", "Read"}."Read" ("Operation"), "error in (no error)"=w3967) -> ("error out"=w3976:errorcluster, "Read data"=w4011:i32)  [unwired: 8 in]
    n1876 = flat-sequence {
      tunnel: [w4015] -> w3973
      tunnel: w3967 -> [_]
      frame #0 {
        n1877 = Tick Count (ms)() -> (millisecond timer value=w4015:u32)
      }
    }
    n1878 = case "Channel 1" shown="True" w3991 {
      tunnel: w3976 -> [w4041 w4047]
      tunnel: w4011 -> [w4040 w4046]
      tunnel: [w4041 w4042] -> w3971
      tunnel: [w4040 w4045] -> w4006
      tunnel: w3975 -> [_ w4043]
      frame False {
        # "Do nothing"
      }
      frame True {
        # "request V\nupdate FGV"
        n1879 = global read "GlobalVariables.vi" "Ch1 LJ pin"() -> (w4044:string)
        n1880 = call "LJM_eWriteName.vi"("Handle In"=w4046, "Name"=w4044, "Value"=w4043, "error in"=w4047) -> ("Handle Out"=w4045:i32, "error out"=w4042:errorcluster)  [unwired: 10 in]
      }
    }
    n1881 = case "Channel 2" shown="True" w3990 {
      tunnel: w3971 -> [w4032 w4039]
      tunnel: [w4032 w4034] -> w3970
      tunnel: w4006 -> [w4033 w4038]
      tunnel: [w4033 w4037] -> w4005
      tunnel: w3986 -> [_ w4035]
      frame False {
        # "Do nothing"
      }
      frame True {
        # "request V\nupdate FGV"
        n1882 = global read "GlobalVariables.vi" "Ch2 LJ pin"() -> (w4036:string)
        n1883 = call "LJM_eWriteName.vi"("Handle In"=w4038, "Name"=w4036, "Value"=w4035, "error in"=w4039) -> ("Handle Out"=w4037:i32, "error out"=w4034:errorcluster)  [unwired: 10 in]
      }
    }
    n1884 = case "Channel 3" shown="True" w3989 {
      tunnel: w3970 -> [w4025 w4031]
      tunnel: [w4025 w4027] -> w3969
      tunnel: w4005 -> [w4024 w4030]
      tunnel: w3988 -> [_ w4028]
      tunnel: [w4024 w4026] -> w3979
      frame False {
        # "Do nothing"
      }
      frame True {
        # "request V\nupdate FGV"
        n1885 = global read "GlobalVariables.vi" "Ch3 LJ pin"() -> (w4029:string)
        n1886 = call "LJM_eWriteName.vi"("Handle In"=w4030, "Name"=w4029, "Value"=w4028, "error in"=w4031) -> ("Handle Out"=w4026:i32, "error out"=w4027:errorcluster)  [unwired: 10 in]
      }
    }
    n1887 = case "Channel 4" shown="True" w3980 {
      tunnel: w3969 -> [w4017 w4023]
      tunnel: w3979 -> [w4016 w4022]
      tunnel: [w4017 w4018] -> w3974
      tunnel: [w4016 w4021] -> _
      tunnel: w3981 -> [_ w4019]
      frame False {
        # "Do nothing"
      }
      frame True {
        # "request V\nupdate FGV"
        n1888 = global read "GlobalVariables.vi" "Ch4 LJ pin"() -> (w4020:string)
        n1889 = call "LJM_eWriteName.vi"("Handle In"=w4022, "Name"=w4020, "Value"=w4019, "error in"=w4023) -> ("Handle Out"=w4021:i32, "error out"=w4018:errorcluster)  [unwired: 10 in]
      }
    }
    "PID loop error out" <- w3974
    n1890 = flat-sequence {
      tunnel: [w4014] -> w3972
      tunnel: w3974 -> [_]
      frame #0 {
        n1891 = Tick Count (ms)() -> (millisecond timer value=w4014:u32)
      }
    }
    n1892 = Subtract(x=w3972, y=w3973) -> (x-y=w3968:u32)
    "LJ process (ms)" <- w3968
    "PID loop" <- w3993
  }
  "LJ time(ms)" <- w1
  n1893 = Unregister For Events(event registration refnum=w46, error in=w4) -> (error out=w52:errorcluster)
  n1894 = Destroy User Event(user event=w39, error in=w52) -> (error out=w3:errorcluster)
  n1895 = Close File(refnum=w21, error in=w3) -> ()  [unwired: 2 out]
  n1896 = Release Notifier(notifier=w16, error in (no error)=w49) -> (error out=w50:errorcluster)  [unwired: 1 in, 2 out]
  n1897 = Release Notifier(notifier=w17, error in (no error)=w38) -> (error out=w43:errorcluster)  [unwired: 1 in, 2 out]
  n1898 = call <vilib>:"Simple Error Handler.vi"("error in (no error)"=w50) -> ()  [unwired: 4 in, 5 out]
  n1899 = call <vilib>:"Simple Error Handler.vi"("error in (no error)"=w43) -> ()  [unwired: 4 in, 5 out]
  n1900 = Release Notifier(notifier=w59, error in (no error)=w58) -> (error out=w57:errorcluster)  [unwired: 1 in, 2 out]
  n1901 = Unregister For Events(event registration refnum=w63, error in=w61) -> (error out=w62:errorcluster)
  n1902 = call <vilib>:"Simple Error Handler.vi"("error in (no error)"=w57) -> ()  [unwired: 4 in, 5 out]
  n1903 = Destroy User Event(user event=w53, error in=w62) -> ()  [unwired: 1 out]
